vi "NoGV_Omniax_MotorDrive_XYZR_20101203stable2.vi"() -> ()   [LabVIEW 2009]
uses:
  <vilib>/Utility/file.llb/Read From Spreadsheet File (DBL).vi
  <vilib>/Utility/file.llb/Read From Spreadsheet File (string).vi
  <vilib>/Instr/_visa.llb/VISA Configure Serial Port (Instr).vi
  <vilib>/Utility/file.llb/Write To Spreadsheet File (string).vi
  <vilib>/Utility/file.llb/Write To Spreadsheet File (DBL).vi
panel:
  out "Scanning":bool
  out "Laser Shutter":bool
  in  "SHUTTER SYNC":bool
  in  "Laser Shutter":bool
  out "#th loop":dbl
  in  "# of loops":dbl
  in  "LOOP":bool
  out "OP":bool
  out "CL":bool
  out "Valve \nopend/closed":bool
  in  "OK Button":bool
  out "STATUS":string
  in  "Delete Button":bool
  in  "String":string
  in  "Add Button":bool
  in  "Set Button":bool
  in  "Preset positions":i32(ring) items=["ZERO", "Default", "CDOSE", "QMS", "test", "test2", "test3", "yag position", "Sample Long Edge  ", "SPUTTER POS"]
  out "Presets":i32[][](array[numeric])
  out "X MINPOS":i32=-94296
  out "X MAXPOS":i32=-34296
  out "Y MINPOS":i32=-94296
  out "Y MAXPOS":i32=-34296
  out "R MAXPOS":i32=-34296
  out "R MINPOS":i32=-94296
  out "Z MINPOS":i32=-94296
  out "Z MAXPOS":i32=-34296
  in  "HARDSTOP":bool
  in  "GO":bool
  out "XYZR VEL PV Array":i32[](array[numeric])
  out "XYZ in RANGE Array":bool[](array[boolean])
  out "STEP SP Array":i32[](array[numeric])
  out "RUNHOLDArray":i32[](array[numeric])
  out "ZCONSTArray":dbl[](array[numeric])
  out "RCONSTArray":dbl[](array[numeric])
  out "XCONSTArray":dbl[](array[numeric])
  out "YCONSTArray":dbl[](array[numeric])
  out "Error Array":errorcluster[](array[cluster])
  out "COM PORT Array":refnum<visa-resource-name>[](array[refnum])
  out "Z COM PORT":refnum<visa-resource-name>="COM6"
  in  "Tab Control 3":enum32{"Status", "Reset"}(tab)
  out "Y in Range":bool
  out "Y Scan":bool
  out "Y in Motion":bool
  out "Y Backlash corr":bool
  out "X  in Range":bool
  out "X Scan":bool
  out "X  in Motion":bool
  out "X Backlash corr":bool
  out "Z in Range":bool
  out "Z Scan":bool
  out "Z in Motion":bool
  out "Z Backlash corr":bool
  out "R in Range":bool
  out "R Scan":bool
  out "R in Motion":bool
  out "R Backlash corr":bool
  out "X Ready":bool
  out "Y Ready":bool
  out "Z Ready":bool
  out "R Ready":bool
  in  "Reset Y Position mm":dbl
  out "Reset Y Motor Steps":i32
  in  "Reset X Position mm":dbl
  out "Reset X Motor Steps":i32
  in  "Reset Z Position mm":dbl
  out "Reset Z Motor Steps":i32
  in  "Reset R Position deg":dbl
  out "Reset R Motor Steps":i32
  in  "Reset":bool
  in  "Tab Control 2":enum32{"mm", "step"}(tab)
  in  "X Scan Length SP mm":dbl
  in  "X Scan Velocity SP mm/sec":dbl
  in  "Y Scan Length SP mm":dbl
  in  "Y Scan Velocity SP mm/sec":dbl
  in  "Set Scan \nParameters":bool
  in  "Z Scan Length SP mm":dbl
  in  "Z Scan Velocity SP mm/sec":dbl
  in  "R Scan Length SP deg":dbl
  in  "R Scan Velocity SP deg/sec":dbl
  in  "Z as dominating length":bool
  in  "X Scan Velocity SP steps/sec":i32=1 min=1 max=102400 step=1
  in  "X Scan Length SP steps":i32 min=-2304000 max=2304000 step=100
  out "X Scan length MV mm":dbl
  out "X Scan velocity MV mm/sec":dbl format="%#_6f"
  in  "Y Scan Velocity SP steps/sec":i32=1 min=1 max=102400 step=1
  in  "Y Scan Length SP steps":i32 min=-2304000 max=2304000 step=100
  out "Y Scan length MV mm":dbl
  out "Y Scan velocity MV mm/sec":dbl format="%#_6f"
  in  "Z Scan Velocity SP steps/sec":i32=1 min=1 max=204800 step=1
  in  "Z Scan Length SP steps":i32 min=-10240000 max=92160000 step=100
  out "Z Scan length MV mm":dbl
  out "Z Scan velocity MV mm/sec":dbl format="%#_6f"
  in  "R Scan Velocity SP steps/sec":i32=1 min=1 max=102400 step=1
  in  "R Scan Length SP steps":i32 min=-1501867 max=4642133 step=100
  out "R Scan length MV deg":dbl
  out "R Scan velocity MV deg/sec":dbl format="%#_6f"
  out "atan Y/Z":dbl
  in  "Tab Control":enum32{"mm", "step"}(tab)
  in  "X Position SP mm":dbl
  in  "X Velocity SP mm/sec":dbl
  in  "X Move Set":bool
  in  "Y Move Set":bool
  in  "Y Position SP mm":dbl
  in  "Y Velocity SP mm/sec":dbl
  in  "Z Position SP mm":dbl
  in  "Z Velocity SP mm/sec":dbl
  in  "Z Move Set":bool
  in  "R Position SP deg":dbl
  in  "R Velocity SP deg/sec":dbl
  in  "R Move Set":bool
  in  "X Velocity SP step/sec":i32 min=1 max=128000
  out "X Velocity MV mm/sec":dbl
  in  "Y Velocity SP step/sec":i32 min=1 max=128000
  out "Y Velocity MV mm/sec":dbl
  in  "Z Velocity SP step/sec":i32 min=1 max=204800
  out "Z Velocity MV mm/sec":dbl
  in  "R Velocity SP step/sec":i32 min=1 max=20000
  out "R Velocity MVdeg/sec":dbl
  in  "Y Step SP":i32=-20000 min=-2304000 max=2304000 step=500
  out "Y Position MV mm":dbl
  in  "X Step SP":i32=-20000 min=-2304000 max=2304000 step=500
  out "X Position MV mm":dbl
  in  "Z Step SP":i32=-20000 min=0 max=102400000 step=500
  out "Z Position MV mm":dbl
  in  "R Step SP":i32=-20000 min=-6144000 max=0 step=500
  out "R Position MV deg":dbl
  out "X Step PV":i32 max=2000
  out "Y Step PV":i32 max=2000
  out "Z Step PV":i32 max=2000
  out "R Step PV":i32 max=2000
  in  "Clear ZY":bool
  out "ZY Graph":cluster{dbl[], dbl[]}(graph)
  out "ZR Graph":cluster{"Y":dbl[], "Y":dbl[]}[](graph)
  out "XY Graph":cluster{"Y":dbl[], "Y":dbl[]}[](graph)
  out "X Scan Duration":dbl
  out "Y Scan Duration":dbl
  out "Z Scan Duration":dbl
  out "R Scan Duration":dbl
  out "R Backlash steps/sec":i32
  out "R Backlash":i32
  out "R Holding Current %":i32
  out "R Run Current %":i32
  out "R offset deg":dbl
  out "R deg/rev":dbl
  out "R steps/rev":u32
  out "R velocity PV step/sec":i32
  out "R COM PORT":refnum<visa-resource-name>="COM5"
  out "R Position deg PV":dbl=270.5
  out "Z Backlash steps/sec":i32
  out "Z Backlash":i32
  out "Z Holding Current %":i32
  out "Z Run Current %":i32
  out "Z offset mm":dbl
  out "Z mm/rev":dbl
  out "Z steps/rev":u32
  out "Z  velocity PV step/sec":i32
  out "Z Position mm PV":dbl=45.0
  out "X Position mm PV":dbl
  out "X velocity PV step/sec":i32
  in  "Send scan parameter":bool
  out "X Backlash steps/sec":i32
  out "X Backlash":i32
  out "X Holding Current %":i32
  out "X Run Current %":i32
  out "X offset mm":dbl
  out "X mm/rev":dbl
  out "X steps/rev":u32
  out "X COM PORT":refnum<visa-resource-name>="COM5"
  out "Y Backlash steps/sec":i32
  out "Y Backlash":i32
  out "Y Holding Current %":i32
  out "Y Run Current %":i32
  in  "Scan Cancel":bool
  out "Y Position mm PV":dbl
  out "Y offset mm":dbl
  out "Y mm/rev":dbl
  out "Y steps/rev":u32
  out "Y velocity PV step/sec":i32
  in  "Scan Go":bool
  in  "Stop":bool
  out "Y COM PORT":refnum<visa-resource-name>="COM5"
  # "MX"
  # "MY"
  # "MZ"
  # "MR"
  # "Indicators"
  # "L"
  # "M"
  # "B"
  # "S"
  # "R"
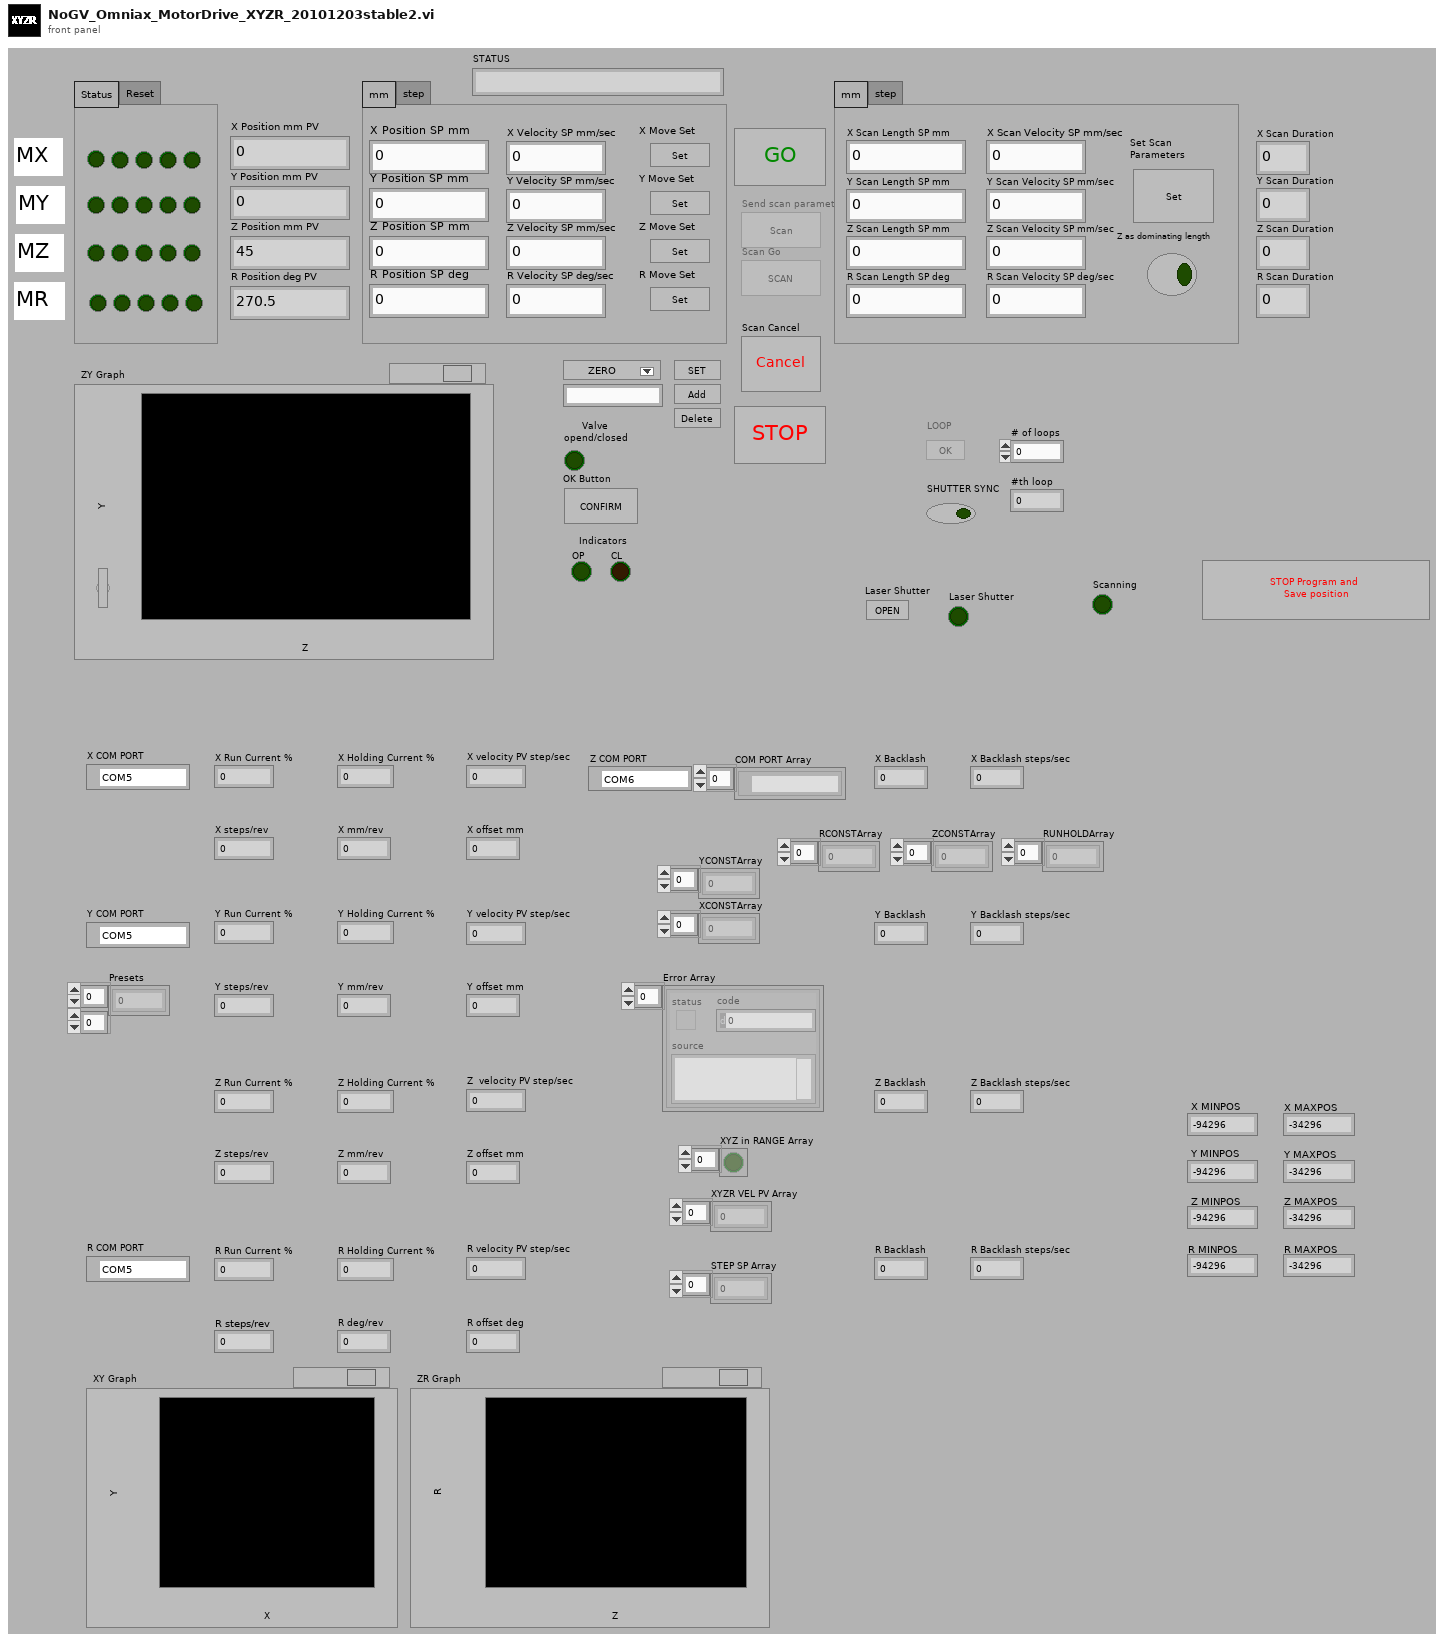
[diagram p1: front panel]
types:
  T1 = cluster{"Error Array OUT[0]":errorcluster, "Error Array OUT[1]":errorcluster, "Error Array OUT[2]":errorcluster, "Error Array OUT[3]":errorcluster, "Error Array OUT[4]":errorcluster, "Error Array OUT[5]":errorcluster, "Error Array OUT[6]":errorcluster, "Error Array OUT[7]":errorcluster, "Error Array OUT[8]":errorcluster}
  T2 = cluster{"COM PORT Array OUT[0]":refnum<visa-resource-name>, "COM PORT Array OUT[1]":refnum<visa-resource-name>, "COM PORT Array OUT[2]":refnum<visa-resource-name>, "COM PORT Array OUT[3]":refnum<visa-resource-name>, "COM PORT Array OUT[4]":refnum<visa-resource-name>, "COM PORT Array OUT[5]":refnum<visa-resource-name>, "COM PORT Array OUT[6]":refnum<visa-resource-name>, "COM PORT Array OUT[7]":refnum<visa-resource-name>, "COM PORT Array OUT[8]":refnum<visa-resource-name>}
  T3 = cluster{"STEP SP Array OUT[0]":i32, "STEP SP Array OUT[1]":i32, "STEP SP Array OUT[2]":i32, "STEP SP Array OUT[3]":i32, "STEP SP Array OUT[4]":i32, "STEP SP Array OUT[5]":i32, "STEP SP Array OUT[6]":i32, "STEP SP Array OUT[7]":i32, "STEP SP Array OUT[8]":i32}
  T4 = cluster{"XYZR MAX MIN POS[0]":i32, "XYZR MAX MIN POS[1]":i32, "XYZR MAX MIN POS[2]":i32, "XYZR MAX MIN POS[3]":i32, "XYZR MAX MIN POS[4]":i32, "XYZR MAX MIN POS[5]":i32, "XYZR MAX MIN POS[6]":i32, "XYZR MAX MIN POS[7]":i32, "XYZR MAX MIN POS[8]":i32}
  T5 = cluster{"XYZ in RANGE Array OUT[0]":bool, "XYZ in RANGE Array OUT[1]":bool, "XYZ in RANGE Array OUT[2]":bool, "XYZ in RANGE Array OUT[3]":bool, "XYZ in RANGE Array OUT[4]":bool, "XYZ in RANGE Array OUT[5]":bool, "XYZ in RANGE Array OUT[6]":bool, "XYZ in RANGE Array OUT[7]":bool, "XYZ in RANGE Array OUT[8]":bool}
  T6 = cluster{"XY Max Min array OUT[0]":dbl, "XY Max Min array OUT[1]":dbl, "XY Max Min array OUT[2]":dbl, "XY Max Min array OUT[3]":dbl, "XY Max Min array OUT[4]":dbl, "XY Max Min array OUT[5]":dbl, "XY Max Min array OUT[6]":dbl, "XY Max Min array OUT[7]":dbl, "XY Max Min array OUT[8]":dbl}
  T7 = cluster{"XYZR VEL PV Array OUT[0]":i32, "XYZR VEL PV Array OUT[1]":i32, "XYZR VEL PV Array OUT[2]":i32, "XYZR VEL PV Array OUT[3]":i32, "XYZR VEL PV Array OUT[4]":i32, "XYZR VEL PV Array OUT[5]":i32, "XYZR VEL PV Array OUT[6]":i32, "XYZR VEL PV Array OUT[7]":i32, "XYZR VEL PV Array OUT[8]":i32}
  T8 = cluster{"[0]":i32, "[1]":i32, "[2]":i32, "[3]":i32, "[4]":i32, "[5]":i32, "[6]":i32, "[7]":i32, "[8]":i32}
  T9 = enum8{"Enabled", "Disabled", "Disabled and Grayed Out"}
  T10 = enum16{"Stop", "Reset", "Run Current", "Holding Current", "Accel Rate", "Decel Rate", "Move to Relative Position", "Move to Absolute Position", "Echo Mode", "Print Parameter", "Send String", "Microstep Resolution", "Set Current Position", "Max Velocity"}
  T11 = cluster{"Presets[0]":i32, "Presets[1]":i32, "Presets[2]":i32, "Presets[3]":i32, "Presets[4]":i32, "Presets[5]":i32, "Presets[6]":i32, "Presets[7]":i32, "Presets[8]":i32}
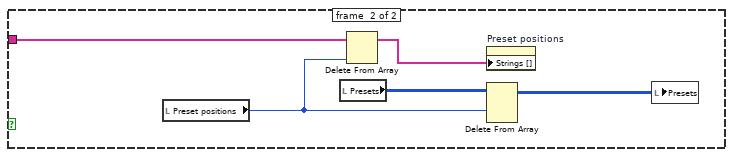
[diagram p4: hidden frame]
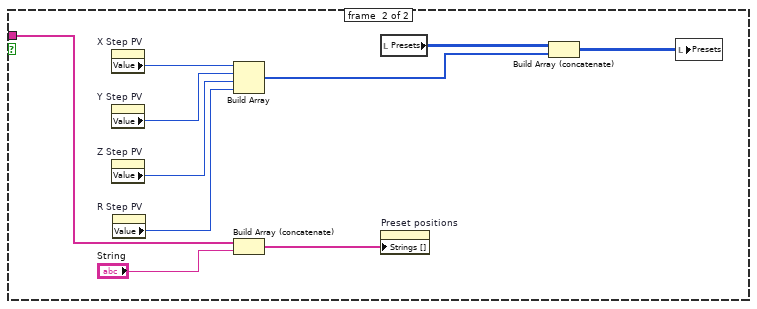
[diagram p5: hidden frame]
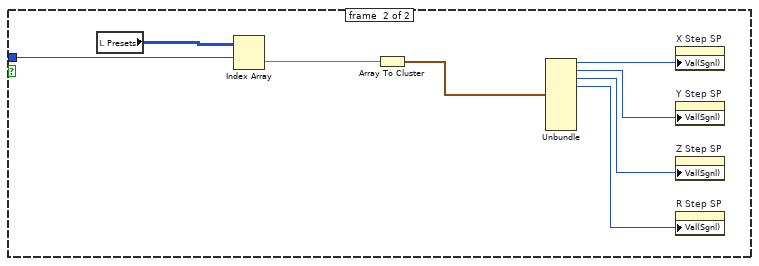
[diagram p6: hidden frame]
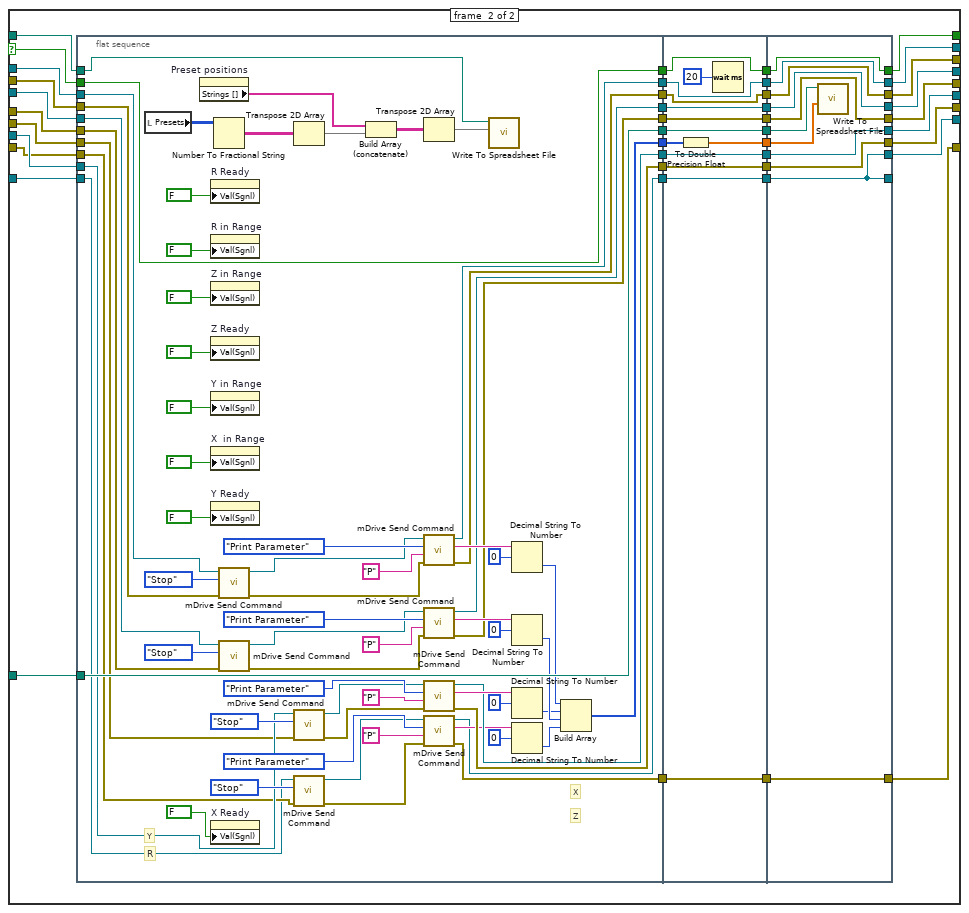
[diagram p7: hidden frame]
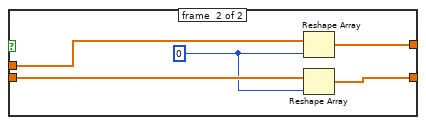
[diagram p8: hidden frame]
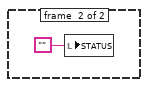
[diagram p10: hidden frame]
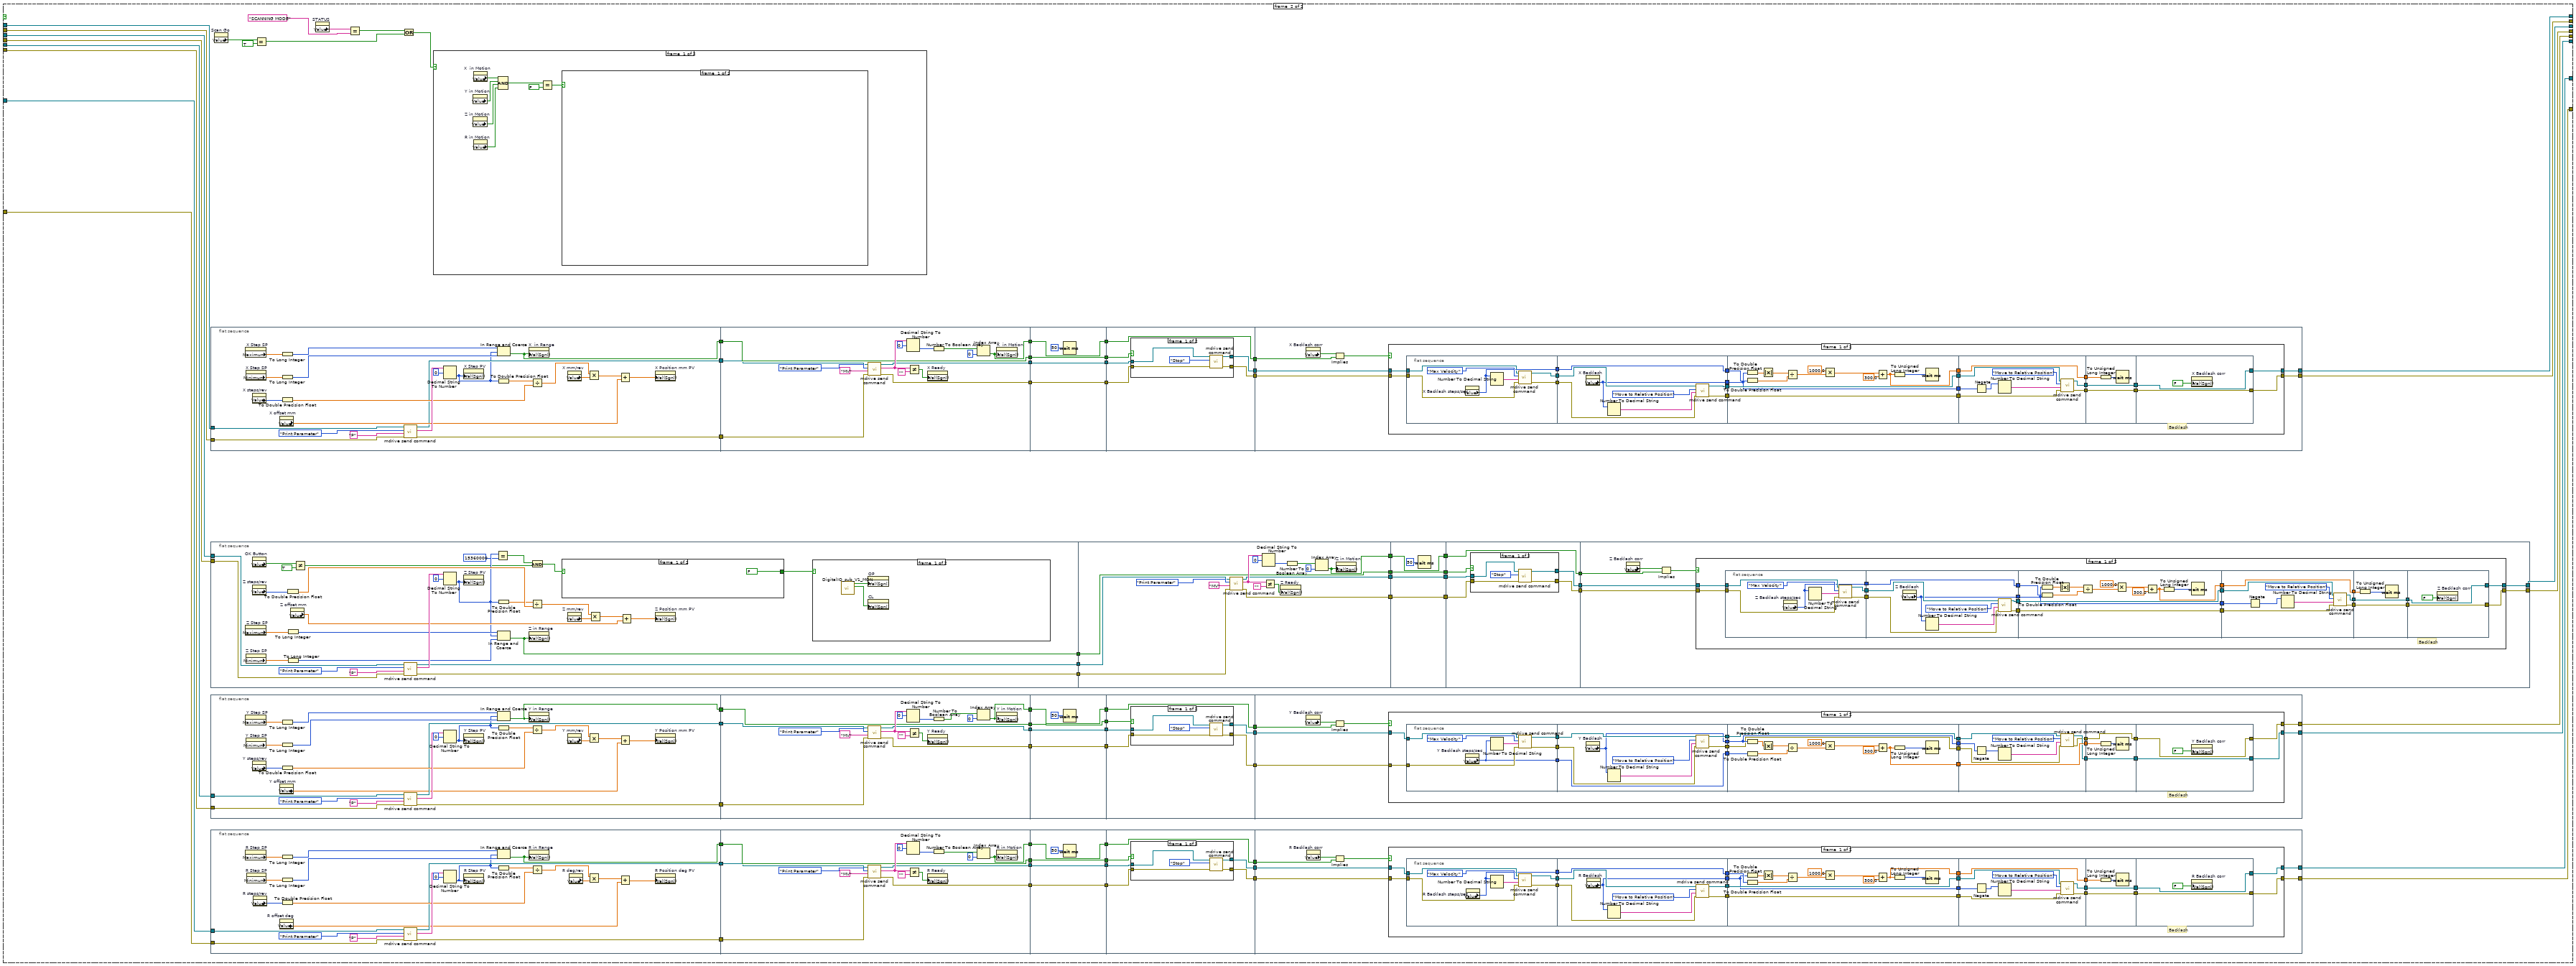
[diagram p11: hidden frame]
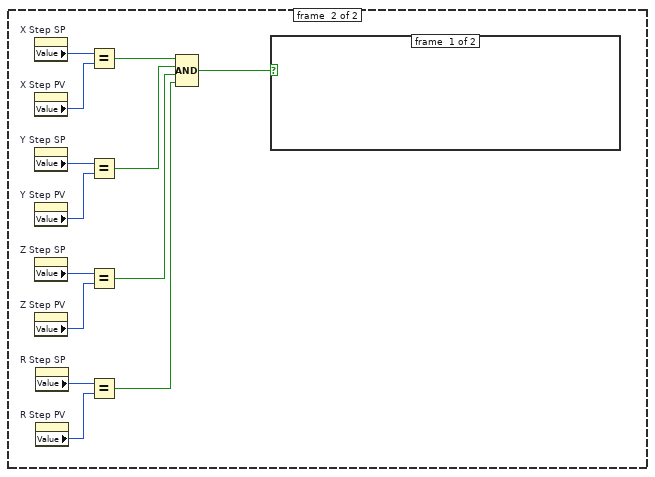
[diagram p12: hidden frame]
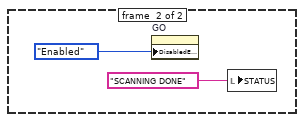
[diagram p13: hidden frame]
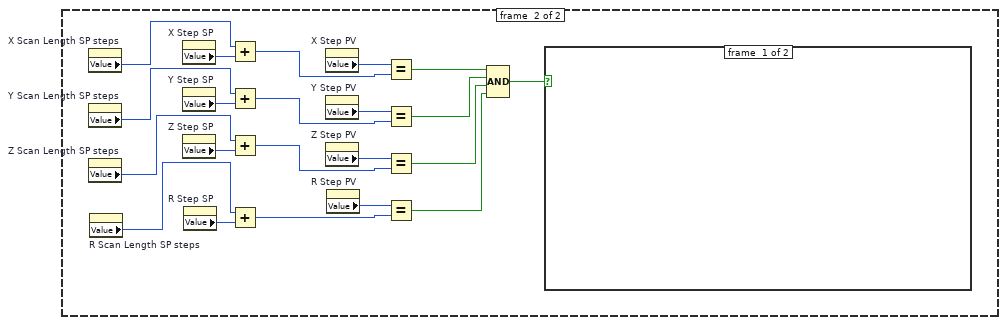
[diagram p14: hidden frame]
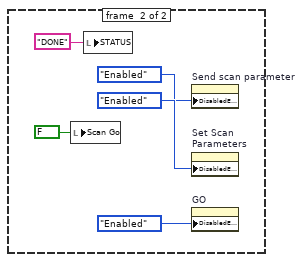
[diagram p15: hidden frame]
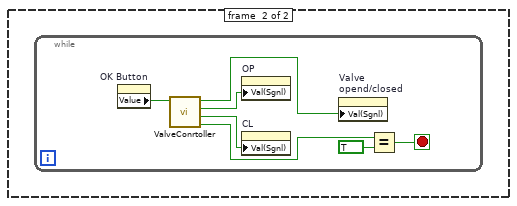
[diagram p20: hidden frame]
diagram:
  (unwired) FALSE ("LOOP MODE")
  n1 = flat-sequence {
    tunnel: [w153] -> w10
    tunnel: [w152] -> w9
    tunnel: [w151] -> w8
    tunnel: [w150] -> w7
    tunnel: [w149] -> w6
    tunnel: [w148] -> w5
    tunnel: [w147] -> w4
    tunnel: [w146] -> w3
    tunnel: [w143] -> w2
    tunnel: [w113] -> w1
    tunnel: [w188] -> w13
    tunnel: [w189] -> w14
    tunnel: [w190] -> w15
    tunnel: [w191] -> w16
    tunnel: [w192] -> w17
    tunnel: [w193] -> w18
    tunnel: [w194] -> w19
    tunnel: [w195] -> w20
    tunnel: [w196] -> w21
    tunnel: [w197] -> w22
    tunnel: w10 -> [w197]
    tunnel: w9 -> [w196]
    tunnel: w8 -> [w195]
    tunnel: w7 -> [w194]
    tunnel: w6 -> [w193]
    tunnel: w5 -> [w192]
    tunnel: w4 -> [w191]
    tunnel: w3 -> [w190]
    tunnel: w2 -> [w189]
    tunnel: w1 -> [w188]
    frame #0 {
      w113 = path "C:/Documents and Settings/b_ogasawara/Desktop/lv1/LV codes/IMS/PRESET.TXT"
      w111 = 0 ("element")
      w143 = path "C:/Documents and Settings/b_ogasawara/Desktop/lv1/LV codes/IMS/POS.TXT"
      w173 = refnum<visa-resource-name> "COM7" ("COM PORT")
      w174 = refnum<visa-resource-name> "COM5" ("COM PORT")
      w175 = refnum<visa-resource-name> "COM6" ("VISA resource name")
      w176 = refnum<visa-resource-name> "COM4" ("COM PORT")
      n2 = property on="Z Step SP" class="DigNum (strict)"() -> ("Maximum"=w68:dbl)  [unwired: 2 in, 2 out]
      n3 = property on="R Step SP" class="DigNum (strict)"() -> ("Maximum"=w66:dbl)  [unwired: 2 in, 2 out]
      n4 = property on="Z Step SP" class="DigNum (strict)"() -> ("Minimum"=w69:dbl)  [unwired: 2 in, 2 out]
      n5 = property on="R Step SP" class="DigNum (strict)"() -> ("Minimum"=w67:dbl)  [unwired: 2 in, 2 out]
      n6 = property on="X steps/rev" class="DigNum (strict)"() -> ("Value"=w84:u32)  [unwired: 2 in, 2 out]
      n7 = property on="Y steps/rev" class="DigNum (strict)"() -> ("Value"=w83:u32)  [unwired: 2 in, 2 out]
      n8 = property on="Z steps/rev" class="DigNum (strict)"() -> ("Value"=w82:u32)  [unwired: 2 in, 2 out]
      n9 = property on="R steps/rev" class="DigNum (strict)"() -> ("Value"=w81:u32)  [unwired: 2 in, 2 out]
      n10 = call "DigitalIO_sub_V1_MON.vi"() -> ("CL"=w70:bool, "OP"=w71:bool)  [unwired: 8 in]
      n11 = local read "RUNHOLDArray"() -> (w163:i32[])
      n12 = local read "STEP SP Array"() -> (w166:i32[])
      n13 = local read "XYZ in RANGE Array"() -> (w165:bool[])
      n14 = local read "XYZR VEL PV Array"() -> (w164:i32[])
      n15 = property on="R offset deg" class="DigNum (strict)"() -> ("Value"=w76:dbl)  [unwired: 2 in, 2 out]
      n16 = property on="X offset mm" class="DigNum (strict)"() -> ("Value"=w73:dbl)  [unwired: 2 in, 2 out]
      n17 = property on="Y offset mm" class="DigNum (strict)"() -> ("Value"=w74:dbl)  [unwired: 2 in, 2 out]
      n18 = property on="Z offset mm" class="DigNum (strict)"() -> ("Value"=w75:dbl)  [unwired: 2 in, 2 out]
      n19 = property on="OP" class="Bool (strict)"("Val(Sgnl)"=w71) -> ()  [unwired: 2 in, 2 out]
      n20 = property on="CL" class="Bool (strict)"("Val(Sgnl)"=w70) -> ()  [unwired: 2 in, 2 out]
      n21 = Build Array(w176, w175, w174, w173) -> (w171:refnum<visa-resource-name>[])
      n22 = Build Array(w68, w69, w66, w67) -> (w65:dbl[])
      n23 = local write "STATUS"("INITIALIZING" ("STATUS")) -> ()
      n24 = for {
        N: 4 -> [_]
        tunnel: w171 -> [w179] mode=indexing
        tunnel: [w178] -> w169 mode=indexing
        tunnel: [w177] -> w170 mode=indexing
        w181 = u16 0 items=["None", "XON/XOFF", "RTS/CTS", "XON/XOFF & RTS/CTS", "DTR/DSR", "XON/XOFF & DTR/DSR"] ("flow control (0:none)")
        w182 = u16 10 items=["1.0"=10, "1.5"=15, "2.0"=20] ("stop bits (10: 1 bit)")
        # "Stop bits"
        n25 = call-poly "VISA Configure Serial Port"("VISA resource name"=w179, "timeout (10sec)"=u32 10000, "baud rate (9600)"=u32 9600, "data bits (8)"=u16 8, "parity (0:none)"=enum16{"None", "Odd", "Even", "Mark", "Space"}."None", "stop bits (10: 1 bit)"=w182, "flow control (0:none)"=w181) -> ("VISA resource name out"=w178:refnum<visa-resource-name>, "error out"=w177:errorcluster)  [unwired: 7 in]
      }
      "COM PORT Array" <- w169
      "Error Array" <- w170
      n26 = call "InitializeMotorsXYZR_V2.vi"("COM PORT Array IN"=w169, "STEP SP Array IN"=w166, "XYZ in RANGE Array IN"=w165, "XYZR VEL PV Array IN"=w164, "RUNHOLDArray IN"=w163, "Error Array IN"=w170, "ZR Max Min array"=w65) -> ("XY Max Min array OUT"=w64:dbl[], "COM PORT Array OUT"=w168:refnum<visa-resource-name>[], "STEP SP Array OUT"=w162:i32[], "XYZ in RANGE Array OUT"=w161:bool[], "XYZR VEL PV Array OUT"=w160:i32[], "XYZR MAX MIN POS"=w145:i32[], "Error Array OUT"=w167:errorcluster[])  [unwired: 6 in]
      n27 = Array To Cluster(array=w167) -> (cluster=w158:T1)
      n28 = Array To Cluster(array=w168) -> (cluster=w159:T2)
      n29 = Array To Cluster(array=w162) -> (cluster=w157:T3)
      n30 = Array To Cluster(array=w145) -> (cluster=w154:T4)
      n31 = Array To Cluster(array=w161) -> (cluster=w156:T5)
      n32 = Array To Cluster(array=w64) -> (cluster=w63:T6)
      n33 = Array To Cluster(array=w160) -> (cluster=w155:T7)
      n34 = Unbundle(w157) -> ("STEP SP Array OUT[0]"=w127:i32, "STEP SP Array OUT[1]"=w128:i32, "STEP SP Array OUT[2]"=w129:i32, "STEP SP Array OUT[3]"=w130:i32)  [unwired: 5 out]
      n35 = Unbundle(w154) -> ("XYZR MAX MIN POS[0]"=w138:i32, "XYZR MAX MIN POS[1]"=w137:i32, "XYZR MAX MIN POS[2]"=w136:i32, "XYZR MAX MIN POS[3]"=w135:i32, "XYZR MAX MIN POS[4]"=w134:i32, "XYZR MAX MIN POS[5]"=w133:i32, "XYZR MAX MIN POS[6]"=w132:i32, "XYZR MAX MIN POS[7]"=w131:i32)  [unwired: 1 out]
      n36 = Unbundle(w156) -> ("XYZ in RANGE Array OUT[0]"=w142:bool, "XYZ in RANGE Array OUT[1]"=w141:bool, "XYZ in RANGE Array OUT[2]"=w140:bool, "XYZ in RANGE Array OUT[3]"=w139:bool)  [unwired: 5 out]
      n37 = Unbundle(w63) -> ("XY Max Min array OUT[0]"=w62:dbl, "XY Max Min array OUT[1]"=w60:dbl, "XY Max Min array OUT[2]"=w59:dbl, "XY Max Min array OUT[3]"=w61:dbl)  [unwired: 5 out]
      n38 = Unbundle(w155) -> ("XYZR VEL PV Array OUT[0]"=w126:i32, "XYZR VEL PV Array OUT[1]"=w125:i32, "XYZR VEL PV Array OUT[2]"=w124:i32, "XYZR VEL PV Array OUT[3]"=w123:i32)  [unwired: 5 out]
      n39 = call-poly <vilib>:"Read From Spreadsheet File.vi"("file path (dialog if empty)"=w113) -> ("all rows"=w118:string[][])  [unwired: 6 in, 4 out]
      n40 = call-poly <vilib>:"Read From Spreadsheet File.vi"("file path (dialog if empty)"=w143) -> ("first row"=w144:dbl[])  [unwired: 6 in, 4 out]
      n41 = To Long Integer(number=w144) -> (32bit integer=w110:i32[])
      n42 = Transpose 2D Array(2D array=w118) -> (transposed array=w117:string[][])
      n43 = property on="X Step SP" class="DigNum (strict)"("Val(Sgnl)"=w127) -> ()  [unwired: 2 in, 2 out]
      n44 = property on="Y Step SP" class="DigNum (strict)"("Val(Sgnl)"=w128) -> ()  [unwired: 2 in, 2 out]
      n45 = property on="Z Step SP" class="DigNum (strict)"("Val(Sgnl)"=w129) -> ()  [unwired: 2 in, 2 out]
      n46 = property on="R Step SP" class="DigNum (strict)"("Val(Sgnl)"=w130) -> ()  [unwired: 2 in, 2 out]
      n47 = property on="X MAXPOS" class="DigNum (strict)"("Val(Sgnl)"=w138) -> ()  [unwired: 2 in, 2 out]
      n48 = property on="X MINPOS" class="DigNum (strict)"("Val(Sgnl)"=w137) -> ()  [unwired: 2 in, 2 out]
      n49 = property on="Y MAXPOS" class="DigNum (strict)"("Val(Sgnl)"=w136) -> ()  [unwired: 2 in, 2 out]
      n50 = property on="Y MINPOS" class="DigNum (strict)"("Val(Sgnl)"=w135) -> ()  [unwired: 2 in, 2 out]
      n51 = property on="Z MAXPOS" class="DigNum (strict)"("Val(Sgnl)"=w134) -> ()  [unwired: 2 in, 2 out]
      n52 = property on="Z MINPOS" class="DigNum (strict)"("Val(Sgnl)"=w133) -> ()  [unwired: 2 in, 2 out]
      n53 = property on="R MAXPOS" class="DigNum (strict)"("Val(Sgnl)"=w132) -> ()  [unwired: 2 in, 2 out]
      n54 = property on="R MINPOS" class="DigNum (strict)"("Val(Sgnl)"=w131) -> ()  [unwired: 2 in, 2 out]
      n55 = property on="X  in Range" class="Bool (strict)"("Val(Sgnl)"=w142) -> ()  [unwired: 2 in, 2 out]
      n56 = property on="Y in Range" class="Bool (strict)"("Val(Sgnl)"=w141) -> ()  [unwired: 2 in, 2 out]
      n57 = property on="Z in Range" class="Bool (strict)"("Val(Sgnl)"=w140) -> ()  [unwired: 2 in, 2 out]
      n58 = property on="R in Range" class="Bool (strict)"("Val(Sgnl)"=w139) -> ()  [unwired: 2 in, 2 out]
      n59 = property on="X velocity PV step/sec" class="DigNum (strict)"("Val(Sgnl)"=w126) -> ()  [unwired: 2 in, 2 out]
      n60 = property on="R velocity PV step/sec" class="DigNum (strict)"("Val(Sgnl)"=w123) -> ()  [unwired: 2 in, 2 out]
      n61 = property on="X Step SP" class="DigNum (strict)"("Maximum"=w62) -> ()  [unwired: 2 in, 2 out]
      n62 = property on="X Step SP" class="DigNum (strict)"("Minimum"=w60) -> ()  [unwired: 2 in, 2 out]
      n63 = property on="Y Step SP" class="DigNum (strict)"("Maximum"=w59) -> ()  [unwired: 2 in, 2 out]
      n64 = property on="Y Step SP" class="DigNum (strict)"("Minimum"=w61) -> ()  [unwired: 2 in, 2 out]
      n65 = property on="Y velocity PV step/sec" class="DigNum (strict)"("Val(Sgnl)"=w125) -> ()  [unwired: 2 in, 2 out]
      n66 = property on="Z  velocity PV step/sec" class="DigNum (strict)"("Val(Sgnl)"=w124) -> ()  [unwired: 2 in, 2 out]
      n67 = Array To Cluster(array=w110) -> (cluster=w109:T8)
      n68 = Delete From Array(array=w117, index (row)=0) -> (deleted portion=w112:string[], array with subset deleted=w115:string[][])  [unwired: 2 in]
      n69 = Transpose 2D Array(2D array=w115) -> (transposed array=w114:string[][])
      n70 = property on="Preset positions" class="Ring (strict)"("Strings []"=w112) -> ()  [unwired: 2 in, 2 out]
      n71 = Unbundle(w109) -> ("[0]"=w85:i32, "[1]"=w86:i32, "[2]"=w87:i32, "[3]"=w88:i32)  [unwired: 5 out]
      n72 = To Double Precision Float(number=w84) -> (double precision float=w105:dbl)
      n73 = To Double Precision Float(number=w85) -> (double precision float=w106:dbl)
      n74 = To Double Precision Float(number=w83) -> (double precision float=w101:dbl)
      n75 = To Double Precision Float(number=w86) -> (double precision float=w102:dbl)
      n76 = To Double Precision Float(number=w87) -> (double precision float=w98:dbl)
      n77 = To Double Precision Float(number=w82) -> (double precision float=w97:dbl)
      n78 = To Double Precision Float(number=w88) -> (double precision float=w94:dbl)
      n79 = To Double Precision Float(number=w81) -> (double precision float=w93:dbl)
      n80 = property on="Reset X Motor Steps" class="DigNum (strict)"("Val(Sgnl)"=w85) -> ()  [unwired: 2 in, 2 out]
      n81 = property on="Reset Y Motor Steps" class="DigNum (strict)"("Val(Sgnl)"=w86) -> ()  [unwired: 2 in, 2 out]
      n82 = property on="Reset Z Motor Steps" class="DigNum (strict)"("Val(Sgnl)"=w87) -> ()  [unwired: 2 in, 2 out]
      n83 = property on="Reset R Motor Steps" class="DigNum (strict)"("Val(Sgnl)"=w88) -> ()  [unwired: 2 in, 2 out]
      n84 = Decimal String To Number(string=w114) -> (number=w116:i32[][])  [unwired: 2 in, 1 out]
      n85 = Divide(x=w106, y=w105) -> (x/y=w108:dbl)
      n86 = Divide(x=w102, y=w101) -> (x/y=w104:dbl)
      n87 = Divide(x=w98, y=w97) -> (x/y=w100:dbl)
      n88 = Divide(x=w94, y=w93) -> (x/y=w96:dbl)
      n89 = Initialize Array(w111, w111, 4 ("dimension size")) -> (w121:i32[][])
      n90 = Build Array (concatenate)(w121, w116) -> (→"Presets":i32[][])
      n91 = property on="X mm/rev" class="DigNum (strict)"() -> ("Value"=w78:dbl)  [unwired: 2 in, 2 out]
      n92 = property on="Y mm/rev" class="DigNum (strict)"() -> ("Value"=w79:dbl)  [unwired: 2 in, 2 out]
      n93 = property on="Z mm/rev" class="DigNum (strict)"() -> ("Value"=w80:dbl)  [unwired: 2 in, 2 out]
      n94 = property on="R deg/rev" class="DigNum (strict)"() -> ("Value"=w77:dbl)  [unwired: 2 in, 2 out]
      n95 = Multiply(x=w108, y=w78) -> (x*y=w107:dbl)
      n96 = Multiply(x=w104, y=w79) -> (x*y=w103:dbl)
      n97 = Multiply(x=w100, y=w80) -> (x*y=w99:dbl)
      n98 = Multiply(x=w96, y=w77) -> (x*y=w95:dbl)
      n99 = Add(x=w107, y=w73) -> (x+y=w89:dbl)
      n100 = Add(x=w103, y=w74) -> (x+y=w90:dbl)
      n101 = Add(x=w99, y=w75) -> (x+y=w91:dbl)
      n102 = Add(x=w95, y=w76) -> (x+y=w92:dbl)
      n103 = property on="X Position mm PV" class="DigNum (strict)"("Val(Sgnl)"=w89) -> ()  [unwired: 2 in, 2 out]
      n104 = property on="X Position SP mm" class="DigNum (strict)"("Val(Sgnl)"=w89) -> ()  [unwired: 2 in, 2 out]
      n105 = property on="Y Position SP mm" class="DigNum (strict)"("Val(Sgnl)"=w90) -> ()  [unwired: 2 in, 2 out]
      n106 = property on="Y Position mm PV" class="DigNum (strict)"("Val(Sgnl)"=w90) -> ()  [unwired: 2 in, 2 out]
      n107 = property on="Z Position SP mm" class="DigNum (strict)"("Val(Sgnl)"=w91) -> ()  [unwired: 2 in, 2 out]
      n108 = property on="Z Position mm PV" class="DigNum (strict)"("Val(Sgnl)"=w91) -> ()  [unwired: 2 in, 2 out]
      n109 = property on="R Position deg PV" class="DigNum (strict)"("Val(Sgnl)"=w92) -> ()  [unwired: 2 in, 2 out]
      n110 = property on="R Position SP deg" class="DigNum (strict)"("Val(Sgnl)"=w92) -> ()  [unwired: 2 in, 2 out]
      n111 = Unbundle(w159) -> ("COM PORT Array OUT[0]"=w153:refnum<visa-resource-name>, "COM PORT Array OUT[1]"=w152:refnum<visa-resource-name>, "COM PORT Array OUT[2]"=w151:refnum<visa-resource-name>, "COM PORT Array OUT[3]"=w150:refnum<visa-resource-name>)  [unwired: 5 out]
      n112 = Unbundle(w158) -> ("Error Array OUT[0]"=w149:errorcluster, "Error Array OUT[1]"=w148:errorcluster, "Error Array OUT[2]"=w147:errorcluster, "Error Array OUT[3]"=w146:errorcluster)  [unwired: 5 out]
      "X COM PORT" <- w176
      "Z COM PORT" <- w175
      "Y COM PORT" <- w174
      "R COM PORT" <- w173
    }
    frame #1 {
      w186 = T9."Disabled and Grayed Out" ("Disabled")
      w187 = T9."Enabled" ("Disabled")
      n113 = property on="LOOP" class="Bool (strict)"("DisabledEnum"=w186) -> ()  [unwired: 2 in, 2 out]
      n114 = property on="GO" class="Bool"("DisabledEnum"=w187) -> ()  [unwired: 2 in, 2 out]
      n115 = property on="Set Scan \nParameters" class="Bool"("DisabledEnum"=w187) -> ()  [unwired: 2 in, 2 out]
      n116 = property on="Send scan parameter" class="Bool"("DisabledEnum"=w186) -> ()  [unwired: 2 in, 2 out]
    }
  }
  n117 = flat-sequence {
    frame #0 {
      n118 = property on="Y Scan" class="Bool (strict)"("Val(Sgnl)"=FALSE ("Value (Signaling)")) -> ()  [unwired: 2 in, 2 out]
      n119 = property on="Z Scan Velocity SP mm/sec" class="DigNum (strict)"("Val(Sgnl)"=0.1 ("Value (Signaling)")) -> ()  [unwired: 2 in, 2 out]
      n120 = property on="Z Scan Velocity SP steps/sec" class="DigNum (strict)"("Minimum"=1.0 ("Data Entry Limits:Maximum")) -> ()  [unwired: 2 in, 2 out]
      n121 = property on="R Scan" class="Bool (strict)"("Val(Sgnl)"=FALSE ("Value (Signaling)")) -> ()  [unwired: 2 in, 2 out]
      n122 = property on="X Scan Velocity SP mm/sec" class="DigNum (strict)"("Val(Sgnl)"=0.1 ("Value (Signaling)")) -> ()  [unwired: 2 in, 2 out]
      n123 = property on="R Velocity SP deg/sec" class="DigNum (strict)"("Val(Sgnl)"=0.1 ("Value (Signaling)")) -> ()  [unwired: 2 in, 2 out]
      n124 = property on="Z Scan Velocity SP steps/sec" class="DigNum (strict)"("Maximum"=204800.0 ("Data Entry Limits:Maximum")) -> ()  [unwired: 2 in, 2 out]
      n125 = property on="X Scan" class="Bool (strict)"("Val(Sgnl)"=FALSE ("Value (Signaling)")) -> ()  [unwired: 2 in, 2 out]
      n126 = property on="Y Scan Velocity SP mm/sec" class="DigNum (strict)"("Val(Sgnl)"=0.1 ("Value (Signaling)")) -> ()  [unwired: 2 in, 2 out]
      n127 = property on="Z Scan" class="Bool (strict)"("Val(Sgnl)"=FALSE ("Value (Signaling)")) -> ()  [unwired: 2 in, 2 out]
      n128 = property on="Scan Go" class="Bool (strict)"("DisabledEnum"=T9."Disabled and Grayed Out" ("Disabled")) -> ()  [unwired: 2 in, 2 out]
    }
  }
  n129 = local read "X  in Range"() -> (w33:bool)
  n130 = flat-sequence {
    tunnel: [w212] -> w45
    frame #0 {
      w210 = 0.2 ("MM/rev")
      w215 = u32 51200 ("step/rev")
      w217 = 128000 ("Value (Signaling)")
      w218 = 1.0 ("Data Entry Limits:Minimum")
      w211 = 0.0 ("offset")
      # "a=1000000"
      n131 = property on="X Velocity SP step/sec" class="DigNum (strict)"("Val(Sgnl)"=w217) -> ()  [unwired: 2 in, 2 out]
      n132 = To Double Precision Float(number=w215) -> (double precision float=w220:dbl)
      n133 = To Double Precision Float(number=w217) -> (double precision float=w209:dbl)
      n134 = Divide(x=w209, y=w220) -> (x/y=w219:dbl)
      n135 = property on="X Velocity SP step/sec" class="DigNum (strict)"("Maximum"=w209) -> ()  [unwired: 2 in, 2 out]
      n136 = Multiply(x=w219, y=w210) -> (x*y=w213:dbl)
      n137 = To Double Precision Float(number=w217) -> (double precision float=w216:dbl)
      n138 = To Double Precision Float(number=w215) -> (double precision float=w214:dbl)
      n139 = property on="X Velocity SP step/sec" class="DigNum (strict)"("Minimum"=w218) -> ()  [unwired: 2 in, 2 out]
      n140 = Build Array(w218, w216, w214, w213, w209, w210, w211) -> (w212:dbl[])
      n141 = property on="X Velocity SP mm/sec" class="DigNum (strict)"("Val(Sgnl)"=w213) -> ()  [unwired: 2 in, 2 out]
      "X offset mm" <- w211
      "X steps/rev" <- w215
      "X mm/rev" <- w210
    }
  }
  n142 = local read "Z  velocity PV step/sec"() -> (w26:i32)
  n143 = flat-sequence {
    tunnel: [w224] -> w46
    frame #0 {
      w222 = 0.2 ("MM/rev")
      w227 = u32 51200 ("step/rev")
      w229 = 128000 ("Value (Signaling)")
      w230 = 1.0 ("Data Entry Limits:Minimum")
      w223 = 0.0 ("offset")
      n144 = property on="Y Velocity SP step/sec" class="DigNum (strict)"("Val(Sgnl)"=w229) -> ()  [unwired: 2 in, 2 out]
      n145 = To Double Precision Float(number=w227) -> (double precision float=w232:dbl)
      n146 = To Double Precision Float(number=w229) -> (double precision float=w221:dbl)
      n147 = Divide(x=w221, y=w232) -> (x/y=w231:dbl)
      n148 = property on="Y Velocity SP step/sec" class="DigNum (strict)"("Maximum"=w221) -> ()  [unwired: 2 in, 2 out]
      n149 = Multiply(x=w231, y=w222) -> (x*y=w225:dbl)
      n150 = To Double Precision Float(number=w229) -> (double precision float=w228:dbl)
      n151 = To Double Precision Float(number=w227) -> (double precision float=w226:dbl)
      n152 = property on="Y Velocity SP step/sec" class="DigNum (strict)"("Minimum"=w230) -> ()  [unwired: 2 in, 2 out]
      n153 = Build Array(w230, w228, w226, w225, w221, w222, w223) -> (w224:dbl[])
      n154 = property on="Y Velocity SP mm/sec" class="DigNum (strict)"("Val(Sgnl)"=w225) -> ()  [unwired: 2 in, 2 out]
      "Y offset mm" <- w223
      "Y steps/rev" <- w227
      "Y mm/rev" <- w222
    }
  }
  n155 = flat-sequence {
    frame #0 {
      n156 = property on="X Backlash corr" class="Bool (strict)"("Val(Sgnl)"=FALSE ("Value (Signaling)")) -> ()  [unwired: 2 in, 2 out]
      n157 = property on="Y Backlash corr" class="Bool (strict)"("Val(Sgnl)"=FALSE ("Value (Signaling)")) -> ()  [unwired: 2 in, 2 out]
      n158 = property on="R Backlash corr" class="Bool (strict)"("Val(Sgnl)"=FALSE ("Value (Signaling)")) -> ()  [unwired: 2 in, 2 out]
      n159 = property on="Z Backlash corr" class="Bool (strict)"("Val(Sgnl)"=FALSE ("Value (Signaling)")) -> ()  [unwired: 2 in, 2 out]
      "Z Backlash steps/sec" <- 25600 ("Z Backlash steps/sec")
      "Z Backlash" <- -12800 ("Z Backlash")
      "X Backlash steps/sec" <- 25600 ("Value (Signaling)")
      "X Backlash" <- 5120 ("Backlash2")
      "Y Backlash" <- -5120 ("Backlash2")
      "Y Backlash steps/sec" <- 25600 ("Value (Signaling)")
      "R Backlash steps/sec" <- 6400 ("R Backlash steps/sec")
      "R Backlash" <- -12800 ("R Backlash")
    }
  }
  n160 = flat-sequence {
    tunnel: [w245] -> w43
    frame #0 {
      w247 = 0.2 ("Z mm/rev")
      w251 = u32 51200 ("step/rev")
      w253 = 204800 ("Value (Signaling)")
      w254 = 1.0 ("Data Entry Limits:Minimum")
      w246 = 0.0 ("Z offset mm")
      n161 = property on="Z Velocity SP step/sec" class="DigNum (strict)"("Val(Sgnl)"=w253) -> ()  [unwired: 2 in, 2 out]
      n162 = To Double Precision Float(number=w251) -> (double precision float=w256:dbl)
      n163 = To Double Precision Float(number=w253) -> (double precision float=w249:dbl)
      n164 = Divide(x=w249, y=w256) -> (x/y=w255:dbl)
      n165 = property on="Z Velocity SP step/sec" class="DigNum (strict)"("Maximum"=w249) -> ()  [unwired: 2 in, 2 out]
      n166 = Multiply(x=w255, y=w247) -> (x*y=w248:dbl)
      n167 = To Double Precision Float(number=w251) -> (double precision float=w250:dbl)
      n168 = To Double Precision Float(number=w253) -> (double precision float=w252:dbl)
      n169 = Build Array(w254, w252, w250, w249, w248, w247, w246) -> (w245:dbl[])
      n170 = property on="Z Velocity SP mm/sec" class="DigNum (strict)"("Val(Sgnl)"=w248) -> ()  [unwired: 2 in, 2 out]
      n171 = property on="Z Velocity SP step/sec" class="DigNum (strict)"("Minimum"=w254) -> ()  [unwired: 2 in, 2 out]
      "Z offset mm" <- w246
      "Z mm/rev" <- w247
      "Z steps/rev" <- w251
    }
  }
  n172 = flat-sequence {
    tunnel: [w257] -> w42
    frame #0 {
      w260 = 20 ("R Holding Current %")
      w259 = 100 ("R Run Current %")
      w262 = 20 ("Holding Current %")
      w261 = 40 ("Run Current %")
      w264 = 20 ("Holding Current %")
      w265 = 40 ("Run Current %")
      w263 = 40 ("Z Run Current %")
      w258 = 20 ("Z Holding Current %")
      n173 = Build Array(w265, w264, w263, w262, w261, w260, w259, w258) -> (w257:i32[])
      "Z Holding Current %" <- w258
      "Z Run Current %" <- w263
      "X Run Current %" <- w265
      "X Holding Current %" <- w264
      "Y Run Current %" <- w261
      "Y Holding Current %" <- w262
      "R Holding Current %" <- w260
      "R Run Current %" <- w259
    }
  }
  n174 = flat-sequence {
    tunnel: [w266] -> w44
    frame #0 {
      w275 = 1.0 ("Data Entry Limits:Minimum")
      w269 = 0.0 ("R offset deg")
      w270 = -3.0 ("R deg/rev")
      w273 = u32 51200 ("step/rev")
      w274 = 20000 ("Value (Signaling)")
      n175 = property on="R Velocity SP step/sec" class="DigNum (strict)"("Val(Sgnl)"=w274) -> ()  [unwired: 2 in, 2 out]
      n176 = To Double Precision Float(number=w273) -> (double precision float=w276:dbl)
      n177 = To Double Precision Float(number=w274) -> (double precision float=w272:dbl)
      n178 = Divide(x=w272, y=w276) -> (x/y=w278:dbl)
      n179 = property on="R Velocity SP step/sec" class="DigNum (strict)"("Maximum"=w272) -> ()  [unwired: 2 in, 2 out]
      n180 = Multiply(x=w278, y=w270) -> (x*y=w277:dbl)
      n181 = To Double Precision Float(number=w273) -> (double precision float=w267:dbl)
      n182 = To Double Precision Float(number=w274) -> (double precision float=w268:dbl)
      n183 = Absolute Value(x=w277) -> (abs(x)=w271:dbl)
      n184 = Build Array(w275, w268, w267, w272, w271, w270, w269) -> (w266:dbl[])
      n185 = property on="R Velocity SP deg/sec" class="DigNum (strict)"("Val(Sgnl)"=w271) -> ()  [unwired: 2 in, 2 out]
      n186 = property on="R Velocity SP step/sec" class="DigNum (strict)"("Minimum"=w275) -> ()  [unwired: 2 in, 2 out]
      "R offset deg" <- w269
      "R deg/rev" <- w270
      "R steps/rev" <- w273
    }
  }
  n187 = local read "Y in Range"() -> (w32:bool)
  n188 = local read "Z in Range"() -> (w31:bool)
  n189 = local read "R in Range"() -> (w30:bool)
  n190 = local read "X velocity PV step/sec"() -> (w29:i32)
  n191 = local read "Y velocity PV step/sec"() -> (w27:i32)
  n192 = local read "R velocity PV step/sec"() -> (w28:i32)
  n193 = property on="Z Step SP" class="DigNum (strict)"("Minimum"=0.0 ("lower limit")) -> ()  [unwired: 2 in, 2 out]
  n194 = property on="R Step SP" class="DigNum (strict)"("Maximum"=0.0 ("Data Entry Limits:Maximum")) -> ()  [unwired: 2 in, 2 out]
  n195 = property on="R Step SP" class="DigNum (strict)"("Minimum"=-6144000.0 ("Data Entry Limits:Minimum")) -> ()  [unwired: 2 in, 2 out]
  n196 = property on="Z Step SP" class="DigNum (strict)"("Maximum"=102400000.0 ("upper limit")) -> ()  [unwired: 2 in, 2 out]
  n197 = Build Array(w33, w32, w31, w30) -> (→"XYZ in RANGE Array":bool[])
  n198 = Build Array("X Step SP", "Y Step SP", "Z Step SP", "R Step SP", "X Velocity SP step/sec", "Y Velocity SP step/sec", "Z Velocity SP step/sec", "R Velocity SP step/sec") -> (→"STEP SP Array":i32[])
  n199 = Build Array(w29, w27, w26, w28) -> (→"XYZR VEL PV Array":i32[])
  n200 = while {
    tunnel: [w306] -> w49
    tunnel: [w309] -> w50
    tunnel: [w312] -> w58
    tunnel: [w305] -> w57
    tunnel: [w311] -> w52
    tunnel: [w310] -> w51
    tunnel: [w308] -> w48
    tunnel: [w307] -> w47
    tunnel: w22 -> [w320]
    tunnel: w21 -> [w318]
    tunnel: w20 -> [w316]
    tunnel: w19 -> [w314]
    tunnel: w18 -> [w319]
    tunnel: w17 -> [w317]
    tunnel: w16 -> [w315]
    tunnel: w15 -> [w313]
    tunnel: w14 -> [w302]
    tunnel: w13 -> [w301]
    shift-right: [w295] -> _
    shift-left: dbl[] [] -> [w293]
    shift-right: [w294] -> _
    shift-left: dbl[] [] -> [w292]
    stop <- w303 stop-if-true
    # "XZYR"
    n201 = property on="Preset positions" class="Ring (strict)"() -> ("Strings []"=w296:string[])  [unwired: 2 in, 2 out]
    n202 = event shown="[0] Timeout" {
      selector: _ -> [_ _ _ _ _ _ _ _ _ _ _ _ _ _ _ _ _]
      dyn-events: _ -> [_ _ _ _ _ _ _ _ _ _ _ _ _ _ _ _ _]
      timeout: 100 -> [_ _ _ _ _ _ _ _ _ _ _ _ _ _ _ _ _]
      tunnel: w320 -> [w524 _ w1393 w1689 _ _ _ _ _ _ _ _ w2219 w2353 w2420 w2650 w2698]
      tunnel: w319 -> [w523 _ w1392 w1710 _ _ _ _ _ _ _ _ w2220 w2351 w2419 w2654 w2694]
      tunnel: w318 -> [w522 _ w1390 w1692 _ _ _ _ _ _ _ _ w2187 w2352 w2418 w2649 w2696]
      tunnel: w317 -> [w521 _ w1391 w1709 _ _ _ _ _ _ _ _ w2188 w2350 w2417 w2653 w2692]
      tunnel: w316 -> [w520 _ w1388 w1695 _ _ _ _ _ _ _ _ w2199 w2349 w2416 w2648 w2690]
      tunnel: w315 -> [w519 _ w1389 w1708 _ _ _ _ _ _ _ _ w2200 w2347 w2415 w2652 w2688]
      tunnel: w314 -> [w518 _ w1386 w1698 _ _ _ _ _ _ _ _ w2175 w2348 w2414 w2647 w2702]
      tunnel: w313 -> [w517 _ w1387 w1707 _ _ _ _ _ _ _ _ w2176 w2346 w2413 w2651 w2700]
      tunnel: [w500 _ _ _ _ _ _ _ _ _ _ _ _ _ _ _ _] -> w295
      tunnel: [w498 _ _ _ _ _ _ _ _ _ _ _ _ _ _ _ _] -> w294
      tunnel: w293 -> [w503 _ _ _ _ _ _ _ _ _ _ _ _ _ _ _ _]
      tunnel: w292 -> [w502 _ _ _ _ _ _ _ _ _ _ _ _ _ _ _ _]
      tunnel: [w496 _ w1371 _ _ _ _ _ _ _ _ _ _ _ _ _ _] -> w286
      tunnel: [w495 _ w1370 _ _ _ _ _ _ _ _ _ _ _ _ _ _] -> w283
      tunnel: [w494 _ w1369 _ _ _ _ _ _ _ _ _ _ _ _ _ _] -> w285
      tunnel: [w493 _ w1368 _ _ _ _ _ _ _ _ _ _ _ _ _ _] -> w284
      tunnel: [w490 _ w1367 _ _ _ _ _ _ _ _ _ _ _ _ _ _] -> w282
      tunnel: [w489 _ w1366 _ _ _ _ _ _ _ _ _ _ _ _ _ _] -> w281
      tunnel: [w492 _ w1365 _ _ _ _ _ _ _ _ _ _ _ _ _ _] -> w279
      tunnel: [_ _ w1364 _ _ _ _ _ _ _ _ _ _ _ _ _ _] -> w280
      tunnel: [w491 _ _ _ _ _ _ _ _ _ _ _ _ _ _ _ _] -> _
      event #0 {
        # "R"
        # "Y"
        # "Z"
        # "X"
        n203 = event-data() -> ()  [unwired: 1 in, 2 out]
        n204 = property on="X Position mm PV" class="DigNum (strict)"() -> ("Value"=w537:dbl)  [unwired: 2 in, 2 out]
        n205 = property on="Z Position mm PV" class="DigNum (strict)"() -> ("Value"=w506:dbl)  [unwired: 2 in, 2 out]
        n206 = property on="Y Position mm PV" class="DigNum (strict)"() -> ("Value"=w505:dbl)  [unwired: 2 in, 2 out]
        n207 = property on="R Position deg PV" class="DigNum (strict)"() -> ("Value"=w538:dbl)  [unwired: 2 in, 2 out]
        n208 = property on="GO" class="Bool"() -> ("DisabledEnum"=w513:T9)  [unwired: 2 in, 2 out]
        n209 = property on="Y Scan Length SP steps" class="DigNum (strict)"() -> ("Value"=w527:i32)  [unwired: 2 in, 2 out]
        n210 = property on="Z Scan Length SP steps" class="DigNum (strict)"() -> ("Value"=w528:i32)  [unwired: 2 in, 2 out]
        n211 = call "Build XY Graph2"("Reset"=TRUE, "Y Input"=w538, "X Input"=w506) -> ("XY Graph"=→"ZR Graph":cluster{"Y":dbl[], "Y":dbl[]}[])  [unwired: 7 in, 1 out]
        n212 = call "Build XY Graph"("Reset"=TRUE, "Y Input"=w505, "X Input"=w537) -> ("XY Graph"=→"XY Graph":cluster{"Y":dbl[], "Y":dbl[]}[])  [unwired: 7 in, 1 out]
        n213 = Build Array (concatenate)(w503, w506) -> (w501:dbl[])
        n214 = Build Array (concatenate)(w502, w505) -> (w499:dbl[])
        n215 = Equal?(x=w513, y=T9."Enabled") -> (x = y?=w511:bool)
        n216 = To Double Precision Float(number=w527) -> (double precision float=w526:dbl)
        n217 = To Double Precision Float(number=w528) -> (double precision float=w525:dbl)
        n218 = Bundle(w501, w499) -> (→"ZY Graph":cluster{dbl[], dbl[]})  [unwired: 1 in]
        n219 = property on="Clear ZY" class="Bool (strict)"() -> ("Value"=w497:bool)  [unwired: 2 in, 2 out]
        n220 = property on="Scan Go" class="Bool (strict)"() -> ("DisabledEnum"=w510:T9)  [unwired: 2 in, 2 out]
        n221 = property on="GO" class="Bool"() -> ("DisabledEnum"=w516:T9)  [unwired: 2 in, 2 out]
        n222 = Divide(x=w526, y=w525) -> (x/y=w529:dbl)
        n223 = Equal?(x=w510, y=T9."Disabled and Grayed Out") -> (x = y?=w507:bool)
        n224 = Equal?(x=w516, y=T9."Disabled and Grayed Out") -> (x = y?=w514:bool)
        n225 = Inverse Tangent(1:w529) -> (0:w530:dbl)
        n226 = case shown="False" w514 {
          tunnel: [w580 w706] -> w496
          tunnel: [w579 w705] -> w495
          tunnel: [w578 w704] -> w494
          tunnel: [w577 w703] -> w493
          tunnel: [w576 w702] -> w490
          tunnel: [w575 w701] -> w489
          tunnel: [w574 w700] -> w492
          tunnel: [w573 w699] -> w491
          tunnel: w524 -> [w566 w698]
          tunnel: w523 -> [w564 w697]
          tunnel: w522 -> [w553 w696]
          tunnel: w521 -> [w552 w695]
          tunnel: w520 -> [w557 w694]
          tunnel: w519 -> [w556 w693]
          tunnel: w518 -> [w562 w692]
          tunnel: w517 -> [w563 w691]
          frame #0 {
            n227 = flat-sequence {
              tunnel: [w621] -> w558
              tunnel: w557 -> [w620]
              tunnel: [w619] -> w559
              tunnel: w556 -> [w618]
              frame #0 {
                n228 = property on="Y Step SP" class="DigNum (strict)"() -> ("Maximum"=w635:dbl)  [unwired: 2 in, 2 out]
                n229 = property on="Y Step SP" class="DigNum (strict)"() -> ("Minimum"=w637:dbl)  [unwired: 2 in, 2 out]
                n230 = property on="Y steps/rev" class="DigNum (strict)"() -> ("Value"=w632:u32)  [unwired: 2 in, 2 out]
                n231 = property on="Y mm/rev" class="DigNum (strict)"() -> ("Value"=w630:dbl)  [unwired: 2 in, 2 out]
                n232 = To Long Integer(number=w635) -> (32bit integer=w634:i32)
                n233 = To Long Integer(number=w637) -> (32bit integer=w636:i32)
                n234 = To Double Precision Float(number=w632) -> (double precision float=w633:dbl)
                n235 = call "mdrive send command.vi"("error in (no error)"=w618, "Extra"="P", "Command"=T10."Print Parameter", "VISA resource name"=w620) -> ("error out"=w619:errorcluster, "read buffer"=w639:string, "VISA resource name out"=w621:refnum<visa-resource-name>)  [unwired: 3 in]
                n236 = Decimal String To Number(string=w639, offset=0) -> (number=w622:i32)  [unwired: 1 in, 1 out]
                n237 = In Range and Coerce(upper limit=w634, x=w622, lower limit=w636) -> (In Range?=w623:bool)  [unwired: 1 out]
                n238 = To Double Precision Float(number=w622) -> (double precision float=w627:dbl)
                n239 = Divide(x=w627, y=w633) -> (x/y=w631:dbl)
                n240 = property on="Y offset mm" class="DigNum (strict)"() -> ("Value"=w628:dbl)  [unwired: 2 in, 2 out]
                n241 = Multiply(x=w631, y=w630) -> (x*y=w629:dbl)
                n242 = Add(x=w629, y=w628) -> (x+y=w626:dbl)
                n243 = property on="Y Position mm PV" class="DigNum (strict)"("Val(Sgnl)"=w626) -> ()  [unwired: 2 in, 2 out]
                n244 = property on="Y in Range" class="Bool (strict)"("Val(Sgnl)"=w623) -> ()  [unwired: 2 in, 2 out]
                n245 = property on="Y Step PV" class="DigNum (strict)"("Val(Sgnl)"=w622) -> ()  [unwired: 2 in, 2 out]
              }
            }
            n246 = flat-sequence {
              tunnel: [w665] -> w551
              tunnel: w566 -> [w664]
              tunnel: [w663] -> w565
              tunnel: w564 -> [w662]
              frame #0 {
                n247 = property on="X Step SP" class="DigNum (strict)"() -> ("Maximum"=w679:dbl)  [unwired: 2 in, 2 out]
                n248 = property on="X Step SP" class="DigNum (strict)"() -> ("Minimum"=w681:dbl)  [unwired: 2 in, 2 out]
                n249 = property on="X steps/rev" class="DigNum (strict)"() -> ("Value"=w676:u32)  [unwired: 2 in, 2 out]
                n250 = To Long Integer(number=w679) -> (32bit integer=w678:i32)
                n251 = To Long Integer(number=w681) -> (32bit integer=w680:i32)
                n252 = To Double Precision Float(number=w676) -> (double precision float=w677:dbl)
                n253 = call "mdrive send command.vi"("error in (no error)"=w662, "Extra"="P", "Command"=T10."Print Parameter", "VISA resource name"=w664) -> ("error out"=w663:errorcluster, "read buffer"=w683:string, "VISA resource name out"=w665:refnum<visa-resource-name>)  [unwired: 3 in]
                n254 = Decimal String To Number(string=w683, offset=0) -> (number=w666:i32)  [unwired: 1 in, 1 out]
                n255 = property on="X Step PV" class="DigNum (strict)"("Val(Sgnl)"=w666) -> ()  [unwired: 2 in, 2 out]
                n256 = In Range and Coerce(upper limit=w678, x=w666, lower limit=w680) -> (In Range?=w667:bool)  [unwired: 1 out]
                n257 = To Double Precision Float(number=w666) -> (double precision float=w671:dbl)
                n258 = Divide(x=w671, y=w677) -> (x/y=w675:dbl)
                n259 = property on="X mm/rev" class="DigNum (strict)"() -> ("Value"=w674:dbl)  [unwired: 2 in, 2 out]
                n260 = property on="X offset mm" class="DigNum (strict)"() -> ("Value"=w672:dbl)  [unwired: 2 in, 2 out]
                n261 = Multiply(x=w675, y=w674) -> (x*y=w673:dbl)
                n262 = Add(x=w673, y=w672) -> (x+y=w670:dbl)
                n263 = property on="X Position mm PV" class="DigNum (strict)"("Val(Sgnl)"=w670) -> ()  [unwired: 2 in, 2 out]
                n264 = property on="X  in Range" class="Bool (strict)"("Val(Sgnl)"=w667) -> ()  [unwired: 2 in, 2 out]
              }
            }
            n265 = flat-sequence {
              tunnel: [w599] -> w555
              tunnel: [w598] -> w554
              tunnel: w553 -> [w597]
              tunnel: w552 -> [w596]
              frame #0 {
                n266 = property on="Z Step SP" class="DigNum (strict)"() -> ("Maximum"=w613:dbl)  [unwired: 2 in, 2 out]
                n267 = property on="Z Step SP" class="DigNum (strict)"() -> ("Minimum"=w615:dbl)  [unwired: 2 in, 2 out]
                n268 = property on="Z steps/rev" class="DigNum (strict)"() -> ("Value"=w610:u32)  [unwired: 2 in, 2 out]
                n269 = To Long Integer(number=w613) -> (32bit integer=w612:i32)
                n270 = To Long Integer(number=w615) -> (32bit integer=w614:i32)
                n271 = To Double Precision Float(number=w610) -> (double precision float=w611:dbl)
                n272 = call "mdrive send command.vi"("error in (no error)"=w596, "Extra"="P", "Command"=T10."Print Parameter", "VISA resource name"=w597) -> ("error out"=w598:errorcluster, "read buffer"=w617:string, "VISA resource name out"=w599:refnum<visa-resource-name>)  [unwired: 3 in]
                n273 = Decimal String To Number(string=w617, offset=0) -> (number=w600:i32)  [unwired: 1 in, 1 out]
                n274 = property on="Z Step PV" class="DigNum (strict)"("Val(Sgnl)"=w600) -> ()  [unwired: 2 in, 2 out]
                n275 = In Range and Coerce(upper limit=w612, x=w600, lower limit=w614) -> (In Range?=w601:bool)  [unwired: 1 out]
                n276 = To Double Precision Float(number=w600) -> (double precision float=w605:dbl)
                n277 = Divide(x=w605, y=w611) -> (x/y=w609:dbl)
                n278 = property on="Z mm/rev" class="DigNum (strict)"() -> ("Value"=w608:dbl)  [unwired: 2 in, 2 out]
                n279 = property on="Z offset mm" class="DigNum (strict)"() -> ("Value"=w606:dbl)  [unwired: 2 in, 2 out]
                n280 = Multiply(x=w609, y=w608) -> (x*y=w607:dbl)
                n281 = Add(x=w607, y=w606) -> (x+y=w604:dbl)
                n282 = property on="Z Position mm PV" class="DigNum (strict)"("Val(Sgnl)"=w604) -> ()  [unwired: 2 in, 2 out]
                n283 = property on="Z in Range" class="Bool (strict)"("Val(Sgnl)"=w601) -> ()  [unwired: 2 in, 2 out]
              }
            }
            n284 = flat-sequence {
              tunnel: [w643] -> w560
              tunnel: w562 -> [w642]
              tunnel: [w641] -> w561
              tunnel: w563 -> [w640]
              frame #0 {
                n285 = property on="R Step SP" class="DigNum (strict)"() -> ("Maximum"=w657:dbl)  [unwired: 2 in, 2 out]
                n286 = property on="R Step SP" class="DigNum (strict)"() -> ("Minimum"=w659:dbl)  [unwired: 2 in, 2 out]
                n287 = property on="R steps/rev" class="DigNum (strict)"() -> ("Value"=w654:u32)  [unwired: 2 in, 2 out]
                n288 = property on="R deg/rev" class="DigNum (strict)"() -> ("Value"=w652:dbl)  [unwired: 2 in, 2 out]
                n289 = To Long Integer(number=w657) -> (32bit integer=w656:i32)
                n290 = To Long Integer(number=w659) -> (32bit integer=w658:i32)
                n291 = To Double Precision Float(number=w654) -> (double precision float=w655:dbl)
                n292 = call "mdrive send command.vi"("error in (no error)"=w640, "Extra"="P", "Command"=T10."Print Parameter", "VISA resource name"=w642) -> ("error out"=w641:errorcluster, "read buffer"=w661:string, "VISA resource name out"=w643:refnum<visa-resource-name>)  [unwired: 3 in]
                n293 = Decimal String To Number(string=w661, offset=0) -> (number=w644:i32)  [unwired: 1 in, 1 out]
                n294 = In Range and Coerce(upper limit=w656, x=w644, lower limit=w658) -> (In Range?=w645:bool)  [unwired: 1 out]
                n295 = To Double Precision Float(number=w644) -> (double precision float=w649:dbl)
                n296 = Divide(x=w649, y=w655) -> (x/y=w653:dbl)
                n297 = property on="R offset deg" class="DigNum (strict)"() -> ("Value"=w650:dbl)  [unwired: 2 in, 2 out]
                n298 = Multiply(x=w653, y=w652) -> (x*y=w651:dbl)
                n299 = Add(x=w651, y=w650) -> (x+y=w648:dbl)
                n300 = property on="R Position deg PV" class="DigNum (strict)"("Val(Sgnl)"=w648) -> ()  [unwired: 2 in, 2 out]
                n301 = property on="R in Range" class="Bool (strict)"("Val(Sgnl)"=w645) -> ()  [unwired: 2 in, 2 out]
                n302 = property on="R Step PV" class="DigNum (strict)"("Val(Sgnl)"=w644) -> ()  [unwired: 2 in, 2 out]
              }
            }
            n303 = call "mdrive send command.vi"("error in (no error)"=w561, "Extra"="MV", "Command"=T10."Print Parameter", "VISA resource name"=w560) -> ("error out"=w573:errorcluster, "read buffer"=w582:string, "VISA resource name out"=w574:refnum<visa-resource-name>)  [unwired: 3 in]
            n304 = call "mdrive send command.vi"("error in (no error)"=w559, "Extra"="MV", "Command"=T10."Print Parameter", "VISA resource name"=w558) -> ("error out"=w575:errorcluster, "read buffer"=w586:string, "VISA resource name out"=w576:refnum<visa-resource-name>)  [unwired: 3 in]
            n305 = Not Equal?(x=w582, y="") -> (x != y?=w569:bool)
            n306 = Not Equal?(x=w586, y="") -> (x != y?=w570:bool)
            n307 = property on="R Ready" class="Bool (strict)"("Val(Sgnl)"=w569) -> ()  [unwired: 2 in, 2 out]
            n308 = property on="Y Ready" class="Bool (strict)"("Val(Sgnl)"=w570) -> ()  [unwired: 2 in, 2 out]
            n309 = call "mdrive send command.vi"("error in (no error)"=w554, "Extra"="MV", "Command"=T10."Print Parameter", "VISA resource name"=w555) -> ("error out"=w577:errorcluster, "read buffer"=w590:string, "VISA resource name out"=w578:refnum<visa-resource-name>)  [unwired: 3 in]
            n310 = Not Equal?(x=w590, y="") -> (x != y?=w571:bool)
            n311 = call "DigitalIO_sub_V1_MON.vi"() -> ("CL"=w567:bool, "OP"=w568:bool)  [unwired: 8 in]
            n312 = property on="Z Ready" class="Bool (strict)"("Val(Sgnl)"=w571) -> ()  [unwired: 2 in, 2 out]
            n313 = property on="OP" class="Bool (strict)"("Val(Sgnl)"=w568) -> ()  [unwired: 2 in, 2 out]
            n314 = property on="CL" class="Bool (strict)"("Val(Sgnl)"=w567) -> ()  [unwired: 2 in, 2 out]
            n315 = call "mdrive send command.vi"("error in (no error)"=w565, "Extra"="MV", "Command"=T10."Print Parameter", "VISA resource name"=w551) -> ("error out"=w579:errorcluster, "read buffer"=w594:string, "VISA resource name out"=w580:refnum<visa-resource-name>)  [unwired: 3 in]
            n316 = Not Equal?(x=w594, y="") -> (x != y?=w572:bool)
            n317 = property on="X Ready" class="Bool (strict)"("Val(Sgnl)"=w572) -> ()  [unwired: 2 in, 2 out]
          }
          frame #1 {
            n318 = flat-sequence {
              tunnel: [w1219] -> w762
              tunnel: [w1218] -> w761
              tunnel: [w1217] -> w760
              tunnel: w698 -> [w1216]
              tunnel: w697 -> [w1215]
              tunnel: [w1241] -> w759
              tunnel: [w1240] -> w758
              tunnel: [w1238] -> w757
              tunnel: [w1239] -> w756
              tunnel: w762 -> [w1238]
              tunnel: w761 -> [w1237]
              tunnel: w760 -> [w1236]
              tunnel: w759 -> [w1255]
              tunnel: [w1255] -> w755
              tunnel: w758 -> [w1254]
              tunnel: [w1254] -> w754
              tunnel: w757 -> [w1253]
              tunnel: [w1253] -> w753
              tunnel: w756 -> [w1252]
              tunnel: [w1252] -> w752
              tunnel: [w1259] -> w751
              tunnel: [w1260] -> w750
              tunnel: [w1256] -> w749
              tunnel: w752 -> [w1256]
              tunnel: w753 -> [w1257]
              tunnel: w754 -> [w1261]
              tunnel: w755 -> [w1258]
              tunnel: w751 -> [w1271]
              tunnel: w750 -> [w1272]
              tunnel: w749 -> [w1274]
              tunnel: [w1270] -> w705
              tunnel: [w1269] -> w706
              frame #0 {
                n319 = property on="X Step SP" class="DigNum (strict)"() -> ("Maximum"=w1231:dbl)  [unwired: 2 in, 2 out]
                n320 = property on="X Step SP" class="DigNum (strict)"() -> ("Minimum"=w1233:dbl)  [unwired: 2 in, 2 out]
                n321 = property on="X steps/rev" class="DigNum (strict)"() -> ("Value"=w1228:u32)  [unwired: 2 in, 2 out]
                n322 = property on="X offset mm" class="DigNum (strict)"() -> ("Value"=w1224:dbl)  [unwired: 2 in, 2 out]
                n323 = To Long Integer(number=w1231) -> (32bit integer=w1230:i32)
                n324 = To Long Integer(number=w1233) -> (32bit integer=w1232:i32)
                n325 = To Double Precision Float(number=w1228) -> (double precision float=w1229:dbl)
                n326 = call "mdrive send command.vi"("error in (no error)"=w1215, "Extra"="P", "Command"=T10."Print Parameter", "VISA resource name"=w1216) -> ("error out"=w1217:errorcluster, "read buffer"=w1235:string, "VISA resource name out"=w1218:refnum<visa-resource-name>)  [unwired: 3 in]
                n327 = Decimal String To Number(string=w1235, offset=0) -> (number=w1214:i32)  [unwired: 1 in, 1 out]
                n328 = property on="X Step PV" class="DigNum (strict)"("Val(Sgnl)"=w1214) -> ()  [unwired: 2 in, 2 out]
                n329 = In Range and Coerce(upper limit=w1230, x=w1214, lower limit=w1232) -> (In Range?=w1219:bool)  [unwired: 1 out]
                n330 = To Double Precision Float(number=w1214) -> (double precision float=w1223:dbl)
                n331 = property on="X  in Range" class="Bool (strict)"("Val(Sgnl)"=w1219) -> ()  [unwired: 2 in, 2 out]
                n332 = Divide(x=w1223, y=w1229) -> (x/y=w1227:dbl)
                n333 = property on="X mm/rev" class="DigNum (strict)"() -> ("Value"=w1226:dbl)  [unwired: 2 in, 2 out]
                n334 = Multiply(x=w1227, y=w1226) -> (x*y=w1225:dbl)
                n335 = Add(x=w1225, y=w1224) -> (x+y=w1222:dbl)
                n336 = property on="X Position mm PV" class="DigNum (strict)"("Val(Sgnl)"=w1222) -> ()  [unwired: 2 in, 2 out]
              }
              frame #1 {
                n337 = call "mdrive send command.vi"("error in (no error)"=w1236, "Extra"="MV", "Command"=T10."Print Parameter", "VISA resource name"=w1237) -> ("error out"=w1240:errorcluster, "read buffer"=w1244:string, "VISA resource name out"=w1241:refnum<visa-resource-name>)  [unwired: 3 in]
                n338 = Decimal String To Number(string=w1244, offset=0 ("offset (0)")) -> (number=w1247:i32)  [unwired: 1 in, 1 out]
                n339 = Not Equal?(x=w1244, y="") -> (x != y?=w1242:bool)
                n340 = property on="X Ready" class="Bool (strict)"("Val(Sgnl)"=w1242) -> ()  [unwired: 2 in, 2 out]
                n341 = Number To Boolean Array(number=w1247) -> (Boolean array=w1246:bool[])
                n342 = Index Array(array=w1246, index=0) -> (element=w1239:bool)
                n343 = property on="X  in Motion" class="Bool (strict)"("Val(Sgnl)"=w1239) -> ()  [unwired: 2 in, 2 out]
              }
              frame #2 {
                n344 = Wait (ms)(milliseconds to wait=u32 50) -> ()  [unwired: 1 out]
              }
              frame #3 {
                n345 = case shown="True" w1257 {
                  tunnel: w1258 -> [w1264 w1268]
                  tunnel: [w1265 w1268] -> w1259
                  tunnel: [w1266 w1267] -> w1260
                  tunnel: w1261 -> [w1263 w1267]
                  frame #0 {
                    n346 = call "mdrive send command.vi"("error in (no error)"=w1263, "Command"=T10."Stop", "VISA resource name"=w1264) -> ("error out"=w1266:errorcluster, "VISA resource name out"=w1265:refnum<visa-resource-name>)  [unwired: 4 in, 1 out]
                  }
                  frame #1 {
                  }
                }
              }
              frame #4 {
                n347 = property on="X Backlash corr" class="Bool (strict)"() -> ("Value"=w1275:bool)  [unwired: 2 in, 2 out]
                n348 = Implies(1:w1274, 2:w1275) -> (0:w1273:bool)
                n349 = case shown="False" w1273 {
                  tunnel: w1272 -> [w1283 w1340]
                  tunnel: w1271 -> [w1282 w1341]
                  tunnel: [w1277 w1340] -> w1270
                  tunnel: [w1281 w1341] -> w1269
                  frame #0 {
                    # "Backlash"
                    n350 = flat-sequence {
                      tunnel: [w1298] -> w1295
                      tunnel: [w1300] -> w1294
                      tunnel: [w1299] -> w1293
                      tunnel: w1283 -> [w1297]
                      tunnel: w1282 -> [w1296]
                      tunnel: w1295 -> [w1308]
                      tunnel: [w1308] -> w1292
                      tunnel: w1294 -> [w1307]
                      tunnel: w1293 -> [w1306]
                      tunnel: [w1305] -> w1291
                      tunnel: [w1304] -> w1290
                      tunnel: [w1303] -> w1280
                      tunnel: w1292 -> [w1322]
                      tunnel: w1291 -> [w1313]
                      tunnel: w1290 -> [w1321]
                      tunnel: [w1313] -> w1289
                      tunnel: [w1321] -> w1288
                      tunnel: [w1312] -> w1285
                      tunnel: [w1320] -> w1284
                      tunnel: w1280 -> [w1320]
                      tunnel: w1289 -> [w1325]
                      tunnel: w1288 -> [w1326]
                      tunnel: [w1324] -> w1287
                      tunnel: [w1332] -> w1286
                      tunnel: w1285 -> [w1332]
                      tunnel: w1284 -> [w1328]
                      tunnel: [w1327] -> w1278
                      tunnel: w1287 -> [w1335]
                      tunnel: w1286 -> [w1334]
                      tunnel: [w1336] -> w1279
                      tunnel: w1278 -> [w1336]
                      tunnel: [w1335] -> w1276
                      tunnel: [w1339] -> w1281
                      tunnel: w1279 -> [w1339]
                      tunnel: [w1337] -> w1277
                      tunnel: w1276 -> [w1337]
                      frame #0 {
                        n351 = property on="X Backlash steps/sec" class="DigNum (strict)"() -> ("Value"=w1298:i32)  [unwired: 2 in, 2 out]
                        n352 = Number To Decimal String(number=w1298) -> (decimal integer string=w1301:string)  [unwired: 1 in]
                        n353 = call "mdrive send command.vi"("error in (no error)"=w1297, "Extra"=w1301, "Command"=T10."Max Velocity", "VISA resource name"=w1296) -> ("error out"=w1299:errorcluster, "VISA resource name out"=w1300:refnum<visa-resource-name>)  [unwired: 3 in, 1 out]
                      }
                      frame #1 {
                        n354 = property on="X Backlash" class="DigNum (strict)"() -> ("Value"=w1303:i32)  [unwired: 2 in, 2 out]
                        n355 = Number To Decimal String(number=w1303) -> (decimal integer string=w1309:string)  [unwired: 1 in]
                        n356 = call "mdrive send command.vi"("error in (no error)"=w1306, "Extra"=w1309, "Command"=T10."Move to Relative Position", "VISA resource name"=w1307) -> ("error out"=w1305:errorcluster, "VISA resource name out"=w1304:refnum<visa-resource-name>)  [unwired: 3 in, 1 out]
                      }
                      frame #2 {
                        n357 = To Double Precision Float(number=w1320) -> (double precision float=w1318:dbl)
                        n358 = To Double Precision Float(number=w1322) -> (double precision float=w1323:dbl)
                        n359 = Absolute Value(x=w1318) -> (abs(x)=w1319:dbl)
                        n360 = Divide(x=w1319, y=w1323) -> (x/y=w1316:dbl)
                        n361 = Multiply(x=1000.0, y=w1316) -> (x*y=w1314:dbl)
                        n362 = Add(x=w1314, y=300.0) -> (x+y=w1312:dbl)
                        n363 = To Unsigned Long Integer(number=w1312) -> (unsigned 32bit integer=w1311:u32)
                        n364 = Wait (ms)(milliseconds to wait=w1311) -> ()  [unwired: 1 out]
                      }
                      frame #3 {
                        n365 = Negate(x=w1328) -> (-x=w1329:i32)
                        n366 = Number To Decimal String(number=w1329) -> (decimal integer string=w1330:string)  [unwired: 1 in]
                        n367 = call "mdrive send command.vi"("error in (no error)"=w1325, "Extra"=w1330, "Command"=T10."Move to Relative Position", "VISA resource name"=w1326) -> ("error out"=w1324:errorcluster, "VISA resource name out"=w1327:refnum<visa-resource-name>)  [unwired: 3 in, 1 out]
                      }
                      frame #4 {
                        n368 = To Unsigned Long Integer(number=w1334) -> (unsigned 32bit integer=w1333:u32)
                        n369 = Wait (ms)(milliseconds to wait=w1333) -> ()  [unwired: 1 out]
                      }
                      frame #5 {
                        n370 = property on="X Backlash corr" class="Bool (strict)"("Val(Sgnl)"=FALSE ("Value (Signaling)")) -> ()  [unwired: 2 in, 2 out]
                      }
                    }
                  }
                  frame #1 {
                  }
                }
              }
            }
            n371 = flat-sequence {
              tunnel: [w1085] -> w748
              tunnel: [w1076] -> w747
              tunnel: [w1075] -> w746
              tunnel: w696 -> [w1079]
              tunnel: w695 -> [w1078]
              tunnel: [w1117] -> w745
              tunnel: [w1116] -> w744
              tunnel: [w1115] -> w743
              tunnel: [w1108] -> w742
              tunnel: w748 -> [w1115]
              tunnel: w747 -> [w1114]
              tunnel: w746 -> [w1113]
              tunnel: w745 -> [w1127]
              tunnel: [w1127] -> w741
              tunnel: w744 -> [w1126]
              tunnel: [w1126] -> w740
              tunnel: w743 -> [w1125]
              tunnel: [w1125] -> w739
              tunnel: w742 -> [w1124]
              tunnel: [w1124] -> w738
              tunnel: [w1131] -> w737
              tunnel: [w1132] -> w736
              tunnel: [w1128] -> w735
              tunnel: w738 -> [w1128]
              tunnel: w739 -> [w1129]
              tunnel: w740 -> [w1133]
              tunnel: w741 -> [w1130]
              tunnel: w737 -> [w1144]
              tunnel: w736 -> [w1145]
              tunnel: w735 -> [w1147]
              tunnel: [w1143] -> w703
              tunnel: [w1142] -> w704
              frame #0 {
                n372 = property on="Z Step SP" class="DigNum (strict)"() -> ("Maximum"=w1086:dbl)  [unwired: 2 in, 2 out]
                n373 = property on="Z Step SP" class="DigNum (strict)"() -> ("Minimum"=w1080:dbl)  [unwired: 2 in, 2 out]
                n374 = property on="OK Button" class="Bool (strict)"() -> ("Value"=w1071:bool)  [unwired: 2 in, 2 out]
                n375 = property on="Z steps/rev" class="DigNum (strict)"() -> ("Value"=w1084:u32)  [unwired: 2 in, 2 out]
                n376 = To Double Precision Float(number=w1084) -> (double precision float=w1091:dbl)
                n377 = To Long Integer(number=w1086) -> (32bit integer=w1092:i32)
                n378 = To Long Integer(number=w1080) -> (32bit integer=w1093:i32)
                n379 = property on="Z offset mm" class="DigNum (strict)"() -> ("Value"=w1082:dbl)  [unwired: 2 in, 2 out]
                n380 = Not Equal?(x=w1071, y=TRUE) -> (x != y?=w1069:bool)
                n381 = call "mdrive send command.vi"("error in (no error)"=w1078, "Extra"="P", "Command"=T10."Print Parameter", "VISA resource name"=w1079) -> ("error out"=w1075:errorcluster, "read buffer"=w1095:string, "VISA resource name out"=w1076:refnum<visa-resource-name>)  [unwired: 3 in]
                n382 = Decimal String To Number(string=w1095, offset=0) -> (number=w1074:i32)  [unwired: 1 in, 1 out]
                n383 = property on="Z Step PV" class="DigNum (strict)"("Val(Sgnl)"=w1074) -> ()  [unwired: 2 in, 2 out]
                n384 = Equal?(x=w1074, y=15360000) -> (x = y?=w1068:bool)
                n385 = To Double Precision Float(number=w1074) -> (double precision float=w1089:dbl)
                n386 = In Range and Coerce(upper limit=w1092, x=w1074, lower limit=w1093) -> (In Range?=w1085:bool)  [unwired: 1 out]
                n387 = property on="Z in Range" class="Bool (strict)"("Val(Sgnl)"=w1085) -> ()  [unwired: 2 in, 2 out]
                n388 = Divide(x=w1089, y=w1091) -> (x/y=w1090:dbl)
                n389 = And(x=w1068, y=w1069) -> (x .and. y?=w1067:bool)
                n390 = case shown="True" w1067 {
                  tunnel: [FALSE ("true") w1106] -> w1072
                  frame #0 {
                  }
                  frame #1 {
                    n391 = One Button Dialog(message="HAVE YOU OPEND THE VALVE???\nTHEN REWRITE YOUR POSITION\n AND PRESS GO!") -> (true=w1106:bool)  [unwired: 1 in]
                  }
                }
                n392 = property on="Z mm/rev" class="DigNum (strict)"() -> ("Value"=w1083:dbl)  [unwired: 2 in, 2 out]
                n393 = Multiply(x=w1090, y=w1083) -> (x*y=w1077:dbl)
                n394 = Add(x=w1077, y=w1082) -> (x+y=w1081:dbl)
                n395 = property on="Z Position mm PV" class="DigNum (strict)"("Val(Sgnl)"=w1081) -> ()  [unwired: 2 in, 2 out]
                n396 = case shown="True" w1072 {
                  frame #0 {
                    n397 = call "DigitalIO_sub_V1_MON.vi"() -> ("CL"=w1096:bool, "OP"=w1097:bool)  [unwired: 8 in]
                    n398 = property on="OP" class="Bool (strict)"("Val(Sgnl)"=w1097) -> ()  [unwired: 2 in, 2 out]
                    n399 = property on="CL" class="Bool (strict)"("Val(Sgnl)"=w1096) -> ()  [unwired: 2 in, 2 out]
                  }
                  frame #1 {
                    n400 = while {
                      stop <- w1104 stop-if-true
                      n401 = property on="OK Button" class="Bool (strict)"() -> ("Value"=w1098:bool)  [unwired: 2 in, 2 out]
                      n402 = call "ValveConrtoller.vi"("OK Button"=w1098) -> ("OUTGOING SIGNAL"=w1099:bool, "CL"=w1100:bool, "OP"=w1101:bool, "VALVE\nopend/closed"=w1102:bool)  [unwired: 3 in]
                      n403 = property on="OP" class="Bool (strict)"("Val(Sgnl)"=w1101) -> ()  [unwired: 2 in, 2 out]
                      n404 = property on="CL" class="Bool (strict)"("Val(Sgnl)"=w1100) -> ()  [unwired: 2 in, 2 out]
                      n405 = property on="Valve \nopend/closed" class="Bool (strict)"("Val(Sgnl)"=w1102) -> ()  [unwired: 2 in, 2 out]
                      n406 = Equal?(x=w1099, y=TRUE) -> (x = y?=w1104:bool)
                    }
                  }
                }
              }
              frame #1 {
                n407 = call "mdrive send command.vi"("error in (no error)"=w1113, "Extra"="MV", "Command"=T10."Print Parameter", "VISA resource name"=w1114) -> ("error out"=w1116:errorcluster, "read buffer"=w1119:string, "VISA resource name out"=w1117:refnum<visa-resource-name>)  [unwired: 3 in]
                n408 = Decimal String To Number(string=w1119, offset=0 ("offset (0)")) -> (number=w1109:i32)  [unwired: 1 in, 1 out]
                n409 = Not Equal?(x=w1119, y="") -> (x != y?=w1112:bool)
                n410 = property on="Z Ready" class="Bool (strict)"("Val(Sgnl)"=w1112) -> ()  [unwired: 2 in, 2 out]
                n411 = Number To Boolean Array(number=w1109) -> (Boolean array=w1111:bool[])
                n412 = Index Array(array=w1111, index=0) -> (element=w1108:bool)
                n413 = property on="Z in Motion" class="Bool (strict)"("Val(Sgnl)"=w1108) -> ()  [unwired: 2 in, 2 out]
              }
              frame #2 {
                n414 = Wait (ms)(milliseconds to wait=u32 50) -> ()  [unwired: 1 out]
              }
              frame #3 {
                n415 = case shown="False" w1129 {
                  tunnel: w1130 -> [w1136 w1140]
                  tunnel: [w1137 w1140] -> w1131
                  tunnel: [w1138 w1139] -> w1132
                  tunnel: w1133 -> [w1135 w1139]
                  frame #0 {
                    n416 = call "mdrive send command.vi"("error in (no error)"=w1135, "Command"=T10."Stop", "VISA resource name"=w1136) -> ("error out"=w1138:errorcluster, "VISA resource name out"=w1137:refnum<visa-resource-name>)  [unwired: 4 in, 1 out]
                  }
                  frame #1 {
                  }
                }
              }
              frame #4 {
                n417 = property on="Z Backlash corr" class="Bool (strict)"() -> ("Value"=w1141:bool)  [unwired: 2 in, 2 out]
                n418 = Implies(1:w1147, 2:w1141) -> (0:w1146:bool)
                n419 = case shown="False" w1146 {
                  tunnel: w1145 -> [w1155 w1212]
                  tunnel: w1144 -> [w1154 w1213]
                  tunnel: [w1149 w1212] -> w1143
                  tunnel: [w1153 w1213] -> w1142
                  frame #0 {
                    # "Backlash"
                    n420 = flat-sequence {
                      tunnel: [w1168] -> w1167
                      tunnel: [w1172] -> w1166
                      tunnel: [w1171] -> w1165
                      tunnel: w1155 -> [w1170]
                      tunnel: w1154 -> [w1169]
                      tunnel: w1167 -> [w1180]
                      tunnel: [w1180] -> w1164
                      tunnel: w1166 -> [w1179]
                      tunnel: w1165 -> [w1178]
                      tunnel: [w1177] -> w1163
                      tunnel: [w1176] -> w1162
                      tunnel: [w1175] -> w1152
                      tunnel: w1164 -> [w1194]
                      tunnel: w1163 -> [w1185]
                      tunnel: w1162 -> [w1193]
                      tunnel: [w1185] -> w1161
                      tunnel: [w1193] -> w1160
                      tunnel: [w1184] -> w1157
                      tunnel: [w1192] -> w1156
                      tunnel: w1152 -> [w1192]
                      tunnel: w1161 -> [w1197]
                      tunnel: w1160 -> [w1198]
                      tunnel: [w1196] -> w1159
                      tunnel: [w1204] -> w1158
                      tunnel: w1157 -> [w1204]
                      tunnel: w1156 -> [w1200]
                      tunnel: [w1199] -> w1150
                      tunnel: w1159 -> [w1207]
                      tunnel: w1158 -> [w1206]
                      tunnel: [w1208] -> w1151
                      tunnel: w1150 -> [w1208]
                      tunnel: [w1207] -> w1148
                      tunnel: [w1211] -> w1153
                      tunnel: w1151 -> [w1211]
                      tunnel: [w1210] -> w1149
                      tunnel: w1148 -> [w1210]
                      frame #0 {
                        n421 = property on="Z Backlash steps/sec" class="DigNum (strict)"() -> ("Value"=w1168:i32)  [unwired: 2 in, 2 out]
                        n422 = Number To Decimal String(number=w1168) -> (decimal integer string=w1173:string)  [unwired: 1 in]
                        n423 = call "mdrive send command.vi"("error in (no error)"=w1170, "Extra"=w1173, "Command"=T10."Max Velocity", "VISA resource name"=w1169) -> ("error out"=w1171:errorcluster, "VISA resource name out"=w1172:refnum<visa-resource-name>)  [unwired: 3 in, 1 out]
                      }
                      frame #1 {
                        n424 = property on="Z Backlash" class="DigNum (strict)"() -> ("Value"=w1175:i32)  [unwired: 2 in, 2 out]
                        n425 = Number To Decimal String(number=w1175) -> (decimal integer string=w1181:string)  [unwired: 1 in]
                        n426 = call "mdrive send command.vi"("error in (no error)"=w1178, "Extra"=w1181, "Command"=T10."Move to Relative Position", "VISA resource name"=w1179) -> ("error out"=w1177:errorcluster, "VISA resource name out"=w1176:refnum<visa-resource-name>)  [unwired: 3 in, 1 out]
                      }
                      frame #2 {
                        n427 = To Double Precision Float(number=w1192) -> (double precision float=w1190:dbl)
                        n428 = To Double Precision Float(number=w1194) -> (double precision float=w1195:dbl)
                        n429 = Absolute Value(x=w1190) -> (abs(x)=w1191:dbl)
                        n430 = Divide(x=w1191, y=w1195) -> (x/y=w1188:dbl)
                        n431 = Multiply(x=1000.0, y=w1188) -> (x*y=w1186:dbl)
                        n432 = Add(x=w1186, y=300.0) -> (x+y=w1184:dbl)
                        n433 = To Unsigned Long Integer(number=w1184) -> (unsigned 32bit integer=w1183:u32)
                        n434 = Wait (ms)(milliseconds to wait=w1183) -> ()  [unwired: 1 out]
                      }
                      frame #3 {
                        n435 = Negate(x=w1200) -> (-x=w1201:i32)
                        n436 = Number To Decimal String(number=w1201) -> (decimal integer string=w1202:string)  [unwired: 1 in]
                        n437 = call "mdrive send command.vi"("error in (no error)"=w1197, "Extra"=w1202, "Command"=T10."Move to Relative Position", "VISA resource name"=w1198) -> ("error out"=w1196:errorcluster, "VISA resource name out"=w1199:refnum<visa-resource-name>)  [unwired: 3 in, 1 out]
                      }
                      frame #4 {
                        n438 = To Unsigned Long Integer(number=w1206) -> (unsigned 32bit integer=w1205:u32)
                        n439 = Wait (ms)(milliseconds to wait=w1205) -> ()  [unwired: 1 out]
                      }
                      frame #5 {
                        n440 = property on="Z Backlash corr" class="Bool (strict)"("Val(Sgnl)"=FALSE ("Value (Signaling)")) -> ()  [unwired: 2 in, 2 out]
                      }
                    }
                  }
                  frame #1 {
                  }
                }
              }
            }
            n441 = flat-sequence {
              tunnel: [w948] -> w734
              tunnel: [w950] -> w733
              tunnel: [w949] -> w732
              tunnel: w694 -> [w941]
              tunnel: w693 -> [w940]
              tunnel: [w970] -> w731
              tunnel: [w969] -> w730
              tunnel: [w968] -> w729
              tunnel: [w961] -> w728
              tunnel: w734 -> [w968]
              tunnel: w733 -> [w967]
              tunnel: w732 -> [w966]
              tunnel: w731 -> [w980]
              tunnel: [w980] -> w727
              tunnel: w730 -> [w979]
              tunnel: [w979] -> w726
              tunnel: w729 -> [w978]
              tunnel: [w978] -> w725
              tunnel: w728 -> [w977]
              tunnel: [w977] -> w724
              tunnel: [w984] -> w723
              tunnel: [w985] -> w722
              tunnel: [w981] -> w721
              tunnel: w724 -> [w981]
              tunnel: w725 -> [w982]
              tunnel: w726 -> [w986]
              tunnel: w727 -> [w983]
              tunnel: w723 -> [w997]
              tunnel: w722 -> [w998]
              tunnel: w721 -> [w1000]
              tunnel: [w996] -> w701
              tunnel: [w995] -> w702
              frame #0 {
                n442 = property on="Y Step SP" class="DigNum (strict)"() -> ("Maximum"=w943:dbl)  [unwired: 2 in, 2 out]
                n443 = property on="Y Step SP" class="DigNum (strict)"() -> ("Minimum"=w942:dbl)  [unwired: 2 in, 2 out]
                n444 = property on="Y steps/rev" class="DigNum (strict)"() -> ("Value"=w944:u32)  [unwired: 2 in, 2 out]
                n445 = property on="Y offset mm" class="DigNum (strict)"() -> ("Value"=w946:dbl)  [unwired: 2 in, 2 out]
                n446 = To Long Integer(number=w943) -> (32bit integer=w957:i32)
                n447 = To Long Integer(number=w942) -> (32bit integer=w958:i32)
                n448 = To Double Precision Float(number=w944) -> (double precision float=w956:dbl)
                n449 = call "mdrive send command.vi"("error in (no error)"=w940, "Extra"="P", "Command"=T10."Print Parameter", "VISA resource name"=w941) -> ("error out"=w949:errorcluster, "read buffer"=w960:string, "VISA resource name out"=w950:refnum<visa-resource-name>)  [unwired: 3 in]
                n450 = Decimal String To Number(string=w960, offset=0) -> (number=w939:i32)  [unwired: 1 in, 1 out]
                n451 = property on="Y Step PV" class="DigNum (strict)"("Val(Sgnl)"=w939) -> ()  [unwired: 2 in, 2 out]
                n452 = In Range and Coerce(upper limit=w957, x=w939, lower limit=w958) -> (In Range?=w948:bool)  [unwired: 1 out]
                n453 = To Double Precision Float(number=w939) -> (double precision float=w953:dbl)
                n454 = property on="Y in Range" class="Bool (strict)"("Val(Sgnl)"=w948) -> ()  [unwired: 2 in, 2 out]
                n455 = Divide(x=w953, y=w956) -> (x/y=w955:dbl)
                n456 = property on="Y mm/rev" class="DigNum (strict)"() -> ("Value"=w945:dbl)  [unwired: 2 in, 2 out]
                n457 = Multiply(x=w955, y=w945) -> (x*y=w954:dbl)
                n458 = Add(x=w954, y=w946) -> (x+y=w947:dbl)
                n459 = property on="Y Position mm PV" class="DigNum (strict)"("Val(Sgnl)"=w947) -> ()  [unwired: 2 in, 2 out]
              }
              frame #1 {
                n460 = call "mdrive send command.vi"("error in (no error)"=w966, "Extra"="MV", "Command"=T10."Print Parameter", "VISA resource name"=w967) -> ("error out"=w969:errorcluster, "read buffer"=w972:string, "VISA resource name out"=w970:refnum<visa-resource-name>)  [unwired: 3 in]
                n461 = Decimal String To Number(string=w972, offset=0 ("offset (0)")) -> (number=w962:i32)  [unwired: 1 in, 1 out]
                n462 = Not Equal?(x=w972, y="") -> (x != y?=w965:bool)
                n463 = property on="Y Ready" class="Bool (strict)"("Val(Sgnl)"=w965) -> ()  [unwired: 2 in, 2 out]
                n464 = Number To Boolean Array(number=w962) -> (Boolean array=w964:bool[])
                n465 = Index Array(array=w964, index=0) -> (element=w961:bool)
                n466 = property on="Y in Motion" class="Bool (strict)"("Val(Sgnl)"=w961) -> ()  [unwired: 2 in, 2 out]
              }
              frame #2 {
                n467 = Wait (ms)(milliseconds to wait=u32 50) -> ()  [unwired: 1 out]
              }
              frame #3 {
                n468 = case shown="True" w982 {
                  tunnel: w983 -> [w989 w992]
                  tunnel: [w990 w992] -> w984
                  tunnel: [w991 w993] -> w985
                  tunnel: w986 -> [w988 w993]
                  frame #0 {
                    n469 = call "mdrive send command.vi"("error in (no error)"=w988, "Command"=T10."Stop", "VISA resource name"=w989) -> ("error out"=w991:errorcluster, "VISA resource name out"=w990:refnum<visa-resource-name>)  [unwired: 4 in, 1 out]
                  }
                  frame #1 {
                  }
                }
              }
              frame #4 {
                n470 = property on="Y Backlash corr" class="Bool (strict)"() -> ("Value"=w994:bool)  [unwired: 2 in, 2 out]
                n471 = Implies(1:w1000, 2:w994) -> (0:w999:bool)
                n472 = case shown="False" w999 {
                  tunnel: w998 -> [w1008 w1065]
                  tunnel: w997 -> [w1007 w1066]
                  tunnel: [w1002 w1065] -> w996
                  tunnel: [w1006 w1066] -> w995
                  frame #0 {
                    # "Backlash"
                    n473 = flat-sequence {
                      tunnel: [w1021] -> w1020
                      tunnel: [w1025] -> w1019
                      tunnel: [w1024] -> w1018
                      tunnel: w1008 -> [w1023]
                      tunnel: w1007 -> [w1022]
                      tunnel: w1020 -> [w1033]
                      tunnel: [w1033] -> w1017
                      tunnel: w1019 -> [w1032]
                      tunnel: w1018 -> [w1031]
                      tunnel: [w1030] -> w1016
                      tunnel: [w1029] -> w1015
                      tunnel: [w1028] -> w1005
                      tunnel: w1017 -> [w1047]
                      tunnel: w1016 -> [w1038]
                      tunnel: w1015 -> [w1046]
                      tunnel: [w1038] -> w1014
                      tunnel: [w1046] -> w1013
                      tunnel: [w1037] -> w1010
                      tunnel: [w1045] -> w1009
                      tunnel: w1005 -> [w1045]
                      tunnel: w1014 -> [w1050]
                      tunnel: w1013 -> [w1051]
                      tunnel: [w1049] -> w1012
                      tunnel: [w1057] -> w1011
                      tunnel: w1010 -> [w1057]
                      tunnel: w1009 -> [w1053]
                      tunnel: [w1052] -> w1003
                      tunnel: w1012 -> [w1060]
                      tunnel: w1011 -> [w1059]
                      tunnel: [w1061] -> w1004
                      tunnel: w1003 -> [w1061]
                      tunnel: [w1060] -> w1001
                      tunnel: [w1064] -> w1006
                      tunnel: w1004 -> [w1064]
                      tunnel: [w1063] -> w1002
                      tunnel: w1001 -> [w1063]
                      frame #0 {
                        n474 = property on="Y Backlash steps/sec" class="DigNum (strict)"() -> ("Value"=w1021:i32)  [unwired: 2 in, 2 out]
                        n475 = Number To Decimal String(number=w1021) -> (decimal integer string=w1026:string)  [unwired: 1 in]
                        n476 = call "mdrive send command.vi"("error in (no error)"=w1023, "Extra"=w1026, "Command"=T10."Max Velocity", "VISA resource name"=w1022) -> ("error out"=w1024:errorcluster, "VISA resource name out"=w1025:refnum<visa-resource-name>)  [unwired: 3 in, 1 out]
                      }
                      frame #1 {
                        n477 = property on="Y Backlash" class="DigNum (strict)"() -> ("Value"=w1028:i32)  [unwired: 2 in, 2 out]
                        n478 = Number To Decimal String(number=w1028) -> (decimal integer string=w1034:string)  [unwired: 1 in]
                        n479 = call "mdrive send command.vi"("error in (no error)"=w1031, "Extra"=w1034, "Command"=T10."Move to Relative Position", "VISA resource name"=w1032) -> ("error out"=w1030:errorcluster, "VISA resource name out"=w1029:refnum<visa-resource-name>)  [unwired: 3 in, 1 out]
                      }
                      frame #2 {
                        n480 = To Double Precision Float(number=w1045) -> (double precision float=w1043:dbl)
                        n481 = To Double Precision Float(number=w1047) -> (double precision float=w1048:dbl)
                        n482 = Absolute Value(x=w1043) -> (abs(x)=w1044:dbl)
                        n483 = Divide(x=w1044, y=w1048) -> (x/y=w1041:dbl)
                        n484 = Multiply(x=1000.0, y=w1041) -> (x*y=w1039:dbl)
                        n485 = Add(x=w1039, y=300.0) -> (x+y=w1037:dbl)
                        n486 = To Unsigned Long Integer(number=w1037) -> (unsigned 32bit integer=w1036:u32)
                        n487 = Wait (ms)(milliseconds to wait=w1036) -> ()  [unwired: 1 out]
                      }
                      frame #3 {
                        n488 = Negate(x=w1053) -> (-x=w1054:i32)
                        n489 = Number To Decimal String(number=w1054) -> (decimal integer string=w1055:string)  [unwired: 1 in]
                        n490 = call "mdrive send command.vi"("error in (no error)"=w1050, "Extra"=w1055, "Command"=T10."Move to Relative Position", "VISA resource name"=w1051) -> ("error out"=w1049:errorcluster, "VISA resource name out"=w1052:refnum<visa-resource-name>)  [unwired: 3 in, 1 out]
                      }
                      frame #4 {
                        n491 = To Unsigned Long Integer(number=w1059) -> (unsigned 32bit integer=w1058:u32)
                        n492 = Wait (ms)(milliseconds to wait=w1058) -> ()  [unwired: 1 out]
                      }
                      frame #5 {
                        n493 = property on="Y Backlash corr" class="Bool (strict)"("Val(Sgnl)"=FALSE ("Value (Signaling)")) -> ()  [unwired: 2 in, 2 out]
                      }
                    }
                  }
                  frame #1 {
                  }
                }
              }
            }
            n494 = flat-sequence {
              tunnel: [w820] -> w720
              tunnel: [w822] -> w719
              tunnel: [w821] -> w718
              tunnel: w692 -> [w813]
              tunnel: w691 -> [w812]
              tunnel: [w842] -> w717
              tunnel: [w841] -> w716
              tunnel: [w840] -> w715
              tunnel: [w833] -> w714
              tunnel: w720 -> [w840]
              tunnel: w719 -> [w839]
              tunnel: w718 -> [w838]
              tunnel: w717 -> [w852]
              tunnel: [w852] -> w713
              tunnel: w716 -> [w851]
              tunnel: [w851] -> w712
              tunnel: w715 -> [w850]
              tunnel: [w850] -> w711
              tunnel: w714 -> [w849]
              tunnel: [w849] -> w710
              tunnel: [w856] -> w709
              tunnel: [w857] -> w708
              tunnel: [w853] -> w707
              tunnel: w710 -> [w853]
              tunnel: w711 -> [w854]
              tunnel: w712 -> [w858]
              tunnel: w713 -> [w855]
              tunnel: w709 -> [w869]
              tunnel: w708 -> [w870]
              tunnel: w707 -> [w872]
              tunnel: [w868] -> w699
              tunnel: [w867] -> w700
              frame #0 {
                n495 = property on="R Step SP" class="DigNum (strict)"() -> ("Maximum"=w815:dbl)  [unwired: 2 in, 2 out]
                n496 = property on="R Step SP" class="DigNum (strict)"() -> ("Minimum"=w816:dbl)  [unwired: 2 in, 2 out]
                n497 = property on="R steps/rev" class="DigNum (strict)"() -> ("Value"=w814:u32)  [unwired: 2 in, 2 out]
                n498 = property on="R offset deg" class="DigNum (strict)"() -> ("Value"=w818:dbl)  [unwired: 2 in, 2 out]
                n499 = To Long Integer(number=w815) -> (32bit integer=w829:i32)
                n500 = To Long Integer(number=w816) -> (32bit integer=w830:i32)
                n501 = To Double Precision Float(number=w814) -> (double precision float=w828:dbl)
                n502 = call "mdrive send command.vi"("error in (no error)"=w812, "Extra"="P", "Command"=T10."Print Parameter", "VISA resource name"=w813) -> ("error out"=w821:errorcluster, "read buffer"=w832:string, "VISA resource name out"=w822:refnum<visa-resource-name>)  [unwired: 3 in]
                n503 = Decimal String To Number(string=w832, offset=0) -> (number=w811:i32)  [unwired: 1 in, 1 out]
                n504 = property on="R Step PV" class="DigNum (strict)"("Val(Sgnl)"=w811) -> ()  [unwired: 2 in, 2 out]
                n505 = In Range and Coerce(upper limit=w829, x=w811, lower limit=w830) -> (In Range?=w820:bool)  [unwired: 1 out]
                n506 = To Double Precision Float(number=w811) -> (double precision float=w825:dbl)
                n507 = property on="R in Range" class="Bool (strict)"("Val(Sgnl)"=w820) -> ()  [unwired: 2 in, 2 out]
                n508 = Divide(x=w825, y=w828) -> (x/y=w827:dbl)
                n509 = property on="R deg/rev" class="DigNum (strict)"() -> ("Value"=w817:dbl)  [unwired: 2 in, 2 out]
                n510 = Multiply(x=w827, y=w817) -> (x*y=w826:dbl)
                n511 = Add(x=w826, y=w818) -> (x+y=w819:dbl)
                n512 = property on="R Position deg PV" class="DigNum (strict)"("Val(Sgnl)"=w819) -> ()  [unwired: 2 in, 2 out]
              }
              frame #1 {
                n513 = call "mdrive send command.vi"("error in (no error)"=w838, "Extra"="MV", "Command"=T10."Print Parameter", "VISA resource name"=w839) -> ("error out"=w841:errorcluster, "read buffer"=w844:string, "VISA resource name out"=w842:refnum<visa-resource-name>)  [unwired: 3 in]
                n514 = Decimal String To Number(string=w844, offset=0 ("offset (0)")) -> (number=w834:i32)  [unwired: 1 in, 1 out]
                n515 = Not Equal?(x=w844, y="") -> (x != y?=w837:bool)
                n516 = property on="R Ready" class="Bool (strict)"("Val(Sgnl)"=w837) -> ()  [unwired: 2 in, 2 out]
                n517 = Number To Boolean Array(number=w834) -> (Boolean array=w836:bool[])
                n518 = Index Array(array=w836, index=0) -> (element=w833:bool)
                n519 = property on="R in Motion" class="Bool (strict)"("Val(Sgnl)"=w833) -> ()  [unwired: 2 in, 2 out]
              }
              frame #2 {
                n520 = Wait (ms)(milliseconds to wait=u32 50) -> ()  [unwired: 1 out]
              }
              frame #3 {
                n521 = case shown="True" w854 {
                  tunnel: w855 -> [w861 w865]
                  tunnel: [w862 w865] -> w856
                  tunnel: [w863 w864] -> w857
                  tunnel: w858 -> [w860 w864]
                  frame #0 {
                    n522 = call "mdrive send command.vi"("error in (no error)"=w860, "Command"=T10."Stop", "VISA resource name"=w861) -> ("error out"=w863:errorcluster, "VISA resource name out"=w862:refnum<visa-resource-name>)  [unwired: 4 in, 1 out]
                  }
                  frame #1 {
                  }
                }
              }
              frame #4 {
                n523 = property on="R Backlash corr" class="Bool (strict)"() -> ("Value"=w866:bool)  [unwired: 2 in, 2 out]
                n524 = Implies(1:w872, 2:w866) -> (0:w871:bool)
                n525 = case shown="False" w871 {
                  tunnel: w870 -> [w880 w937]
                  tunnel: w869 -> [w879 w938]
                  tunnel: [w874 w937] -> w868
                  tunnel: [w878 w938] -> w867
                  frame #0 {
                    # "Backlash"
                    n526 = flat-sequence {
                      tunnel: [w893] -> w892
                      tunnel: [w897] -> w891
                      tunnel: [w896] -> w890
                      tunnel: w880 -> [w895]
                      tunnel: w879 -> [w894]
                      tunnel: w892 -> [w905]
                      tunnel: [w905] -> w889
                      tunnel: w891 -> [w904]
                      tunnel: w890 -> [w903]
                      tunnel: [w902] -> w888
                      tunnel: [w901] -> w887
                      tunnel: [w900] -> w877
                      tunnel: w889 -> [w919]
                      tunnel: w888 -> [w910]
                      tunnel: w887 -> [w918]
                      tunnel: [w910] -> w886
                      tunnel: [w918] -> w885
                      tunnel: [w909] -> w882
                      tunnel: [w917] -> w881
                      tunnel: w877 -> [w917]
                      tunnel: w886 -> [w922]
                      tunnel: w885 -> [w923]
                      tunnel: [w921] -> w884
                      tunnel: [w929] -> w883
                      tunnel: w882 -> [w929]
                      tunnel: w881 -> [w925]
                      tunnel: [w924] -> w875
                      tunnel: w884 -> [w932]
                      tunnel: w883 -> [w931]
                      tunnel: [w933] -> w876
                      tunnel: w875 -> [w933]
                      tunnel: [w932] -> w873
                      tunnel: [w936] -> w878
                      tunnel: w876 -> [w936]
                      tunnel: [w935] -> w874
                      tunnel: w873 -> [w935]
                      frame #0 {
                        n527 = property on="R Backlash steps/sec" class="DigNum (strict)"() -> ("Value"=w893:i32)  [unwired: 2 in, 2 out]
                        n528 = Number To Decimal String(number=w893) -> (decimal integer string=w898:string)  [unwired: 1 in]
                        n529 = call "mdrive send command.vi"("error in (no error)"=w895, "Extra"=w898, "Command"=T10."Max Velocity", "VISA resource name"=w894) -> ("error out"=w896:errorcluster, "VISA resource name out"=w897:refnum<visa-resource-name>)  [unwired: 3 in, 1 out]
                      }
                      frame #1 {
                        n530 = property on="R Backlash" class="DigNum (strict)"() -> ("Value"=w900:i32)  [unwired: 2 in, 2 out]
                        n531 = Number To Decimal String(number=w900) -> (decimal integer string=w906:string)  [unwired: 1 in]
                        n532 = call "mdrive send command.vi"("error in (no error)"=w903, "Extra"=w906, "Command"=T10."Move to Relative Position", "VISA resource name"=w904) -> ("error out"=w902:errorcluster, "VISA resource name out"=w901:refnum<visa-resource-name>)  [unwired: 3 in, 1 out]
                      }
                      frame #2 {
                        n533 = To Double Precision Float(number=w917) -> (double precision float=w915:dbl)
                        n534 = To Double Precision Float(number=w919) -> (double precision float=w920:dbl)
                        n535 = Absolute Value(x=w915) -> (abs(x)=w916:dbl)
                        n536 = Divide(x=w916, y=w920) -> (x/y=w913:dbl)
                        n537 = Multiply(x=1000.0, y=w913) -> (x*y=w911:dbl)
                        n538 = Add(x=w911, y=300.0) -> (x+y=w909:dbl)
                        n539 = To Unsigned Long Integer(number=w909) -> (unsigned 32bit integer=w908:u32)
                        n540 = Wait (ms)(milliseconds to wait=w908) -> ()  [unwired: 1 out]
                      }
                      frame #3 {
                        n541 = Negate(x=w925) -> (-x=w926:i32)
                        n542 = Number To Decimal String(number=w926) -> (decimal integer string=w927:string)  [unwired: 1 in]
                        n543 = call "mdrive send command.vi"("error in (no error)"=w922, "Extra"=w927, "Command"=T10."Move to Relative Position", "VISA resource name"=w923) -> ("error out"=w921:errorcluster, "VISA resource name out"=w924:refnum<visa-resource-name>)  [unwired: 3 in, 1 out]
                      }
                      frame #4 {
                        n544 = To Unsigned Long Integer(number=w931) -> (unsigned 32bit integer=w930:u32)
                        n545 = Wait (ms)(milliseconds to wait=w930) -> ()  [unwired: 1 out]
                      }
                      frame #5 {
                        n546 = property on="R Backlash corr" class="Bool (strict)"("Val(Sgnl)"=FALSE ("Value (Signaling)")) -> ()  [unwired: 2 in, 2 out]
                      }
                    }
                  }
                  frame #1 {
                  }
                }
              }
            }
            n547 = property on="Scan Go" class="Bool (strict)"() -> ("Value"=w690:bool)  [unwired: 2 in, 2 out]
            n548 = Equal?(x=w690, y=TRUE) -> (x = y?=w685:bool)
            n549 = property on="STATUS" class="Str"() -> ("Value"=w688:string)  [unwired: 2 in, 2 out]
            n550 = Equal?(x=w688, y="SCANNING MODE" ("STATUS")) -> (x = y?=w686:bool)
            n551 = Or(x=w686, y=w685) -> (x .or. y?=w684:bool)
            n552 = case shown="False" w684 {
              frame #0 {
                n553 = property on="Y in Motion" class="Bool (strict)"() -> ("Value"=w766:bool)  [unwired: 2 in, 2 out]
                n554 = property on="Z in Motion" class="Bool (strict)"() -> ("Value"=w769:bool)  [unwired: 2 in, 2 out]
                n555 = property on="X  in Motion" class="Bool (strict)"() -> ("Value"=w767:bool)  [unwired: 2 in, 2 out]
                n556 = property on="R in Motion" class="Bool (strict)"() -> ("Value"=w768:bool)  [unwired: 2 in, 2 out]
                n557 = Compound Arithmetic op=AND(w767, w766, w769, w768) -> (w764:bool)
                n558 = Equal?(x=w764, y=FALSE) -> (x = y?=w765:bool)
                n559 = case shown="True" w765 {
                  frame #0 {
                  }
                  frame #1 {
                    n560 = property on="X Step SP" class="DigNum (strict)"() -> ("Value"=w777:i32)  [unwired: 2 in, 2 out]
                    n561 = property on="X Step PV" class="DigNum (strict)"() -> ("Value"=w776:i32)  [unwired: 2 in, 2 out]
                    n562 = property on="Y Step SP" class="DigNum (strict)"() -> ("Value"=w775:i32)  [unwired: 2 in, 2 out]
                    n563 = property on="Y Step PV" class="DigNum (strict)"() -> ("Value"=w774:i32)  [unwired: 2 in, 2 out]
                    n564 = property on="Z Step SP" class="DigNum (strict)"() -> ("Value"=w773:i32)  [unwired: 2 in, 2 out]
                    n565 = property on="Z Step PV" class="DigNum (strict)"() -> ("Value"=w772:i32)  [unwired: 2 in, 2 out]
                    n566 = property on="R Step SP" class="DigNum (strict)"() -> ("Value"=w770:i32)  [unwired: 2 in, 2 out]
                    n567 = property on="R Step PV" class="DigNum (strict)"() -> ("Value"=w771:i32)  [unwired: 2 in, 2 out]
                    n568 = Equal?(x=w777, y=w776) -> (x = y?=w782:bool)
                    n569 = Equal?(x=w775, y=w774) -> (x = y?=w781:bool)
                    n570 = Equal?(x=w773, y=w772) -> (x = y?=w779:bool)
                    n571 = Equal?(x=w770, y=w771) -> (x = y?=w780:bool)
                    n572 = Compound Arithmetic op=AND(w782, w781, w779, w780) -> (w778:bool)
                    n573 = case shown="True" w778 {
                      frame #0 {
                      }
                      frame #1 {
                        n574 = property on="GO" class="Bool"("DisabledEnum"=T9."Enabled" ("Disabled")) -> ()  [unwired: 2 in, 2 out]
                        n575 = local write "STATUS"("SCANNING DONE" ("STATUS")) -> ()
                      }
                    }
                  }
                }
              }
              frame #1 {
                n576 = property on="X Scan Length SP steps" class="DigNum (strict)"() -> ("Value"=w796:i32)  [unwired: 2 in, 2 out]
                n577 = property on="Y Scan Length SP steps" class="DigNum (strict)"() -> ("Value"=w795:i32)  [unwired: 2 in, 2 out]
                n578 = property on="Z Scan Length SP steps" class="DigNum (strict)"() -> ("Value"=w794:i32)  [unwired: 2 in, 2 out]
                n579 = property on="R Scan Length SP steps" class="DigNum (strict)"() -> ("Value"=w793:i32)  [unwired: 2 in, 2 out]
                n580 = property on="X Step SP" class="DigNum (strict)"() -> ("Value"=w792:i32)  [unwired: 2 in, 2 out]
                n581 = property on="Y Step SP" class="DigNum (strict)"() -> ("Value"=w791:i32)  [unwired: 2 in, 2 out]
                n582 = property on="Z Step SP" class="DigNum (strict)"() -> ("Value"=w790:i32)  [unwired: 2 in, 2 out]
                n583 = property on="R Step SP" class="DigNum (strict)"() -> ("Value"=w789:i32)  [unwired: 2 in, 2 out]
                n584 = Add(x=w796, y=w792) -> (x+y=w805:i32)
                n585 = Add(x=w795, y=w791) -> (x+y=w804:i32)
                n586 = Add(x=w794, y=w790) -> (x+y=w803:i32)
                n587 = Add(x=w793, y=w789) -> (x+y=w802:i32)
                n588 = property on="X Step PV" class="DigNum (strict)"() -> ("Value"=w788:i32)  [unwired: 2 in, 2 out]
                n589 = property on="Y Step PV" class="DigNum (strict)"() -> ("Value"=w787:i32)  [unwired: 2 in, 2 out]
                n590 = property on="Z Step PV" class="DigNum (strict)"() -> ("Value"=w786:i32)  [unwired: 2 in, 2 out]
                n591 = property on="R Step PV" class="DigNum (strict)"() -> ("Value"=w785:i32)  [unwired: 2 in, 2 out]
                n592 = Equal?(x=w788, y=w805) -> (x = y?=w801:bool)
                n593 = Equal?(x=w787, y=w804) -> (x = y?=w800:bool)
                n594 = Equal?(x=w786, y=w803) -> (x = y?=w798:bool)
                n595 = Equal?(x=w785, y=w802) -> (x = y?=w799:bool)
                n596 = Compound Arithmetic op=AND(w801, w800, w798, w799) -> (w797:bool)
                n597 = case shown="True" w797 {
                  frame #0 {
                  }
                  frame #1 {
                    n598 = local write "Scan Go"(FALSE ("Scan Go")) -> ()
                    n599 = local write "STATUS"("DONE" ("STATUS")) -> ()
                    n600 = property on="Send scan parameter" class="Bool"("DisabledEnum"=T9."Enabled" ("Disabled")) -> ()  [unwired: 2 in, 2 out]
                    n601 = property on="Set Scan \nParameters" class="Bool"("DisabledEnum"=T9."Enabled" ("Disabled")) -> ()  [unwired: 2 in, 2 out]
                    n602 = property on="GO" class="Bool"("DisabledEnum"=T9."Enabled" ("Disabled")) -> ()  [unwired: 2 in, 2 out]
                  }
                }
              }
            }
          }
        }
        n603 = case shown="False" w497 {
          tunnel: w501 -> [w542 w547]
          tunnel: [w542 w546] -> w500
          tunnel: w499 -> [w541 w545]
          tunnel: [w541 w544] -> w498
          frame #0 {
          }
          frame #1 {
            w543 = 0 ("dimension size")
            n604 = Reshape Array(w547, w543) -> (w546:dbl[])
            n605 = Reshape Array(w545, w543) -> (w544:dbl[])
          }
        }
        n606 = And(x=w511, y=w507) -> (x .and. y?=w508:bool)
        n607 = case shown="False" w507 {
          frame #0 {
            n608 = local write "STATUS"("SCANNING MODE" ("STATUS")) -> ()
          }
          frame #1 {
          }
        }
        n609 = Divide(x=w530, y=6.283185307179586) -> (x/y=w531:dbl)
        n610 = case shown="False" w508 {
          frame #0 {
          }
          frame #1 {
            n611 = local write "STATUS"("") -> ()
          }
        }
        n612 = Multiply(x=360.0, y=w531) -> (x*y=w534:dbl)
        n613 = property on="atan Y/Z" class="DigNum (strict)"("Val(Sgnl)"=w534) -> ()  [unwired: 2 in, 2 out]
      }
      event #1 {
        n614 = event-data() -> ()  [unwired: 1 in, 5 out]
        n615 = property on="OK Button" class="Bool (strict)"() -> ("Value"=w1342:bool)  [unwired: 2 in, 2 out]
        n616 = property on="Z Step PV" class="DigNum (strict)"() -> ("Value"=w1347:i32)  [unwired: 2 in, 2 out]
        n617 = Greater?(x=w1347, y=15360000) -> (0:w1344:bool)
        n618 = Equal?(x=w1342, y=TRUE) -> (x = y?=w1345:bool)
        n619 = local write "STATUS"("VALVE CHANGED" ("STATUS")) -> ()
        n620 = And(x=w1345, y=w1344) -> (x .and. y?=w1343:bool)
        n621 = case shown="False" w1343 {
          frame #0 {
            n622 = property on="OK Button" class="Bool (strict)"() -> ("Value"=w1350:bool)  [unwired: 2 in, 2 out]
            n623 = property on="Z Step PV" class="DigNum (strict)"() -> ("Value"=w1355:i32)  [unwired: 2 in, 2 out]
            n624 = Greater?(x=w1355, y=15360000) -> (0:w1353:bool)
            n625 = Equal?(x=w1350, y=FALSE) -> (x = y?=w1352:bool)
            n626 = And(x=w1352, y=w1353) -> (x .and. y?=w1351:bool)
            n627 = case shown="True" w1351 {
              frame #0 {
              }
              frame #1 {
                n628 = One Button Dialog(message="YOU CAN'T CLOSE THE VALVE\nWHEN YOU ARE IN THE THIS\nPOSITION!!") -> (true=w1357:bool)  [unwired: 1 in]
                n629 = property on="OK Button" class="Bool (strict)"("Val(Sgnl)"=w1357) -> ()  [unwired: 2 in, 2 out]
              }
            }
          }
          frame #1 {
            n630 = flat-sequence {
              frame #0 {
                n631 = local read "OK Button"() -> (w1360:bool)
                n632 = call "DigitalIO_sub_V1_CNTL.vi"("OK Button"=w1360) -> ("Boolean"=w1359:bool)  [unwired: 2 in]
                n633 = property on="Valve \nopend/closed" class="Bool (strict)"("Val(Sgnl)"=w1359) -> ()  [unwired: 2 in, 2 out]
              }
              frame #1 {
                n634 = call "DigitalIO_sub_V1_MON.vi"() -> ("CL"=w1362:bool, "OP"=w1361:bool)  [unwired: 8 in]
                n635 = property on="OP" class="Bool (strict)"("Val(Sgnl)"=w1361) -> ()  [unwired: 2 in, 2 out]
                n636 = property on="CL" class="Bool (strict)"("Val(Sgnl)"=w1362) -> ()  [unwired: 2 in, 2 out]
              }
              frame #2 {
                n637 = Wait (ms)(milliseconds to wait=u32 100) -> ()  [unwired: 1 out]
              }
            }
          }
        }
      }
      event #2 {
        n638 = event-data() -> ()  [unwired: 1 in, 7 out]
        n639 = local write "STATUS"("MOVING" ("STATUS")) -> ()
        n640 = property on="X Position mm PV" class="DigNum (strict)"() -> ("Value"=w1384:dbl)  [unwired: 2 in, 2 out]
        n641 = property on="X Position SP mm" class="DigNum (strict)"() -> ("Value"=w1383:dbl)  [unwired: 2 in, 2 out]
        n642 = property on="Z Position mm PV" class="DigNum (strict)"() -> ("Value"=w1380:dbl)  [unwired: 2 in, 2 out]
        n643 = property on="Z Position SP mm" class="DigNum (strict)"() -> ("Value"=w1372:dbl)  [unwired: 2 in, 2 out]
        n644 = property on="Y Position mm PV" class="DigNum (strict)"() -> ("Value"=w1378:dbl)  [unwired: 2 in, 2 out]
        n645 = property on="Y Position SP mm" class="DigNum (strict)"() -> ("Value"=w1377:dbl)  [unwired: 2 in, 2 out]
        n646 = property on="R Position SP deg" class="DigNum (strict)"() -> ("Value"=w1375:dbl)  [unwired: 2 in, 2 out]
        n647 = property on="R Position deg PV" class="DigNum (strict)"() -> ("Value"=w1374:dbl)  [unwired: 2 in, 2 out]
        n648 = Not Equal?(x=w1384, y=w1383) -> (x != y?=w1382:bool)
        n649 = Not Equal?(x=w1380, y=w1372) -> (x != y?=w1381:bool)
        n650 = Not Equal?(x=w1378, y=w1377) -> (x != y?=w1379:bool)
        n651 = Not Equal?(x=w1375, y=w1374) -> (x != y?=w1376:bool)
        n652 = case shown="True" w1381 {
          tunnel: w1391 -> [w1534 w1541]
          tunnel: w1390 -> [w1535 w1540]
          tunnel: [w1535 w1539] -> w1369
          tunnel: [w1534 w1538] -> w1368
          frame #0 {
          }
          frame #1 {
            n653 = flat-sequence {
              tunnel: w1540 -> [w1563]
              tunnel: w1541 -> [w1564]
              tunnel: [w1564] -> w1537
              tunnel: [w1563] -> w1536
              tunnel: [w1579] -> w1555
              tunnel: [w1578] -> w1554
              tunnel: [w1566] -> w1553
              tunnel: w1537 -> [w1579]
              tunnel: w1536 -> [w1578]
              tunnel: [w1582] -> w1552
              tunnel: [w1581] -> w1551
              tunnel: [w1580] -> w1550
              tunnel: w1553 -> [w1580]
              tunnel: w1554 -> [w1581]
              tunnel: w1555 -> [w1582]
              tunnel: [w1598] -> w1549
              tunnel: [w1597] -> w1548
              tunnel: w1552 -> [w1596]
              tunnel: w1551 -> [w1595]
              tunnel: [w1594] -> w1547
              tunnel: w1550 -> [w1594]
              tunnel: w1549 -> [w1605]
              tunnel: [w1605] -> w1546
              tunnel: w1548 -> [w1604]
              tunnel: [w1604] -> w1545
              tunnel: w1547 -> [w1603]
              tunnel: [w1603] -> w1544
              tunnel: [w1610] -> w1543
              tunnel: [w1609] -> w1542
              tunnel: w1546 -> [w1608]
              tunnel: w1545 -> [w1607]
              tunnel: w1544 -> [w1606]
              tunnel: [w1614] -> w1538
              tunnel: [w1615] -> w1539
              tunnel: w1543 -> [w1615]
              tunnel: w1542 -> [w1614]
              frame #0 {
                n654 = property on="Z Position mm PV" class="DigNum (strict)"() -> ("Value"=w1556:dbl)  [unwired: 2 in, 2 out]
                n655 = property on="Z Position SP mm" class="DigNum (strict)"() -> ("Value"=w1558:dbl)  [unwired: 2 in, 2 out]
                n656 = Less?(x=w1556, y=60.0) -> (x < y?=w1560:bool)
                n657 = Greater?(x=w1558, y=60.0) -> (0:w1561:bool)
                n658 = And(x=w1560, y=w1561) -> (x .and. y?=w1562:bool)
                n659 = case shown="True" w1562 {
                  frame #0 {
                  }
                  frame #1 {
                    n660 = property on="Z Position SP mm" class="DigNum (strict)"("Val(Sgnl)"=60.0 ("Value (Signaling)")) -> ()  [unwired: 2 in, 2 out]
                  }
                }
              }
              frame #1 {
                n661 = property on="Z steps/rev" class="DigNum (strict)"() -> ("Value"=w1575:u32)  [unwired: 2 in, 2 out]
                n662 = To Double Precision Float(number=w1575) -> (double precision float=w1571:dbl)
                n663 = property on="Z offset mm" class="DigNum (strict)"() -> ("Value"=w1573:dbl)  [unwired: 2 in, 2 out]
                n664 = property on="Z Position SP mm" class="DigNum (strict)"() -> ("Value"=w1572:dbl)  [unwired: 2 in, 2 out]
                n665 = Subtract(x=w1572, y=w1573) -> (x-y=w1568:dbl)
                n666 = property on="Z mm/rev" class="DigNum (strict)"() -> ("Value"=w1574:dbl)  [unwired: 2 in, 2 out]
                n667 = Divide(x=w1568, y=w1574) -> (x/y=w1567:dbl)
                n668 = property on="Z Step SP" class="DigNum (strict)"() -> ("Maximum"=w1577:dbl)  [unwired: 2 in, 2 out]
                n669 = property on="Z Step SP" class="DigNum (strict)"() -> ("Minimum"=w1576:dbl)  [unwired: 2 in, 2 out]
                n670 = Multiply(x=w1567, y=w1571) -> (x*y=w1569:dbl)
                n671 = In Range and Coerce(upper limit=w1577, x=w1569, lower limit=w1576) -> (coerced(x)=w1570:dbl)  [unwired: 1 out]
                n672 = To Long Integer(number=w1570) -> (32bit integer=w1566:i32)
                n673 = property on="Z Step SP" class="DigNum (strict)"("Val(Sgnl)"=w1566) -> ()  [unwired: 2 in, 2 out]
              }
              frame #2 {
                n674 = property on="Z Step SP" class="DigNum (strict)"() -> ("Value"=w1591:i32)  [unwired: 2 in, 2 out]
                n675 = property on="Z Step PV" class="DigNum (strict)"() -> ("Value"=w1590:i32)  [unwired: 2 in, 2 out]
                n676 = property on="Z Backlash" class="DigNum (strict)"() -> ("Value"=w1583:i32)  [unwired: 2 in, 2 out]
                n677 = Subtract(x=w1591, y=w1590) -> (x-y=w1589:i32)
                n678 = Sign(1:w1583) -> (0:w1587:i32)
                n679 = Sign(1:w1589) -> (0:w1588:i32)
                n680 = Multiply(x=w1588, y=w1587) -> (x*y=w1586:i32)
                n681 = Equal?(x=w1586, y=1) -> (x = y?=w1584:bool)
                n682 = case shown="False" w1584 {
                  frame #0 {
                    n683 = property on="Z Backlash corr" class="Bool (strict)"("Val(Sgnl)"=FALSE ("Value (Signaling)")) -> ()  [unwired: 2 in, 2 out]
                  }
                  frame #1 {
                    n684 = property on="Z Backlash corr" class="Bool (strict)"("Val(Sgnl)"=TRUE ("Value (Signaling)")) -> ()  [unwired: 2 in, 2 out]
                  }
                }
              }
              frame #3 {
                # "Velocity Setting"
                n685 = property on="Z Velocity SP step/sec" class="DigNum (strict)"() -> ("Value"=w1599:i32)  [unwired: 2 in, 2 out]
                n686 = Number To Decimal String(number=w1599) -> (decimal integer string=w1600:string)  [unwired: 1 in]
                n687 = call "mdrive send command.vi"("error in (no error)"=w1596, "Extra"=w1600, "Command"=T10."Max Velocity", "VISA resource name"=w1595) -> ("error out"=w1597:errorcluster, "VISA resource name out"=w1598:refnum<visa-resource-name>)  [unwired: 3 in, 1 out]
              }
              frame #4 {
                n688 = Wait (ms)(milliseconds to wait=u32 50) -> ()  [unwired: 1 out]
              }
              frame #5 {
                # "Move to Abs Position"
                n689 = Number To Decimal String(number=w1606) -> (decimal integer string=w1612:string)  [unwired: 1 in]
                n690 = call "mdrive send command.vi"("error in (no error)"=w1607, "Extra"=w1612, "Command"=T10."Move to Absolute Position", "VISA resource name"=w1608) -> ("error out"=w1609:errorcluster, "VISA resource name out"=w1610:refnum<visa-resource-name>)  [unwired: 3 in, 1 out]
              }
              frame #6 {
                n691 = Wait (ms)(milliseconds to wait=u32 50) -> ()  [unwired: 1 out]
              }
            }
          }
        }
        n692 = property on="GO" class="Bool"("DisabledEnum"=T9."Disabled and Grayed Out" ("Disabled")) -> ()  [unwired: 2 in, 2 out]
        n693 = case shown="True" w1382 {
          tunnel: w1393 -> [w1617 w1621]
          tunnel: w1392 -> [w1616 w1620]
          tunnel: [w1617 w1619] -> w1371
          tunnel: [w1616 w1618] -> w1370
          frame #0 {
          }
          frame #1 {
            n694 = flat-sequence {
              tunnel: w1620 -> [w1648]
              tunnel: w1621 -> [w1649]
              tunnel: [w1649] -> w1635
              tunnel: [w1648] -> w1634
              tunnel: [w1637] -> w1633
              tunnel: [w1652] -> w1632
              tunnel: [w1651] -> w1631
              tunnel: [w1650] -> w1630
              tunnel: w1633 -> [w1650]
              tunnel: w1634 -> [w1651]
              tunnel: w1635 -> [w1652]
              tunnel: [w1668] -> w1629
              tunnel: [w1667] -> w1628
              tunnel: w1632 -> [w1666]
              tunnel: w1631 -> [w1665]
              tunnel: w1630 -> [w1664]
              tunnel: [w1664] -> w1627
              tunnel: w1629 -> [w1675]
              tunnel: [w1675] -> w1626
              tunnel: w1628 -> [w1674]
              tunnel: [w1674] -> w1625
              tunnel: [w1672] -> w1624
              tunnel: w1627 -> [w1672]
              tunnel: [w1680] -> w1623
              tunnel: [w1679] -> w1622
              tunnel: w1626 -> [w1678]
              tunnel: w1625 -> [w1677]
              tunnel: w1624 -> [w1676]
              tunnel: [w1684] -> w1618
              tunnel: [w1685] -> w1619
              tunnel: w1623 -> [w1685]
              tunnel: w1622 -> [w1684]
              frame #0 {
                n695 = property on="X steps/rev" class="DigNum (strict)"() -> ("Value"=w1647:u32)  [unwired: 2 in, 2 out]
                n696 = To Double Precision Float(number=w1647) -> (double precision float=w1642:dbl)
                n697 = property on="X offset mm" class="DigNum (strict)"() -> ("Value"=w1646:dbl)  [unwired: 2 in, 2 out]
                n698 = property on="X Position SP mm" class="DigNum (strict)"() -> ("Value"=w1645:dbl)  [unwired: 2 in, 2 out]
                n699 = Subtract(x=w1645, y=w1646) -> (x-y=w1639:dbl)
                n700 = property on="X mm/rev" class="DigNum (strict)"() -> ("Value"=w1636:dbl)  [unwired: 2 in, 2 out]
                n701 = Divide(x=w1639, y=w1636) -> (x/y=w1638:dbl)
                n702 = property on="X Step SP" class="DigNum (strict)"() -> ("Maximum"=w1644:dbl)  [unwired: 2 in, 2 out]
                n703 = property on="X Step SP" class="DigNum (strict)"() -> ("Minimum"=w1643:dbl)  [unwired: 2 in, 2 out]
                n704 = Multiply(x=w1638, y=w1642) -> (x*y=w1640:dbl)
                n705 = In Range and Coerce(upper limit=w1644, x=w1640, lower limit=w1643) -> (coerced(x)=w1641:dbl)  [unwired: 1 out]
                n706 = To Long Integer(number=w1641) -> (32bit integer=w1637:i32)
                n707 = property on="X Step SP" class="DigNum (strict)"("Val(Sgnl)"=w1637) -> ()  [unwired: 2 in, 2 out]
              }
              frame #1 {
                n708 = property on="X Step SP" class="DigNum (strict)"() -> ("Value"=w1661:i32)  [unwired: 2 in, 2 out]
                n709 = property on="X Step PV" class="DigNum (strict)"() -> ("Value"=w1660:i32)  [unwired: 2 in, 2 out]
                n710 = property on="X Backlash" class="DigNum (strict)"() -> ("Value"=w1653:i32)  [unwired: 2 in, 2 out]
                n711 = Subtract(x=w1661, y=w1660) -> (x-y=w1659:i32)
                n712 = Sign(1:w1653) -> (0:w1657:i32)
                n713 = Sign(1:w1659) -> (0:w1658:i32)
                n714 = Multiply(x=w1658, y=w1657) -> (x*y=w1656:i32)
                n715 = Equal?(x=w1656, y=1) -> (x = y?=w1654:bool)
                n716 = case shown="False" w1654 {
                  frame #0 {
                    n717 = property on="X Backlash corr" class="Bool (strict)"("Val(Sgnl)"=FALSE ("Value (Signaling)")) -> ()  [unwired: 2 in, 2 out]
                  }
                  frame #1 {
                    n718 = property on="X Backlash corr" class="Bool (strict)"("Val(Sgnl)"=TRUE ("Value (Signaling)")) -> ()  [unwired: 2 in, 2 out]
                  }
                }
              }
              frame #2 {
                # "Velocity Setting"
                n719 = property on="X Velocity SP step/sec" class="DigNum (strict)"() -> ("Value"=w1669:i32)  [unwired: 2 in, 2 out]
                n720 = Number To Decimal String(number=w1669) -> (decimal integer string=w1670:string)  [unwired: 1 in]
                n721 = call "mDrive Send Command.vi"("error in (no error)"=w1665, "Extra"=w1670, "Command"=T10."Max Velocity", "VISA resource name"=w1666) -> ("error out"=w1667:errorcluster, "VISA resource name out"=w1668:refnum<visa-resource-name>)  [unwired: 3 in, 1 out]
              }
              frame #3 {
                n722 = Wait (ms)(milliseconds to wait=u32 50) -> ()  [unwired: 1 out]
              }
              frame #4 {
                # "Move to Abs Position"
                n723 = Number To Decimal String(number=w1676) -> (decimal integer string=w1682:string)  [unwired: 1 in]
                n724 = call "mDrive Send Command.vi"("error in (no error)"=w1677, "Extra"=w1682, "Command"=T10."Move to Absolute Position", "VISA resource name"=w1678) -> ("error out"=w1679:errorcluster, "VISA resource name out"=w1680:refnum<visa-resource-name>)  [unwired: 3 in, 1 out]
              }
              frame #5 {
                n725 = Wait (ms)(milliseconds to wait=u32 50) -> ()  [unwired: 1 out]
              }
            }
          }
        }
        n726 = case shown="True" w1379 {
          tunnel: w1389 -> [w1464 w1469]
          tunnel: w1388 -> [w1465 w1468]
          tunnel: [w1465 w1467] -> w1367
          tunnel: [w1464 w1466] -> w1366
          frame #0 {
          }
          frame #1 {
            n727 = flat-sequence {
              tunnel: [w1497] -> w1483
              tunnel: [w1496] -> w1482
              tunnel: [w1484] -> w1481
              tunnel: w1468 -> [w1496]
              tunnel: w1469 -> [w1497]
              tunnel: [w1500] -> w1480
              tunnel: [w1499] -> w1479
              tunnel: [w1498] -> w1478
              tunnel: w1481 -> [w1498]
              tunnel: w1482 -> [w1499]
              tunnel: w1483 -> [w1500]
              tunnel: [w1516] -> w1477
              tunnel: [w1515] -> w1476
              tunnel: w1480 -> [w1514]
              tunnel: w1479 -> [w1513]
              tunnel: [w1512] -> w1475
              tunnel: w1478 -> [w1512]
              tunnel: w1477 -> [w1523]
              tunnel: [w1523] -> w1474
              tunnel: w1476 -> [w1522]
              tunnel: [w1522] -> w1473
              tunnel: [w1520] -> w1472
              tunnel: w1475 -> [w1520]
              tunnel: [w1528] -> w1471
              tunnel: [w1527] -> w1470
              tunnel: w1474 -> [w1526]
              tunnel: w1473 -> [w1525]
              tunnel: w1472 -> [w1524]
              tunnel: [w1531] -> w1466
              tunnel: [w1533] -> w1467
              tunnel: w1471 -> [w1533]
              tunnel: w1470 -> [w1531]
              frame #0 {
                n728 = property on="Y steps/rev" class="DigNum (strict)"() -> ("Value"=w1493:u32)  [unwired: 2 in, 2 out]
                n729 = To Double Precision Float(number=w1493) -> (double precision float=w1489:dbl)
                n730 = property on="Y offset mm" class="DigNum (strict)"() -> ("Value"=w1491:dbl)  [unwired: 2 in, 2 out]
                n731 = property on="Y Position SP mm" class="DigNum (strict)"() -> ("Value"=w1490:dbl)  [unwired: 2 in, 2 out]
                n732 = Subtract(x=w1490, y=w1491) -> (x-y=w1486:dbl)
                n733 = property on="Y mm/rev" class="DigNum (strict)"() -> ("Value"=w1492:dbl)  [unwired: 2 in, 2 out]
                n734 = Divide(x=w1486, y=w1492) -> (x/y=w1485:dbl)
                n735 = property on="Y Step SP" class="DigNum (strict)"() -> ("Maximum"=w1494:dbl)  [unwired: 2 in, 2 out]
                n736 = property on="Y Step SP" class="DigNum (strict)"() -> ("Minimum"=w1495:dbl)  [unwired: 2 in, 2 out]
                n737 = Multiply(x=w1485, y=w1489) -> (x*y=w1487:dbl)
                n738 = In Range and Coerce(upper limit=w1494, x=w1487, lower limit=w1495) -> (coerced(x)=w1488:dbl)  [unwired: 1 out]
                n739 = To Long Integer(number=w1488) -> (32bit integer=w1484:i32)
                n740 = property on="Y Step SP" class="DigNum (strict)"("Val(Sgnl)"=w1484) -> ()  [unwired: 2 in, 2 out]
              }
              frame #1 {
                n741 = property on="Y Step SP" class="DigNum (strict)"() -> ("Value"=w1509:i32)  [unwired: 2 in, 2 out]
                n742 = property on="Y Step PV" class="DigNum (strict)"() -> ("Value"=w1508:i32)  [unwired: 2 in, 2 out]
                n743 = property on="Y Backlash" class="DigNum (strict)"() -> ("Value"=w1501:i32)  [unwired: 2 in, 2 out]
                n744 = Subtract(x=w1509, y=w1508) -> (x-y=w1507:i32)
                n745 = Sign(1:w1501) -> (0:w1505:i32)
                n746 = Sign(1:w1507) -> (0:w1506:i32)
                n747 = Multiply(x=w1506, y=w1505) -> (x*y=w1504:i32)
                n748 = Equal?(x=w1504, y=1) -> (x = y?=w1502:bool)
                n749 = case shown="False" w1502 {
                  frame #0 {
                    n750 = property on="Y Backlash corr" class="Bool (strict)"("Val(Sgnl)"=FALSE ("Value (Signaling)")) -> ()  [unwired: 2 in, 2 out]
                  }
                  frame #1 {
                    n751 = property on="Y Backlash corr" class="Bool (strict)"("Val(Sgnl)"=TRUE ("Value (Signaling)")) -> ()  [unwired: 2 in, 2 out]
                  }
                }
              }
              frame #2 {
                # "Velocity Setting"
                n752 = property on="Y Velocity SP step/sec" class="DigNum (strict)"() -> ("Value"=w1517:i32)  [unwired: 2 in, 2 out]
                n753 = Number To Decimal String(number=w1517) -> (decimal integer string=w1518:string)  [unwired: 1 in]
                n754 = call "mdrive send command.vi"("error in (no error)"=w1514, "Extra"=w1518, "Command"=T10."Max Velocity", "VISA resource name"=w1513) -> ("error out"=w1515:errorcluster, "VISA resource name out"=w1516:refnum<visa-resource-name>)  [unwired: 3 in, 1 out]
              }
              frame #3 {
                n755 = Wait (ms)(milliseconds to wait=u32 50) -> ()  [unwired: 1 out]
              }
              frame #4 {
                # "Move to Abs Position"
                n756 = Number To Decimal String(number=w1524) -> (decimal integer string=w1530:string)  [unwired: 1 in]
                n757 = call "mdrive send command.vi"("error in (no error)"=w1525, "Extra"=w1530, "Command"=T10."Move to Absolute Position", "VISA resource name"=w1526) -> ("error out"=w1527:errorcluster, "VISA resource name out"=w1528:refnum<visa-resource-name>)  [unwired: 3 in, 1 out]
              }
              frame #5 {
                n758 = Wait (ms)(milliseconds to wait=u32 25) -> ()  [unwired: 1 out]
              }
            }
          }
        }
        n759 = case shown="True" w1376 {
          tunnel: w1387 -> [w1394 w1399]
          tunnel: w1386 -> [w1395 w1398]
          tunnel: [w1395 w1397] -> w1365
          tunnel: [w1394 w1396] -> w1364
          frame #0 {
          }
          frame #1 {
            n760 = flat-sequence {
              tunnel: w1398 -> [w1426]
              tunnel: w1399 -> [w1427]
              tunnel: [w1427] -> w1413
              tunnel: [w1426] -> w1412
              tunnel: [w1414] -> w1411
              tunnel: [w1430] -> w1410
              tunnel: [w1429] -> w1409
              tunnel: [w1428] -> w1408
              tunnel: w1411 -> [w1428]
              tunnel: w1412 -> [w1429]
              tunnel: w1413 -> [w1430]
              tunnel: [w1446] -> w1407
              tunnel: [w1445] -> w1406
              tunnel: w1410 -> [w1444]
              tunnel: w1409 -> [w1443]
              tunnel: [w1442] -> w1405
              tunnel: w1408 -> [w1442]
              tunnel: w1407 -> [w1453]
              tunnel: [w1453] -> w1404
              tunnel: w1406 -> [w1452]
              tunnel: [w1452] -> w1403
              tunnel: w1405 -> [w1451]
              tunnel: [w1451] -> w1402
              tunnel: [w1458] -> w1401
              tunnel: [w1457] -> w1400
              tunnel: w1404 -> [w1456]
              tunnel: w1403 -> [w1455]
              tunnel: w1402 -> [w1454]
              tunnel: [w1463] -> w1397
              tunnel: w1401 -> [w1463]
              tunnel: w1400 -> [w1462]
              tunnel: [w1462] -> w1396
              frame #0 {
                n761 = property on="R steps/rev" class="DigNum (strict)"() -> ("Value"=w1422:u32)  [unwired: 2 in, 2 out]
                n762 = To Double Precision Float(number=w1422) -> (double precision float=w1419:dbl)
                n763 = property on="R offset deg" class="DigNum (strict)"() -> ("Value"=w1423:dbl)  [unwired: 2 in, 2 out]
                n764 = property on="R Position SP deg" class="DigNum (strict)"() -> ("Value"=w1424:dbl)  [unwired: 2 in, 2 out]
                n765 = Subtract(x=w1424, y=w1423) -> (x-y=w1416:dbl)
                n766 = property on="R deg/rev" class="DigNum (strict)"() -> ("Value"=w1425:dbl)  [unwired: 2 in, 2 out]
                n767 = Divide(x=w1416, y=w1425) -> (x/y=w1415:dbl)
                n768 = property on="R Step SP" class="DigNum (strict)"() -> ("Maximum"=w1420:dbl)  [unwired: 2 in, 2 out]
                n769 = Multiply(x=w1415, y=w1419) -> (x*y=w1417:dbl)
                n770 = property on="R Step SP" class="DigNum (strict)"() -> ("Minimum"=w1421:dbl)  [unwired: 2 in, 2 out]
                n771 = In Range and Coerce(upper limit=w1420, x=w1417, lower limit=w1421) -> (coerced(x)=w1418:dbl)  [unwired: 1 out]
                n772 = To Long Integer(number=w1418) -> (32bit integer=w1414:i32)
                n773 = property on="R Step SP" class="DigNum (strict)"("Val(Sgnl)"=w1414) -> ()  [unwired: 2 in, 2 out]
              }
              frame #1 {
                n774 = property on="R Step SP" class="DigNum (strict)"() -> ("Value"=w1439:i32)  [unwired: 2 in, 2 out]
                n775 = property on="R Step PV" class="DigNum (strict)"() -> ("Value"=w1438:i32)  [unwired: 2 in, 2 out]
                n776 = property on="R Backlash" class="DigNum (strict)"() -> ("Value"=w1431:i32)  [unwired: 2 in, 2 out]
                n777 = Subtract(x=w1439, y=w1438) -> (x-y=w1437:i32)
                n778 = Sign(1:w1431) -> (0:w1435:i32)
                n779 = Sign(1:w1437) -> (0:w1436:i32)
                n780 = Multiply(x=w1436, y=w1435) -> (x*y=w1434:i32)
                n781 = Equal?(x=w1434, y=1) -> (x = y?=w1432:bool)
                n782 = case shown="False" w1432 {
                  frame #0 {
                    n783 = property on="R Backlash corr" class="Bool (strict)"("Val(Sgnl)"=FALSE ("Value (Signaling)")) -> ()  [unwired: 2 in, 2 out]
                  }
                  frame #1 {
                    n784 = property on="R Backlash corr" class="Bool (strict)"("Val(Sgnl)"=TRUE ("Value (Signaling)")) -> ()  [unwired: 2 in, 2 out]
                  }
                }
              }
              frame #2 {
                # "Velocity Setting"
                n785 = property on="R Velocity SP step/sec" class="DigNum (strict)"() -> ("Value"=w1447:i32)  [unwired: 2 in, 2 out]
                n786 = Number To Decimal String(number=w1447) -> (decimal integer string=w1448:string)  [unwired: 1 in]
                n787 = call "mdrive send command.vi"("error in (no error)"=w1444, "Extra"=w1448, "Command"=T10."Max Velocity", "VISA resource name"=w1443) -> ("error out"=w1445:errorcluster, "VISA resource name out"=w1446:refnum<visa-resource-name>)  [unwired: 3 in, 1 out]
              }
              frame #3 {
                n788 = Wait (ms)(milliseconds to wait=u32 50) -> ()  [unwired: 1 out]
              }
              frame #4 {
                # "Move to Abs Position"
                n789 = Number To Decimal String(number=w1454) -> (decimal integer string=w1460:string)  [unwired: 1 in]
                n790 = call "mdrive send command.vi"("error in (no error)"=w1455, "Extra"=w1460, "Command"=T10."Move to Absolute Position", "VISA resource name"=w1456) -> ("error out"=w1457:errorcluster, "VISA resource name out"=w1458:refnum<visa-resource-name>)  [unwired: 3 in, 1 out]
              }
              frame #5 {
                n791 = Wait (ms)(milliseconds to wait=u32 25) -> ()  [unwired: 1 out]
              }
            }
          }
        }
      }
      event #3 {
        n792 = event-data() -> ()  [unwired: 1 in, 7 out]
        n793 = flat-sequence {
          tunnel: w1710 -> [w1739]
          tunnel: [w1738] -> w1705
          tunnel: w1689 -> [w1737]
          tunnel: [w1736] -> w1687
          tunnel: [w1743] -> w1706
          tunnel: w1705 -> [w1743]
          tunnel: [w1742] -> w1688
          tunnel: w1687 -> [w1742]
          tunnel: w1706 -> [w1760]
          tunnel: w1688 -> [w1757]
          tunnel: [w1756] -> _
          tunnel: [w1755] -> _
          frame #0 {
            n794 = call "mDrive Send Command.vi"("error in (no error)"=w1739, "Command"=T10."Stop", "VISA resource name"=w1737) -> ("error out"=w1738:errorcluster, "VISA resource name out"=w1736:refnum<visa-resource-name>)  [unwired: 4 in, 1 out]
          }
          frame #1 {
            n795 = Wait (ms)(milliseconds to wait=u32 50) -> ()  [unwired: 1 out]
          }
          frame #2 {
            n796 = property on="X steps/rev" class="DigNum (strict)"() -> ("Value"=w1746:u32)  [unwired: 2 in, 2 out]
            n797 = property on="X offset mm" class="DigNum (strict)"() -> ("Value"=w1744:dbl)  [unwired: 2 in, 2 out]
            n798 = To Double Precision Float(number=w1746) -> (double precision float=w1751:dbl)
            n799 = call "mDrive Send Command.vi"("error in (no error)"=w1760, "Extra"="P", "Command"=T10."Print Parameter", "VISA resource name"=w1757) -> ("error out"=w1755:errorcluster, "read buffer"=w1750:string, "VISA resource name out"=w1756:refnum<visa-resource-name>)  [unwired: 3 in]
            n800 = Decimal String To Number(string=w1750, offset=0) -> (number=w1748:i32)  [unwired: 1 in, 1 out]
            n801 = property on="X Step PV" class="DigNum (strict)"("Val(Sgnl)"=w1748) -> ()  [unwired: 2 in, 2 out]
            n802 = To Double Precision Float(number=w1748) -> (double precision float=w1752:dbl)
            n803 = Divide(x=w1752, y=w1751) -> (x/y=w1754:dbl)
            n804 = property on="X mm/rev" class="DigNum (strict)"() -> ("Value"=w1745:dbl)  [unwired: 2 in, 2 out]
            n805 = Multiply(x=w1754, y=w1745) -> (x*y=w1753:dbl)
            n806 = Add(x=w1753, y=w1744) -> (x+y=w1747:dbl)
            n807 = property on="X Position mm PV" class="DigNum (strict)"("Val(Sgnl)"=w1747) -> ()  [unwired: 2 in, 2 out]
          }
        }
        n808 = property on="GO" class="Bool"("DisabledEnum"=T9."Enabled" ("Disabled")) -> ()  [unwired: 2 in, 2 out]
        n809 = flat-sequence {
          tunnel: w1707 -> [w1714]
          tunnel: [w1713] -> w1699
          tunnel: w1698 -> [w1712]
          tunnel: [w1711] -> w1696
          tunnel: [w1718] -> w1700
          tunnel: w1699 -> [w1718]
          tunnel: [w1717] -> w1697
          tunnel: w1696 -> [w1717]
          tunnel: w1700 -> [w1735]
          tunnel: w1697 -> [w1732]
          tunnel: [w1731] -> _
          tunnel: [w1730] -> _
          frame #0 {
            n810 = call "mDrive Send Command.vi"("error in (no error)"=w1714, "Command"=T10."Stop", "VISA resource name"=w1712) -> ("error out"=w1713:errorcluster, "VISA resource name out"=w1711:refnum<visa-resource-name>)  [unwired: 4 in, 1 out]
          }
          frame #1 {
            n811 = Wait (ms)(milliseconds to wait=u32 50) -> ()  [unwired: 1 out]
          }
          frame #2 {
            n812 = property on="R steps/rev" class="DigNum (strict)"() -> ("Value"=w1723:u32)  [unwired: 2 in, 2 out]
            n813 = property on="R offset deg" class="DigNum (strict)"() -> ("Value"=w1720:dbl)  [unwired: 2 in, 2 out]
            n814 = To Double Precision Float(number=w1723) -> (double precision float=w1726:dbl)
            n815 = call "mDrive Send Command.vi"("error in (no error)"=w1735, "Extra"="P", "Command"=T10."Print Parameter", "VISA resource name"=w1732) -> ("error out"=w1730:errorcluster, "read buffer"=w1725:string, "VISA resource name out"=w1731:refnum<visa-resource-name>)  [unwired: 3 in]
            n816 = Decimal String To Number(string=w1725, offset=0) -> (number=w1722:i32)  [unwired: 1 in, 1 out]
            n817 = property on="R Step PV" class="DigNum (strict)"("Val(Sgnl)"=w1722) -> ()  [unwired: 2 in, 2 out]
            n818 = To Double Precision Float(number=w1722) -> (double precision float=w1727:dbl)
            n819 = Divide(x=w1727, y=w1726) -> (x/y=w1729:dbl)
            n820 = property on="R deg/rev" class="DigNum (strict)"() -> ("Value"=w1721:dbl)  [unwired: 2 in, 2 out]
            n821 = Multiply(x=w1729, y=w1721) -> (x*y=w1728:dbl)
            n822 = Add(x=w1728, y=w1720) -> (x+y=w1719:dbl)
            n823 = property on="R Position deg PV" class="DigNum (strict)"("Val(Sgnl)"=w1719) -> ()  [unwired: 2 in, 2 out]
          }
        }
        n824 = flat-sequence {
          tunnel: w1709 -> [w1764]
          tunnel: [w1763] -> w1703
          tunnel: w1692 -> [w1762]
          tunnel: [w1761] -> w1690
          tunnel: [w1768] -> w1704
          tunnel: w1703 -> [w1768]
          tunnel: [w1767] -> w1691
          tunnel: w1690 -> [w1767]
          tunnel: w1704 -> [w1785]
          tunnel: w1691 -> [w1782]
          tunnel: [w1781] -> _
          tunnel: [w1780] -> _
          frame #0 {
            n825 = call "mDrive Send Command.vi"("error in (no error)"=w1764, "Command"=T10."Stop", "VISA resource name"=w1762) -> ("error out"=w1763:errorcluster, "VISA resource name out"=w1761:refnum<visa-resource-name>)  [unwired: 4 in, 1 out]
          }
          frame #1 {
            n826 = Wait (ms)(milliseconds to wait=u32 50) -> ()  [unwired: 1 out]
          }
          frame #2 {
            n827 = property on="Z steps/rev" class="DigNum (strict)"() -> ("Value"=w1771:u32)  [unwired: 2 in, 2 out]
            n828 = property on="Z offset mm" class="DigNum (strict)"() -> ("Value"=w1769:dbl)  [unwired: 2 in, 2 out]
            n829 = To Double Precision Float(number=w1771) -> (double precision float=w1776:dbl)
            n830 = call "mDrive Send Command.vi"("error in (no error)"=w1785, "Extra"="P", "Command"=T10."Print Parameter", "VISA resource name"=w1782) -> ("error out"=w1780:errorcluster, "read buffer"=w1775:string, "VISA resource name out"=w1781:refnum<visa-resource-name>)  [unwired: 3 in]
            n831 = Decimal String To Number(string=w1775, offset=0) -> (number=w1773:i32)  [unwired: 1 in, 1 out]
            n832 = property on="Z Step PV" class="DigNum (strict)"("Val(Sgnl)"=w1773) -> ()  [unwired: 2 in, 2 out]
            n833 = To Double Precision Float(number=w1773) -> (double precision float=w1777:dbl)
            n834 = Divide(x=w1777, y=w1776) -> (x/y=w1779:dbl)
            n835 = property on="Z mm/rev" class="DigNum (strict)"() -> ("Value"=w1770:dbl)  [unwired: 2 in, 2 out]
            n836 = Multiply(x=w1779, y=w1770) -> (x*y=w1778:dbl)
            n837 = Add(x=w1778, y=w1769) -> (x+y=w1772:dbl)
            n838 = property on="Z Position mm PV" class="DigNum (strict)"("Val(Sgnl)"=w1772) -> ()  [unwired: 2 in, 2 out]
          }
        }
        n839 = flat-sequence {
          tunnel: w1708 -> [w1789]
          tunnel: [w1788] -> w1701
          tunnel: w1695 -> [w1787]
          tunnel: [w1786] -> w1693
          tunnel: [w1793] -> w1702
          tunnel: w1701 -> [w1793]
          tunnel: [w1792] -> w1694
          tunnel: w1693 -> [w1792]
          tunnel: w1702 -> [w1810]
          tunnel: w1694 -> [w1807]
          tunnel: [w1806] -> _
          tunnel: [w1805] -> _
          frame #0 {
            n840 = call "mDrive Send Command.vi"("error in (no error)"=w1789, "Command"=T10."Stop", "VISA resource name"=w1787) -> ("error out"=w1788:errorcluster, "VISA resource name out"=w1786:refnum<visa-resource-name>)  [unwired: 4 in, 1 out]
          }
          frame #1 {
            n841 = Wait (ms)(milliseconds to wait=u32 50) -> ()  [unwired: 1 out]
          }
          frame #2 {
            n842 = property on="Y steps/rev" class="DigNum (strict)"() -> ("Value"=w1796:u32)  [unwired: 2 in, 2 out]
            n843 = property on="Y offset mm" class="DigNum (strict)"() -> ("Value"=w1794:dbl)  [unwired: 2 in, 2 out]
            n844 = To Double Precision Float(number=w1796) -> (double precision float=w1801:dbl)
            n845 = call "mDrive Send Command.vi"("error in (no error)"=w1810, "Extra"="P", "Command"=T10."Print Parameter", "VISA resource name"=w1807) -> ("error out"=w1805:errorcluster, "read buffer"=w1800:string, "VISA resource name out"=w1806:refnum<visa-resource-name>)  [unwired: 3 in]
            n846 = Decimal String To Number(string=w1800, offset=0) -> (number=w1797:i32)  [unwired: 1 in, 1 out]
            n847 = property on="Y Step PV" class="DigNum (strict)"("Val(Sgnl)"=w1797) -> ()  [unwired: 2 in, 2 out]
            n848 = To Double Precision Float(number=w1797) -> (double precision float=w1802:dbl)
            n849 = Divide(x=w1802, y=w1801) -> (x/y=w1804:dbl)
            n850 = property on="Y mm/rev" class="DigNum (strict)"() -> ("Value"=w1795:dbl)  [unwired: 2 in, 2 out]
            n851 = Multiply(x=w1804, y=w1795) -> (x*y=w1803:dbl)
            n852 = Add(x=w1803, y=w1794) -> (x+y=w1798:dbl)
            n853 = property on="Y Position mm PV" class="DigNum (strict)"("Val(Sgnl)"=w1798) -> ()  [unwired: 2 in, 2 out]
          }
        }
      }
      event #4 {
        n854 = event-data() -> ()  [unwired: 1 in, 5 out]
        n855 = property on="Y steps/rev" class="DigNum (strict)"() -> ("Value"=w1841:u32)  [unwired: 2 in, 2 out]
        n856 = property on="X steps/rev" class="DigNum (strict)"() -> ("Value"=w1832:u32)  [unwired: 2 in, 2 out]
        n857 = property on="Z steps/rev" class="DigNum (strict)"() -> ("Value"=w1823:u32)  [unwired: 2 in, 2 out]
        n858 = property on="R steps/rev" class="DigNum (strict)"() -> ("Value"=w1814:u32)  [unwired: 2 in, 2 out]
        n859 = property on="R offset deg" class="DigNum (strict)"() -> ("Value"=w1812:dbl)  [unwired: 2 in, 2 out]
        n860 = property on="Y offset mm" class="DigNum (strict)"() -> ("Value"=w1839:dbl)  [unwired: 2 in, 2 out]
        n861 = property on="X offset mm" class="DigNum (strict)"() -> ("Value"=w1830:dbl)  [unwired: 2 in, 2 out]
        n862 = property on="Z offset mm" class="DigNum (strict)"() -> ("Value"=w1821:dbl)  [unwired: 2 in, 2 out]
        n863 = To Double Precision Float(number=w1814) -> (double precision float=w1817:dbl)
        n864 = To Double Precision Float(number=w1832) -> (double precision float=w1835:dbl)
        n865 = To Double Precision Float(number=w1823) -> (double precision float=w1826:dbl)
        n866 = property on="Reset Y Position mm" class="DigNum (strict)"() -> ("Value"=w1847:dbl)  [unwired: 2 in, 2 out]
        n867 = property on="Reset X Position mm" class="DigNum (strict)"() -> ("Value"=w1838:dbl)  [unwired: 2 in, 2 out]
        n868 = property on="Reset Z Position mm" class="DigNum (strict)"() -> ("Value"=w1829:dbl)  [unwired: 2 in, 2 out]
        n869 = property on="Reset R Position deg" class="DigNum (strict)"() -> ("Value"=w1820:dbl)  [unwired: 2 in, 2 out]
        n870 = local write "STATUS"("RESSETTING" ("STATUS")) -> ()
        n871 = Subtract(x=w1847, y=w1839) -> (x-y=w1846:dbl)
        n872 = Subtract(x=w1820, y=w1812) -> (x-y=w1819:dbl)
        n873 = Subtract(x=w1838, y=w1830) -> (x-y=w1837:dbl)
        n874 = Subtract(x=w1829, y=w1821) -> (x-y=w1828:dbl)
        n875 = property on="Y mm/rev" class="DigNum (strict)"() -> ("Value"=w1840:dbl)  [unwired: 2 in, 2 out]
        n876 = property on="X mm/rev" class="DigNum (strict)"() -> ("Value"=w1831:dbl)  [unwired: 2 in, 2 out]
        n877 = property on="Z mm/rev" class="DigNum (strict)"() -> ("Value"=w1822:dbl)  [unwired: 2 in, 2 out]
        n878 = property on="R deg/rev" class="DigNum (strict)"() -> ("Value"=w1813:dbl)  [unwired: 2 in, 2 out]
        n879 = Divide(x=w1819, y=w1813) -> (x/y=w1818:dbl)
        n880 = Divide(x=w1837, y=w1831) -> (x/y=w1836:dbl)
        n881 = Divide(x=w1828, y=w1822) -> (x/y=w1827:dbl)
        n882 = Divide(x=w1846, y=w1840) -> (x/y=w1845:dbl)
        n883 = To Double Precision Float(number=w1841) -> (double precision float=w1844:dbl)
        n884 = Multiply(x=w1845, y=w1844) -> (x*y=w1843:dbl)
        n885 = Multiply(x=w1818, y=w1817) -> (x*y=w1816:dbl)
        n886 = Multiply(x=w1836, y=w1835) -> (x*y=w1834:dbl)
        n887 = Multiply(x=w1827, y=w1826) -> (x*y=w1825:dbl)
        n888 = To Long Integer(number=w1843) -> (32bit integer=w1842:i32)
        n889 = To Long Integer(number=w1816) -> (32bit integer=w1815:i32)
        n890 = To Long Integer(number=w1834) -> (32bit integer=w1833:i32)
        n891 = To Long Integer(number=w1825) -> (32bit integer=w1824:i32)
        n892 = property on="Reset Y Motor Steps" class="DigNum (strict)"("Val(Sgnl)"=w1842) -> ()  [unwired: 2 in, 2 out]
        n893 = property on="Reset R Motor Steps" class="DigNum (strict)"("Val(Sgnl)"=w1815) -> ()  [unwired: 2 in, 2 out]
        n894 = property on="Reset X Motor Steps" class="DigNum (strict)"("Val(Sgnl)"=w1833) -> ()  [unwired: 2 in, 2 out]
        n895 = property on="Reset Z Motor Steps" class="DigNum (strict)"("Val(Sgnl)"=w1824) -> ()  [unwired: 2 in, 2 out]
      }
      event #5 {
        n896 = event-data() -> ()  [unwired: 1 in, 5 out]
        n897 = property on="X Step SP" class="DigNum (strict)"() -> ("Value"=w1872:i32)  [unwired: 2 in, 2 out]
        n898 = property on="Z Step SP" class="DigNum (strict)"() -> ("Value"=w1864:i32)  [unwired: 2 in, 2 out]
        n899 = property on="Y Step SP" class="DigNum (strict)"() -> ("Value"=w1880:i32)  [unwired: 2 in, 2 out]
        n900 = property on="X steps/rev" class="DigNum (strict)"() -> ("Value"=w1897:u32)  [unwired: 2 in, 2 out]
        n901 = property on="X steps/rev" class="DigNum (strict)"() -> ("Value"=w1870:u32)  [unwired: 2 in, 2 out]
        n902 = property on="R Step SP" class="DigNum (strict)"() -> ("Value"=w1856:i32)  [unwired: 2 in, 2 out]
        n903 = property on="Z steps/rev" class="DigNum (strict)"() -> ("Value"=w1891:u32)  [unwired: 2 in, 2 out]
        n904 = property on="Z steps/rev" class="DigNum (strict)"() -> ("Value"=w1862:u32)  [unwired: 2 in, 2 out]
        n905 = property on="Y steps/rev" class="DigNum (strict)"() -> ("Value"=w1903:u32)  [unwired: 2 in, 2 out]
        n906 = property on="Y steps/rev" class="DigNum (strict)"() -> ("Value"=w1878:u32)  [unwired: 2 in, 2 out]
        n907 = property on="R steps/rev" class="DigNum (strict)"() -> ("Value"=w1885:u32)  [unwired: 2 in, 2 out]
        n908 = property on="R steps/rev" class="DigNum (strict)"() -> ("Value"=w1854:u32)  [unwired: 2 in, 2 out]
        n909 = property on="R offset deg" class="DigNum (strict)"() -> ("Value"=w1853:dbl)  [unwired: 2 in, 2 out]
        n910 = property on="X offset mm" class="DigNum (strict)"() -> ("Value"=w1869:dbl)  [unwired: 2 in, 2 out]
        n911 = property on="Z offset mm" class="DigNum (strict)"() -> ("Value"=w1861:dbl)  [unwired: 2 in, 2 out]
        n912 = property on="Y offset mm" class="DigNum (strict)"() -> ("Value"=w1877:dbl)  [unwired: 2 in, 2 out]
        n913 = To Double Precision Float(number=w1897) -> (double precision float=w1902:dbl)
        n914 = To Double Precision Float(number=w1872) -> (double precision float=w1873:dbl)
        n915 = To Double Precision Float(number=w1870) -> (double precision float=w1876:dbl)
        n916 = To Double Precision Float(number=w1885) -> (double precision float=w1890:dbl)
        n917 = To Double Precision Float(number=w1856) -> (double precision float=w1857:dbl)
        n918 = To Double Precision Float(number=w1854) -> (double precision float=w1860:dbl)
        n919 = To Double Precision Float(number=w1891) -> (double precision float=w1896:dbl)
        n920 = To Double Precision Float(number=w1864) -> (double precision float=w1865:dbl)
        n921 = To Double Precision Float(number=w1862) -> (double precision float=w1868:dbl)
        n922 = To Double Precision Float(number=w1903) -> (double precision float=w1908:dbl)
        n923 = To Double Precision Float(number=w1880) -> (double precision float=w1881:dbl)
        n924 = To Double Precision Float(number=w1878) -> (double precision float=w1884:dbl)
        n925 = Divide(x=w1873, y=w1876) -> (x/y=w1875:dbl)
        n926 = Divide(x=w1865, y=w1868) -> (x/y=w1867:dbl)
        n927 = Divide(x=w1881, y=w1884) -> (x/y=w1883:dbl)
        n928 = Divide(x=w1857, y=w1860) -> (x/y=w1859:dbl)
        n929 = property on="X Velocity SP step/sec" class="DigNum (strict)"() -> ("Value"=w1899:i32)  [unwired: 2 in, 2 out]
        n930 = property on="X mm/rev" class="DigNum (strict)"() -> ("Value"=w1850:dbl)  [unwired: 2 in, 2 out]
        n931 = property on="Z Velocity SP step/sec" class="DigNum (strict)"() -> ("Value"=w1893:i32)  [unwired: 2 in, 2 out]
        n932 = property on="Z mm/rev" class="DigNum (strict)"() -> ("Value"=w1851:dbl)  [unwired: 2 in, 2 out]
        n933 = property on="Y Velocity SP step/sec" class="DigNum (strict)"() -> ("Value"=w1905:i32)  [unwired: 2 in, 2 out]
        n934 = property on="Y mm/rev" class="DigNum (strict)"() -> ("Value"=w1849:dbl)  [unwired: 2 in, 2 out]
        n935 = property on="R Velocity SP step/sec" class="DigNum (strict)"() -> ("Value"=w1887:i32)  [unwired: 2 in, 2 out]
        n936 = property on="R deg/rev" class="DigNum (strict)"() -> ("Value"=w1852:dbl)  [unwired: 2 in, 2 out]
        n937 = Multiply(x=w1875, y=w1850) -> (x*y=w1874:dbl)
        n938 = Multiply(x=w1859, y=w1852) -> (x*y=w1858:dbl)
        n939 = Multiply(x=w1867, y=w1851) -> (x*y=w1866:dbl)
        n940 = Multiply(x=w1883, y=w1849) -> (x*y=w1882:dbl)
        n941 = To Double Precision Float(number=w1899) -> (double precision float=w1900:dbl)
        n942 = To Double Precision Float(number=w1887) -> (double precision float=w1888:dbl)
        n943 = To Double Precision Float(number=w1893) -> (double precision float=w1894:dbl)
        n944 = To Double Precision Float(number=w1905) -> (double precision float=w1906:dbl)
        n945 = Divide(x=w1900, y=w1902) -> (x/y=w1901:dbl)
        n946 = Add(x=w1874, y=w1869) -> (x+y=w1871:dbl)
        n947 = Divide(x=w1888, y=w1890) -> (x/y=w1889:dbl)
        n948 = Add(x=w1858, y=w1853) -> (x+y=w1855:dbl)
        n949 = Divide(x=w1894, y=w1896) -> (x/y=w1895:dbl)
        n950 = Add(x=w1866, y=w1861) -> (x+y=w1863:dbl)
        n951 = Divide(x=w1906, y=w1908) -> (x/y=w1907:dbl)
        n952 = Add(x=w1882, y=w1877) -> (x+y=w1879:dbl)
        n953 = Multiply(x=w1901, y=w1850) -> (x*y=w1898:dbl)
        n954 = Multiply(x=w1889, y=w1852) -> (x*y=w1886:dbl)
        n955 = Multiply(x=w1895, y=w1851) -> (x*y=w1892:dbl)
        n956 = Multiply(x=w1907, y=w1849) -> (x*y=w1904:dbl)
        n957 = property on="X Position MV mm" class="DigNum (strict)"("Val(Sgnl)"=w1871) -> ()  [unwired: 2 in, 2 out]
        n958 = property on="R Position MV deg" class="DigNum (strict)"("Val(Sgnl)"=w1855) -> ()  [unwired: 2 in, 2 out]
        n959 = property on="Z Position MV mm" class="DigNum (strict)"("Val(Sgnl)"=w1863) -> ()  [unwired: 2 in, 2 out]
        n960 = property on="Y Position MV mm" class="DigNum (strict)"("Val(Sgnl)"=w1879) -> ()  [unwired: 2 in, 2 out]
        n961 = property on="X Velocity MV mm/sec" class="DigNum (strict)"("Val(Sgnl)"=w1898) -> ()  [unwired: 2 in, 2 out]
        n962 = property on="Z Velocity MV mm/sec" class="DigNum (strict)"("Val(Sgnl)"=w1892) -> ()  [unwired: 2 in, 2 out]
        n963 = property on="Y Velocity MV mm/sec" class="DigNum (strict)"("Val(Sgnl)"=w1904) -> ()  [unwired: 2 in, 2 out]
        n964 = Absolute Value(x=w1886) -> (abs(x)=w1848:dbl)
        n965 = property on="R Velocity MVdeg/sec" class="DigNum (strict)"("Val(Sgnl)"=w1848) -> ()  [unwired: 2 in, 2 out]
      }
      event #6 {
        n966 = event-data() -> ()  [unwired: 1 in, 5 out]
        n967 = property on="R Step PV" class="DigNum (strict)"() -> ("Value"=w1941:i32)  [unwired: 2 in, 2 out]
        n968 = property on="X steps/rev" class="DigNum (strict)"() -> ("Value"=w1982:u32)  [unwired: 2 in, 2 out]
        n969 = property on="Y steps/rev" class="DigNum (strict)"() -> ("Value"=w1970:u32)  [unwired: 2 in, 2 out]
        n970 = property on="Z steps/rev" class="DigNum (strict)"() -> ("Value"=w1957:u32)  [unwired: 2 in, 2 out]
        n971 = property on="X Step PV" class="DigNum (strict)"() -> ("Value"=w1981:i32)  [unwired: 2 in, 2 out]
        n972 = property on="Y Step PV" class="DigNum (strict)"() -> ("Value"=w1968:i32)  [unwired: 2 in, 2 out]
        n973 = property on="Z Step PV" class="DigNum (strict)"() -> ("Value"=w1955:i32)  [unwired: 2 in, 2 out]
        n974 = property on="R steps/rev" class="DigNum (strict)"() -> ("Value"=w1943:u32)  [unwired: 2 in, 2 out]
        n975 = To Double Precision Float(number=w1981) -> (double precision float=w1935:dbl)
        n976 = To Double Precision Float(number=w1968) -> (double precision float=w1934:dbl)
        n977 = To Double Precision Float(number=w1955) -> (double precision float=w1933:dbl)
        n978 = To Double Precision Float(number=w1941) -> (double precision float=w1932:dbl)
        n979 = To Double Precision Float(number=w1982) -> (double precision float=w1980:dbl)
        n980 = To Double Precision Float(number=w1970) -> (double precision float=w1925:dbl)
        n981 = To Double Precision Float(number=w1943) -> (double precision float=w1940:dbl)
        n982 = To Double Precision Float(number=w1957) -> (double precision float=w1954:dbl)
        n983 = property on="X Step SP" class="DigNum (strict)"() -> ("Maximum"=w1985:dbl)  [unwired: 2 in, 2 out]
        n984 = property on="Y Step SP" class="DigNum (strict)"() -> ("Maximum"=w1974:dbl)  [unwired: 2 in, 2 out]
        n985 = property on="Z Step SP" class="DigNum (strict)"() -> ("Maximum"=w1961:dbl)  [unwired: 2 in, 2 out]
        n986 = property on="R Step SP" class="DigNum (strict)"() -> ("Maximum"=w1949:dbl)  [unwired: 2 in, 2 out]
        n987 = property on="X Scan Length SP steps" class="DigNum (strict)"() -> ("Value"=w1979:i32)  [unwired: 2 in, 2 out]
        n988 = property on="X Scan Length SP mm" class="DigNum (strict)"() -> ("Value"=w1911:dbl)  [unwired: 2 in, 2 out]
        n989 = property on="Y Scan Length SP mm" class="DigNum (strict)"() -> ("Value"=w1912:dbl)  [unwired: 2 in, 2 out]
        n990 = property on="Y Scan Length SP steps" class="DigNum (strict)"() -> ("Value"=w1971:i32)  [unwired: 2 in, 2 out]
        n991 = property on="Z Scan Length SP steps" class="DigNum (strict)"() -> ("Value"=w1958:i32)  [unwired: 2 in, 2 out]
        n992 = property on="R Scan Length SP steps" class="DigNum (strict)"() -> ("Value"=w1944:i32)  [unwired: 2 in, 2 out]
        n993 = property on="X Step SP" class="DigNum (strict)"() -> ("Minimum"=w1986:dbl)  [unwired: 2 in, 2 out]
        n994 = property on="Y Step SP" class="DigNum (strict)"() -> ("Minimum"=w1975:dbl)  [unwired: 2 in, 2 out]
        n995 = property on="Z Step SP" class="DigNum (strict)"() -> ("Minimum"=w1962:dbl)  [unwired: 2 in, 2 out]
        n996 = property on="R Step SP" class="DigNum (strict)"() -> ("Minimum"=w1946:dbl)  [unwired: 2 in, 2 out]
        n997 = property on="Z Scan Velocity SP steps/sec" class="DigNum (strict)"() -> ("Value"=w1953:i32)  [unwired: 2 in, 2 out]
        n998 = property on="R Scan Velocity SP steps/sec" class="DigNum (strict)"() -> ("Value"=w1939:i32)  [unwired: 2 in, 2 out]
        n999 = Subtract(x=w1985, y=w1935) -> (x-y=w1984:dbl)
        n1000 = Subtract(x=w1986, y=w1935) -> (x-y=w1987:dbl)
        n1001 = Subtract(x=w1975, y=w1934) -> (x-y=w1976:dbl)
        n1002 = Subtract(x=w1974, y=w1934) -> (x-y=w1973:dbl)
        n1003 = Subtract(x=w1962, y=w1933) -> (x-y=w1963:dbl)
        n1004 = Subtract(x=w1961, y=w1933) -> (x-y=w1960:dbl)
        n1005 = Subtract(x=w1946, y=w1932) -> (x-y=w1947:dbl)
        n1006 = Subtract(x=w1949, y=w1932) -> (x-y=w1948:dbl)
        n1007 = To Double Precision Float(number=w1944) -> (double precision float=w1929:dbl)
        n1008 = To Double Precision Float(number=w1958) -> (double precision float=w1931:dbl)
        n1009 = To Double Precision Float(number=w1979) -> (double precision float=w1922:dbl)
        n1010 = To Double Precision Float(number=w1971) -> (double precision float=w1924:dbl)
        n1011 = property on="X Scan Velocity SP steps/sec" class="DigNum (strict)"() -> ("Value"=w1983:i32)  [unwired: 2 in, 2 out]
        n1012 = property on="Y Scan Velocity SP steps/sec" class="DigNum (strict)"() -> ("Value"=w1967:i32)  [unwired: 2 in, 2 out]
        n1013 = Equal?(x=w1911, y=0.0) -> (x = y?=w1909:bool)
        n1014 = Equal?(x=w1912, y=0.0) -> (x = y?=w1910:bool)
        n1015 = property on="X Scan Length SP steps" class="DigNum (strict)"("Maximum"=w1984) -> ()  [unwired: 2 in, 2 out]
        n1016 = property on="X Scan Length SP steps" class="DigNum (strict)"("Minimum"=w1987) -> ()  [unwired: 2 in, 2 out]
        n1017 = property on="Y Scan Length SP steps" class="DigNum (strict)"("Minimum"=w1976) -> ()  [unwired: 2 in, 2 out]
        n1018 = property on="Y Scan Length SP steps" class="DigNum (strict)"("Maximum"=w1973) -> ()  [unwired: 2 in, 2 out]
        n1019 = property on="Z Scan Length SP steps" class="DigNum (strict)"("Minimum"=w1963) -> ()  [unwired: 2 in, 2 out]
        n1020 = property on="Z Scan Length SP steps" class="DigNum (strict)"("Maximum"=w1960) -> ()  [unwired: 2 in, 2 out]
        n1021 = property on="R Scan Length SP steps" class="DigNum (strict)"("Minimum"=w1947) -> ()  [unwired: 2 in, 2 out]
        n1022 = property on="R Scan Length SP steps" class="DigNum (strict)"("Maximum"=w1948) -> ()  [unwired: 2 in, 2 out]
        n1023 = Divide(x=w1922, y=w1980) -> (x/y=w1917:dbl)
        n1024 = Divide(x=w1924, y=w1925) -> (x/y=w1972:dbl)
        n1025 = Divide(x=w1931, y=w1954) -> (x/y=w1959:dbl)
        n1026 = Divide(x=w1929, y=w1940) -> (x/y=w1945:dbl)
        n1027 = To Double Precision Float(number=w1983) -> (double precision float=w1921:dbl)
        n1028 = To Double Precision Float(number=w1967) -> (double precision float=w1923:dbl)
        n1029 = To Double Precision Float(number=w1953) -> (double precision float=w1930:dbl)
        n1030 = To Double Precision Float(number=w1939) -> (double precision float=w1928:dbl)
        n1031 = property on="X mm/rev" class="DigNum (strict)"() -> ("Value"=w1916:dbl)  [unwired: 2 in, 2 out]
        n1032 = property on="Y mm/rev" class="DigNum (strict)"() -> ("Value"=w1969:dbl)  [unwired: 2 in, 2 out]
        n1033 = property on="Z mm/rev" class="DigNum (strict)"() -> ("Value"=w1956:dbl)  [unwired: 2 in, 2 out]
        n1034 = property on="R deg/rev" class="DigNum (strict)"() -> ("Value"=w1942:dbl)  [unwired: 2 in, 2 out]
        n1035 = Multiply(x=w1917, y=w1916) -> (x*y=w1977:dbl)
        n1036 = Divide(x=w1921, y=w1980) -> (x/y=w1915:dbl)
        n1037 = Multiply(x=w1972, y=w1969) -> (x*y=w1965:dbl)
        n1038 = Divide(x=w1923, y=w1925) -> (x/y=w1966:dbl)
        n1039 = Divide(x=w1929, y=w1928) -> (x/y=w1927:dbl)
        n1040 = Multiply(x=w1945, y=w1942) -> (x*y=w1937:dbl)
        n1041 = Divide(x=w1928, y=w1940) -> (x/y=w1938:dbl)
        n1042 = Multiply(x=w1959, y=w1956) -> (x*y=w1951:dbl)
        n1043 = Divide(x=w1931, y=w1930) -> (x/y=w1926:dbl)
        n1044 = Divide(x=w1930, y=w1954) -> (x/y=w1952:dbl)
        n1045 = case shown="True" w1909 {
          tunnel: w1922 -> [w1990 _]
          tunnel: w1921 -> [w1989 _]
          frame #0 {
            n1046 = Divide(x=w1990, y=w1989) -> (x/y=w1991:dbl)
            n1047 = Absolute Value(x=w1991) -> (abs(x)=→"X Scan Duration":dbl)
          }
          frame #1 {
            n1048 = local write "X Scan Duration"(0.0 ("X Scan Duration")) -> ()
          }
        }
        n1049 = case shown="True" w1910 {
          tunnel: w1924 -> [w1996 _]
          tunnel: w1923 -> [w1995 _]
          frame #0 {
            n1050 = Divide(x=w1996, y=w1995) -> (x/y=w1994:dbl)
            n1051 = Absolute Value(x=w1994) -> (abs(x)=→"Y Scan Duration":dbl)
          }
          frame #1 {
            n1052 = local write "Y Scan Duration"(0.0 ("Y Scan Duration")) -> ()
          }
        }
        n1053 = Multiply(x=w1916, y=w1915) -> (x*y=w1978:dbl)
        n1054 = Multiply(x=w1969, y=w1966) -> (x*y=w1964:dbl)
        n1055 = Multiply(x=w1942, y=w1938) -> (x*y=w1936:dbl)
        n1056 = Multiply(x=w1956, y=w1952) -> (x*y=w1950:dbl)
        n1057 = Absolute Value(x=w1927) -> (abs(x)=→"R Scan Duration":dbl)
        n1058 = Absolute Value(x=w1926) -> (abs(x)=→"Z Scan Duration":dbl)
        n1059 = property on="X Scan length MV mm" class="DigNum (strict)"("Val(Sgnl)"=w1977) -> ()  [unwired: 2 in, 2 out]
        n1060 = property on="Y Scan length MV mm" class="DigNum (strict)"("Value"=w1965) -> ()  [unwired: 2 in, 2 out]
        n1061 = property on="R Scan length MV deg" class="DigNum (strict)"("Value"=w1937) -> ()  [unwired: 2 in, 2 out]
        n1062 = property on="Z Scan length MV mm" class="DigNum (strict)"("Value"=w1951) -> ()  [unwired: 2 in, 2 out]
        n1063 = Absolute Value(x=w1936) -> (abs(x)=w1920:dbl)
        n1064 = property on="X Scan velocity MV mm/sec" class="DigNum (strict)"("Value"=w1978) -> ()  [unwired: 2 in, 2 out]
        n1065 = property on="Y Scan velocity MV mm/sec" class="DigNum (strict)"("Val(Sgnl)"=w1964) -> ()  [unwired: 2 in, 2 out]
        n1066 = property on="Z Scan velocity MV mm/sec" class="DigNum (strict)"("Val(Sgnl)"=w1950) -> ()  [unwired: 2 in, 2 out]
        n1067 = property on="R Scan Velocity SP deg/sec" class="DigNum (strict)"("Val(Sgnl)"=w1920) -> ()  [unwired: 2 in, 2 out]
      }
      event #7 {
        n1068 = event-data() -> ()  [unwired: 1 in, 7 out]
        n1069 = property on="Y steps/rev" class="DigNum (strict)"() -> ("Value"=w2016:u32)  [unwired: 2 in, 2 out]
        n1070 = Wait (ms)(milliseconds to wait=u32 100) -> ()  [unwired: 1 out]
        n1071 = To Double Precision Float(number=w2016) -> (double precision float=w2001:dbl)
        n1072 = property on="Y offset mm" class="DigNum (strict)"() -> ("Value"=w2014:dbl)  [unwired: 2 in, 2 out]
        n1073 = property on="Y Position SP mm" class="DigNum (strict)"() -> ("Value"=w2013:dbl)  [unwired: 2 in, 2 out]
        n1074 = property on="Y Velocity SP step/sec" class="DigNum (strict)"() -> ("Maximum"=w2003:dbl)  [unwired: 2 in, 2 out]
        n1075 = local write "STATUS"("SETTING Y" ("STATUS")) -> ()
        n1076 = property on="Y Velocity SP step/sec" class="DigNum (strict)"() -> ("Minimum"=w2002:dbl)  [unwired: 2 in, 2 out]
        n1077 = Subtract(x=w2013, y=w2014) -> (x-y=w2017:dbl)
        n1078 = property on="Y Velocity SP mm/sec" class="DigNum (strict)"() -> ("Value"=w2007:dbl)  [unwired: 2 in, 2 out]
        n1079 = property on="Y mm/rev" class="DigNum (strict)"() -> ("Value"=w2000:dbl)  [unwired: 2 in, 2 out]
        n1080 = Divide(x=w2017, y=w2000) -> (x/y=w2018:dbl)
        n1081 = Divide(x=w2007, y=w2000) -> (x/y=w2008:dbl)
        n1082 = Multiply(x=w2018, y=w2001) -> (x*y=w2012:dbl)
        n1083 = Multiply(x=w2008, y=w2001) -> (x*y=w2005:dbl)
        n1084 = In Range and Coerce(upper limit=w2003, x=w2005, lower limit=w2002) -> (coerced(x)=w2004:dbl)  [unwired: 1 out]
        n1085 = property on="Y Step SP" class="DigNum (strict)"() -> ("Maximum"=w2010:dbl)  [unwired: 2 in, 2 out]
        n1086 = property on="Y Step SP" class="DigNum (strict)"() -> ("Minimum"=w2009:dbl)  [unwired: 2 in, 2 out]
        n1087 = To Long Integer(number=w2004) -> (32bit integer=w2006:i32)
        n1088 = In Range and Coerce(upper limit=w2010, x=w2012, lower limit=w2009) -> (coerced(x)=w2011:dbl)  [unwired: 1 out]
        n1089 = To Long Integer(number=w2011) -> (32bit integer=w2015:i32)
        n1090 = property on="Y Velocity SP step/sec" class="DigNum (strict)"("Val(Sgnl)"=w2006) -> ()  [unwired: 2 in, 2 out]
        n1091 = property on="Y Step SP" class="DigNum (strict)"("Val(Sgnl)"=w2015) -> ()  [unwired: 2 in, 2 out]
      }
      event #8 {
        n1092 = event-data() -> ()  [unwired: 1 in, 7 out]
        n1093 = property on="X steps/rev" class="DigNum (strict)"() -> ("Value"=w2037:u32)  [unwired: 2 in, 2 out]
        n1094 = Wait (ms)(milliseconds to wait=u32 100) -> ()  [unwired: 1 out]
        n1095 = property on="X offset mm" class="DigNum (strict)"() -> ("Value"=w2035:dbl)  [unwired: 2 in, 2 out]
        n1096 = property on="X Position SP mm" class="DigNum (strict)"() -> ("Value"=w2034:dbl)  [unwired: 2 in, 2 out]
        n1097 = property on="X Velocity SP step/sec" class="DigNum (strict)"() -> ("Maximum"=w2024:dbl)  [unwired: 2 in, 2 out]
        n1098 = local write "STATUS"("SETTING X" ("STATUS")) -> ()
        n1099 = property on="X Velocity SP step/sec" class="DigNum (strict)"() -> ("Minimum"=w2023:dbl)  [unwired: 2 in, 2 out]
        n1100 = Subtract(x=w2034, y=w2035) -> (x-y=w2038:dbl)
        n1101 = property on="X Velocity SP mm/sec" class="DigNum (strict)"() -> ("Value"=w2028:dbl)  [unwired: 2 in, 2 out]
        n1102 = property on="X mm/rev" class="DigNum (strict)"() -> ("Value"=w2021:dbl)  [unwired: 2 in, 2 out]
        n1103 = Divide(x=w2038, y=w2021) -> (x/y=w2039:dbl)
        n1104 = Divide(x=w2028, y=w2021) -> (x/y=w2029:dbl)
        n1105 = To Double Precision Float(number=w2037) -> (double precision float=w2022:dbl)
        n1106 = Multiply(x=w2039, y=w2022) -> (x*y=w2033:dbl)
        n1107 = Multiply(x=w2029, y=w2022) -> (x*y=w2026:dbl)
        n1108 = In Range and Coerce(upper limit=w2024, x=w2026, lower limit=w2023) -> (coerced(x)=w2025:dbl)  [unwired: 1 out]
        n1109 = property on="X Step SP" class="DigNum (strict)"() -> ("Maximum"=w2031:dbl)  [unwired: 2 in, 2 out]
        n1110 = property on="X Step SP" class="DigNum (strict)"() -> ("Minimum"=w2030:dbl)  [unwired: 2 in, 2 out]
        n1111 = To Long Integer(number=w2025) -> (32bit integer=w2027:i32)
        n1112 = In Range and Coerce(upper limit=w2031, x=w2033, lower limit=w2030) -> (coerced(x)=w2032:dbl)  [unwired: 1 out]
        n1113 = To Long Integer(number=w2032) -> (32bit integer=w2036:i32)
        n1114 = property on="X Velocity SP step/sec" class="DigNum (strict)"("Val(Sgnl)"=w2027) -> ()  [unwired: 2 in, 2 out]
        n1115 = property on="X Step SP" class="DigNum (strict)"("Val(Sgnl)"=w2036) -> ()  [unwired: 2 in, 2 out]
      }
      event #9 {
        n1116 = event-data() -> ()  [unwired: 1 in, 7 out]
        n1117 = property on="Z steps/rev" class="DigNum (strict)"() -> ("Value"=w2056:u32)  [unwired: 2 in, 2 out]
        n1118 = Wait (ms)(milliseconds to wait=u32 100) -> ()  [unwired: 1 out]
        n1119 = property on="Z offset mm" class="DigNum (strict)"() -> ("Value"=w2054:dbl)  [unwired: 2 in, 2 out]
        n1120 = property on="Z Position SP mm" class="DigNum (strict)"() -> ("Value"=w2053:dbl)  [unwired: 2 in, 2 out]
        n1121 = property on="Z Velocity SP step/sec" class="DigNum (strict)"() -> ("Maximum"=w2043:dbl)  [unwired: 2 in, 2 out]
        n1122 = local write "STATUS"("SETTING Z" ("STATUS")) -> ()
        n1123 = property on="Z Velocity SP step/sec" class="DigNum (strict)"() -> ("Minimum"=w2042:dbl)  [unwired: 2 in, 2 out]
        n1124 = Subtract(x=w2053, y=w2054) -> (x-y=w2057:dbl)
        n1125 = property on="Z Velocity SP mm/sec" class="DigNum (strict)"() -> ("Value"=w2047:dbl)  [unwired: 2 in, 2 out]
        n1126 = property on="Z mm/rev" class="DigNum (strict)"() -> ("Value"=w2059:dbl)  [unwired: 2 in, 2 out]
        n1127 = Divide(x=w2057, y=w2059) -> (x/y=w2058:dbl)
        n1128 = Divide(x=w2047, y=w2059) -> (x/y=w2048:dbl)
        n1129 = To Double Precision Float(number=w2056) -> (double precision float=w2060:dbl)
        n1130 = Multiply(x=w2058, y=w2060) -> (x*y=w2052:dbl)
        n1131 = Multiply(x=w2048, y=w2060) -> (x*y=w2045:dbl)
        n1132 = In Range and Coerce(upper limit=w2043, x=w2045, lower limit=w2042) -> (coerced(x)=w2044:dbl)  [unwired: 1 out]
        n1133 = property on="Z Step SP" class="DigNum (strict)"() -> ("Maximum"=w2050:dbl)  [unwired: 2 in, 2 out]
        n1134 = property on="Z Step SP" class="DigNum (strict)"() -> ("Minimum"=w2049:dbl)  [unwired: 2 in, 2 out]
        n1135 = To Long Integer(number=w2044) -> (32bit integer=w2046:i32)
        n1136 = In Range and Coerce(upper limit=w2050, x=w2052, lower limit=w2049) -> (coerced(x)=w2051:dbl)  [unwired: 1 out]
        n1137 = To Long Integer(number=w2051) -> (32bit integer=w2055:i32)
        n1138 = property on="Z Velocity SP step/sec" class="DigNum (strict)"("Val(Sgnl)"=w2046) -> ()  [unwired: 2 in, 2 out]
        n1139 = property on="Z Step SP" class="DigNum (strict)"("Val(Sgnl)"=w2055) -> ()  [unwired: 2 in, 2 out]
      }
      event #10 {
        n1140 = event-data() -> ()  [unwired: 1 in, 7 out]
        n1141 = property on="R steps/rev" class="DigNum (strict)"() -> ("Value"=w2080:u32)  [unwired: 2 in, 2 out]
        n1142 = Wait (ms)(milliseconds to wait=u32 100) -> ()  [unwired: 1 out]
        n1143 = property on="R offset deg" class="DigNum (strict)"() -> ("Value"=w2078:dbl)  [unwired: 2 in, 2 out]
        n1144 = property on="R Position SP deg" class="DigNum (strict)"() -> ("Value"=w2077:dbl)  [unwired: 2 in, 2 out]
        n1145 = property on="R Velocity SP step/sec" class="DigNum (strict)"() -> ("Maximum"=w2067:dbl)  [unwired: 2 in, 2 out]
        n1146 = local write "STATUS"("SETTING R" ("STATUS")) -> ()
        n1147 = property on="R Velocity SP step/sec" class="DigNum (strict)"() -> ("Minimum"=w2066:dbl)  [unwired: 2 in, 2 out]
        n1148 = Subtract(x=w2077, y=w2078) -> (x-y=w2081:dbl)
        n1149 = property on="R Velocity SP deg/sec" class="DigNum (strict)"() -> ("Value"=w2071:dbl)  [unwired: 2 in, 2 out]
        n1150 = property on="R deg/rev" class="DigNum (strict)"() -> ("Value"=w2064:dbl)  [unwired: 2 in, 2 out]
        n1151 = Divide(x=w2081, y=w2064) -> (x/y=w2082:dbl)
        n1152 = Divide(x=w2071, y=w2064) -> (x/y=w2072:dbl)
        n1153 = To Double Precision Float(number=w2080) -> (double precision float=w2065:dbl)
        n1154 = Multiply(x=w2082, y=w2065) -> (x*y=w2076:dbl)
        n1155 = Multiply(x=w2072, y=w2065) -> (x*y=w2069:dbl)
        n1156 = property on="R Step SP" class="DigNum (strict)"() -> ("Maximum"=w2074:dbl)  [unwired: 2 in, 2 out]
        n1157 = property on="R Step SP" class="DigNum (strict)"() -> ("Minimum"=w2073:dbl)  [unwired: 2 in, 2 out]
        n1158 = Absolute Value(x=w2069) -> (abs(x)=w2063:dbl)
        n1159 = In Range and Coerce(upper limit=w2074, x=w2076, lower limit=w2073) -> (coerced(x)=w2075:dbl)  [unwired: 1 out]
        n1160 = In Range and Coerce(upper limit=w2067, x=w2063, lower limit=w2066) -> (coerced(x)=w2068:dbl)  [unwired: 1 out]
        n1161 = To Long Integer(number=w2075) -> (32bit integer=w2079:i32)
        n1162 = To Long Integer(number=w2068) -> (32bit integer=w2070:i32)
        n1163 = property on="R Step SP" class="DigNum (strict)"("Val(Sgnl)"=w2079) -> ()  [unwired: 2 in, 2 out]
        n1164 = property on="R Velocity SP step/sec" class="DigNum (strict)"("Val(Sgnl)"=w2070) -> ()  [unwired: 2 in, 2 out]
      }
      event #11 {
        n1165 = event-data() -> ()  [unwired: 1 in, 7 out]
        n1166 = flat-sequence {
          frame #0 {
            n1167 = property on="Z steps/rev" class="DigNum (strict)"() -> ("Value"=w2151:u32)  [unwired: 2 in, 2 out]
            n1168 = property on="X steps/rev" class="DigNum (strict)"() -> ("Value"=w2134:u32)  [unwired: 2 in, 2 out]
            n1169 = property on="Y steps/rev" class="DigNum (strict)"() -> ("Value"=w2099:u32)  [unwired: 2 in, 2 out]
            n1170 = property on="R steps/rev" class="DigNum (strict)"() -> ("Value"=w2117:u32)  [unwired: 2 in, 2 out]
            n1171 = To Double Precision Float(number=w2151) -> (double precision float=w2137:dbl)
            n1172 = To Double Precision Float(number=w2134) -> (double precision float=w2120:dbl)
            n1173 = To Double Precision Float(number=w2099) -> (double precision float=w2085:dbl)
            n1174 = To Double Precision Float(number=w2117) -> (double precision float=w2103:dbl)
            n1175 = property on="R Velocity SP step/sec" class="DigNum (strict)"() -> ("Maximum"=w2105:dbl)  [unwired: 2 in, 2 out]
            n1176 = property on="Z mm/rev" class="DigNum (strict)"() -> ("Value"=w2136:dbl)  [unwired: 2 in, 2 out]
            n1177 = property on="X mm/rev" class="DigNum (strict)"() -> ("Value"=w2119:dbl)  [unwired: 2 in, 2 out]
            n1178 = property on="Y mm/rev" class="DigNum (strict)"() -> ("Value"=w2084:dbl)  [unwired: 2 in, 2 out]
            n1179 = property on="Z Scan Length SP mm" class="DigNum (strict)"() -> ("Value"=w2149:dbl)  [unwired: 2 in, 2 out]
            n1180 = property on="Z Scan Velocity SP mm/sec" class="DigNum (strict)"() -> ("Value"=w2143:dbl)  [unwired: 2 in, 2 out]
            n1181 = property on="X Scan Length SP mm" class="DigNum (strict)"() -> ("Value"=w2132:dbl)  [unwired: 2 in, 2 out]
            n1182 = property on="X Scan Velocity SP mm/sec" class="DigNum (strict)"() -> ("Value"=w2126:dbl)  [unwired: 2 in, 2 out]
            n1183 = property on="Y Scan Length SP mm" class="DigNum (strict)"() -> ("Value"=w2097:dbl)  [unwired: 2 in, 2 out]
            n1184 = property on="Y Scan Velocity SP mm/sec" class="DigNum (strict)"() -> ("Value"=w2091:dbl)  [unwired: 2 in, 2 out]
            n1185 = property on="R Scan Length SP deg" class="DigNum (strict)"() -> ("Value"=w2115:dbl)  [unwired: 2 in, 2 out]
            n1186 = property on="R deg/rev" class="DigNum (strict)"() -> ("Value"=w2102:dbl)  [unwired: 2 in, 2 out]
            n1187 = property on="Z Scan Velocity SP steps/sec" class="DigNum (strict)"() -> ("Maximum"=w2139:dbl)  [unwired: 2 in, 2 out]
            n1188 = property on="X Scan Velocity SP steps/sec" class="DigNum (strict)"() -> ("Maximum"=w2122:dbl)  [unwired: 2 in, 2 out]
            n1189 = property on="Y Scan Velocity SP steps/sec" class="DigNum (strict)"() -> ("Maximum"=w2087:dbl)  [unwired: 2 in, 2 out]
            n1190 = property on="R Scan Velocity SP steps/sec" class="DigNum (strict)"() -> ("Minimum"=w2104:dbl)  [unwired: 2 in, 2 out]
            n1191 = property on="Z Scan Velocity SP steps/sec" class="DigNum (strict)"() -> ("Minimum"=w2138:dbl)  [unwired: 2 in, 2 out]
            n1192 = property on="X Scan Velocity SP steps/sec" class="DigNum (strict)"() -> ("Minimum"=w2121:dbl)  [unwired: 2 in, 2 out]
            n1193 = property on="Y Scan Velocity SP steps/sec" class="DigNum (strict)"() -> ("Minimum"=w2086:dbl)  [unwired: 2 in, 2 out]
            n1194 = property on="R Scan Velocity SP deg/sec" class="DigNum (strict)"() -> ("Value"=w2109:dbl)  [unwired: 2 in, 2 out]
            n1195 = Divide(x=w2149, y=w2136) -> (x/y=w2152:dbl)
            n1196 = Divide(x=w2143, y=w2136) -> (x/y=w2144:dbl)
            n1197 = Divide(x=w2132, y=w2119) -> (x/y=w2135:dbl)
            n1198 = Divide(x=w2126, y=w2119) -> (x/y=w2127:dbl)
            n1199 = Divide(x=w2097, y=w2084) -> (x/y=w2100:dbl)
            n1200 = Divide(x=w2091, y=w2084) -> (x/y=w2092:dbl)
            n1201 = Divide(x=w2115, y=w2102) -> (x/y=w2118:dbl)
            n1202 = Multiply(x=w2152, y=w2137) -> (x*y=w2148:dbl)
            n1203 = Multiply(x=w2144, y=w2137) -> (x*y=w2141:dbl)
            n1204 = Multiply(x=w2135, y=w2120) -> (x*y=w2131:dbl)
            n1205 = Multiply(x=w2127, y=w2120) -> (x*y=w2124:dbl)
            n1206 = Multiply(x=w2100, y=w2085) -> (x*y=w2096:dbl)
            n1207 = Multiply(x=w2092, y=w2085) -> (x*y=w2089:dbl)
            n1208 = Multiply(x=w2118, y=w2103) -> (x*y=w2114:dbl)
            n1209 = Divide(x=w2109, y=w2102) -> (x/y=w2110:dbl)
            n1210 = property on="Z Step SP" class="DigNum (strict)"() -> ("Maximum"=w2145:dbl)  [unwired: 2 in, 2 out]
            n1211 = property on="X Step SP" class="DigNum (strict)"() -> ("Maximum"=w2128:dbl)  [unwired: 2 in, 2 out]
            n1212 = property on="Y Step SP" class="DigNum (strict)"() -> ("Maximum"=w2093:dbl)  [unwired: 2 in, 2 out]
            n1213 = property on="R Step SP" class="DigNum (strict)"() -> ("Maximum"=w2111:dbl)  [unwired: 2 in, 2 out]
            n1214 = property on="Z Step SP" class="DigNum (strict)"() -> ("Minimum"=w2146:dbl)  [unwired: 2 in, 2 out]
            n1215 = property on="X Step SP" class="DigNum (strict)"() -> ("Minimum"=w2129:dbl)  [unwired: 2 in, 2 out]
            n1216 = property on="Y Step SP" class="DigNum (strict)"() -> ("Minimum"=w2094:dbl)  [unwired: 2 in, 2 out]
            n1217 = property on="R Step SP" class="DigNum (strict)"() -> ("Minimum"=w2112:dbl)  [unwired: 2 in, 2 out]
            n1218 = Multiply(x=w2110, y=w2103) -> (x*y=w2107:dbl)
            n1219 = In Range and Coerce(upper limit=w2139, x=w2141, lower limit=w2138) -> (coerced(x)=w2140:dbl)  [unwired: 1 out]
            n1220 = In Range and Coerce(upper limit=w2122, x=w2124, lower limit=w2121) -> (coerced(x)=w2123:dbl)  [unwired: 1 out]
            n1221 = In Range and Coerce(upper limit=w2087, x=w2089, lower limit=w2086) -> (coerced(x)=w2088:dbl)  [unwired: 1 out]
            n1222 = To Long Integer(number=w2140) -> (32bit integer=w2142:i32)
            n1223 = To Long Integer(number=w2123) -> (32bit integer=w2125:i32)
            n1224 = To Long Integer(number=w2088) -> (32bit integer=w2090:i32)
            n1225 = Absolute Value(x=w2107) -> (abs(x)=w2101:dbl)
            n1226 = In Range and Coerce(upper limit=w2145, x=w2148, lower limit=w2146) -> (coerced(x)=w2147:dbl)  [unwired: 1 out]
            n1227 = In Range and Coerce(upper limit=w2128, x=w2131, lower limit=w2129) -> (coerced(x)=w2130:dbl)  [unwired: 1 out]
            n1228 = In Range and Coerce(upper limit=w2093, x=w2096, lower limit=w2094) -> (coerced(x)=w2095:dbl)  [unwired: 1 out]
            n1229 = In Range and Coerce(upper limit=w2111, x=w2114, lower limit=w2112) -> (coerced(x)=w2113:dbl)  [unwired: 1 out]
            n1230 = To Long Integer(number=w2147) -> (32bit integer=w2150:i32)
            n1231 = To Long Integer(number=w2130) -> (32bit integer=w2133:i32)
            n1232 = To Long Integer(number=w2095) -> (32bit integer=w2098:i32)
            n1233 = To Long Integer(number=w2113) -> (32bit integer=w2116:i32)
            n1234 = property on="Z Scan Velocity SP steps/sec" class="DigNum (strict)"("Val(Sgnl)"=w2142) -> ()  [unwired: 2 in, 2 out]
            n1235 = property on="X Scan Velocity SP steps/sec" class="DigNum (strict)"("Val(Sgnl)"=w2125) -> ()  [unwired: 2 in, 2 out]
            n1236 = property on="Y Scan Velocity SP steps/sec" class="DigNum (strict)"("Val(Sgnl)"=w2090) -> ()  [unwired: 2 in, 2 out]
            n1237 = In Range and Coerce(upper limit=w2105, x=w2101, lower limit=w2104) -> (coerced(x)=w2106:dbl)  [unwired: 1 out]
            n1238 = To Long Integer(number=w2106) -> (32bit integer=w2108:i32)
            n1239 = property on="Z Scan Length SP steps" class="DigNum (strict)"("Val(Sgnl)"=w2150) -> ()  [unwired: 2 in, 2 out]
            n1240 = property on="X Scan Length SP steps" class="DigNum (strict)"("Val(Sgnl)"=w2133) -> ()  [unwired: 2 in, 2 out]
            n1241 = property on="Y Scan Length SP steps" class="DigNum (strict)"("Val(Sgnl)"=w2098) -> ()  [unwired: 2 in, 2 out]
            n1242 = property on="R Scan Length SP steps" class="DigNum (strict)"("Val(Sgnl)"=w2116) -> ()  [unwired: 2 in, 2 out]
            n1243 = property on="R Scan Velocity SP steps/sec" class="DigNum (strict)"("Val(Sgnl)"=w2108) -> ()  [unwired: 2 in, 2 out]
          }
          frame #1 {
            n1244 = case shown="True" "Z as dominating length" {
              frame #0 {
              }
              frame #1 {
                n1245 = property on="Y Scan Length SP steps" class="DigNum (strict)"() -> ("Value"=w2162:i32)  [unwired: 2 in, 2 out]
                n1246 = property on="Z Scan Length SP steps" class="DigNum (strict)"() -> ("Value"=w2161:i32)  [unwired: 2 in, 2 out]
                n1247 = property on="X Scan Length SP steps" class="DigNum (strict)"() -> ("Value"=w2170:i32)  [unwired: 2 in, 2 out]
                n1248 = property on="Z Scan Length SP steps" class="DigNum (strict)"() -> ("Value"=w2169:i32)  [unwired: 2 in, 2 out]
                n1249 = property on="Y Scan Velocity SP steps/sec" class="DigNum (strict)"() -> ("Value"=w2158:i32)  [unwired: 2 in, 2 out]
                n1250 = property on="X Scan Velocity SP steps/sec" class="DigNum (strict)"() -> ("Value"=w2168:i32)  [unwired: 2 in, 2 out]
                n1251 = To Double Precision Float(number=w2162) -> (double precision float=w2160:dbl)
                n1252 = To Double Precision Float(number=w2161) -> (double precision float=w2159:dbl)
                n1253 = To Double Precision Float(number=w2170) -> (double precision float=w2164:dbl)
                n1254 = To Double Precision Float(number=w2169) -> (double precision float=w2165:dbl)
                n1255 = Divide(x=w2160, y=w2159) -> (x/y=w2154:dbl)
                n1256 = Divide(x=w2164, y=w2165) -> (x/y=w2171:dbl)
                n1257 = To Double Precision Float(number=w2158) -> (double precision float=w2157:dbl)
                n1258 = To Double Precision Float(number=w2168) -> (double precision float=w2166:dbl)
                n1259 = Multiply(x=w2154, y=w2157) -> (x*y=w2156:dbl)
                n1260 = Multiply(x=w2171, y=w2166) -> (x*y=w2167:dbl)
                n1261 = To Long Integer(number=w2156) -> (32bit integer=w2155:i32)
                n1262 = To Long Integer(number=w2167) -> (32bit integer=w2163:i32)
                n1263 = property on="Y Scan Velocity SP steps/sec" class="DigNum (strict)"("Val(Sgnl)"=w2155) -> ()  [unwired: 2 in, 2 out]
                n1264 = property on="X Scan Velocity SP steps/sec" class="DigNum (strict)"("Val(Sgnl)"=w2163) -> ()  [unwired: 2 in, 2 out]
              }
            }
          }
          frame #2 {
            w2172 = T9."Enabled" ("Disabled")
            n1265 = property on="Send scan parameter" class="Bool"("DisabledEnum"=w2172) -> ()  [unwired: 2 in, 2 out]
            n1266 = property on="LOOP" class="Bool (strict)"("DisabledEnum"=w2172) -> ()  [unwired: 2 in, 2 out]
          }
        }
        n1267 = local write "STATUS"("SCANNING PARAMETERS SET" ("STATUS")) -> ()
      }
      event #12 {
        n1268 = event-data() -> ()  [unwired: 1 in, 7 out]
        n1269 = local write "STATUS"("READY TO SCAN" ("STATUS")) -> ()
        n1270 = flat-sequence {
          tunnel: [w2226] -> w2186
          tunnel: [w2225] -> w2185
          tunnel: w2176 -> [w2224]
          tunnel: w2175 -> [w2223]
          tunnel: w2186 -> [w2232]
          tunnel: [w2232] -> w2184
          tunnel: w2185 -> [w2231]
          tunnel: [w2231] -> w2183
          tunnel: w2184 -> [w2238]
          tunnel: [w2237] -> w2182
          tunnel: w2183 -> [w2236]
          tunnel: [w2235] -> w2181
          tunnel: w2182 -> [w2244]
          tunnel: w2181 -> [w2243]
          tunnel: [w2244] -> w2180
          tunnel: [w2243] -> w2179
          tunnel: w2180 -> [w2249]
          tunnel: w2179 -> [w2248]
          tunnel: [w2249] -> w2178
          tunnel: [w2248] -> w2177
          tunnel: [w2251] -> _
          tunnel: [w2252] -> _
          tunnel: w2178 -> [w2252]
          tunnel: w2177 -> [w2251]
          frame #0 {
            n1271 = property on="R Scan Velocity SP steps/sec" class="DigNum (strict)"() -> ("Value"=w2228:i32)  [unwired: 2 in, 2 out]
            n1272 = Number To Decimal String(number=w2228) -> (decimal integer string=w2229:string)  [unwired: 1 in]
            n1273 = call "mDrive Send Command.vi"("error in (no error)"=w2224, "Extra"=w2229, "Command"=T10."Max Velocity", "VISA resource name"=w2223) -> ("error out"=w2225:errorcluster, "VISA resource name out"=w2226:refnum<visa-resource-name>)  [unwired: 3 in, 1 out]
          }
          frame #1 {
            n1274 = Wait (ms)(milliseconds to wait=u32 100) -> ()  [unwired: 1 out]
          }
          frame #2 {
            # "VELOCITY"
            n1275 = call "mdrive send command.vi"("error in (no error)"=w2236, "Extra"="VM", "Command"=T10."Print Parameter", "VISA resource name"=w2238) -> ("error out"=w2235:errorcluster, "read buffer"=w2240:string, "VISA resource name out"=w2237:refnum<visa-resource-name>)  [unwired: 3 in]
            n1276 = Decimal String To Number(string=w2240, offset=0) -> (number=w2239:i32)  [unwired: 1 in, 1 out]
            n1277 = property on="R velocity PV step/sec" class="DigNum (strict)"("Val(Sgnl)"=w2239) -> ()  [unwired: 2 in, 2 out]
          }
          frame #3 {
            n1278 = Wait (ms)(milliseconds to wait=u32 100) -> ()  [unwired: 1 out]
          }
          frame #4 {
            n1279 = property on="Scan Go" class="Bool (strict)"("DisabledEnum"=T9."Enabled" ("Disabled")) -> ()  [unwired: 2 in, 2 out]
            n1280 = property on="R Scan Velocity SP steps/sec" class="DigNum (strict)"("DisabledEnum"=T9."Disabled and Grayed Out" ("Disabled")) -> ()  [unwired: 2 in, 2 out]
            n1281 = property on="R Scan Length SP steps" class="DigNum (strict)"("DisabledEnum"=T9."Disabled and Grayed Out" ("Disabled")) -> ()  [unwired: 2 in, 2 out]
          }
          frame #5 {
            n1282 = property on="R Scan" class="Bool (strict)"("Val(Sgnl)"=TRUE ("Slew Ready 2")) -> ()  [unwired: 2 in, 2 out]
          }
        }
        n1283 = flat-sequence {
          tunnel: [w2286] -> w2210
          tunnel: [w2285] -> w2209
          tunnel: w2200 -> [w2284]
          tunnel: w2199 -> [w2283]
          tunnel: w2210 -> [w2292]
          tunnel: [w2292] -> w2208
          tunnel: w2209 -> [w2291]
          tunnel: [w2291] -> w2207
          tunnel: w2208 -> [w2296]
          tunnel: [w2295] -> w2206
          tunnel: w2207 -> [w2294]
          tunnel: [w2293] -> w2205
          tunnel: w2206 -> [w2304]
          tunnel: [w2304] -> w2204
          tunnel: w2205 -> [w2303]
          tunnel: [w2303] -> w2203
          tunnel: w2204 -> [w2309]
          tunnel: w2203 -> [w2308]
          tunnel: [w2309] -> w2202
          tunnel: [w2308] -> w2201
          tunnel: [w2311] -> _
          tunnel: [w2312] -> _
          tunnel: w2202 -> [w2312]
          tunnel: w2201 -> [w2311]
          frame #0 {
            n1284 = property on="Y Scan Velocity SP steps/sec" class="DigNum (strict)"() -> ("Value"=w2288:i32)  [unwired: 2 in, 2 out]
            n1285 = Number To Decimal String(number=w2288) -> (decimal integer string=w2289:string)  [unwired: 1 in]
            n1286 = call "mdrive send command.vi"("error in (no error)"=w2284, "Extra"=w2289, "Command"=T10."Max Velocity", "VISA resource name"=w2283) -> ("error out"=w2285:errorcluster, "VISA resource name out"=w2286:refnum<visa-resource-name>)  [unwired: 3 in, 1 out]
          }
          frame #1 {
            n1287 = Wait (ms)(milliseconds to wait=u32 100) -> ()  [unwired: 1 out]
          }
          frame #2 {
            # "VELOCITY"
            n1288 = call "mdrive send command.vi"("error in (no error)"=w2294, "Extra"="VM", "Command"=T10."Print Parameter", "VISA resource name"=w2296) -> ("error out"=w2293:errorcluster, "read buffer"=w2300:string, "VISA resource name out"=w2295:refnum<visa-resource-name>)  [unwired: 3 in]
            n1289 = Decimal String To Number(string=w2300, offset=0) -> (number=w2298:i32)  [unwired: 1 in, 1 out]
            n1290 = property on="Y velocity PV step/sec" class="DigNum (strict)"("Val(Sgnl)"=w2298) -> ()  [unwired: 2 in, 2 out]
          }
          frame #3 {
            n1291 = Wait (ms)(milliseconds to wait=u32 100) -> ()  [unwired: 1 out]
          }
          frame #4 {
            n1292 = property on="Scan Go" class="Bool (strict)"("DisabledEnum"=T9."Enabled" ("Disabled")) -> ()  [unwired: 2 in, 2 out]
            n1293 = property on="Y Scan Velocity SP steps/sec" class="DigNum (strict)"("DisabledEnum"=T9."Disabled and Grayed Out" ("Disabled")) -> ()  [unwired: 2 in, 2 out]
            n1294 = property on="Y Scan Length SP steps" class="DigNum (strict)"("DisabledEnum"=T9."Disabled and Grayed Out" ("Disabled")) -> ()  [unwired: 2 in, 2 out]
          }
          frame #5 {
            n1295 = property on="Y Scan" class="Bool (strict)"("Val(Sgnl)"=TRUE ("Slew Ready 2")) -> ()  [unwired: 2 in, 2 out]
          }
        }
        n1296 = flat-sequence {
          tunnel: [w2314] -> w2214
          tunnel: [w2313] -> w2212
          tunnel: w2220 -> [w2316]
          tunnel: w2219 -> [w2315]
          tunnel: w2214 -> [w2322]
          tunnel: [w2322] -> w2213
          tunnel: w2212 -> [w2321]
          tunnel: [w2321] -> w2211
          tunnel: w2213 -> [w2326]
          tunnel: [w2325] -> w2216
          tunnel: w2211 -> [w2324]
          tunnel: [w2323] -> w2215
          tunnel: w2216 -> [w2334]
          tunnel: [w2334] -> w2218
          tunnel: w2215 -> [w2333]
          tunnel: [w2333] -> w2217
          tunnel: w2218 -> [w2339]
          tunnel: w2217 -> [w2338]
          tunnel: [w2339] -> w2222
          tunnel: [w2338] -> w2221
          tunnel: [w2341] -> _
          tunnel: [w2342] -> _
          tunnel: w2222 -> [w2342]
          tunnel: w2221 -> [w2341]
          frame #0 {
            n1297 = property on="X Scan Velocity SP steps/sec" class="DigNum (strict)"() -> ("Value"=w2318:i32)  [unwired: 2 in, 2 out]
            n1298 = Number To Decimal String(number=w2318) -> (decimal integer string=w2319:string)  [unwired: 1 in]
            n1299 = call "mdrive send command.vi"("error in (no error)"=w2316, "Extra"=w2319, "Command"=T10."Max Velocity", "VISA resource name"=w2315) -> ("error out"=w2313:errorcluster, "VISA resource name out"=w2314:refnum<visa-resource-name>)  [unwired: 3 in, 1 out]
          }
          frame #1 {
            n1300 = Wait (ms)(milliseconds to wait=u32 100) -> ()  [unwired: 1 out]
          }
          frame #2 {
            # "VELOCITY"
            n1301 = call "mdrive send command.vi"("error in (no error)"=w2324, "Extra"="VM", "Command"=T10."Print Parameter", "VISA resource name"=w2326) -> ("error out"=w2323:errorcluster, "read buffer"=w2329:string, "VISA resource name out"=w2325:refnum<visa-resource-name>)  [unwired: 3 in]
            n1302 = Decimal String To Number(string=w2329, offset=0) -> (number=w2327:i32)  [unwired: 1 in, 1 out]
            n1303 = property on="X velocity PV step/sec" class="DigNum (strict)"("Val(Sgnl)"=w2327) -> ()  [unwired: 2 in, 2 out]
          }
          frame #3 {
            n1304 = Wait (ms)(milliseconds to wait=u32 100) -> ()  [unwired: 1 out]
          }
          frame #4 {
            n1305 = property on="Scan Go" class="Bool (strict)"("DisabledEnum"=T9."Enabled" ("Disabled")) -> ()  [unwired: 2 in, 2 out]
            n1306 = property on="X Scan Velocity SP steps/sec" class="DigNum (strict)"("DisabledEnum"=T9."Disabled and Grayed Out" ("Disabled")) -> ()  [unwired: 2 in, 2 out]
            n1307 = property on="X Scan Length SP steps" class="DigNum (strict)"("DisabledEnum"=T9."Disabled and Grayed Out" ("Disabled")) -> ()  [unwired: 2 in, 2 out]
          }
          frame #5 {
            n1308 = property on="X Scan" class="Bool (strict)"("Val(Sgnl)"=TRUE ("Slew Ready 2")) -> ()  [unwired: 2 in, 2 out]
          }
        }
        n1309 = flat-sequence {
          tunnel: [w2256] -> w2198
          tunnel: [w2255] -> w2197
          tunnel: w2188 -> [w2254]
          tunnel: w2187 -> [w2253]
          tunnel: w2198 -> [w2262]
          tunnel: [w2262] -> w2196
          tunnel: w2197 -> [w2261]
          tunnel: [w2261] -> w2195
          tunnel: w2196 -> [w2268]
          tunnel: [w2267] -> w2194
          tunnel: w2195 -> [w2266]
          tunnel: [w2265] -> w2193
          tunnel: w2194 -> [w2274]
          tunnel: [w2274] -> w2192
          tunnel: w2193 -> [w2273]
          tunnel: [w2273] -> w2191
          tunnel: w2192 -> [w2279]
          tunnel: w2191 -> [w2278]
          tunnel: [w2279] -> w2190
          tunnel: [w2278] -> w2189
          tunnel: [w2281] -> _
          tunnel: [w2282] -> _
          tunnel: w2190 -> [w2282]
          tunnel: w2189 -> [w2281]
          frame #0 {
            n1310 = property on="Z Scan Velocity SP steps/sec" class="DigNum (strict)"() -> ("Value"=w2258:i32)  [unwired: 2 in, 2 out]
            n1311 = Number To Decimal String(number=w2258) -> (decimal integer string=w2259:string)  [unwired: 1 in]
            n1312 = call "mdrive send command.vi"("error in (no error)"=w2254, "Extra"=w2259, "Command"=T10."Max Velocity", "VISA resource name"=w2253) -> ("error out"=w2255:errorcluster, "VISA resource name out"=w2256:refnum<visa-resource-name>)  [unwired: 3 in, 1 out]
          }
          frame #1 {
            n1313 = Wait (ms)(milliseconds to wait=u32 100) -> ()  [unwired: 1 out]
          }
          frame #2 {
            # "VELOCITY"
            n1314 = call "mdrive send command.vi"("error in (no error)"=w2266, "Extra"="VM", "Command"=T10."Print Parameter", "VISA resource name"=w2268) -> ("error out"=w2265:errorcluster, "read buffer"=w2269:string, "VISA resource name out"=w2267:refnum<visa-resource-name>)  [unwired: 3 in]
            n1315 = Decimal String To Number(string=w2269, offset=0) -> (number=w2270:i32)  [unwired: 1 in, 1 out]
            n1316 = property on="Z  velocity PV step/sec" class="DigNum (strict)"("Val(Sgnl)"=w2270) -> ()  [unwired: 2 in, 2 out]
          }
          frame #3 {
            n1317 = Wait (ms)(milliseconds to wait=u32 100) -> ()  [unwired: 1 out]
          }
          frame #4 {
            n1318 = property on="Scan Go" class="Bool (strict)"("DisabledEnum"=T9."Enabled" ("Disabled")) -> ()  [unwired: 2 in, 2 out]
            n1319 = property on="Z Scan Velocity SP steps/sec" class="DigNum (strict)"("DisabledEnum"=T9."Disabled and Grayed Out" ("Disabled")) -> ()  [unwired: 2 in, 2 out]
            n1320 = property on="Z Scan Length SP steps" class="DigNum (strict)"("DisabledEnum"=T9."Disabled and Grayed Out" ("Disabled")) -> ()  [unwired: 2 in, 2 out]
          }
          frame #5 {
            n1321 = property on="Z Scan" class="Bool (strict)"("Val(Sgnl)"=TRUE ("Slew Ready 2")) -> ()  [unwired: 2 in, 2 out]
          }
        }
        n1322 = property on="GO" class="Bool"("DisabledEnum"=T9."Disabled and Grayed Out" ("Disabled")) -> ()  [unwired: 2 in, 2 out]
      }
      event #13 {
        n1323 = event-data() -> ()  [unwired: 1 in, 7 out]
        n1324 = flat-sequence {
          tunnel: [w2367] -> w2355
          tunnel: [w2366] -> w2354
          tunnel: w2348 -> [w2364]
          tunnel: w2346 -> [w2363]
          tunnel: [w2371] -> _
          tunnel: [w2372] -> _
          tunnel: w2355 -> [w2372]
          tunnel: w2354 -> [w2371]
          frame #0 {
            n1325 = call "mDrive Send Command.vi"("error in (no error)"=w2363, "Command"=T10."Stop", "VISA resource name"=w2364) -> ("error out"=w2366:errorcluster, "VISA resource name out"=w2367:refnum<visa-resource-name>)  [unwired: 4 in, 1 out]
          }
          frame #1 {
            n1326 = property on="R Scan" class="Bool (strict)"("Value"=FALSE ("Slew Ready")) -> ()  [unwired: 2 in, 2 out]
            n1327 = property on="R Scan Length SP steps" class="DigNum (strict)"("DisabledEnum"=T9."Enabled" ("Disabled")) -> ()  [unwired: 2 in, 2 out]
            n1328 = property on="R Scan Velocity SP steps/sec" class="DigNum (strict)"("DisabledEnum"=T9."Enabled" ("Disabled")) -> ()  [unwired: 2 in, 2 out]
          }
        }
        n1329 = flat-sequence {
          tunnel: [w2387] -> w2359
          tunnel: [w2386] -> w2358
          tunnel: w2353 -> [w2384]
          tunnel: w2351 -> [w2383]
          tunnel: [w2391] -> _
          tunnel: [w2392] -> _
          tunnel: w2359 -> [w2392]
          tunnel: w2358 -> [w2391]
          frame #0 {
            n1330 = call "mDrive Send Command.vi"("error in (no error)"=w2383, "Command"=T10."Stop", "VISA resource name"=w2384) -> ("error out"=w2386:errorcluster, "VISA resource name out"=w2387:refnum<visa-resource-name>)  [unwired: 4 in, 1 out]
          }
          frame #1 {
            n1331 = property on="X Scan" class="Bool (strict)"("Value"=FALSE ("Slew Ready")) -> ()  [unwired: 2 in, 2 out]
            n1332 = property on="X Scan Velocity SP steps/sec" class="DigNum (strict)"("DisabledEnum"=T9."Enabled" ("Disabled")) -> ()  [unwired: 2 in, 2 out]
            n1333 = property on="X Scan Length SP steps" class="DigNum (strict)"("DisabledEnum"=T9."Enabled" ("Disabled")) -> ()  [unwired: 2 in, 2 out]
          }
        }
        n1334 = flat-sequence {
          tunnel: [w2377] -> w2357
          tunnel: [w2376] -> w2356
          tunnel: w2352 -> [w2374]
          tunnel: w2350 -> [w2373]
          tunnel: [w2381] -> _
          tunnel: [w2382] -> _
          tunnel: w2357 -> [w2382]
          tunnel: w2356 -> [w2381]
          frame #0 {
            n1335 = call "mDrive Send Command.vi"("error in (no error)"=w2373, "Command"=T10."Stop", "VISA resource name"=w2374) -> ("error out"=w2376:errorcluster, "VISA resource name out"=w2377:refnum<visa-resource-name>)  [unwired: 4 in, 1 out]
          }
          frame #1 {
            n1336 = property on="Z Scan" class="Bool (strict)"("Value"=FALSE ("Slew Ready")) -> ()  [unwired: 2 in, 2 out]
            n1337 = property on="Z Scan Velocity SP steps/sec" class="DigNum (strict)"("DisabledEnum"=T9."Enabled" ("Disabled")) -> ()  [unwired: 2 in, 2 out]
            n1338 = property on="Z Scan Length SP steps" class="DigNum (strict)"("DisabledEnum"=T9."Enabled" ("Disabled")) -> ()  [unwired: 2 in, 2 out]
          }
        }
        n1339 = flat-sequence {
          tunnel: [w2397] -> w2361
          tunnel: [w2396] -> w2360
          tunnel: w2349 -> [w2394]
          tunnel: w2347 -> [w2393]
          tunnel: [w2401] -> _
          tunnel: [w2402] -> _
          tunnel: w2361 -> [w2402]
          tunnel: w2360 -> [w2401]
          frame #0 {
            n1340 = call "mDrive Send Command.vi"("error in (no error)"=w2393, "Command"=T10."Stop", "VISA resource name"=w2394) -> ("error out"=w2396:errorcluster, "VISA resource name out"=w2397:refnum<visa-resource-name>)  [unwired: 4 in, 1 out]
          }
          frame #1 {
            n1341 = property on="Y Scan" class="Bool (strict)"("Value"=FALSE ("Slew Ready")) -> ()  [unwired: 2 in, 2 out]
            n1342 = property on="Y Scan Velocity SP steps/sec" class="DigNum (strict)"("DisabledEnum"=T9."Enabled" ("Disabled")) -> ()  [unwired: 2 in, 2 out]
            n1343 = property on="Y Scan Length SP steps" class="DigNum (strict)"("DisabledEnum"=T9."Enabled" ("Disabled")) -> ()  [unwired: 2 in, 2 out]
          }
        }
        n1344 = property on="GO" class="Bool"("DisabledEnum"=T9."Enabled" ("Disabled")) -> ()  [unwired: 2 in, 2 out]
        n1345 = property on="Set Scan \nParameters" class="Bool"("DisabledEnum"=T9."Enabled" ("Disabled")) -> ()  [unwired: 2 in, 2 out]
        n1346 = property on="Send scan parameter" class="Bool"("DisabledEnum"=T9."Enabled" ("Disabled")) -> ()  [unwired: 2 in, 2 out]
        n1347 = property on="Scan Go" class="Bool (strict)"("DisabledEnum"=T9."Disabled and Grayed Out" ("Disabled")) -> ()  [unwired: 2 in, 2 out]
      }
      event #14 {
        w2403 = T9."Disabled and Grayed Out" ("Disabled")
        n1348 = event-data() -> ()  [unwired: 1 in, 7 out]
        n1349 = flat-sequence {
          tunnel: [w2476] -> w2460
          tunnel: [w2474] -> w2453
          tunnel: [w2475] -> w2450
          tunnel: [w2469] -> w2449
          tunnel: [w2473] -> w2448
          tunnel: [w2472] -> w2447
          tunnel: [w2471] -> w2446
          tunnel: [w2470] -> w2445
          tunnel: w2420 -> [w2468]
          tunnel: w2419 -> [w2467]
          tunnel: w2418 -> [w2466]
          tunnel: w2417 -> [w2465]
          tunnel: w2416 -> [w2464]
          tunnel: w2415 -> [w2463]
          tunnel: w2414 -> [w2462]
          tunnel: w2413 -> [w2461]
          tunnel: [w2468] -> w2412
          tunnel: [w2467] -> w2411
          tunnel: [w2466] -> w2410
          tunnel: [w2465] -> w2409
          tunnel: [w2464] -> w2408
          tunnel: [w2463] -> w2407
          tunnel: [w2462] -> w2406
          tunnel: [w2461] -> w2405
          tunnel: [w2528] -> w2457
          tunnel: [w2527] -> w2455
          tunnel: w2460 -> [w2526]
          tunnel: w2453 -> [w2525]
          tunnel: [w2525] -> w2451
          tunnel: w2450 -> [w2524]
          tunnel: w2449 -> [w2513]
          tunnel: w2448 -> [w2523]
          tunnel: w2447 -> [w2519]
          tunnel: w2446 -> [w2516]
          tunnel: w2445 -> [w2522]
          tunnel: [w2521] -> w2443
          tunnel: [w2520] -> w2441
          tunnel: [w2519] -> w2438
          tunnel: [w2518] -> w2436
          tunnel: [w2517] -> w2434
          tunnel: [w2516] -> w2432
          tunnel: [w2515] -> w2430
          tunnel: [w2514] -> w2428
          tunnel: [w2513] -> w2427
          tunnel: w2412 -> [w2512]
          tunnel: w2411 -> [w2511]
          tunnel: w2410 -> [w2510]
          tunnel: w2409 -> [w2509]
          tunnel: w2408 -> [w2508]
          tunnel: w2407 -> [w2507]
          tunnel: w2406 -> [w2506]
          tunnel: w2405 -> [w2505]
          tunnel: w2457 -> [w2569]
          tunnel: [w2569] -> w2456
          tunnel: w2455 -> [w2568]
          tunnel: [w2568] -> w2454
          tunnel: [w2567] -> w2452
          tunnel: w2451 -> [w2567]
          tunnel: [w2566] -> w2444
          tunnel: w2443 -> [w2566]
          tunnel: [w2565] -> w2442
          tunnel: w2441 -> [w2565]
          tunnel: [w2564] -> w2440
          tunnel: [w2563] -> w2439
          tunnel: w2438 -> [w2563]
          tunnel: [w2562] -> w2437
          tunnel: w2436 -> [w2562]
          tunnel: [w2561] -> w2435
          tunnel: w2434 -> [w2561]
          tunnel: [w2560] -> w2433
          tunnel: w2432 -> [w2560]
          tunnel: [w2559] -> w2431
          tunnel: w2430 -> [w2559]
          tunnel: [w2558] -> w2429
          tunnel: w2428 -> [w2558]
          tunnel: w2427 -> [w2564]
          tunnel: w2456 -> [w2589]
          tunnel: [w2587] -> w2459
          tunnel: w2454 -> [w2588]
          tunnel: [w2586] -> w2458
          tunnel: w2452 -> [w2585]
          tunnel: w2444 -> [w2584]
          tunnel: w2442 -> [w2583]
          tunnel: w2440 -> [w2582]
          tunnel: w2439 -> [w2581]
          tunnel: w2437 -> [w2580]
          tunnel: w2435 -> [w2579]
          tunnel: w2433 -> [w2578]
          tunnel: w2431 -> [w2577]
          tunnel: w2429 -> [w2576]
          tunnel: [w2575] -> w2426
          tunnel: [w2574] -> w2425
          tunnel: [w2573] -> w2424
          tunnel: [w2572] -> w2423
          tunnel: [w2571] -> w2422
          tunnel: [w2570] -> w2421
          tunnel: w2459 -> [w2646]
          tunnel: w2458 -> [w2645]
          tunnel: [w2646] -> _
          tunnel: [w2645] -> _
          tunnel: [w2640] -> _
          tunnel: w2426 -> [w2640]
          tunnel: [w2639] -> _
          tunnel: w2425 -> [w2639]
          tunnel: w2424 -> [w2629]
          tunnel: [w2629] -> _
          tunnel: [w2628] -> _
          tunnel: w2423 -> [w2628]
          tunnel: [w2627] -> _
          tunnel: w2422 -> [w2627]
          tunnel: [w2626] -> _
          tunnel: w2421 -> [w2626]
          frame #0 {
            n1350 = property on="X Scan" class="Bool (strict)"() -> ("Value"=w2469:bool)  [unwired: 2 in, 2 out]
            n1351 = property on="Z Scan" class="Bool (strict)"() -> ("Value"=w2471:bool)  [unwired: 2 in, 2 out]
            n1352 = property on="Y Scan" class="Bool (strict)"() -> ("Value"=w2474:bool)  [unwired: 2 in, 2 out]
            n1353 = property on="R Scan" class="Bool (strict)"() -> ("Value"=w2472:bool)  [unwired: 2 in, 2 out]
            n1354 = case shown="False" w2469 {
              tunnel: ["" w2492] -> w2475
              frame #0 {
              }
              frame #1 {
                n1355 = property on="X Scan Length SP steps" class="DigNum (strict)"() -> ("Value"=w2497:i32)  [unwired: 2 in, 2 out]
                n1356 = Number To Decimal String(number=w2497) -> (decimal integer string=w2494:string)  [unwired: 1 in]
                n1357 = call <vilib>:"Space Constant.vi"() -> ("String"=w2495:string)
                n1358 = Concatenate Strings("MR", w2495, w2494, "\r") -> (w2492:string)
              }
            }
            n1359 = case shown="False" w2471 {
              tunnel: ["" w2485] -> w2473
              frame #0 {
              }
              frame #1 {
                n1360 = property on="Z Scan Length SP steps" class="DigNum (strict)"() -> ("Value"=w2490:i32)  [unwired: 2 in, 2 out]
                n1361 = Number To Decimal String(number=w2490) -> (decimal integer string=w2487:string)  [unwired: 1 in]
                n1362 = call <vilib>:"Space Constant.vi"() -> ("String"=w2488:string)
                n1363 = Concatenate Strings("MR", w2488, w2487, "\r") -> (w2485:string)
              }
            }
            n1364 = case shown="False" w2474 {
              tunnel: ["" w2499] -> w2476
              frame #0 {
              }
              frame #1 {
                n1365 = property on="Y Scan Length SP steps" class="DigNum (strict)"() -> ("Value"=w2504:i32)  [unwired: 2 in, 2 out]
                n1366 = Number To Decimal String(number=w2504) -> (decimal integer string=w2501:string)  [unwired: 1 in]
                n1367 = call <vilib>:"Space Constant.vi"() -> ("String"=w2502:string)
                n1368 = Concatenate Strings("MR", w2502, w2501, "\r") -> (w2499:string)
              }
            }
            n1369 = case shown="False" w2472 {
              tunnel: ["" w2478] -> w2470
              frame #0 {
              }
              frame #1 {
                n1370 = property on="R Scan Length SP steps" class="DigNum (strict)"() -> ("Value"=w2483:i32)  [unwired: 2 in, 2 out]
                n1371 = Number To Decimal String(number=w2483) -> (decimal integer string=w2480:string)  [unwired: 1 in]
                n1372 = call <vilib>:"Space Constant.vi"() -> ("String"=w2481:string)
                n1373 = Concatenate Strings("MR", w2481, w2480, "\r") -> (w2478:string)
              }
            }
          }
          frame #1 {
            n1374 = case shown="False" w2513 {
              tunnel: [w2544 w2549] -> w2521
              tunnel: [w2543 w2548] -> w2520
              tunnel: w2524 -> [_ w2547]
              tunnel: w2512 -> [w2544 w2546]
              tunnel: w2511 -> [w2543 w2545]
              frame #0 {
              }
              frame #1 {
                n1375 = VISA Write(VISA resource name=w2546, write buffer=w2547, error in (no error)=w2545) -> (VISA resource name out=w2549:refnum<visa-resource-name>, error out=w2548:errorcluster)  [unwired: 1 out]
              }
            }
            n1376 = case shown="True" w2516 {
              tunnel: [w2537 w2542] -> w2515
              tunnel: [w2536 w2541] -> w2514
              tunnel: w2523 -> [_ w2540]
              tunnel: w2510 -> [w2537 w2539]
              tunnel: w2509 -> [w2536 w2538]
              frame #0 {
              }
              frame #1 {
                n1377 = VISA Write(VISA resource name=w2539, write buffer=w2540, error in (no error)=w2538) -> (VISA resource name out=w2542:refnum<visa-resource-name>, error out=w2541:errorcluster)  [unwired: 1 out]
              }
            }
            n1378 = case shown="True" w2525 {
              tunnel: [w2551 w2556] -> w2528
              tunnel: [w2550 w2555] -> w2527
              tunnel: w2526 -> [_ w2554]
              tunnel: w2508 -> [w2551 w2553]
              tunnel: w2507 -> [w2550 w2552]
              frame #0 {
              }
              frame #1 {
                n1379 = VISA Write(VISA resource name=w2553, write buffer=w2554, error in (no error)=w2552) -> (VISA resource name out=w2556:refnum<visa-resource-name>, error out=w2555:errorcluster)  [unwired: 1 out]
              }
            }
            n1380 = case shown="True" w2519 {
              tunnel: [w2530 w2535] -> w2518
              tunnel: [w2529 w2534] -> w2517
              tunnel: w2522 -> [_ w2533]
              tunnel: w2506 -> [w2530 w2532]
              tunnel: w2505 -> [w2529 w2531]
              frame #0 {
              }
              frame #1 {
                n1381 = VISA Write(VISA resource name=w2532, write buffer=w2533, error in (no error)=w2531) -> (VISA resource name out=w2535:refnum<visa-resource-name>, error out=w2534:errorcluster)  [unwired: 1 out]
              }
            }
          }
          frame #2 {
            n1382 = Wait (ms)(milliseconds to wait=u32 100) -> ()  [unwired: 1 out]
          }
          frame #3 {
            n1383 = case shown="True" w2582 {
              tunnel: w2584 -> [w2609 w2613]
              tunnel: w2583 -> [w2608 w2612]
              tunnel: [w2609 w2611] -> w2571
              tunnel: [w2608 w2610] -> w2570
              frame #0 {
              }
              frame #1 {
                n1384 = property class="Instr"(reference=w2613, error in=w2612) -> (reference out=w2615:refnum<visa-resource-name>, error out=w2614:errorcluster, "Serial Settings:Number of Bytes at Serial Port"=w2616:u32)
                n1385 = VISA Read(VISA resource name=w2615, byte count=w2616, error in (no error)=w2614) -> (VISA resource name out=w2611:refnum<visa-resource-name>, error out=w2610:errorcluster)  [unwired: 2 out]
              }
            }
            n1386 = case shown="True" w2578 {
              tunnel: w2577 -> [w2591 w2595]
              tunnel: w2576 -> [w2590 w2594]
              tunnel: [w2591 w2593] -> w2575
              tunnel: [w2590 w2592] -> w2574
              frame #0 {
              }
              frame #1 {
                n1387 = property class="Instr"(reference=w2595, error in=w2594) -> (reference out=w2597:refnum<visa-resource-name>, error out=w2596:errorcluster, "Serial Settings:Number of Bytes at Serial Port"=w2598:u32)
                n1388 = VISA Read(VISA resource name=w2597, byte count=w2598, error in (no error)=w2596) -> (VISA resource name out=w2593:refnum<visa-resource-name>, error out=w2592:errorcluster)  [unwired: 2 out]
              }
            }
            n1389 = case shown="True" w2585 {
              tunnel: w2589 -> [w2618 w2622]
              tunnel: w2588 -> [w2617 w2621]
              tunnel: [w2618 w2620] -> w2587
              tunnel: [w2617 w2619] -> w2586
              frame #0 {
              }
              frame #1 {
                n1390 = property class="Instr"(reference=w2622, error in=w2621) -> (reference out=w2624:refnum<visa-resource-name>, error out=w2623:errorcluster, "Serial Settings:Number of Bytes at Serial Port"=w2625:u32)
                n1391 = VISA Read(VISA resource name=w2624, byte count=w2625, error in (no error)=w2623) -> (VISA resource name out=w2620:refnum<visa-resource-name>, error out=w2619:errorcluster)  [unwired: 2 out]
              }
            }
            n1392 = case shown="True" w2581 {
              tunnel: w2580 -> [w2600 w2604]
              tunnel: w2579 -> [w2599 w2603]
              tunnel: [w2600 w2602] -> w2573
              tunnel: [w2599 w2601] -> w2572
              frame #0 {
              }
              frame #1 {
                n1393 = property class="Instr"(reference=w2604, error in=w2603) -> (reference out=w2606:refnum<visa-resource-name>, error out=w2605:errorcluster, "Serial Settings:Number of Bytes at Serial Port"=w2607:u32)
                n1394 = VISA Read(VISA resource name=w2606, byte count=w2607, error in (no error)=w2605) -> (VISA resource name out=w2602:refnum<visa-resource-name>, error out=w2601:errorcluster)  [unwired: 2 out]
              }
            }
          }
          frame #4 {
            n1395 = property on="R Scan" class="Bool (strict)"("Val(Sgnl)"=FALSE ("Slew Ready 2")) -> ()  [unwired: 2 in, 2 out]
            n1396 = property on="Z Scan" class="Bool (strict)"("Val(Sgnl)"=FALSE ("Slew Ready 2")) -> ()  [unwired: 2 in, 2 out]
            n1397 = property on="Y Scan" class="Bool (strict)"("Val(Sgnl)"=FALSE ("Slew Ready 2")) -> ()  [unwired: 2 in, 2 out]
            n1398 = property on="X Scan" class="Bool (strict)"("Val(Sgnl)"=FALSE ("Slew Ready 2")) -> ()  [unwired: 2 in, 2 out]
            n1399 = property on="R Scan Length SP steps" class="DigNum (strict)"("DisabledEnum"=T9."Enabled" ("Disabled")) -> ()  [unwired: 2 in, 2 out]
            n1400 = property on="Z Scan Velocity SP steps/sec" class="DigNum (strict)"("DisabledEnum"=T9."Enabled" ("Disabled")) -> ()  [unwired: 2 in, 2 out]
            n1401 = property on="X Scan Length SP steps" class="DigNum (strict)"("DisabledEnum"=T9."Enabled" ("Disabled")) -> ()  [unwired: 2 in, 2 out]
            n1402 = property on="Y Scan Selocity SP steps/sec" class="DigNum (strict)"("DisabledEnum"=T9."Enabled" ("Disabled")) -> ()  [unwired: 2 in, 2 out]
            n1403 = property on="Z Scan Length SP steps" class="DigNum (strict)"("DisabledEnum"=T9."Enabled" ("Disabled")) -> ()  [unwired: 2 in, 2 out]
            n1404 = property on="X Scan Velocity SP steps/sec" class="DigNum (strict)"("DisabledEnum"=T9."Enabled" ("Disabled")) -> ()  [unwired: 2 in, 2 out]
            n1405 = property on="Y Scan Length SP steps" class="DigNum (strict)"("DisabledEnum"=T9."Enabled" ("Disabled")) -> ()  [unwired: 2 in, 2 out]
            n1406 = property on="R Scan Velocity SP steps/sec" class="DigNum (strict)"("DisabledEnum"=T9."Enabled" ("Disabled")) -> ()  [unwired: 2 in, 2 out]
            n1407 = property on="Scan Go" class="Bool (strict)"("DisabledEnum"=T9."Disabled and Grayed Out" ("Disabled")) -> ()  [unwired: 2 in, 2 out]
          }
        }
        n1408 = local write "STATUS"("SCANNING" ("STATUS")) -> ()
        n1409 = property on="GO" class="Bool"("DisabledEnum"=w2403) -> ()  [unwired: 2 in, 2 out]
        n1410 = property on="Set Scan \nParameters" class="Bool"("DisabledEnum"=w2403) -> ()  [unwired: 2 in, 2 out]
        n1411 = property on="Send scan parameter" class="Bool"("DisabledEnum"=w2403) -> ()  [unwired: 2 in, 2 out]
      }
      event #15 {
        n1412 = event-data() -> ()  [unwired: 1 in, 7 out]
        n1413 = flat-sequence {
          tunnel: [w2658] -> _
          tunnel: [w2659] -> _
          tunnel: w2651 -> [w2656]
          tunnel: w2647 -> [w2655]
          frame #0 {
            n1414 = property on="Reset R Motor Steps" class="DigNum (strict)"() -> ("Value"=w2657:i32)  [unwired: 2 in, 2 out]
            n1415 = Number To Decimal String(number=w2657) -> (decimal integer string=w2660:string)  [unwired: 1 in]
            n1416 = call "mDrive Send Command.vi"("error in (no error)"=w2656, "Extra"=w2660, "Command"=T10."Set Current Position", "VISA resource name"=w2655) -> ("error out"=w2659:errorcluster, "VISA resource name out"=w2658:refnum<visa-resource-name>)  [unwired: 3 in, 1 out]
          }
        }
        n1417 = flat-sequence {
          tunnel: [w2678] -> _
          tunnel: [w2679] -> _
          tunnel: w2654 -> [w2677]
          tunnel: w2650 -> [w2676]
          frame #0 {
            n1418 = property on="Reset X Motor Steps" class="DigNum (strict)"() -> ("Value"=w2680:i32)  [unwired: 2 in, 2 out]
            n1419 = Number To Decimal String(number=w2680) -> (decimal integer string=w2681:string)  [unwired: 1 in]
            n1420 = call "mDrive Send Command.vi"("error in (no error)"=w2677, "Extra"=w2681, "Command"=T10."Set Current Position", "VISA resource name"=w2676) -> ("error out"=w2679:errorcluster, "VISA resource name out"=w2678:refnum<visa-resource-name>)  [unwired: 3 in, 1 out]
          }
        }
        n1421 = flat-sequence {
          tunnel: [w2672] -> _
          tunnel: [w2673] -> _
          tunnel: w2653 -> [w2670]
          tunnel: w2649 -> [w2669]
          frame #0 {
            n1422 = property on="Reset Z Motor Steps" class="DigNum (strict)"() -> ("Value"=w2671:i32)  [unwired: 2 in, 2 out]
            n1423 = Number To Decimal String(number=w2671) -> (decimal integer string=w2674:string)  [unwired: 1 in]
            n1424 = call "mDrive Send Command.vi"("error in (no error)"=w2670, "Extra"=w2674, "Command"=T10."Set Current Position", "VISA resource name"=w2669) -> ("error out"=w2673:errorcluster, "VISA resource name out"=w2672:refnum<visa-resource-name>)  [unwired: 3 in, 1 out]
          }
        }
        n1425 = flat-sequence {
          tunnel: [w2665] -> _
          tunnel: [w2666] -> _
          tunnel: w2652 -> [w2663]
          tunnel: w2648 -> [w2662]
          frame #0 {
            n1426 = property on="Reset Y Motor Steps" class="DigNum (strict)"() -> ("Value"=w2664:i32)  [unwired: 2 in, 2 out]
            n1427 = Number To Decimal String(number=w2664) -> (decimal integer string=w2667:string)  [unwired: 1 in]
            n1428 = call "mDrive Send Command.vi"("error in (no error)"=w2663, "Extra"=w2667, "Command"=T10."Set Current Position", "VISA resource name"=w2662) -> ("error out"=w2666:errorcluster, "VISA resource name out"=w2665:refnum<visa-resource-name>)  [unwired: 3 in, 1 out]
          }
        }
      }
      event #16 {
        n1429 = event-data() -> ()  [unwired: 1 in, 7 out]
        n1430 = flat-sequence {
          tunnel: w2702 -> [w4288]
          tunnel: [w4288] -> w2701
          tunnel: w2700 -> [w4287]
          tunnel: [w4287] -> w2699
          tunnel: w2698 -> [w4286]
          tunnel: [w4286] -> w2697
          tunnel: w2696 -> [w4285]
          tunnel: [w4285] -> w2695
          tunnel: w2694 -> [w4284]
          tunnel: [w4284] -> w2693
          tunnel: w2692 -> [w4283]
          tunnel: [w4283] -> w2691
          tunnel: w2690 -> [w4282]
          tunnel: [w4282] -> w2689
          tunnel: w2688 -> [w4281]
          tunnel: [w4281] -> w2687
          frame #0 {
            w4289 = T9."Disabled and Grayed Out" ("Disabled")
            n1431 = local write "STATUS"("ENTERING LOOP" ("STATUS")) -> ()
            n1432 = property on="Z Scan Length SP steps" class="DigNum (strict)"("DisabledEnum"=T9."Disabled and Grayed Out" ("Disabled")) -> ()  [unwired: 2 in, 2 out]
            n1433 = property on="Z Scan Velocity SP steps/sec" class="DigNum (strict)"("DisabledEnum"=T9."Disabled and Grayed Out" ("Disabled")) -> ()  [unwired: 2 in, 2 out]
            n1434 = property on="GO" class="Bool"("DisabledEnum"=w4289) -> ()  [unwired: 2 in, 2 out]
            n1435 = property on="Set Scan \nParameters" class="Bool"("DisabledEnum"=w4289) -> ()  [unwired: 2 in, 2 out]
            n1436 = property on="Scan Go" class="Bool (strict)"("DisabledEnum"=w4289) -> ()  [unwired: 2 in, 2 out]
            n1437 = property on="Send scan parameter" class="Bool"("DisabledEnum"=w4289) -> ()  [unwired: 2 in, 2 out]
            n1438 = property on="R Scan Length SP steps" class="DigNum (strict)"("DisabledEnum"=T9."Disabled and Grayed Out" ("Disabled")) -> ()  [unwired: 2 in, 2 out]
            n1439 = property on="R Scan Velocity SP steps/sec" class="DigNum (strict)"("DisabledEnum"=T9."Disabled and Grayed Out" ("Disabled")) -> ()  [unwired: 2 in, 2 out]
            n1440 = property on="Y Scan Length SP steps" class="DigNum (strict)"("DisabledEnum"=T9."Disabled and Grayed Out" ("Disabled")) -> ()  [unwired: 2 in, 2 out]
            n1441 = property on="Y Scan Velocity SP steps/sec" class="DigNum (strict)"("DisabledEnum"=T9."Disabled and Grayed Out" ("Disabled")) -> ()  [unwired: 2 in, 2 out]
            n1442 = property on="X Scan Length SP steps" class="DigNum (strict)"("DisabledEnum"=T9."Disabled and Grayed Out" ("Disabled")) -> ()  [unwired: 2 in, 2 out]
            n1443 = property on="X Scan Velocity SP steps/sec" class="DigNum (strict)"("DisabledEnum"=T9."Disabled and Grayed Out" ("Disabled")) -> ()  [unwired: 2 in, 2 out]
          }
        }
        n1444 = while {
          tunnel: w2697 -> [w2759]
          tunnel: w2693 -> [w2758]
          tunnel: w2695 -> [w2757]
          tunnel: w2691 -> [w2756]
          tunnel: w2689 -> [w2755]
          tunnel: w2687 -> [w2754]
          tunnel: w2699 -> [w2753]
          tunnel: w2701 -> [w2752]
          tunnel: [w2751] -> w2686 mode=indexing
          tunnel: [w2750] -> w2685 mode=indexing
          tunnel: [w2749] -> w2684 mode=indexing
          tunnel: [w2748] -> w2683 mode=indexing
          i -> [w2714]
          stop <- w2703 stop-if-true
          # "XZYR"
          n1445 = flat-sequence {
            tunnel: w2758 -> [w2787]
            tunnel: w2759 -> [w2788]
            tunnel: [w2784] -> w2775
            tunnel: [w2777] -> w2774
            tunnel: [w2783] -> w2773
            tunnel: [w2782] -> w2772
            tunnel: [w2781] -> w2771
            tunnel: [w2780] -> w2770
            tunnel: [w2776] -> w2769
            tunnel: [w2779] -> w2768
            tunnel: w2757 -> [w2792]
            tunnel: w2756 -> [w2791]
            tunnel: w2755 -> [w2790]
            tunnel: w2754 -> [w2789]
            tunnel: w2753 -> [w2786]
            tunnel: w2752 -> [w2785]
            tunnel: [w2922] -> w2731
            tunnel: [w2921] -> w2729
            tunnel: [w2920] -> w2727
            tunnel: [w2919] -> w2725
            tunnel: [w2917] -> w2723
            tunnel: [w2916] -> w2721
            tunnel: [w2918] -> w2719
            tunnel: w2775 -> [w2915]
            tunnel: w2774 -> [w2914]
            tunnel: w2773 -> [w2913]
            tunnel: w2772 -> [w2912]
            tunnel: w2771 -> [w2911]
            tunnel: w2770 -> [w2910]
            tunnel: w2769 -> [w2909]
            tunnel: w2768 -> [w2908]
            tunnel: [w2907] -> w2717
            tunnel: w2731 -> [w3047]
            tunnel: [w3047] -> w2730
            tunnel: w2729 -> [w3046]
            tunnel: [w3046] -> w2728
            tunnel: w2727 -> [w3045]
            tunnel: [w3045] -> w2726
            tunnel: w2725 -> [w3044]
            tunnel: [w3044] -> w2724
            tunnel: w2723 -> [w3043]
            tunnel: [w3043] -> w2722
            tunnel: w2721 -> [w3042]
            tunnel: [w3042] -> w2720
            tunnel: w2719 -> [w3041]
            tunnel: [w3041] -> w2718
            tunnel: w2717 -> [w3040]
            tunnel: [w3040] -> w2716
            tunnel: [w3062] -> w2747
            tunnel: [w3060] -> w2745
            tunnel: [w3053] -> w2743
            tunnel: [w3052] -> w2741
            tunnel: [w3051] -> w2739
            tunnel: [w3050] -> w2737
            tunnel: [w3049] -> w2735
            tunnel: [w3048] -> w2733
            tunnel: w2730 -> [w3063]
            tunnel: w2728 -> [w3061]
            tunnel: w2726 -> [w3058]
            tunnel: w2724 -> [w3057]
            tunnel: w2722 -> [w3055]
            tunnel: w2720 -> [w3054]
            tunnel: w2718 -> [w3056]
            tunnel: w2716 -> [w3059]
            tunnel: w2747 -> [w3342]
            tunnel: [w3342] -> w2746
            tunnel: w2745 -> [w3341]
            tunnel: [w3341] -> w2744
            tunnel: w2743 -> [w3340]
            tunnel: [w3340] -> w2742
            tunnel: w2741 -> [w3339]
            tunnel: [w3339] -> w2740
            tunnel: w2739 -> [w3338]
            tunnel: [w3338] -> w2738
            tunnel: w2737 -> [w3337]
            tunnel: [w3337] -> w2736
            tunnel: w2735 -> [w3336]
            tunnel: [w3336] -> w2734
            tunnel: w2733 -> [w3335]
            tunnel: [w3335] -> w2732
            tunnel: w2746 -> [w3360]
            tunnel: w2744 -> [w3358]
            tunnel: w2742 -> [w3359]
            tunnel: w2740 -> [w3357]
            tunnel: w2738 -> [w3356]
            tunnel: w2736 -> [w3355]
            tunnel: w2734 -> [w3354]
            tunnel: w2732 -> [w3353]
            tunnel: [w3352] -> w2767
            tunnel: [w3351] -> w2766
            tunnel: [w3350] -> w2765
            tunnel: [w3349] -> w2764
            tunnel: [w3348] -> w2763
            tunnel: [w3347] -> w2762
            tunnel: [w3346] -> w2761
            tunnel: [w3345] -> w2760
            tunnel: w2767 -> [w3653]
            tunnel: w2766 -> [w3654]
            tunnel: w2765 -> [w3656]
            tunnel: w2764 -> [w3655]
            tunnel: w2763 -> [w3659]
            tunnel: w2762 -> [w3660]
            tunnel: w2761 -> [w3657]
            tunnel: w2760 -> [w3658]
            tunnel: [w3662] -> w2713
            tunnel: [w3661] -> w2712
            tunnel: [w3663] -> w2711
            tunnel: [w3664] -> w2710
            tunnel: [w3667] -> w2709
            tunnel: [w3668] -> w2708
            tunnel: [w3665] -> w2707
            tunnel: [w3666] -> w2706
            tunnel: [w4260] -> _
            tunnel: [w4261] -> w2751
            tunnel: [w4262] -> _
            tunnel: [w4263] -> w2750
            tunnel: [w4264] -> _
            tunnel: [w4265] -> w2748
            tunnel: [w4266] -> w2749
            tunnel: [w4267] -> _
            tunnel: w2713 -> [w4267]
            tunnel: w2712 -> [w4266]
            tunnel: w2711 -> [w4265]
            tunnel: w2710 -> [w4264]
            tunnel: w2709 -> [w4263]
            tunnel: w2708 -> [w4262]
            tunnel: w2707 -> [w4261]
            tunnel: w2706 -> [w4260]
            frame #0 {
              n1446 = flat-sequence {
                tunnel: [w2884] -> w2816
                tunnel: [w2883] -> w2815
                tunnel: w2787 -> [w2886]
                tunnel: w2788 -> [w2885]
                tunnel: w2816 -> [w2892]
                tunnel: [w2892] -> w2814
                tunnel: w2815 -> [w2891]
                tunnel: [w2891] -> w2813
                tunnel: w2814 -> [w2896]
                tunnel: [w2895] -> w2812
                tunnel: w2813 -> [w2894]
                tunnel: [w2893] -> w2811
                tunnel: w2812 -> [w2904]
                tunnel: w2811 -> [w2902]
                tunnel: [w2904] -> w2784
                tunnel: [w2902] -> w2777
                frame #0 {
                  n1447 = property on="X Scan Velocity SP steps/sec" class="DigNum (strict)"() -> ("Value"=w2888:i32)  [unwired: 2 in, 2 out]
                  n1448 = Number To Decimal String(number=w2888) -> (decimal integer string=w2889:string)  [unwired: 1 in]
                  n1449 = call "mDrive Send Command.vi"("error in (no error)"=w2886, "Extra"=w2889, "Command"=T10."Max Velocity", "VISA resource name"=w2885) -> ("error out"=w2883:errorcluster, "VISA resource name out"=w2884:refnum<visa-resource-name>)  [unwired: 3 in, 1 out]
                }
                frame #1 {
                  n1450 = Wait (ms)(milliseconds to wait=u32 100) -> ()  [unwired: 1 out]
                }
                frame #2 {
                  # "VELOCITY"
                  n1451 = call "mDrive Send Command.vi"("error in (no error)"=w2894, "Extra"="VM", "Command"=T10."Print Parameter", "VISA resource name"=w2896) -> ("error out"=w2893:errorcluster, "read buffer"=w2899:string, "VISA resource name out"=w2895:refnum<visa-resource-name>)  [unwired: 3 in]
                  n1452 = Decimal String To Number(string=w2899, offset=0) -> (number=w2897:i32)  [unwired: 1 in, 1 out]
                  n1453 = property on="X velocity PV step/sec" class="DigNum (strict)"("Val(Sgnl)"=w2897) -> ()  [unwired: 2 in, 2 out]
                }
                frame #3 {
                  n1454 = Wait (ms)(milliseconds to wait=u32 100) -> ()  [unwired: 1 out]
                }
              }
              n1455 = flat-sequence {
                tunnel: [w2842] -> w2804
                tunnel: [w2841] -> w2803
                tunnel: w2791 -> [w2840]
                tunnel: w2792 -> [w2839]
                tunnel: w2804 -> [w2848]
                tunnel: [w2848] -> w2802
                tunnel: w2803 -> [w2847]
                tunnel: [w2847] -> w2801
                tunnel: w2802 -> [w2854]
                tunnel: [w2853] -> w2800
                tunnel: w2801 -> [w2852]
                tunnel: [w2851] -> w2799
                tunnel: w2800 -> [w2860]
                tunnel: w2799 -> [w2859]
                tunnel: [w2860] -> w2783
                tunnel: [w2859] -> w2782
                frame #0 {
                  n1456 = property on="Z Scan Velocity SP steps/sec" class="DigNum (strict)"() -> ("Value"=w2844:i32)  [unwired: 2 in, 2 out]
                  n1457 = Number To Decimal String(number=w2844) -> (decimal integer string=w2845:string)  [unwired: 1 in]
                  n1458 = call "mDrive Send Command.vi"("error in (no error)"=w2840, "Extra"=w2845, "Command"=T10."Max Velocity", "VISA resource name"=w2839) -> ("error out"=w2841:errorcluster, "VISA resource name out"=w2842:refnum<visa-resource-name>)  [unwired: 3 in, 1 out]
                }
                frame #1 {
                  n1459 = Wait (ms)(milliseconds to wait=u32 100) -> ()  [unwired: 1 out]
                }
                frame #2 {
                  # "VELOCITY"
                  n1460 = call "mDrive Send Command.vi"("error in (no error)"=w2852, "Extra"="VM", "Command"=T10."Print Parameter", "VISA resource name"=w2854) -> ("error out"=w2851:errorcluster, "read buffer"=w2855:string, "VISA resource name out"=w2853:refnum<visa-resource-name>)  [unwired: 3 in]
                  n1461 = Decimal String To Number(string=w2855, offset=0) -> (number=w2856:i32)  [unwired: 1 in, 1 out]
                  n1462 = property on="Z  velocity PV step/sec" class="DigNum (strict)"("Val(Sgnl)"=w2856) -> ()  [unwired: 2 in, 2 out]
                }
                frame #3 {
                  n1463 = Wait (ms)(milliseconds to wait=u32 100) -> ()  [unwired: 1 out]
                }
              }
              n1464 = flat-sequence {
                tunnel: [w2864] -> w2810
                tunnel: [w2863] -> w2809
                tunnel: w2789 -> [w2862]
                tunnel: w2790 -> [w2861]
                tunnel: w2810 -> [w2870]
                tunnel: [w2870] -> w2808
                tunnel: w2809 -> [w2869]
                tunnel: [w2869] -> w2807
                tunnel: w2808 -> [w2874]
                tunnel: [w2873] -> w2806
                tunnel: w2807 -> [w2872]
                tunnel: [w2871] -> w2805
                tunnel: w2806 -> [w2882]
                tunnel: w2805 -> [w2881]
                tunnel: [w2882] -> w2781
                tunnel: [w2881] -> w2780
                frame #0 {
                  n1465 = property on="Y Scan Velocity SP steps/sec" class="DigNum (strict)"() -> ("Value"=w2866:i32)  [unwired: 2 in, 2 out]
                  n1466 = Number To Decimal String(number=w2866) -> (decimal integer string=w2867:string)  [unwired: 1 in]
                  n1467 = call "mDrive Send Command.vi"("error in (no error)"=w2862, "Extra"=w2867, "Command"=T10."Max Velocity", "VISA resource name"=w2861) -> ("error out"=w2863:errorcluster, "VISA resource name out"=w2864:refnum<visa-resource-name>)  [unwired: 3 in, 1 out]
                }
                frame #1 {
                  n1468 = Wait (ms)(milliseconds to wait=u32 100) -> ()  [unwired: 1 out]
                }
                frame #2 {
                  # "VELOCITY"
                  n1469 = call "mDrive Send Command.vi"("error in (no error)"=w2872, "Extra"="VM", "Command"=T10."Print Parameter", "VISA resource name"=w2874) -> ("error out"=w2871:errorcluster, "read buffer"=w2878:string, "VISA resource name out"=w2873:refnum<visa-resource-name>)  [unwired: 3 in]
                  n1470 = Decimal String To Number(string=w2878, offset=0) -> (number=w2876:i32)  [unwired: 1 in, 1 out]
                  n1471 = property on="Y velocity PV step/sec" class="DigNum (strict)"("Val(Sgnl)"=w2876) -> ()  [unwired: 2 in, 2 out]
                }
                frame #3 {
                  n1472 = Wait (ms)(milliseconds to wait=u32 100) -> ()  [unwired: 1 out]
                }
              }
              n1473 = flat-sequence {
                tunnel: [w2820] -> w2798
                tunnel: [w2819] -> w2797
                tunnel: w2786 -> [w2818]
                tunnel: w2785 -> [w2817]
                tunnel: w2798 -> [w2826]
                tunnel: [w2826] -> w2796
                tunnel: w2797 -> [w2825]
                tunnel: [w2825] -> w2795
                tunnel: w2796 -> [w2832]
                tunnel: [w2831] -> w2794
                tunnel: w2795 -> [w2830]
                tunnel: [w2829] -> w2793
                tunnel: w2794 -> [w2836]
                tunnel: w2793 -> [w2838]
                tunnel: [w2838] -> w2779
                tunnel: [w2836] -> w2776
                frame #0 {
                  n1474 = property on="R Scan Velocity SP steps/sec" class="DigNum (strict)"() -> ("Value"=w2822:i32)  [unwired: 2 in, 2 out]
                  n1475 = Number To Decimal String(number=w2822) -> (decimal integer string=w2823:string)  [unwired: 1 in]
                  n1476 = call "mDrive Send Command.vi"("error in (no error)"=w2818, "Extra"=w2823, "Command"=T10."Max Velocity", "VISA resource name"=w2817) -> ("error out"=w2819:errorcluster, "VISA resource name out"=w2820:refnum<visa-resource-name>)  [unwired: 3 in, 1 out]
                }
                frame #1 {
                  n1477 = Wait (ms)(milliseconds to wait=u32 100) -> ()  [unwired: 1 out]
                }
                frame #2 {
                  # "VELOCITY"
                  n1478 = call "mDrive Send Command.vi"("error in (no error)"=w2830, "Extra"="VM", "Command"=T10."Print Parameter", "VISA resource name"=w2832) -> ("error out"=w2829:errorcluster, "read buffer"=w2834:string, "VISA resource name out"=w2831:refnum<visa-resource-name>)  [unwired: 3 in]
                  n1479 = Decimal String To Number(string=w2834, offset=0) -> (number=w2833:i32)  [unwired: 1 in, 1 out]
                  n1480 = property on="R velocity PV step/sec" class="DigNum (strict)"("Val(Sgnl)"=w2833) -> ()  [unwired: 2 in, 2 out]
                }
                frame #3 {
                  n1481 = Wait (ms)(milliseconds to wait=u32 100) -> ()  [unwired: 1 out]
                }
              }
              n1482 = local write "STATUS"("LOOP INITIALIZING" ("STATUS")) -> ()
            }
            frame #1 {
              w2905 = TRUE ("R in Motion")
              n1483 = flat-sequence {
                tunnel: [w2982] -> w2950
                tunnel: [w2981] -> w2949
                tunnel: [w2980] -> w2948
                tunnel: [w2979] -> w2947
                tunnel: w2915 -> [w2978]
                tunnel: w2914 -> [w2977]
                tunnel: w2913 -> [w2976]
                tunnel: w2912 -> [w2975]
                tunnel: w2911 -> [w2974]
                tunnel: w2910 -> [w2973]
                tunnel: w2909 -> [w2972]
                tunnel: w2908 -> [w2971]
                tunnel: [w2978] -> w2946
                tunnel: [w2977] -> w2945
                tunnel: [w2976] -> w2944
                tunnel: [w2975] -> w2943
                tunnel: [w2974] -> w2942
                tunnel: [w2973] -> w2941
                tunnel: [w2972] -> w2940
                tunnel: [w2971] -> w2939
                tunnel: [w3002] -> w2938
                tunnel: [w3001] -> w2937
                tunnel: w2950 -> [w3000]
                tunnel: w2949 -> [w2999]
                tunnel: w2948 -> [w2998]
                tunnel: w2947 -> [w2997]
                tunnel: [w2996] -> w2936
                tunnel: [w2995] -> w2935
                tunnel: [w2994] -> w2934
                tunnel: [w2993] -> w2933
                tunnel: [w2992] -> w2932
                tunnel: [w2991] -> w2931
                tunnel: w2946 -> [w2990]
                tunnel: w2945 -> [w2989]
                tunnel: w2944 -> [w2988]
                tunnel: w2943 -> [w2987]
                tunnel: w2942 -> [w2986]
                tunnel: w2941 -> [w2985]
                tunnel: w2940 -> [w2984]
                tunnel: w2939 -> [w2983]
                tunnel: w2938 -> [w3011]
                tunnel: [w3011] -> w2930
                tunnel: w2937 -> [w3010]
                tunnel: [w3010] -> w2929
                tunnel: [w3009] -> w2928
                tunnel: w2936 -> [w3009]
                tunnel: [w3008] -> w2927
                tunnel: w2935 -> [w3008]
                tunnel: [w3007] -> w2926
                tunnel: w2934 -> [w3007]
                tunnel: [w3006] -> w2925
                tunnel: w2933 -> [w3006]
                tunnel: [w3005] -> w2924
                tunnel: w2932 -> [w3005]
                tunnel: [w3004] -> w2923
                tunnel: w2931 -> [w3004]
                tunnel: w2930 -> [w3039]
                tunnel: w2929 -> [w3038]
                tunnel: w2928 -> [w3035]
                tunnel: w2927 -> [w3034]
                tunnel: w2926 -> [w3033]
                tunnel: w2925 -> [w3032]
                tunnel: w2924 -> [w3031]
                tunnel: w2923 -> [w3030]
                tunnel: [w3037] -> w2919
                tunnel: [w3036] -> w2918
                tunnel: [w3029] -> w2920
                tunnel: [w3028] -> w2917
                tunnel: [w3027] -> w2916
                tunnel: [w3026] -> w2922
                tunnel: [w3025] -> w2921
                tunnel: [w3012] -> w2907
                frame #0 {
                  n1484 = property on="X Scan Length SP steps" class="DigNum (strict)"() -> ("Value"=w2965:i32)  [unwired: 2 in, 2 out]
                  n1485 = property on="Z Scan Length SP steps" class="DigNum (strict)"() -> ("Value"=w2970:i32)  [unwired: 2 in, 2 out]
                  n1486 = property on="Y Scan Length SP steps" class="DigNum (strict)"() -> ("Value"=w2960:i32)  [unwired: 2 in, 2 out]
                  n1487 = property on="R Scan Length SP steps" class="DigNum (strict)"() -> ("Value"=w2955:i32)  [unwired: 2 in, 2 out]
                  n1488 = Number To Decimal String(number=w2965) -> (decimal integer string=w2962:string)  [unwired: 1 in]
                  n1489 = Number To Decimal String(number=w2970) -> (decimal integer string=w2967:string)  [unwired: 1 in]
                  n1490 = Number To Decimal String(number=w2960) -> (decimal integer string=w2957:string)  [unwired: 1 in]
                  n1491 = Number To Decimal String(number=w2955) -> (decimal integer string=w2952:string)  [unwired: 1 in]
                  n1492 = call <vilib>:"Space Constant.vi"() -> ("String"=w2963:string)
                  n1493 = call <vilib>:"Space Constant.vi"() -> ("String"=w2968:string)
                  n1494 = call <vilib>:"Space Constant.vi"() -> ("String"=w2958:string)
                  n1495 = call <vilib>:"Space Constant.vi"() -> ("String"=w2953:string)
                  n1496 = Concatenate Strings("MR", w2963, w2962, "\r") -> (w2981:string)
                  n1497 = Concatenate Strings("MR", w2968, w2967, "\r") -> (w2980:string)
                  n1498 = Concatenate Strings("MR", w2958, w2957, "\r") -> (w2982:string)
                  n1499 = Concatenate Strings("MR", w2953, w2952, "\r") -> (w2979:string)
                }
                frame #1 {
                  n1500 = VISA Write(VISA resource name=w2990, write buffer=w2999, error in (no error)=w2989) -> (VISA resource name out=w2996:refnum<visa-resource-name>, error out=w2995:errorcluster)  [unwired: 1 out]
                  n1501 = VISA Write(VISA resource name=w2988, write buffer=w2998, error in (no error)=w2987) -> (VISA resource name out=w2992:refnum<visa-resource-name>, error out=w2991:errorcluster)  [unwired: 1 out]
                  n1502 = VISA Write(VISA resource name=w2986, write buffer=w3000, error in (no error)=w2985) -> (VISA resource name out=w3002:refnum<visa-resource-name>, error out=w3001:errorcluster)  [unwired: 1 out]
                  n1503 = VISA Write(VISA resource name=w2984, write buffer=w2997, error in (no error)=w2983) -> (VISA resource name out=w2994:refnum<visa-resource-name>, error out=w2993:errorcluster)  [unwired: 1 out]
                }
                frame #2 {
                  n1504 = Wait (ms)(milliseconds to wait=u32 100) -> ()  [unwired: 1 out]
                }
                frame #3 {
                  n1505 = property class="Instr"(reference=w3035, error in=w3034) -> (reference out=w3017:refnum<visa-resource-name>, error out=w3016:errorcluster, "Serial Settings:Number of Bytes at Serial Port"=w3018:u32)
                  n1506 = property class="Instr"(reference=w3031, error in=w3030) -> (reference out=w3014:refnum<visa-resource-name>, error out=w3013:errorcluster, "Serial Settings:Number of Bytes at Serial Port"=w3015:u32)
                  n1507 = property class="Instr"(reference=w3039, error in=w3038) -> (reference out=w3020:refnum<visa-resource-name>, error out=w3019:errorcluster, "Serial Settings:Number of Bytes at Serial Port"=w3021:u32)
                  n1508 = property class="Instr"(reference=w3033, error in=w3032) -> (reference out=w3023:refnum<visa-resource-name>, error out=w3022:errorcluster, "Serial Settings:Number of Bytes at Serial Port"=w3024:u32)
                  n1509 = VISA Read(VISA resource name=w3017, byte count=w3018, error in (no error)=w3016) -> (VISA resource name out=w3026:refnum<visa-resource-name>, error out=w3025:errorcluster)  [unwired: 2 out]
                  n1510 = VISA Read(VISA resource name=w3014, byte count=w3015, error in (no error)=w3013) -> (VISA resource name out=w3012:refnum<visa-resource-name>, error out=w3029:errorcluster)  [unwired: 2 out]
                  n1511 = VISA Read(VISA resource name=w3020, byte count=w3021, error in (no error)=w3019) -> (VISA resource name out=w3037:refnum<visa-resource-name>, error out=w3036:errorcluster)  [unwired: 2 out]
                  n1512 = VISA Read(VISA resource name=w3023, byte count=w3024, error in (no error)=w3022) -> (VISA resource name out=w3028:refnum<visa-resource-name>, error out=w3027:errorcluster)  [unwired: 2 out]
                }
              }
              n1513 = local write "STATUS"("LOOP SCANNING" ("STATUS")) -> ()
              n1514 = property on="Y in Motion" class="Bool (strict)"("Value"=w2905) -> ()  [unwired: 2 in, 2 out]
              n1515 = property on="Z in Motion" class="Bool (strict)"("Value"=w2905) -> ()  [unwired: 2 in, 2 out]
              n1516 = property on="X  in Motion" class="Bool (strict)"("Value"=w2905) -> ()  [unwired: 2 in, 2 out]
              n1517 = property on="R in Motion" class="Bool (strict)"("Value"=w2905) -> ()  [unwired: 2 in, 2 out]
            }
            frame #2 {
            }
            frame #3 {
              n1518 = while {
                tunnel: w3063 -> [w3085]
                tunnel: [w3073] -> w3062
                tunnel: w3061 -> [w3084]
                tunnel: [w3072] -> w3060
                tunnel: w3059 -> [w3083]
                tunnel: w3058 -> [w3082]
                tunnel: w3057 -> [w3081]
                tunnel: w3056 -> [w3080]
                tunnel: w3055 -> [w3079]
                tunnel: w3054 -> [w3078]
                tunnel: [w3075] -> w3053
                tunnel: [w3074] -> w3052
                tunnel: [w3071] -> w3051
                tunnel: [w3070] -> w3050
                tunnel: [w3069] -> w3049
                tunnel: [w3068] -> w3048
                stop <- w3064 stop-if-true
                n1519 = flat-sequence {
                  tunnel: [w3286] -> w3121
                  tunnel: [w3285] -> w3120
                  tunnel: [w3284] -> w3119
                  tunnel: w3085 -> [w3283]
                  tunnel: w3084 -> [w3282]
                  tunnel: [w3308] -> w3118
                  tunnel: [w3307] -> w3117
                  tunnel: [w3305] -> w3116
                  tunnel: w3121 -> [w3305]
                  tunnel: w3120 -> [w3304]
                  tunnel: w3119 -> [w3303]
                  tunnel: w3118 -> [w3321]
                  tunnel: [w3321] -> w3113
                  tunnel: w3117 -> [w3320]
                  tunnel: [w3320] -> w3114
                  tunnel: w3116 -> [w3319]
                  tunnel: [w3319] -> w3115
                  tunnel: w3115 -> [w3324]
                  tunnel: w3114 -> [w3326]
                  tunnel: w3113 -> [w3325]
                  tunnel: [w3323] -> w3073
                  tunnel: [w3322] -> w3072
                  frame #0 {
                    n1520 = property on="X Step SP" class="DigNum (strict)"() -> ("Maximum"=w3298:dbl)  [unwired: 2 in, 2 out]
                    n1521 = property on="X Step SP" class="DigNum (strict)"() -> ("Minimum"=w3300:dbl)  [unwired: 2 in, 2 out]
                    n1522 = property on="X steps/rev" class="DigNum (strict)"() -> ("Value"=w3295:u32)  [unwired: 2 in, 2 out]
                    n1523 = property on="X offset mm" class="DigNum (strict)"() -> ("Value"=w3291:dbl)  [unwired: 2 in, 2 out]
                    n1524 = To Long Integer(number=w3298) -> (32bit integer=w3297:i32)
                    n1525 = To Long Integer(number=w3300) -> (32bit integer=w3299:i32)
                    n1526 = To Double Precision Float(number=w3295) -> (double precision float=w3296:dbl)
                    n1527 = call "mDrive Send Command.vi"("error in (no error)"=w3282, "Extra"="P", "Command"=T10."Print Parameter", "VISA resource name"=w3283) -> ("error out"=w3284:errorcluster, "read buffer"=w3302:string, "VISA resource name out"=w3285:refnum<visa-resource-name>)  [unwired: 3 in]
                    n1528 = Decimal String To Number(string=w3302, offset=0) -> (number=w3281:i32)  [unwired: 1 in, 1 out]
                    n1529 = property on="X Step PV" class="DigNum (strict)"("Val(Sgnl)"=w3281) -> ()  [unwired: 2 in, 2 out]
                    n1530 = In Range and Coerce(upper limit=w3297, x=w3281, lower limit=w3299) -> (In Range?=w3286:bool)  [unwired: 1 out]
                    n1531 = To Double Precision Float(number=w3281) -> (double precision float=w3290:dbl)
                    n1532 = property on="X  in Range" class="Bool (strict)"("Val(Sgnl)"=w3286) -> ()  [unwired: 2 in, 2 out]
                    n1533 = Divide(x=w3290, y=w3296) -> (x/y=w3294:dbl)
                    n1534 = property on="X mm/rev" class="DigNum (strict)"() -> ("Value"=w3293:dbl)  [unwired: 2 in, 2 out]
                    n1535 = Multiply(x=w3294, y=w3293) -> (x*y=w3292:dbl)
                    n1536 = Add(x=w3292, y=w3291) -> (x+y=w3289:dbl)
                    n1537 = property on="X Position mm PV" class="DigNum (strict)"("Val(Sgnl)"=w3289) -> ()  [unwired: 2 in, 2 out]
                  }
                  frame #1 {
                    n1538 = call "mDrive Send Command.vi"("error in (no error)"=w3303, "Extra"="MV", "Command"=T10."Print Parameter", "VISA resource name"=w3304) -> ("error out"=w3307:errorcluster, "read buffer"=w3311:string, "VISA resource name out"=w3308:refnum<visa-resource-name>)  [unwired: 3 in]
                    n1539 = Decimal String To Number(string=w3311, offset=0 ("offset (0)")) -> (number=w3314:i32)  [unwired: 1 in, 1 out]
                    n1540 = Not Equal?(x=w3311, y="") -> (x != y?=w3309:bool)
                    n1541 = property on="X Ready" class="Bool (strict)"("Val(Sgnl)"=w3309) -> ()  [unwired: 2 in, 2 out]
                    n1542 = Number To Boolean Array(number=w3314) -> (Boolean array=w3313:bool[])
                    n1543 = Index Array(array=w3313, index=0) -> (element=w3306:bool)
                    n1544 = property on="X  in Motion" class="Bool (strict)"("Val(Sgnl)"=w3306) -> ()  [unwired: 2 in, 2 out]
                  }
                  frame #2 {
                    n1545 = Wait (ms)(milliseconds to wait=u32 10) -> ()  [unwired: 1 out]
                  }
                  frame #3 {
                    n1546 = case shown="False" w3324 {
                      tunnel: w3325 -> [w3329 w3333]
                      tunnel: [w3330 w3333] -> w3323
                      tunnel: [w3331 w3332] -> w3322
                      tunnel: w3326 -> [w3328 w3332]
                      frame #0 {
                        n1547 = call "mDrive Send Command.vi"("error in (no error)"=w3328, "Command"=T10."Stop", "VISA resource name"=w3329) -> ("error out"=w3331:errorcluster, "VISA resource name out"=w3330:refnum<visa-resource-name>)  [unwired: 4 in, 1 out]
                      }
                      frame #1 {
                      }
                    }
                  }
                }
                n1548 = flat-sequence {
                  tunnel: [w3239] -> w3112
                  tunnel: [w3230] -> w3111
                  tunnel: [w3229] -> w3110
                  tunnel: w3083 -> [w3233]
                  tunnel: w3082 -> [w3232]
                  tunnel: [w3259] -> w3109
                  tunnel: [w3258] -> w3108
                  tunnel: [w3257] -> w3107
                  tunnel: w3112 -> [w3257]
                  tunnel: w3111 -> [w3256]
                  tunnel: w3110 -> [w3255]
                  tunnel: w3109 -> [w3268]
                  tunnel: [w3268] -> w3104
                  tunnel: w3108 -> [w3267]
                  tunnel: [w3267] -> w3105
                  tunnel: w3107 -> [w3266]
                  tunnel: [w3266] -> w3106
                  tunnel: w3106 -> [w3271]
                  tunnel: w3105 -> [w3273]
                  tunnel: w3104 -> [w3272]
                  tunnel: [w3270] -> w3075
                  tunnel: [w3269] -> w3074
                  frame #0 {
                    n1549 = property on="Z Step SP" class="DigNum (strict)"() -> ("Maximum"=w3240:dbl)  [unwired: 2 in, 2 out]
                    n1550 = property on="Z Step SP" class="DigNum (strict)"() -> ("Minimum"=w3234:dbl)  [unwired: 2 in, 2 out]
                    n1551 = property on="Z steps/rev" class="DigNum (strict)"() -> ("Value"=w3238:u32)  [unwired: 2 in, 2 out]
                    n1552 = property on="Z offset mm" class="DigNum (strict)"() -> ("Value"=w3236:dbl)  [unwired: 2 in, 2 out]
                    n1553 = To Long Integer(number=w3240) -> (32bit integer=w3246:i32)
                    n1554 = To Long Integer(number=w3234) -> (32bit integer=w3247:i32)
                    n1555 = To Double Precision Float(number=w3238) -> (double precision float=w3245:dbl)
                    n1556 = call "mDrive Send Command.vi"("error in (no error)"=w3232, "Extra"="P", "Command"=T10."Print Parameter", "VISA resource name"=w3233) -> ("error out"=w3229:errorcluster, "read buffer"=w3249:string, "VISA resource name out"=w3230:refnum<visa-resource-name>)  [unwired: 3 in]
                    n1557 = Decimal String To Number(string=w3249, offset=0) -> (number=w3228:i32)  [unwired: 1 in, 1 out]
                    n1558 = property on="Z Step PV" class="DigNum (strict)"("Val(Sgnl)"=w3228) -> ()  [unwired: 2 in, 2 out]
                    n1559 = In Range and Coerce(upper limit=w3246, x=w3228, lower limit=w3247) -> (In Range?=w3239:bool)  [unwired: 1 out]
                    n1560 = To Double Precision Float(number=w3228) -> (double precision float=w3243:dbl)
                    n1561 = property on="Z in Range" class="Bool (strict)"("Val(Sgnl)"=w3239) -> ()  [unwired: 2 in, 2 out]
                    n1562 = Divide(x=w3243, y=w3245) -> (x/y=w3244:dbl)
                    n1563 = property on="Z mm/rev" class="DigNum (strict)"() -> ("Value"=w3237:dbl)  [unwired: 2 in, 2 out]
                    n1564 = Multiply(x=w3244, y=w3237) -> (x*y=w3231:dbl)
                    n1565 = Add(x=w3231, y=w3236) -> (x+y=w3235:dbl)
                    n1566 = property on="Z Position mm PV" class="DigNum (strict)"("Val(Sgnl)"=w3235) -> ()  [unwired: 2 in, 2 out]
                  }
                  frame #1 {
                    n1567 = call "mDrive Send Command.vi"("error in (no error)"=w3255, "Extra"="MV", "Command"=T10."Print Parameter", "VISA resource name"=w3256) -> ("error out"=w3258:errorcluster, "read buffer"=w3261:string, "VISA resource name out"=w3259:refnum<visa-resource-name>)  [unwired: 3 in]
                    n1568 = Decimal String To Number(string=w3261, offset=0 ("offset (0)")) -> (number=w3251:i32)  [unwired: 1 in, 1 out]
                    n1569 = Not Equal?(x=w3261, y="") -> (x != y?=w3254:bool)
                    n1570 = property on="Z Ready" class="Bool (strict)"("Val(Sgnl)"=w3254) -> ()  [unwired: 2 in, 2 out]
                    n1571 = Number To Boolean Array(number=w3251) -> (Boolean array=w3253:bool[])
                    n1572 = Index Array(array=w3253, index=0) -> (element=w3250:bool)
                    n1573 = property on="Z in Motion" class="Bool (strict)"("Val(Sgnl)"=w3250) -> ()  [unwired: 2 in, 2 out]
                  }
                  frame #2 {
                    n1574 = Wait (ms)(milliseconds to wait=u32 10) -> ()  [unwired: 1 out]
                  }
                  frame #3 {
                    n1575 = case shown="False" w3271 {
                      tunnel: w3272 -> [w3276 w3280]
                      tunnel: [w3277 w3280] -> w3270
                      tunnel: [w3278 w3279] -> w3269
                      tunnel: w3273 -> [w3275 w3279]
                      frame #0 {
                        n1576 = call "mDrive Send Command.vi"("error in (no error)"=w3275, "Command"=T10."Stop", "VISA resource name"=w3276) -> ("error out"=w3278:errorcluster, "VISA resource name out"=w3277:refnum<visa-resource-name>)  [unwired: 4 in, 1 out]
                      }
                      frame #1 {
                      }
                    }
                  }
                }
                n1577 = flat-sequence {
                  tunnel: [w3184] -> w3103
                  tunnel: [w3186] -> w3102
                  tunnel: [w3185] -> w3101
                  tunnel: w3081 -> [w3177]
                  tunnel: w3080 -> [w3176]
                  tunnel: [w3206] -> w3100
                  tunnel: [w3205] -> w3099
                  tunnel: [w3204] -> w3098
                  tunnel: w3103 -> [w3204]
                  tunnel: w3102 -> [w3203]
                  tunnel: w3101 -> [w3202]
                  tunnel: w3100 -> [w3215]
                  tunnel: [w3215] -> w3095
                  tunnel: w3099 -> [w3214]
                  tunnel: [w3214] -> w3096
                  tunnel: w3098 -> [w3213]
                  tunnel: [w3213] -> w3097
                  tunnel: w3097 -> [w3218]
                  tunnel: w3096 -> [w3220]
                  tunnel: w3095 -> [w3219]
                  tunnel: [w3216] -> w3071
                  tunnel: [w3217] -> w3070
                  frame #0 {
                    n1578 = property on="Y Step SP" class="DigNum (strict)"() -> ("Maximum"=w3179:dbl)  [unwired: 2 in, 2 out]
                    n1579 = property on="Y Step SP" class="DigNum (strict)"() -> ("Minimum"=w3178:dbl)  [unwired: 2 in, 2 out]
                    n1580 = property on="Y steps/rev" class="DigNum (strict)"() -> ("Value"=w3180:u32)  [unwired: 2 in, 2 out]
                    n1581 = property on="Y offset mm" class="DigNum (strict)"() -> ("Value"=w3182:dbl)  [unwired: 2 in, 2 out]
                    n1582 = To Long Integer(number=w3179) -> (32bit integer=w3193:i32)
                    n1583 = To Long Integer(number=w3178) -> (32bit integer=w3194:i32)
                    n1584 = To Double Precision Float(number=w3180) -> (double precision float=w3192:dbl)
                    n1585 = call "mDrive Send Command.vi"("error in (no error)"=w3176, "Extra"="P", "Command"=T10."Print Parameter", "VISA resource name"=w3177) -> ("error out"=w3185:errorcluster, "read buffer"=w3196:string, "VISA resource name out"=w3186:refnum<visa-resource-name>)  [unwired: 3 in]
                    n1586 = Decimal String To Number(string=w3196, offset=0) -> (number=w3175:i32)  [unwired: 1 in, 1 out]
                    n1587 = property on="Y Step PV" class="DigNum (strict)"("Val(Sgnl)"=w3175) -> ()  [unwired: 2 in, 2 out]
                    n1588 = In Range and Coerce(upper limit=w3193, x=w3175, lower limit=w3194) -> (In Range?=w3184:bool)  [unwired: 1 out]
                    n1589 = To Double Precision Float(number=w3175) -> (double precision float=w3189:dbl)
                    n1590 = property on="Y in Range" class="Bool (strict)"("Val(Sgnl)"=w3184) -> ()  [unwired: 2 in, 2 out]
                    n1591 = Divide(x=w3189, y=w3192) -> (x/y=w3191:dbl)
                    n1592 = property on="Y mm/rev" class="DigNum (strict)"() -> ("Value"=w3181:dbl)  [unwired: 2 in, 2 out]
                    n1593 = Multiply(x=w3191, y=w3181) -> (x*y=w3190:dbl)
                    n1594 = Add(x=w3190, y=w3182) -> (x+y=w3183:dbl)
                    n1595 = property on="Y Position mm PV" class="DigNum (strict)"("Val(Sgnl)"=w3183) -> ()  [unwired: 2 in, 2 out]
                  }
                  frame #1 {
                    n1596 = call "mDrive Send Command.vi"("error in (no error)"=w3202, "Extra"="MV", "Command"=T10."Print Parameter", "VISA resource name"=w3203) -> ("error out"=w3205:errorcluster, "read buffer"=w3208:string, "VISA resource name out"=w3206:refnum<visa-resource-name>)  [unwired: 3 in]
                    n1597 = Decimal String To Number(string=w3208, offset=0 ("offset (0)")) -> (number=w3198:i32)  [unwired: 1 in, 1 out]
                    n1598 = Not Equal?(x=w3208, y="") -> (x != y?=w3201:bool)
                    n1599 = property on="Y Ready" class="Bool (strict)"("Val(Sgnl)"=w3201) -> ()  [unwired: 2 in, 2 out]
                    n1600 = Number To Boolean Array(number=w3198) -> (Boolean array=w3200:bool[])
                    n1601 = Index Array(array=w3200, index=0) -> (element=w3197:bool)
                    n1602 = property on="Y in Motion" class="Bool (strict)"("Val(Sgnl)"=w3197) -> ()  [unwired: 2 in, 2 out]
                  }
                  frame #2 {
                    n1603 = Wait (ms)(milliseconds to wait=u32 10) -> ()  [unwired: 1 out]
                  }
                  frame #3 {
                    n1604 = case shown="False" w3218 {
                      tunnel: w3219 -> [w3223 w3226]
                      tunnel: [w3224 w3226] -> w3216
                      tunnel: [w3225 w3227] -> w3217
                      tunnel: w3220 -> [w3222 w3227]
                      frame #0 {
                        n1605 = call "mDrive Send Command.vi"("error in (no error)"=w3222, "Command"=T10."Stop", "VISA resource name"=w3223) -> ("error out"=w3225:errorcluster, "VISA resource name out"=w3224:refnum<visa-resource-name>)  [unwired: 4 in, 1 out]
                      }
                      frame #1 {
                      }
                    }
                  }
                }
                n1606 = flat-sequence {
                  tunnel: [w3131] -> w3094
                  tunnel: [w3133] -> w3093
                  tunnel: [w3132] -> w3092
                  tunnel: w3079 -> [w3124]
                  tunnel: w3078 -> [w3123]
                  tunnel: [w3153] -> w3091
                  tunnel: [w3152] -> w3090
                  tunnel: [w3151] -> w3089
                  tunnel: w3094 -> [w3151]
                  tunnel: w3093 -> [w3150]
                  tunnel: w3092 -> [w3149]
                  tunnel: w3091 -> [w3162]
                  tunnel: [w3162] -> w3086
                  tunnel: w3090 -> [w3161]
                  tunnel: [w3161] -> w3087
                  tunnel: w3089 -> [w3160]
                  tunnel: [w3160] -> w3088
                  tunnel: w3088 -> [w3165]
                  tunnel: w3087 -> [w3167]
                  tunnel: w3086 -> [w3166]
                  tunnel: [w3164] -> w3069
                  tunnel: [w3163] -> w3068
                  frame #0 {
                    n1607 = property on="R Step SP" class="DigNum (strict)"() -> ("Maximum"=w3126:dbl)  [unwired: 2 in, 2 out]
                    n1608 = property on="R Step SP" class="DigNum (strict)"() -> ("Minimum"=w3127:dbl)  [unwired: 2 in, 2 out]
                    n1609 = property on="R steps/rev" class="DigNum (strict)"() -> ("Value"=w3125:u32)  [unwired: 2 in, 2 out]
                    n1610 = property on="R offset deg" class="DigNum (strict)"() -> ("Value"=w3129:dbl)  [unwired: 2 in, 2 out]
                    n1611 = To Long Integer(number=w3126) -> (32bit integer=w3140:i32)
                    n1612 = To Long Integer(number=w3127) -> (32bit integer=w3141:i32)
                    n1613 = To Double Precision Float(number=w3125) -> (double precision float=w3139:dbl)
                    n1614 = call "mDrive Send Command.vi"("error in (no error)"=w3123, "Extra"="P", "Command"=T10."Print Parameter", "VISA resource name"=w3124) -> ("error out"=w3132:errorcluster, "read buffer"=w3143:string, "VISA resource name out"=w3133:refnum<visa-resource-name>)  [unwired: 3 in]
                    n1615 = Decimal String To Number(string=w3143, offset=0) -> (number=w3122:i32)  [unwired: 1 in, 1 out]
                    n1616 = property on="R Step PV" class="DigNum (strict)"("Val(Sgnl)"=w3122) -> ()  [unwired: 2 in, 2 out]
                    n1617 = In Range and Coerce(upper limit=w3140, x=w3122, lower limit=w3141) -> (In Range?=w3131:bool)  [unwired: 1 out]
                    n1618 = To Double Precision Float(number=w3122) -> (double precision float=w3136:dbl)
                    n1619 = property on="R in Range" class="Bool (strict)"("Val(Sgnl)"=w3131) -> ()  [unwired: 2 in, 2 out]
                    n1620 = Divide(x=w3136, y=w3139) -> (x/y=w3138:dbl)
                    n1621 = property on="R deg/rev" class="DigNum (strict)"() -> ("Value"=w3128:dbl)  [unwired: 2 in, 2 out]
                    n1622 = Multiply(x=w3138, y=w3128) -> (x*y=w3137:dbl)
                    n1623 = Add(x=w3137, y=w3129) -> (x+y=w3130:dbl)
                    n1624 = property on="R Position deg PV" class="DigNum (strict)"("Val(Sgnl)"=w3130) -> ()  [unwired: 2 in, 2 out]
                  }
                  frame #1 {
                    n1625 = call "mDrive Send Command.vi"("error in (no error)"=w3149, "Extra"="MV", "Command"=T10."Print Parameter", "VISA resource name"=w3150) -> ("error out"=w3152:errorcluster, "read buffer"=w3155:string, "VISA resource name out"=w3153:refnum<visa-resource-name>)  [unwired: 3 in]
                    n1626 = Decimal String To Number(string=w3155, offset=0 ("offset (0)")) -> (number=w3145:i32)  [unwired: 1 in, 1 out]
                    n1627 = Not Equal?(x=w3155, y="") -> (x != y?=w3148:bool)
                    n1628 = property on="R Ready" class="Bool (strict)"("Val(Sgnl)"=w3148) -> ()  [unwired: 2 in, 2 out]
                    n1629 = Number To Boolean Array(number=w3145) -> (Boolean array=w3147:bool[])
                    n1630 = Index Array(array=w3147, index=0) -> (element=w3144:bool)
                    n1631 = property on="R in Motion" class="Bool (strict)"("Val(Sgnl)"=w3144) -> ()  [unwired: 2 in, 2 out]
                  }
                  frame #2 {
                    n1632 = Wait (ms)(milliseconds to wait=u32 10) -> ()  [unwired: 1 out]
                  }
                  frame #3 {
                    n1633 = case shown="False" w3165 {
                      tunnel: w3166 -> [w3170 w3174]
                      tunnel: [w3171 w3174] -> w3164
                      tunnel: [w3172 w3173] -> w3163
                      tunnel: w3167 -> [w3169 w3173]
                      frame #0 {
                        n1634 = call "mDrive Send Command.vi"("error in (no error)"=w3169, "Command"=T10."Stop", "VISA resource name"=w3170) -> ("error out"=w3172:errorcluster, "VISA resource name out"=w3171:refnum<visa-resource-name>)  [unwired: 4 in, 1 out]
                      }
                      frame #1 {
                      }
                    }
                  }
                }
                n1635 = property on="Y in Motion" class="Bool (strict)"() -> ("Value"=w3077:bool)  [unwired: 2 in, 2 out]
                n1636 = property on="Z in Motion" class="Bool (strict)"() -> ("Value"=w3067:bool)  [unwired: 2 in, 2 out]
                n1637 = property on="X  in Motion" class="Bool (strict)"() -> ("Value"=w3076:bool)  [unwired: 2 in, 2 out]
                n1638 = property on="R in Motion" class="Bool (strict)"() -> ("Value"=w3066:bool)  [unwired: 2 in, 2 out]
                n1639 = Compound Arithmetic op=OR(w3076, w3077, w3067, w3066) -> (w3065:bool)
                n1640 = Not(x=w3065) -> (.not. x?=w3064:bool)
              }
            }
            frame #4 {
              n1641 = Wait (ms)(milliseconds to wait=u32 300) -> ()  [unwired: 1 out]
            }
            frame #5 {
              w3343 = TRUE ("R in Motion")
              n1642 = property on="X Position mm PV" class="DigNum (strict)"() -> ("Value"=w3372:dbl)  [unwired: 2 in, 2 out]
              n1643 = property on="X Position SP mm" class="DigNum (strict)"() -> ("Value"=w3371:dbl)  [unwired: 2 in, 2 out]
              n1644 = property on="Z Position mm PV" class="DigNum (strict)"() -> ("Value"=w3368:dbl)  [unwired: 2 in, 2 out]
              n1645 = property on="Z Position SP mm" class="DigNum (strict)"() -> ("Value"=w3361:dbl)  [unwired: 2 in, 2 out]
              n1646 = property on="Y Position mm PV" class="DigNum (strict)"() -> ("Value"=w3366:dbl)  [unwired: 2 in, 2 out]
              n1647 = property on="Y Position SP mm" class="DigNum (strict)"() -> ("Value"=w3365:dbl)  [unwired: 2 in, 2 out]
              n1648 = property on="R Position SP deg" class="DigNum (strict)"() -> ("Value"=w3363:dbl)  [unwired: 2 in, 2 out]
              n1649 = property on="R Position deg PV" class="DigNum (strict)"() -> ("Value"=w3362:dbl)  [unwired: 2 in, 2 out]
              n1650 = Not Equal?(x=w3372, y=w3371) -> (x != y?=w3370:bool)
              n1651 = Not Equal?(x=w3368, y=w3361) -> (x != y?=w3369:bool)
              n1652 = Not Equal?(x=w3366, y=w3365) -> (x != y?=w3367:bool)
              n1653 = Not Equal?(x=w3363, y=w3362) -> (x != y?=w3364:bool)
              n1654 = local write "STATUS"("LOOP HOMING" ("STATUS")) -> ()
              n1655 = case shown="True" w3370 {
                tunnel: w3360 -> [w3584 w3588]
                tunnel: w3358 -> [w3583 w3587]
                tunnel: [w3584 w3586] -> w3345
                tunnel: [w3583 w3585] -> w3346
                frame #0 {
                }
                frame #1 {
                  n1656 = flat-sequence {
                    tunnel: w3587 -> [w3603]
                    tunnel: w3588 -> [w3616]
                    tunnel: [w3616] -> w3602
                    tunnel: [w3603] -> w3601
                    tunnel: [w3605] -> w3600
                    tunnel: [w3619] -> w3599
                    tunnel: [w3618] -> w3598
                    tunnel: [w3617] -> w3597
                    tunnel: w3600 -> [w3617]
                    tunnel: w3601 -> [w3618]
                    tunnel: w3602 -> [w3619]
                    tunnel: [w3635] -> w3596
                    tunnel: [w3634] -> w3595
                    tunnel: w3599 -> [w3633]
                    tunnel: w3598 -> [w3632]
                    tunnel: w3597 -> [w3631]
                    tunnel: [w3631] -> w3594
                    tunnel: w3596 -> [w3642]
                    tunnel: [w3642] -> w3593
                    tunnel: w3595 -> [w3641]
                    tunnel: [w3641] -> w3592
                    tunnel: [w3639] -> w3591
                    tunnel: w3594 -> [w3639]
                    tunnel: [w3647] -> w3590
                    tunnel: [w3646] -> w3589
                    tunnel: w3593 -> [w3645]
                    tunnel: w3592 -> [w3644]
                    tunnel: w3591 -> [w3643]
                    tunnel: [w3651] -> w3585
                    tunnel: [w3652] -> w3586
                    tunnel: w3590 -> [w3652]
                    tunnel: w3589 -> [w3651]
                    frame #0 {
                      n1657 = property on="X steps/rev" class="DigNum (strict)"() -> ("Value"=w3615:u32)  [unwired: 2 in, 2 out]
                      n1658 = To Double Precision Float(number=w3615) -> (double precision float=w3610:dbl)
                      n1659 = property on="X offset mm" class="DigNum (strict)"() -> ("Value"=w3614:dbl)  [unwired: 2 in, 2 out]
                      n1660 = property on="X Position SP mm" class="DigNum (strict)"() -> ("Value"=w3613:dbl)  [unwired: 2 in, 2 out]
                      n1661 = Subtract(x=w3613, y=w3614) -> (x-y=w3607:dbl)
                      n1662 = property on="X mm/rev" class="DigNum (strict)"() -> ("Value"=w3604:dbl)  [unwired: 2 in, 2 out]
                      n1663 = Divide(x=w3607, y=w3604) -> (x/y=w3606:dbl)
                      n1664 = property on="X Step SP" class="DigNum (strict)"() -> ("Maximum"=w3612:dbl)  [unwired: 2 in, 2 out]
                      n1665 = property on="X Step SP" class="DigNum (strict)"() -> ("Minimum"=w3611:dbl)  [unwired: 2 in, 2 out]
                      n1666 = Multiply(x=w3606, y=w3610) -> (x*y=w3608:dbl)
                      n1667 = In Range and Coerce(upper limit=w3612, x=w3608, lower limit=w3611) -> (coerced(x)=w3609:dbl)  [unwired: 1 out]
                      n1668 = To Long Integer(number=w3609) -> (32bit integer=w3605:i32)
                      n1669 = property on="X Step SP" class="DigNum (strict)"("Val(Sgnl)"=w3605) -> ()  [unwired: 2 in, 2 out]
                    }
                    frame #1 {
                      n1670 = property on="X Step SP" class="DigNum (strict)"() -> ("Value"=w3628:i32)  [unwired: 2 in, 2 out]
                      n1671 = property on="X Step PV" class="DigNum (strict)"() -> ("Value"=w3627:i32)  [unwired: 2 in, 2 out]
                      n1672 = property on="X Backlash" class="DigNum (strict)"() -> ("Value"=w3620:i32)  [unwired: 2 in, 2 out]
                      n1673 = Subtract(x=w3628, y=w3627) -> (x-y=w3626:i32)
                      n1674 = Sign(1:w3620) -> (0:w3624:i32)
                      n1675 = Sign(1:w3626) -> (0:w3625:i32)
                      n1676 = Multiply(x=w3625, y=w3624) -> (x*y=w3623:i32)
                      n1677 = Equal?(x=w3623, y=1) -> (x = y?=w3621:bool)
                      n1678 = case shown="True" w3621 {
                        frame #0 {
                          n1679 = property on="X Backlash corr" class="Bool (strict)"("Val(Sgnl)"=FALSE ("Value (Signaling)")) -> ()  [unwired: 2 in, 2 out]
                        }
                        frame #1 {
                          n1680 = property on="X Backlash corr" class="Bool (strict)"("Val(Sgnl)"=TRUE ("Value (Signaling)")) -> ()  [unwired: 2 in, 2 out]
                        }
                      }
                    }
                    frame #2 {
                      # "Velocity Setting"
                      n1681 = property on="X Velocity SP step/sec" class="DigNum (strict)"() -> ("Value"=w3636:i32)  [unwired: 2 in, 2 out]
                      n1682 = Number To Decimal String(number=w3636) -> (decimal integer string=w3637:string)  [unwired: 1 in]
                      n1683 = call "mDrive Send Command.vi"("error in (no error)"=w3632, "Extra"=w3637, "Command"=T10."Max Velocity", "VISA resource name"=w3633) -> ("error out"=w3634:errorcluster, "VISA resource name out"=w3635:refnum<visa-resource-name>)  [unwired: 3 in, 1 out]
                    }
                    frame #3 {
                      n1684 = Wait (ms)(milliseconds to wait=u32 50) -> ()  [unwired: 1 out]
                    }
                    frame #4 {
                      # "Move to Abs Position"
                      n1685 = Number To Decimal String(number=w3643) -> (decimal integer string=w3649:string)  [unwired: 1 in]
                      n1686 = call "mDrive Send Command.vi"("error in (no error)"=w3644, "Extra"=w3649, "Command"=T10."Move to Absolute Position", "VISA resource name"=w3645) -> ("error out"=w3646:errorcluster, "VISA resource name out"=w3647:refnum<visa-resource-name>)  [unwired: 3 in, 1 out]
                    }
                    frame #5 {
                      n1687 = Wait (ms)(milliseconds to wait=u32 50) -> ()  [unwired: 1 out]
                    }
                  }
                }
              }
              n1688 = case shown="True" w3369 {
                tunnel: w3357 -> [w3513 w3518]
                tunnel: w3359 -> [w3514 w3517]
                tunnel: [w3514 w3516] -> w3347
                tunnel: [w3513 w3515] -> w3348
                frame #0 {
                }
                frame #1 {
                  n1689 = flat-sequence {
                    tunnel: [w3546] -> w3532
                    tunnel: [w3545] -> w3531
                    tunnel: [w3534] -> w3530
                    tunnel: w3518 -> [w3546]
                    tunnel: w3517 -> [w3545]
                    tunnel: [w3549] -> w3529
                    tunnel: [w3548] -> w3528
                    tunnel: [w3547] -> w3527
                    tunnel: w3530 -> [w3547]
                    tunnel: w3531 -> [w3548]
                    tunnel: w3532 -> [w3549]
                    tunnel: [w3565] -> w3526
                    tunnel: [w3564] -> w3525
                    tunnel: w3529 -> [w3563]
                    tunnel: w3528 -> [w3562]
                    tunnel: [w3561] -> w3524
                    tunnel: w3527 -> [w3561]
                    tunnel: w3526 -> [w3572]
                    tunnel: [w3572] -> w3523
                    tunnel: w3525 -> [w3571]
                    tunnel: [w3571] -> w3522
                    tunnel: w3524 -> [w3570]
                    tunnel: [w3570] -> w3521
                    tunnel: [w3577] -> w3520
                    tunnel: [w3576] -> w3519
                    tunnel: w3523 -> [w3575]
                    tunnel: w3522 -> [w3574]
                    tunnel: w3521 -> [w3573]
                    tunnel: [w3581] -> w3515
                    tunnel: [w3582] -> w3516
                    tunnel: w3520 -> [w3582]
                    tunnel: w3519 -> [w3581]
                    frame #0 {
                      n1690 = property on="Z steps/rev" class="DigNum (strict)"() -> ("Value"=w3533:u32)  [unwired: 2 in, 2 out]
                      n1691 = To Double Precision Float(number=w3533) -> (double precision float=w3539:dbl)
                      n1692 = property on="Z offset mm" class="DigNum (strict)"() -> ("Value"=w3541:dbl)  [unwired: 2 in, 2 out]
                      n1693 = property on="Z Position SP mm" class="DigNum (strict)"() -> ("Value"=w3540:dbl)  [unwired: 2 in, 2 out]
                      n1694 = Subtract(x=w3540, y=w3541) -> (x-y=w3536:dbl)
                      n1695 = property on="Z mm/rev" class="DigNum (strict)"() -> ("Value"=w3542:dbl)  [unwired: 2 in, 2 out]
                      n1696 = Divide(x=w3536, y=w3542) -> (x/y=w3535:dbl)
                      n1697 = property on="Z Step SP" class="DigNum (strict)"() -> ("Maximum"=w3544:dbl)  [unwired: 2 in, 2 out]
                      n1698 = property on="Z Step SP" class="DigNum (strict)"() -> ("Minimum"=w3543:dbl)  [unwired: 2 in, 2 out]
                      n1699 = Multiply(x=w3535, y=w3539) -> (x*y=w3537:dbl)
                      n1700 = In Range and Coerce(upper limit=w3544, x=w3537, lower limit=w3543) -> (coerced(x)=w3538:dbl)  [unwired: 1 out]
                      n1701 = To Long Integer(number=w3538) -> (32bit integer=w3534:i32)
                      n1702 = property on="Z Step SP" class="DigNum (strict)"("Val(Sgnl)"=w3534) -> ()  [unwired: 2 in, 2 out]
                    }
                    frame #1 {
                      n1703 = property on="Z Step SP" class="DigNum (strict)"() -> ("Value"=w3558:i32)  [unwired: 2 in, 2 out]
                      n1704 = property on="Z Backlash" class="DigNum (strict)"() -> ("Value"=w3550:i32)  [unwired: 2 in, 2 out]
                      n1705 = property on="Z Step PV" class="DigNum (strict)"() -> ("Value"=w3557:i32)  [unwired: 2 in, 2 out]
                      n1706 = Subtract(x=w3558, y=w3557) -> (x-y=w3556:i32)
                      n1707 = Sign(1:w3550) -> (0:w3554:i32)
                      n1708 = Sign(1:w3556) -> (0:w3555:i32)
                      n1709 = Multiply(x=w3555, y=w3554) -> (x*y=w3553:i32)
                      n1710 = Equal?(x=w3553, y=1) -> (x = y?=w3551:bool)
                      n1711 = case shown="False" w3551 {
                        frame #0 {
                          n1712 = property on="Z Backlash corr" class="Bool (strict)"("Val(Sgnl)"=FALSE ("Value (Signaling)")) -> ()  [unwired: 2 in, 2 out]
                        }
                        frame #1 {
                          n1713 = property on="Z Backlash corr" class="Bool (strict)"("Val(Sgnl)"=TRUE ("Value (Signaling)")) -> ()  [unwired: 2 in, 2 out]
                        }
                      }
                    }
                    frame #2 {
                      # "Velocity Setting"
                      n1714 = property on="Z Velocity SP step/sec" class="DigNum (strict)"() -> ("Value"=w3566:i32)  [unwired: 2 in, 2 out]
                      n1715 = Number To Decimal String(number=w3566) -> (decimal integer string=w3567:string)  [unwired: 1 in]
                      n1716 = call "mDrive Send Command.vi"("error in (no error)"=w3563, "Extra"=w3567, "Command"=T10."Max Velocity", "VISA resource name"=w3562) -> ("error out"=w3564:errorcluster, "VISA resource name out"=w3565:refnum<visa-resource-name>)  [unwired: 3 in, 1 out]
                    }
                    frame #3 {
                      n1717 = Wait (ms)(milliseconds to wait=u32 50) -> ()  [unwired: 1 out]
                    }
                    frame #4 {
                      # "Move to Abs Position"
                      n1718 = Number To Decimal String(number=w3573) -> (decimal integer string=w3579:string)  [unwired: 1 in]
                      n1719 = call "mDrive Send Command.vi"("error in (no error)"=w3574, "Extra"=w3579, "Command"=T10."Move to Absolute Position", "VISA resource name"=w3575) -> ("error out"=w3576:errorcluster, "VISA resource name out"=w3577:refnum<visa-resource-name>)  [unwired: 3 in, 1 out]
                    }
                    frame #5 {
                      n1720 = Wait (ms)(milliseconds to wait=u32 50) -> ()  [unwired: 1 out]
                    }
                  }
                }
              }
              n1721 = case shown="True" w3367 {
                tunnel: w3355 -> [w3443 w3448]
                tunnel: w3356 -> [w3444 w3447]
                tunnel: [w3444 w3446] -> w3349
                tunnel: [w3443 w3445] -> w3350
                frame #0 {
                }
                frame #1 {
                  n1722 = flat-sequence {
                    tunnel: [w3476] -> w3462
                    tunnel: [w3475] -> w3461
                    tunnel: [w3463] -> w3460
                    tunnel: w3447 -> [w3475]
                    tunnel: w3448 -> [w3476]
                    tunnel: [w3479] -> w3459
                    tunnel: [w3478] -> w3458
                    tunnel: [w3477] -> w3457
                    tunnel: w3460 -> [w3477]
                    tunnel: w3461 -> [w3478]
                    tunnel: w3462 -> [w3479]
                    tunnel: [w3495] -> w3456
                    tunnel: [w3494] -> w3455
                    tunnel: w3459 -> [w3493]
                    tunnel: w3458 -> [w3492]
                    tunnel: [w3491] -> w3454
                    tunnel: w3457 -> [w3491]
                    tunnel: w3456 -> [w3502]
                    tunnel: [w3502] -> w3453
                    tunnel: w3455 -> [w3501]
                    tunnel: [w3501] -> w3452
                    tunnel: [w3499] -> w3451
                    tunnel: w3454 -> [w3499]
                    tunnel: [w3507] -> w3450
                    tunnel: [w3506] -> w3449
                    tunnel: w3453 -> [w3505]
                    tunnel: w3452 -> [w3504]
                    tunnel: w3451 -> [w3503]
                    tunnel: [w3510] -> w3445
                    tunnel: [w3512] -> w3446
                    tunnel: w3450 -> [w3512]
                    tunnel: w3449 -> [w3510]
                    frame #0 {
                      n1723 = property on="Y steps/rev" class="DigNum (strict)"() -> ("Value"=w3472:u32)  [unwired: 2 in, 2 out]
                      n1724 = To Double Precision Float(number=w3472) -> (double precision float=w3468:dbl)
                      n1725 = property on="Y offset mm" class="DigNum (strict)"() -> ("Value"=w3470:dbl)  [unwired: 2 in, 2 out]
                      n1726 = property on="Y Position SP mm" class="DigNum (strict)"() -> ("Value"=w3469:dbl)  [unwired: 2 in, 2 out]
                      n1727 = Subtract(x=w3469, y=w3470) -> (x-y=w3465:dbl)
                      n1728 = property on="Y mm/rev" class="DigNum (strict)"() -> ("Value"=w3471:dbl)  [unwired: 2 in, 2 out]
                      n1729 = Divide(x=w3465, y=w3471) -> (x/y=w3464:dbl)
                      n1730 = property on="Y Step SP" class="DigNum (strict)"() -> ("Maximum"=w3473:dbl)  [unwired: 2 in, 2 out]
                      n1731 = property on="Y Step SP" class="DigNum (strict)"() -> ("Minimum"=w3474:dbl)  [unwired: 2 in, 2 out]
                      n1732 = Multiply(x=w3464, y=w3468) -> (x*y=w3466:dbl)
                      n1733 = In Range and Coerce(upper limit=w3473, x=w3466, lower limit=w3474) -> (coerced(x)=w3467:dbl)  [unwired: 1 out]
                      n1734 = To Long Integer(number=w3467) -> (32bit integer=w3463:i32)
                      n1735 = property on="Y Step SP" class="DigNum (strict)"("Val(Sgnl)"=w3463) -> ()  [unwired: 2 in, 2 out]
                    }
                    frame #1 {
                      n1736 = property on="Y Step SP" class="DigNum (strict)"() -> ("Value"=w3488:i32)  [unwired: 2 in, 2 out]
                      n1737 = property on="Y Backlash" class="DigNum (strict)"() -> ("Value"=w3480:i32)  [unwired: 2 in, 2 out]
                      n1738 = property on="Y Step PV" class="DigNum (strict)"() -> ("Value"=w3487:i32)  [unwired: 2 in, 2 out]
                      n1739 = Subtract(x=w3488, y=w3487) -> (x-y=w3486:i32)
                      n1740 = Sign(1:w3480) -> (0:w3484:i32)
                      n1741 = Sign(1:w3486) -> (0:w3485:i32)
                      n1742 = Multiply(x=w3485, y=w3484) -> (x*y=w3483:i32)
                      n1743 = Equal?(x=w3483, y=1) -> (x = y?=w3481:bool)
                      n1744 = case shown="True" w3481 {
                        frame #0 {
                          n1745 = property on="Y Backlash corr" class="Bool (strict)"("Val(Sgnl)"=FALSE ("Value (Signaling)")) -> ()  [unwired: 2 in, 2 out]
                        }
                        frame #1 {
                          n1746 = property on="Y Backlash corr" class="Bool (strict)"("Val(Sgnl)"=TRUE ("Value (Signaling)")) -> ()  [unwired: 2 in, 2 out]
                        }
                      }
                    }
                    frame #2 {
                      # "Velocity Setting"
                      n1747 = property on="Y Velocity SP step/sec" class="DigNum (strict)"() -> ("Value"=w3496:i32)  [unwired: 2 in, 2 out]
                      n1748 = Number To Decimal String(number=w3496) -> (decimal integer string=w3497:string)  [unwired: 1 in]
                      n1749 = call "mDrive Send Command.vi"("error in (no error)"=w3493, "Extra"=w3497, "Command"=T10."Max Velocity", "VISA resource name"=w3492) -> ("error out"=w3494:errorcluster, "VISA resource name out"=w3495:refnum<visa-resource-name>)  [unwired: 3 in, 1 out]
                    }
                    frame #3 {
                      n1750 = Wait (ms)(milliseconds to wait=u32 50) -> ()  [unwired: 1 out]
                    }
                    frame #4 {
                      # "Move to Abs Position"
                      n1751 = Number To Decimal String(number=w3503) -> (decimal integer string=w3509:string)  [unwired: 1 in]
                      n1752 = call "mDrive Send Command.vi"("error in (no error)"=w3504, "Extra"=w3509, "Command"=T10."Move to Absolute Position", "VISA resource name"=w3505) -> ("error out"=w3506:errorcluster, "VISA resource name out"=w3507:refnum<visa-resource-name>)  [unwired: 3 in, 1 out]
                    }
                    frame #5 {
                      n1753 = Wait (ms)(milliseconds to wait=u32 25) -> ()  [unwired: 1 out]
                    }
                  }
                }
              }
              n1754 = case shown="True" w3364 {
                tunnel: w3353 -> [w3373 w3378]
                tunnel: w3354 -> [w3374 w3377]
                tunnel: [w3374 w3376] -> w3352
                tunnel: [w3373 w3375] -> w3351
                frame #0 {
                }
                frame #1 {
                  n1755 = flat-sequence {
                    tunnel: w3377 -> [w3405]
                    tunnel: w3378 -> [w3406]
                    tunnel: [w3406] -> w3392
                    tunnel: [w3405] -> w3391
                    tunnel: [w3393] -> w3390
                    tunnel: [w3409] -> w3389
                    tunnel: [w3408] -> w3388
                    tunnel: [w3407] -> w3387
                    tunnel: w3390 -> [w3407]
                    tunnel: w3391 -> [w3408]
                    tunnel: w3392 -> [w3409]
                    tunnel: [w3425] -> w3386
                    tunnel: [w3424] -> w3385
                    tunnel: w3389 -> [w3423]
                    tunnel: w3388 -> [w3422]
                    tunnel: [w3421] -> w3384
                    tunnel: w3387 -> [w3421]
                    tunnel: w3386 -> [w3432]
                    tunnel: [w3432] -> w3383
                    tunnel: w3385 -> [w3431]
                    tunnel: [w3431] -> w3382
                    tunnel: w3384 -> [w3430]
                    tunnel: [w3430] -> w3381
                    tunnel: [w3437] -> w3380
                    tunnel: [w3436] -> w3379
                    tunnel: w3383 -> [w3435]
                    tunnel: w3382 -> [w3434]
                    tunnel: w3381 -> [w3433]
                    tunnel: [w3442] -> w3376
                    tunnel: w3380 -> [w3442]
                    tunnel: w3379 -> [w3441]
                    tunnel: [w3441] -> w3375
                    frame #0 {
                      n1756 = property on="R steps/rev" class="DigNum (strict)"() -> ("Value"=w3401:u32)  [unwired: 2 in, 2 out]
                      n1757 = To Double Precision Float(number=w3401) -> (double precision float=w3398:dbl)
                      n1758 = property on="R offset deg" class="DigNum (strict)"() -> ("Value"=w3402:dbl)  [unwired: 2 in, 2 out]
                      n1759 = property on="R Position SP deg" class="DigNum (strict)"() -> ("Value"=w3403:dbl)  [unwired: 2 in, 2 out]
                      n1760 = Subtract(x=w3403, y=w3402) -> (x-y=w3395:dbl)
                      n1761 = property on="R deg/rev" class="DigNum (strict)"() -> ("Value"=w3404:dbl)  [unwired: 2 in, 2 out]
                      n1762 = Divide(x=w3395, y=w3404) -> (x/y=w3394:dbl)
                      n1763 = property on="R Step SP" class="DigNum (strict)"() -> ("Maximum"=w3399:dbl)  [unwired: 2 in, 2 out]
                      n1764 = Multiply(x=w3394, y=w3398) -> (x*y=w3396:dbl)
                      n1765 = property on="R Step SP" class="DigNum (strict)"() -> ("Minimum"=w3400:dbl)  [unwired: 2 in, 2 out]
                      n1766 = In Range and Coerce(upper limit=w3399, x=w3396, lower limit=w3400) -> (coerced(x)=w3397:dbl)  [unwired: 1 out]
                      n1767 = To Long Integer(number=w3397) -> (32bit integer=w3393:i32)
                      n1768 = property on="R Step SP" class="DigNum (strict)"("Val(Sgnl)"=w3393) -> ()  [unwired: 2 in, 2 out]
                    }
                    frame #1 {
                      n1769 = property on="R Step SP" class="DigNum (strict)"() -> ("Value"=w3418:i32)  [unwired: 2 in, 2 out]
                      n1770 = property on="R Step PV" class="DigNum (strict)"() -> ("Value"=w3417:i32)  [unwired: 2 in, 2 out]
                      n1771 = property on="R Backlash" class="DigNum (strict)"() -> ("Value"=w3410:i32)  [unwired: 2 in, 2 out]
                      n1772 = Subtract(x=w3418, y=w3417) -> (x-y=w3416:i32)
                      n1773 = Sign(1:w3410) -> (0:w3414:i32)
                      n1774 = Sign(1:w3416) -> (0:w3415:i32)
                      n1775 = Multiply(x=w3415, y=w3414) -> (x*y=w3413:i32)
                      n1776 = Equal?(x=w3413, y=1) -> (x = y?=w3411:bool)
                      n1777 = case shown="True" w3411 {
                        frame #0 {
                          n1778 = property on="R Backlash corr" class="Bool (strict)"("Val(Sgnl)"=FALSE ("Value (Signaling)")) -> ()  [unwired: 2 in, 2 out]
                        }
                        frame #1 {
                          n1779 = property on="R Backlash corr" class="Bool (strict)"("Val(Sgnl)"=TRUE ("Value (Signaling)")) -> ()  [unwired: 2 in, 2 out]
                        }
                      }
                    }
                    frame #2 {
                      # "Velocity Setting"
                      n1780 = property on="R Velocity SP step/sec" class="DigNum (strict)"() -> ("Value"=w3426:i32)  [unwired: 2 in, 2 out]
                      n1781 = Number To Decimal String(number=w3426) -> (decimal integer string=w3427:string)  [unwired: 1 in]
                      n1782 = call "mDrive Send Command.vi"("error in (no error)"=w3423, "Extra"=w3427, "Command"=T10."Max Velocity", "VISA resource name"=w3422) -> ("error out"=w3424:errorcluster, "VISA resource name out"=w3425:refnum<visa-resource-name>)  [unwired: 3 in, 1 out]
                    }
                    frame #3 {
                      n1783 = Wait (ms)(milliseconds to wait=u32 50) -> ()  [unwired: 1 out]
                    }
                    frame #4 {
                      # "Move to Abs Position"
                      n1784 = Number To Decimal String(number=w3433) -> (decimal integer string=w3439:string)  [unwired: 1 in]
                      n1785 = call "mDrive Send Command.vi"("error in (no error)"=w3434, "Extra"=w3439, "Command"=T10."Move to Absolute Position", "VISA resource name"=w3435) -> ("error out"=w3436:errorcluster, "VISA resource name out"=w3437:refnum<visa-resource-name>)  [unwired: 3 in, 1 out]
                    }
                    frame #5 {
                      n1786 = Wait (ms)(milliseconds to wait=u32 25) -> ()  [unwired: 1 out]
                    }
                  }
                }
              }
              n1787 = property on="Y in Motion" class="Bool (strict)"("Value"=w3343) -> ()  [unwired: 2 in, 2 out]
              n1788 = property on="R in Motion" class="Bool (strict)"("Value"=w3343) -> ()  [unwired: 2 in, 2 out]
              n1789 = property on="X  in Motion" class="Bool (strict)"("Value"=w3343) -> ()  [unwired: 2 in, 2 out]
              n1790 = property on="Z in Motion" class="Bool (strict)"("Value"=w3343) -> ()  [unwired: 2 in, 2 out]
            }
            frame #6 {
              n1791 = while {
                tunnel: [w3690] -> w3666
                tunnel: [w3689] -> w3665
                tunnel: [w3688] -> w3668
                tunnel: [w3687] -> w3667
                tunnel: [w3686] -> w3664
                tunnel: [w3685] -> w3663
                tunnel: [w3684] -> w3662
                tunnel: [w3683] -> w3661
                tunnel: w3660 -> [w3672]
                tunnel: w3659 -> [w3671]
                tunnel: w3658 -> [w3674]
                tunnel: w3657 -> [w3673]
                tunnel: w3656 -> [w3679]
                tunnel: w3655 -> [w3678]
                tunnel: w3654 -> [w3677]
                tunnel: w3653 -> [w3676]
                stop <- w3675 stop-if-true
                n1792 = flat-sequence {
                  tunnel: [w4136] -> w3746
                  tunnel: [w4135] -> w3745
                  tunnel: [w4134] -> w3744
                  tunnel: w3672 -> [w4132]
                  tunnel: w3671 -> [w4131]
                  tunnel: [w4158] -> w3743
                  tunnel: [w4157] -> w3742
                  tunnel: [w4155] -> w3741
                  tunnel: [w4156] -> w3740
                  tunnel: w3746 -> [w4155]
                  tunnel: w3745 -> [w4154]
                  tunnel: w3744 -> [w4153]
                  tunnel: w3743 -> [w4172]
                  tunnel: [w4172] -> w3736
                  tunnel: w3742 -> [w4171]
                  tunnel: [w4171] -> w3737
                  tunnel: w3741 -> [w4170]
                  tunnel: [w4170] -> w3738
                  tunnel: w3740 -> [w4169]
                  tunnel: [w4169] -> w3739
                  tunnel: [w4176] -> w3735
                  tunnel: [w4177] -> w3734
                  tunnel: [w4173] -> w3733
                  tunnel: w3739 -> [w4173]
                  tunnel: w3738 -> [w4174]
                  tunnel: w3737 -> [w4178]
                  tunnel: w3736 -> [w4175]
                  tunnel: w3735 -> [w4188]
                  tunnel: w3734 -> [w4189]
                  tunnel: w3733 -> [w4191]
                  tunnel: [w4187] -> w3689
                  tunnel: [w4186] -> w3690
                  frame #0 {
                    n1793 = property on="Z Step SP" class="DigNum (strict)"() -> ("Maximum"=w4148:dbl)  [unwired: 2 in, 2 out]
                    n1794 = property on="Z Step SP" class="DigNum (strict)"() -> ("Minimum"=w4150:dbl)  [unwired: 2 in, 2 out]
                    n1795 = property on="Z steps/rev" class="DigNum (strict)"() -> ("Value"=w4145:u32)  [unwired: 2 in, 2 out]
                    n1796 = property on="Z offset mm" class="DigNum (strict)"() -> ("Value"=w4141:dbl)  [unwired: 2 in, 2 out]
                    n1797 = To Long Integer(number=w4148) -> (32bit integer=w4147:i32)
                    n1798 = To Long Integer(number=w4150) -> (32bit integer=w4149:i32)
                    n1799 = To Double Precision Float(number=w4145) -> (double precision float=w4146:dbl)
                    n1800 = call "mDrive Send Command.vi"("error in (no error)"=w4131, "Extra"="P", "Command"=T10."Print Parameter", "VISA resource name"=w4132) -> ("error out"=w4134:errorcluster, "read buffer"=w4152:string, "VISA resource name out"=w4135:refnum<visa-resource-name>)  [unwired: 3 in]
                    n1801 = Decimal String To Number(string=w4152, offset=0) -> (number=w4133:i32)  [unwired: 1 in, 1 out]
                    n1802 = property on="Z Step PV" class="DigNum (strict)"("Val(Sgnl)"=w4133) -> ()  [unwired: 2 in, 2 out]
                    n1803 = In Range and Coerce(upper limit=w4147, x=w4133, lower limit=w4149) -> (In Range?=w4136:bool)  [unwired: 1 out]
                    n1804 = To Double Precision Float(number=w4133) -> (double precision float=w4140:dbl)
                    n1805 = property on="Z in Range" class="Bool (strict)"("Val(Sgnl)"=w4136) -> ()  [unwired: 2 in, 2 out]
                    n1806 = Divide(x=w4140, y=w4146) -> (x/y=w4144:dbl)
                    n1807 = property on="Z mm/rev" class="DigNum (strict)"() -> ("Value"=w4143:dbl)  [unwired: 2 in, 2 out]
                    n1808 = Multiply(x=w4144, y=w4143) -> (x*y=w4142:dbl)
                    n1809 = Add(x=w4142, y=w4141) -> (x+y=w4139:dbl)
                    n1810 = property on="Z Position mm PV" class="DigNum (strict)"("Val(Sgnl)"=w4139) -> ()  [unwired: 2 in, 2 out]
                  }
                  frame #1 {
                    n1811 = call "mDrive Send Command.vi"("error in (no error)"=w4153, "Extra"="MV", "Command"=T10."Print Parameter", "VISA resource name"=w4154) -> ("error out"=w4157:errorcluster, "read buffer"=w4161:string, "VISA resource name out"=w4158:refnum<visa-resource-name>)  [unwired: 3 in]
                    n1812 = Decimal String To Number(string=w4161, offset=0 ("offset (0)")) -> (number=w4164:i32)  [unwired: 1 in, 1 out]
                    n1813 = Not Equal?(x=w4161, y="") -> (x != y?=w4159:bool)
                    n1814 = property on="Z Ready" class="Bool (strict)"("Val(Sgnl)"=w4159) -> ()  [unwired: 2 in, 2 out]
                    n1815 = Number To Boolean Array(number=w4164) -> (Boolean array=w4163:bool[])
                    n1816 = Index Array(array=w4163, index=0) -> (element=w4156:bool)
                    n1817 = property on="Z in Motion" class="Bool (strict)"("Val(Sgnl)"=w4156) -> ()  [unwired: 2 in, 2 out]
                  }
                  frame #2 {
                    n1818 = Wait (ms)(milliseconds to wait=u32 50) -> ()  [unwired: 1 out]
                  }
                  frame #3 {
                    n1819 = case shown="True" w4174 {
                      tunnel: w4175 -> [w4181 w4185]
                      tunnel: [w4182 w4185] -> w4176
                      tunnel: [w4183 w4184] -> w4177
                      tunnel: w4178 -> [w4180 w4184]
                      frame #0 {
                        n1820 = call "mDrive Send Command.vi"("error in (no error)"=w4180, "Command"=T10."Stop", "VISA resource name"=w4181) -> ("error out"=w4183:errorcluster, "VISA resource name out"=w4182:refnum<visa-resource-name>)  [unwired: 4 in, 1 out]
                      }
                      frame #1 {
                      }
                    }
                  }
                  frame #4 {
                    n1821 = property on="Z Backlash corr" class="Bool (strict)"() -> ("Value"=w4192:bool)  [unwired: 2 in, 2 out]
                    n1822 = Implies(1:w4191, 2:w4192) -> (0:w4190:bool)
                    n1823 = case shown="False" w4190 {
                      tunnel: w4189 -> [w4200 w4257]
                      tunnel: w4188 -> [w4199 w4258]
                      tunnel: [w4194 w4257] -> w4187
                      tunnel: [w4198 w4258] -> w4186
                      frame #0 {
                        # "Backlash"
                        n1824 = flat-sequence {
                          tunnel: [w4215] -> w4212
                          tunnel: [w4217] -> w4211
                          tunnel: [w4216] -> w4210
                          tunnel: w4200 -> [w4214]
                          tunnel: w4199 -> [w4213]
                          tunnel: w4212 -> [w4225]
                          tunnel: [w4225] -> w4209
                          tunnel: w4211 -> [w4224]
                          tunnel: w4210 -> [w4223]
                          tunnel: [w4222] -> w4208
                          tunnel: [w4221] -> w4207
                          tunnel: [w4220] -> w4197
                          tunnel: w4209 -> [w4239]
                          tunnel: w4208 -> [w4230]
                          tunnel: w4207 -> [w4238]
                          tunnel: [w4230] -> w4206
                          tunnel: [w4238] -> w4205
                          tunnel: [w4229] -> w4202
                          tunnel: [w4237] -> w4201
                          tunnel: w4197 -> [w4237]
                          tunnel: w4206 -> [w4242]
                          tunnel: w4205 -> [w4243]
                          tunnel: [w4241] -> w4204
                          tunnel: [w4249] -> w4203
                          tunnel: w4202 -> [w4249]
                          tunnel: w4201 -> [w4245]
                          tunnel: [w4244] -> w4195
                          tunnel: w4204 -> [w4252]
                          tunnel: w4203 -> [w4251]
                          tunnel: [w4253] -> w4196
                          tunnel: w4195 -> [w4253]
                          tunnel: [w4252] -> w4193
                          tunnel: [w4256] -> w4198
                          tunnel: w4196 -> [w4256]
                          tunnel: [w4254] -> w4194
                          tunnel: w4193 -> [w4254]
                          frame #0 {
                            n1825 = property on="Z Backlash steps/sec" class="DigNum (strict)"() -> ("Value"=w4215:i32)  [unwired: 2 in, 2 out]
                            n1826 = Number To Decimal String(number=w4215) -> (decimal integer string=w4218:string)  [unwired: 1 in]
                            n1827 = call "mDrive Send Command.vi"("error in (no error)"=w4214, "Extra"=w4218, "Command"=T10."Max Velocity", "VISA resource name"=w4213) -> ("error out"=w4216:errorcluster, "VISA resource name out"=w4217:refnum<visa-resource-name>)  [unwired: 3 in, 1 out]
                          }
                          frame #1 {
                            n1828 = property on="Z Backlash" class="DigNum (strict)"() -> ("Value"=w4220:i32)  [unwired: 2 in, 2 out]
                            n1829 = Number To Decimal String(number=w4220) -> (decimal integer string=w4226:string)  [unwired: 1 in]
                            n1830 = call "mDrive Send Command.vi"("error in (no error)"=w4223, "Extra"=w4226, "Command"=T10."Move to Relative Position", "VISA resource name"=w4224) -> ("error out"=w4222:errorcluster, "VISA resource name out"=w4221:refnum<visa-resource-name>)  [unwired: 3 in, 1 out]
                          }
                          frame #2 {
                            n1831 = To Double Precision Float(number=w4237) -> (double precision float=w4235:dbl)
                            n1832 = To Double Precision Float(number=w4239) -> (double precision float=w4240:dbl)
                            n1833 = Absolute Value(x=w4235) -> (abs(x)=w4236:dbl)
                            n1834 = Divide(x=w4236, y=w4240) -> (x/y=w4233:dbl)
                            n1835 = Multiply(x=1000.0, y=w4233) -> (x*y=w4231:dbl)
                            n1836 = Add(x=w4231, y=300.0) -> (x+y=w4229:dbl)
                            n1837 = To Unsigned Long Integer(number=w4229) -> (unsigned 32bit integer=w4228:u32)
                            n1838 = Wait (ms)(milliseconds to wait=w4228) -> ()  [unwired: 1 out]
                          }
                          frame #3 {
                            n1839 = Negate(x=w4245) -> (-x=w4246:i32)
                            n1840 = Number To Decimal String(number=w4246) -> (decimal integer string=w4247:string)  [unwired: 1 in]
                            n1841 = call "mDrive Send Command.vi"("error in (no error)"=w4242, "Extra"=w4247, "Command"=T10."Move to Relative Position", "VISA resource name"=w4243) -> ("error out"=w4241:errorcluster, "VISA resource name out"=w4244:refnum<visa-resource-name>)  [unwired: 3 in, 1 out]
                          }
                          frame #4 {
                            n1842 = To Unsigned Long Integer(number=w4251) -> (unsigned 32bit integer=w4250:u32)
                            n1843 = Wait (ms)(milliseconds to wait=w4250) -> ()  [unwired: 1 out]
                          }
                          frame #5 {
                            n1844 = property on="Z Backlash corr" class="Bool (strict)"("Val(Sgnl)"=FALSE ("Value (Signaling)")) -> ()  [unwired: 2 in, 2 out]
                          }
                        }
                      }
                      frame #1 {
                      }
                    }
                  }
                }
                n1845 = flat-sequence {
                  tunnel: [w4014] -> w3732
                  tunnel: [w4007] -> w3731
                  tunnel: [w4006] -> w3730
                  tunnel: w3674 -> [w4004]
                  tunnel: w3673 -> [w4003]
                  tunnel: [w4034] -> w3729
                  tunnel: [w4033] -> w3728
                  tunnel: [w4032] -> w3727
                  tunnel: [w4025] -> w3726
                  tunnel: w3732 -> [w4032]
                  tunnel: w3731 -> [w4031]
                  tunnel: w3730 -> [w4030]
                  tunnel: w3729 -> [w4044]
                  tunnel: [w4044] -> w3722
                  tunnel: w3728 -> [w4043]
                  tunnel: [w4043] -> w3723
                  tunnel: w3727 -> [w4042]
                  tunnel: [w4042] -> w3724
                  tunnel: w3726 -> [w4041]
                  tunnel: [w4041] -> w3725
                  tunnel: [w4048] -> w3721
                  tunnel: [w4049] -> w3720
                  tunnel: [w4045] -> w3719
                  tunnel: w3725 -> [w4045]
                  tunnel: w3724 -> [w4046]
                  tunnel: w3723 -> [w4050]
                  tunnel: w3722 -> [w4047]
                  tunnel: w3721 -> [w4061]
                  tunnel: w3720 -> [w4062]
                  tunnel: w3719 -> [w4064]
                  tunnel: [w4060] -> w3687
                  tunnel: [w4059] -> w3688
                  frame #0 {
                    n1846 = property on="X Step SP" class="DigNum (strict)"() -> ("Maximum"=w4015:dbl)  [unwired: 2 in, 2 out]
                    n1847 = property on="X Step SP" class="DigNum (strict)"() -> ("Minimum"=w4009:dbl)  [unwired: 2 in, 2 out]
                    n1848 = property on="X steps/rev" class="DigNum (strict)"() -> ("Value"=w4013:u32)  [unwired: 2 in, 2 out]
                    n1849 = property on="X offset mm" class="DigNum (strict)"() -> ("Value"=w4011:dbl)  [unwired: 2 in, 2 out]
                    n1850 = To Long Integer(number=w4015) -> (32bit integer=w4021:i32)
                    n1851 = To Long Integer(number=w4009) -> (32bit integer=w4022:i32)
                    n1852 = To Double Precision Float(number=w4013) -> (double precision float=w4020:dbl)
                    n1853 = call "mDrive Send Command.vi"("error in (no error)"=w4003, "Extra"="P", "Command"=T10."Print Parameter", "VISA resource name"=w4004) -> ("error out"=w4006:errorcluster, "read buffer"=w4024:string, "VISA resource name out"=w4007:refnum<visa-resource-name>)  [unwired: 3 in]
                    n1854 = Decimal String To Number(string=w4024, offset=0) -> (number=w4005:i32)  [unwired: 1 in, 1 out]
                    n1855 = property on="X Step PV" class="DigNum (strict)"("Val(Sgnl)"=w4005) -> ()  [unwired: 2 in, 2 out]
                    n1856 = In Range and Coerce(upper limit=w4021, x=w4005, lower limit=w4022) -> (In Range?=w4014:bool)  [unwired: 1 out]
                    n1857 = To Double Precision Float(number=w4005) -> (double precision float=w4018:dbl)
                    n1858 = property on="X  in Range" class="Bool (strict)"("Val(Sgnl)"=w4014) -> ()  [unwired: 2 in, 2 out]
                    n1859 = Divide(x=w4018, y=w4020) -> (x/y=w4019:dbl)
                    n1860 = property on="X mm/rev" class="DigNum (strict)"() -> ("Value"=w4012:dbl)  [unwired: 2 in, 2 out]
                    n1861 = Multiply(x=w4019, y=w4012) -> (x*y=w4008:dbl)
                    n1862 = Add(x=w4008, y=w4011) -> (x+y=w4010:dbl)
                    n1863 = property on="X Position mm PV" class="DigNum (strict)"("Val(Sgnl)"=w4010) -> ()  [unwired: 2 in, 2 out]
                  }
                  frame #1 {
                    n1864 = call "mDrive Send Command.vi"("error in (no error)"=w4030, "Extra"="MV", "Command"=T10."Print Parameter", "VISA resource name"=w4031) -> ("error out"=w4033:errorcluster, "read buffer"=w4036:string, "VISA resource name out"=w4034:refnum<visa-resource-name>)  [unwired: 3 in]
                    n1865 = Decimal String To Number(string=w4036, offset=0 ("offset (0)")) -> (number=w4026:i32)  [unwired: 1 in, 1 out]
                    n1866 = Not Equal?(x=w4036, y="") -> (x != y?=w4029:bool)
                    n1867 = property on="X Ready" class="Bool (strict)"("Val(Sgnl)"=w4029) -> ()  [unwired: 2 in, 2 out]
                    n1868 = Number To Boolean Array(number=w4026) -> (Boolean array=w4028:bool[])
                    n1869 = Index Array(array=w4028, index=0) -> (element=w4025:bool)
                    n1870 = property on="X  in Motion" class="Bool (strict)"("Val(Sgnl)"=w4025) -> ()  [unwired: 2 in, 2 out]
                  }
                  frame #2 {
                    n1871 = Wait (ms)(milliseconds to wait=u32 50) -> ()  [unwired: 1 out]
                  }
                  frame #3 {
                    n1872 = case shown="False" w4046 {
                      tunnel: w4047 -> [w4053 w4057]
                      tunnel: [w4054 w4057] -> w4048
                      tunnel: [w4055 w4056] -> w4049
                      tunnel: w4050 -> [w4052 w4056]
                      frame #0 {
                        n1873 = call "mDrive Send Command.vi"("error in (no error)"=w4052, "Command"=T10."Stop", "VISA resource name"=w4053) -> ("error out"=w4055:errorcluster, "VISA resource name out"=w4054:refnum<visa-resource-name>)  [unwired: 4 in, 1 out]
                      }
                      frame #1 {
                      }
                    }
                  }
                  frame #4 {
                    n1874 = property on="X Backlash corr" class="Bool (strict)"() -> ("Value"=w4058:bool)  [unwired: 2 in, 2 out]
                    n1875 = Implies(1:w4064, 2:w4058) -> (0:w4063:bool)
                    n1876 = case shown="False" w4063 {
                      tunnel: w4062 -> [w4072 w4129]
                      tunnel: w4061 -> [w4071 w4130]
                      tunnel: [w4066 w4129] -> w4060
                      tunnel: [w4070 w4130] -> w4059
                      frame #0 {
                        # "Backlash"
                        n1877 = flat-sequence {
                          tunnel: [w4085] -> w4084
                          tunnel: [w4089] -> w4083
                          tunnel: [w4088] -> w4082
                          tunnel: w4072 -> [w4087]
                          tunnel: w4071 -> [w4086]
                          tunnel: w4084 -> [w4097]
                          tunnel: [w4097] -> w4081
                          tunnel: w4083 -> [w4096]
                          tunnel: w4082 -> [w4095]
                          tunnel: [w4094] -> w4080
                          tunnel: [w4093] -> w4079
                          tunnel: [w4092] -> w4069
                          tunnel: w4081 -> [w4111]
                          tunnel: w4080 -> [w4102]
                          tunnel: w4079 -> [w4110]
                          tunnel: [w4102] -> w4078
                          tunnel: [w4110] -> w4077
                          tunnel: [w4101] -> w4074
                          tunnel: [w4109] -> w4073
                          tunnel: w4069 -> [w4109]
                          tunnel: w4078 -> [w4114]
                          tunnel: w4077 -> [w4115]
                          tunnel: [w4113] -> w4076
                          tunnel: [w4121] -> w4075
                          tunnel: w4074 -> [w4121]
                          tunnel: w4073 -> [w4117]
                          tunnel: [w4116] -> w4067
                          tunnel: w4076 -> [w4124]
                          tunnel: w4075 -> [w4123]
                          tunnel: [w4125] -> w4068
                          tunnel: w4067 -> [w4125]
                          tunnel: [w4124] -> w4065
                          tunnel: [w4128] -> w4070
                          tunnel: w4068 -> [w4128]
                          tunnel: [w4127] -> w4066
                          tunnel: w4065 -> [w4127]
                          frame #0 {
                            n1878 = property on="X Backlash steps/sec" class="DigNum (strict)"() -> ("Value"=w4085:i32)  [unwired: 2 in, 2 out]
                            n1879 = Number To Decimal String(number=w4085) -> (decimal integer string=w4090:string)  [unwired: 1 in]
                            n1880 = call "mDrive Send Command.vi"("error in (no error)"=w4087, "Extra"=w4090, "Command"=T10."Max Velocity", "VISA resource name"=w4086) -> ("error out"=w4088:errorcluster, "VISA resource name out"=w4089:refnum<visa-resource-name>)  [unwired: 3 in, 1 out]
                          }
                          frame #1 {
                            n1881 = property on="X Backlash" class="DigNum (strict)"() -> ("Value"=w4092:i32)  [unwired: 2 in, 2 out]
                            n1882 = Number To Decimal String(number=w4092) -> (decimal integer string=w4098:string)  [unwired: 1 in]
                            n1883 = call "mDrive Send Command.vi"("error in (no error)"=w4095, "Extra"=w4098, "Command"=T10."Move to Relative Position", "VISA resource name"=w4096) -> ("error out"=w4094:errorcluster, "VISA resource name out"=w4093:refnum<visa-resource-name>)  [unwired: 3 in, 1 out]
                          }
                          frame #2 {
                            n1884 = To Double Precision Float(number=w4109) -> (double precision float=w4107:dbl)
                            n1885 = To Double Precision Float(number=w4111) -> (double precision float=w4112:dbl)
                            n1886 = Absolute Value(x=w4107) -> (abs(x)=w4108:dbl)
                            n1887 = Divide(x=w4108, y=w4112) -> (x/y=w4105:dbl)
                            n1888 = Multiply(x=1000.0, y=w4105) -> (x*y=w4103:dbl)
                            n1889 = Add(x=w4103, y=300.0) -> (x+y=w4101:dbl)
                            n1890 = To Unsigned Long Integer(number=w4101) -> (unsigned 32bit integer=w4100:u32)
                            n1891 = Wait (ms)(milliseconds to wait=w4100) -> ()  [unwired: 1 out]
                          }
                          frame #3 {
                            n1892 = Negate(x=w4117) -> (-x=w4118:i32)
                            n1893 = Number To Decimal String(number=w4118) -> (decimal integer string=w4119:string)  [unwired: 1 in]
                            n1894 = call "mDrive Send Command.vi"("error in (no error)"=w4114, "Extra"=w4119, "Command"=T10."Move to Relative Position", "VISA resource name"=w4115) -> ("error out"=w4113:errorcluster, "VISA resource name out"=w4116:refnum<visa-resource-name>)  [unwired: 3 in, 1 out]
                          }
                          frame #4 {
                            n1895 = To Unsigned Long Integer(number=w4123) -> (unsigned 32bit integer=w4122:u32)
                            n1896 = Wait (ms)(milliseconds to wait=w4122) -> ()  [unwired: 1 out]
                          }
                          frame #5 {
                            n1897 = property on="X Backlash corr" class="Bool (strict)"("Val(Sgnl)"=FALSE ("Value (Signaling)")) -> ()  [unwired: 2 in, 2 out]
                          }
                        }
                      }
                      frame #1 {
                      }
                    }
                  }
                }
                n1898 = flat-sequence {
                  tunnel: [w3884] -> w3718
                  tunnel: [w3886] -> w3717
                  tunnel: [w3885] -> w3716
                  tunnel: w3679 -> [w3876]
                  tunnel: w3678 -> [w3875]
                  tunnel: [w3906] -> w3715
                  tunnel: [w3905] -> w3714
                  tunnel: [w3904] -> w3713
                  tunnel: [w3897] -> w3712
                  tunnel: w3718 -> [w3904]
                  tunnel: w3717 -> [w3903]
                  tunnel: w3716 -> [w3902]
                  tunnel: w3715 -> [w3916]
                  tunnel: [w3916] -> w3708
                  tunnel: w3714 -> [w3915]
                  tunnel: [w3915] -> w3709
                  tunnel: w3713 -> [w3914]
                  tunnel: [w3914] -> w3710
                  tunnel: w3712 -> [w3913]
                  tunnel: [w3913] -> w3711
                  tunnel: [w3920] -> w3707
                  tunnel: [w3921] -> w3706
                  tunnel: [w3917] -> w3705
                  tunnel: w3711 -> [w3917]
                  tunnel: w3710 -> [w3918]
                  tunnel: w3709 -> [w3922]
                  tunnel: w3708 -> [w3919]
                  tunnel: w3707 -> [w3933]
                  tunnel: w3706 -> [w3934]
                  tunnel: w3705 -> [w3936]
                  tunnel: [w3932] -> w3685
                  tunnel: [w3931] -> w3686
                  frame #0 {
                    n1899 = property on="Y Step SP" class="DigNum (strict)"() -> ("Maximum"=w3879:dbl)  [unwired: 2 in, 2 out]
                    n1900 = property on="Y Step SP" class="DigNum (strict)"() -> ("Minimum"=w3878:dbl)  [unwired: 2 in, 2 out]
                    n1901 = property on="Y steps/rev" class="DigNum (strict)"() -> ("Value"=w3880:u32)  [unwired: 2 in, 2 out]
                    n1902 = property on="Y offset mm" class="DigNum (strict)"() -> ("Value"=w3882:dbl)  [unwired: 2 in, 2 out]
                    n1903 = To Long Integer(number=w3879) -> (32bit integer=w3893:i32)
                    n1904 = To Long Integer(number=w3878) -> (32bit integer=w3894:i32)
                    n1905 = To Double Precision Float(number=w3880) -> (double precision float=w3892:dbl)
                    n1906 = call "mDrive Send Command.vi"("error in (no error)"=w3876, "Extra"="P", "Command"=T10."Print Parameter", "VISA resource name"=w3875) -> ("error out"=w3885:errorcluster, "read buffer"=w3896:string, "VISA resource name out"=w3886:refnum<visa-resource-name>)  [unwired: 3 in]
                    n1907 = Decimal String To Number(string=w3896, offset=0) -> (number=w3877:i32)  [unwired: 1 in, 1 out]
                    n1908 = property on="Y Step PV" class="DigNum (strict)"("Val(Sgnl)"=w3877) -> ()  [unwired: 2 in, 2 out]
                    n1909 = In Range and Coerce(upper limit=w3893, x=w3877, lower limit=w3894) -> (In Range?=w3884:bool)  [unwired: 1 out]
                    n1910 = To Double Precision Float(number=w3877) -> (double precision float=w3889:dbl)
                    n1911 = property on="Y in Range" class="Bool (strict)"("Val(Sgnl)"=w3884) -> ()  [unwired: 2 in, 2 out]
                    n1912 = Divide(x=w3889, y=w3892) -> (x/y=w3891:dbl)
                    n1913 = property on="Y mm/rev" class="DigNum (strict)"() -> ("Value"=w3881:dbl)  [unwired: 2 in, 2 out]
                    n1914 = Multiply(x=w3891, y=w3881) -> (x*y=w3890:dbl)
                    n1915 = Add(x=w3890, y=w3882) -> (x+y=w3883:dbl)
                    n1916 = property on="Y Position mm PV" class="DigNum (strict)"("Val(Sgnl)"=w3883) -> ()  [unwired: 2 in, 2 out]
                  }
                  frame #1 {
                    n1917 = call "mDrive Send Command.vi"("error in (no error)"=w3902, "Extra"="MV", "Command"=T10."Print Parameter", "VISA resource name"=w3903) -> ("error out"=w3905:errorcluster, "read buffer"=w3908:string, "VISA resource name out"=w3906:refnum<visa-resource-name>)  [unwired: 3 in]
                    n1918 = Decimal String To Number(string=w3908, offset=0 ("offset (0)")) -> (number=w3898:i32)  [unwired: 1 in, 1 out]
                    n1919 = Not Equal?(x=w3908, y="") -> (x != y?=w3901:bool)
                    n1920 = property on="Y Ready" class="Bool (strict)"("Val(Sgnl)"=w3901) -> ()  [unwired: 2 in, 2 out]
                    n1921 = Number To Boolean Array(number=w3898) -> (Boolean array=w3900:bool[])
                    n1922 = Index Array(array=w3900, index=0) -> (element=w3897:bool)
                    n1923 = property on="Y in Motion" class="Bool (strict)"("Val(Sgnl)"=w3897) -> ()  [unwired: 2 in, 2 out]
                  }
                  frame #2 {
                    n1924 = Wait (ms)(milliseconds to wait=u32 50) -> ()  [unwired: 1 out]
                  }
                  frame #3 {
                    n1925 = case shown="False" w3918 {
                      tunnel: w3919 -> [w3925 w3928]
                      tunnel: [w3926 w3928] -> w3920
                      tunnel: [w3927 w3929] -> w3921
                      tunnel: w3922 -> [w3924 w3929]
                      frame #0 {
                        n1926 = call "mDrive Send Command.vi"("error in (no error)"=w3924, "Command"=T10."Stop", "VISA resource name"=w3925) -> ("error out"=w3927:errorcluster, "VISA resource name out"=w3926:refnum<visa-resource-name>)  [unwired: 4 in, 1 out]
                      }
                      frame #1 {
                      }
                    }
                  }
                  frame #4 {
                    n1927 = property on="Y Backlash corr" class="Bool (strict)"() -> ("Value"=w3930:bool)  [unwired: 2 in, 2 out]
                    n1928 = Implies(1:w3936, 2:w3930) -> (0:w3935:bool)
                    n1929 = case shown="False" w3935 {
                      tunnel: w3934 -> [w3944 w4001]
                      tunnel: w3933 -> [w3943 w4002]
                      tunnel: [w3938 w4001] -> w3932
                      tunnel: [w3942 w4002] -> w3931
                      frame #0 {
                        # "Backlash"
                        n1930 = flat-sequence {
                          tunnel: [w3957] -> w3956
                          tunnel: [w3961] -> w3955
                          tunnel: [w3960] -> w3954
                          tunnel: w3944 -> [w3959]
                          tunnel: w3943 -> [w3958]
                          tunnel: w3956 -> [w3969]
                          tunnel: [w3969] -> w3953
                          tunnel: w3955 -> [w3968]
                          tunnel: w3954 -> [w3967]
                          tunnel: [w3966] -> w3952
                          tunnel: [w3965] -> w3951
                          tunnel: [w3964] -> w3941
                          tunnel: w3953 -> [w3983]
                          tunnel: w3952 -> [w3974]
                          tunnel: w3951 -> [w3982]
                          tunnel: [w3974] -> w3950
                          tunnel: [w3982] -> w3949
                          tunnel: [w3973] -> w3946
                          tunnel: [w3981] -> w3945
                          tunnel: w3941 -> [w3981]
                          tunnel: w3950 -> [w3986]
                          tunnel: w3949 -> [w3987]
                          tunnel: [w3985] -> w3948
                          tunnel: [w3993] -> w3947
                          tunnel: w3946 -> [w3993]
                          tunnel: w3945 -> [w3989]
                          tunnel: [w3988] -> w3939
                          tunnel: w3948 -> [w3996]
                          tunnel: w3947 -> [w3995]
                          tunnel: [w3997] -> w3940
                          tunnel: w3939 -> [w3997]
                          tunnel: [w3996] -> w3937
                          tunnel: [w4000] -> w3942
                          tunnel: w3940 -> [w4000]
                          tunnel: [w3999] -> w3938
                          tunnel: w3937 -> [w3999]
                          frame #0 {
                            n1931 = property on="Y Backlash steps/sec" class="DigNum (strict)"() -> ("Value"=w3957:i32)  [unwired: 2 in, 2 out]
                            n1932 = Number To Decimal String(number=w3957) -> (decimal integer string=w3962:string)  [unwired: 1 in]
                            n1933 = call "mDrive Send Command.vi"("error in (no error)"=w3959, "Extra"=w3962, "Command"=T10."Max Velocity", "VISA resource name"=w3958) -> ("error out"=w3960:errorcluster, "VISA resource name out"=w3961:refnum<visa-resource-name>)  [unwired: 3 in, 1 out]
                          }
                          frame #1 {
                            n1934 = property on="Y Backlash" class="DigNum (strict)"() -> ("Value"=w3964:i32)  [unwired: 2 in, 2 out]
                            n1935 = Number To Decimal String(number=w3964) -> (decimal integer string=w3970:string)  [unwired: 1 in]
                            n1936 = call "mDrive Send Command.vi"("error in (no error)"=w3967, "Extra"=w3970, "Command"=T10."Move to Relative Position", "VISA resource name"=w3968) -> ("error out"=w3966:errorcluster, "VISA resource name out"=w3965:refnum<visa-resource-name>)  [unwired: 3 in, 1 out]
                          }
                          frame #2 {
                            n1937 = To Double Precision Float(number=w3981) -> (double precision float=w3979:dbl)
                            n1938 = To Double Precision Float(number=w3983) -> (double precision float=w3984:dbl)
                            n1939 = Absolute Value(x=w3979) -> (abs(x)=w3980:dbl)
                            n1940 = Divide(x=w3980, y=w3984) -> (x/y=w3977:dbl)
                            n1941 = Multiply(x=1000.0, y=w3977) -> (x*y=w3975:dbl)
                            n1942 = Add(x=w3975, y=300.0) -> (x+y=w3973:dbl)
                            n1943 = To Unsigned Long Integer(number=w3973) -> (unsigned 32bit integer=w3972:u32)
                            n1944 = Wait (ms)(milliseconds to wait=w3972) -> ()  [unwired: 1 out]
                          }
                          frame #3 {
                            n1945 = Negate(x=w3989) -> (-x=w3990:i32)
                            n1946 = Number To Decimal String(number=w3990) -> (decimal integer string=w3991:string)  [unwired: 1 in]
                            n1947 = call "mDrive Send Command.vi"("error in (no error)"=w3986, "Extra"=w3991, "Command"=T10."Move to Relative Position", "VISA resource name"=w3987) -> ("error out"=w3985:errorcluster, "VISA resource name out"=w3988:refnum<visa-resource-name>)  [unwired: 3 in, 1 out]
                          }
                          frame #4 {
                            n1948 = To Unsigned Long Integer(number=w3995) -> (unsigned 32bit integer=w3994:u32)
                            n1949 = Wait (ms)(milliseconds to wait=w3994) -> ()  [unwired: 1 out]
                          }
                          frame #5 {
                            n1950 = property on="Y Backlash corr" class="Bool (strict)"("Val(Sgnl)"=FALSE ("Value (Signaling)")) -> ()  [unwired: 2 in, 2 out]
                          }
                        }
                      }
                      frame #1 {
                      }
                    }
                  }
                }
                n1951 = flat-sequence {
                  tunnel: [w3756] -> w3704
                  tunnel: [w3758] -> w3703
                  tunnel: [w3757] -> w3702
                  tunnel: w3677 -> [w3748]
                  tunnel: w3676 -> [w3747]
                  tunnel: [w3778] -> w3701
                  tunnel: [w3777] -> w3700
                  tunnel: [w3776] -> w3699
                  tunnel: [w3769] -> w3698
                  tunnel: w3704 -> [w3776]
                  tunnel: w3703 -> [w3775]
                  tunnel: w3702 -> [w3774]
                  tunnel: w3701 -> [w3788]
                  tunnel: [w3788] -> w3694
                  tunnel: w3700 -> [w3787]
                  tunnel: [w3787] -> w3695
                  tunnel: w3699 -> [w3786]
                  tunnel: [w3786] -> w3696
                  tunnel: w3698 -> [w3785]
                  tunnel: [w3785] -> w3697
                  tunnel: [w3792] -> w3693
                  tunnel: [w3793] -> w3692
                  tunnel: [w3789] -> w3691
                  tunnel: w3697 -> [w3789]
                  tunnel: w3696 -> [w3790]
                  tunnel: w3695 -> [w3794]
                  tunnel: w3694 -> [w3791]
                  tunnel: w3693 -> [w3805]
                  tunnel: w3692 -> [w3806]
                  tunnel: w3691 -> [w3808]
                  tunnel: [w3804] -> w3683
                  tunnel: [w3803] -> w3684
                  frame #0 {
                    n1952 = property on="R Step SP" class="DigNum (strict)"() -> ("Maximum"=w3751:dbl)  [unwired: 2 in, 2 out]
                    n1953 = property on="R Step SP" class="DigNum (strict)"() -> ("Minimum"=w3752:dbl)  [unwired: 2 in, 2 out]
                    n1954 = property on="R steps/rev" class="DigNum (strict)"() -> ("Value"=w3750:u32)  [unwired: 2 in, 2 out]
                    n1955 = property on="R offset deg" class="DigNum (strict)"() -> ("Value"=w3754:dbl)  [unwired: 2 in, 2 out]
                    n1956 = To Long Integer(number=w3751) -> (32bit integer=w3765:i32)
                    n1957 = To Long Integer(number=w3752) -> (32bit integer=w3766:i32)
                    n1958 = To Double Precision Float(number=w3750) -> (double precision float=w3764:dbl)
                    n1959 = call "mDrive Send Command.vi"("error in (no error)"=w3748, "Extra"="P", "Command"=T10."Print Parameter", "VISA resource name"=w3747) -> ("error out"=w3757:errorcluster, "read buffer"=w3768:string, "VISA resource name out"=w3758:refnum<visa-resource-name>)  [unwired: 3 in]
                    n1960 = Decimal String To Number(string=w3768, offset=0) -> (number=w3749:i32)  [unwired: 1 in, 1 out]
                    n1961 = property on="R Step PV" class="DigNum (strict)"("Val(Sgnl)"=w3749) -> ()  [unwired: 2 in, 2 out]
                    n1962 = In Range and Coerce(upper limit=w3765, x=w3749, lower limit=w3766) -> (In Range?=w3756:bool)  [unwired: 1 out]
                    n1963 = To Double Precision Float(number=w3749) -> (double precision float=w3761:dbl)
                    n1964 = property on="R in Range" class="Bool (strict)"("Val(Sgnl)"=w3756) -> ()  [unwired: 2 in, 2 out]
                    n1965 = Divide(x=w3761, y=w3764) -> (x/y=w3763:dbl)
                    n1966 = property on="R deg/rev" class="DigNum (strict)"() -> ("Value"=w3753:dbl)  [unwired: 2 in, 2 out]
                    n1967 = Multiply(x=w3763, y=w3753) -> (x*y=w3762:dbl)
                    n1968 = Add(x=w3762, y=w3754) -> (x+y=w3755:dbl)
                    n1969 = property on="R Position deg PV" class="DigNum (strict)"("Val(Sgnl)"=w3755) -> ()  [unwired: 2 in, 2 out]
                  }
                  frame #1 {
                    n1970 = call "mDrive Send Command.vi"("error in (no error)"=w3774, "Extra"="MV", "Command"=T10."Print Parameter", "VISA resource name"=w3775) -> ("error out"=w3777:errorcluster, "read buffer"=w3780:string, "VISA resource name out"=w3778:refnum<visa-resource-name>)  [unwired: 3 in]
                    n1971 = Decimal String To Number(string=w3780, offset=0 ("offset (0)")) -> (number=w3770:i32)  [unwired: 1 in, 1 out]
                    n1972 = Not Equal?(x=w3780, y="") -> (x != y?=w3773:bool)
                    n1973 = property on="R Ready" class="Bool (strict)"("Val(Sgnl)"=w3773) -> ()  [unwired: 2 in, 2 out]
                    n1974 = Number To Boolean Array(number=w3770) -> (Boolean array=w3772:bool[])
                    n1975 = Index Array(array=w3772, index=0) -> (element=w3769:bool)
                    n1976 = property on="R in Motion" class="Bool (strict)"("Val(Sgnl)"=w3769) -> ()  [unwired: 2 in, 2 out]
                  }
                  frame #2 {
                    n1977 = Wait (ms)(milliseconds to wait=u32 50) -> ()  [unwired: 1 out]
                  }
                  frame #3 {
                    n1978 = case shown="False" w3790 {
                      tunnel: w3791 -> [w3797 w3801]
                      tunnel: [w3798 w3801] -> w3792
                      tunnel: [w3799 w3800] -> w3793
                      tunnel: w3794 -> [w3796 w3800]
                      frame #0 {
                        n1979 = call "mDrive Send Command.vi"("error in (no error)"=w3796, "Command"=T10."Stop", "VISA resource name"=w3797) -> ("error out"=w3799:errorcluster, "VISA resource name out"=w3798:refnum<visa-resource-name>)  [unwired: 4 in, 1 out]
                      }
                      frame #1 {
                      }
                    }
                  }
                  frame #4 {
                    n1980 = property on="R Backlash corr" class="Bool (strict)"() -> ("Value"=w3802:bool)  [unwired: 2 in, 2 out]
                    n1981 = Implies(1:w3808, 2:w3802) -> (0:w3807:bool)
                    n1982 = case shown="False" w3807 {
                      tunnel: w3806 -> [w3816 w3873]
                      tunnel: w3805 -> [w3815 w3874]
                      tunnel: [w3810 w3873] -> w3804
                      tunnel: [w3814 w3874] -> w3803
                      frame #0 {
                        # "Backlash"
                        n1983 = flat-sequence {
                          tunnel: [w3829] -> w3828
                          tunnel: [w3833] -> w3827
                          tunnel: [w3832] -> w3826
                          tunnel: w3816 -> [w3831]
                          tunnel: w3815 -> [w3830]
                          tunnel: w3828 -> [w3841]
                          tunnel: [w3841] -> w3825
                          tunnel: w3827 -> [w3840]
                          tunnel: w3826 -> [w3839]
                          tunnel: [w3838] -> w3824
                          tunnel: [w3837] -> w3823
                          tunnel: [w3836] -> w3813
                          tunnel: w3825 -> [w3855]
                          tunnel: w3824 -> [w3846]
                          tunnel: w3823 -> [w3854]
                          tunnel: [w3846] -> w3822
                          tunnel: [w3854] -> w3821
                          tunnel: [w3845] -> w3818
                          tunnel: [w3853] -> w3817
                          tunnel: w3813 -> [w3853]
                          tunnel: w3822 -> [w3858]
                          tunnel: w3821 -> [w3859]
                          tunnel: [w3857] -> w3820
                          tunnel: [w3865] -> w3819
                          tunnel: w3818 -> [w3865]
                          tunnel: w3817 -> [w3861]
                          tunnel: [w3860] -> w3811
                          tunnel: w3820 -> [w3868]
                          tunnel: w3819 -> [w3867]
                          tunnel: [w3869] -> w3812
                          tunnel: w3811 -> [w3869]
                          tunnel: [w3868] -> w3809
                          tunnel: [w3872] -> w3814
                          tunnel: w3812 -> [w3872]
                          tunnel: [w3871] -> w3810
                          tunnel: w3809 -> [w3871]
                          frame #0 {
                            n1984 = property on="R Backlash steps/sec" class="DigNum (strict)"() -> ("Value"=w3829:i32)  [unwired: 2 in, 2 out]
                            n1985 = Number To Decimal String(number=w3829) -> (decimal integer string=w3834:string)  [unwired: 1 in]
                            n1986 = call "mDrive Send Command.vi"("error in (no error)"=w3831, "Extra"=w3834, "Command"=T10."Max Velocity", "VISA resource name"=w3830) -> ("error out"=w3832:errorcluster, "VISA resource name out"=w3833:refnum<visa-resource-name>)  [unwired: 3 in, 1 out]
                          }
                          frame #1 {
                            n1987 = property on="R Backlash steps/sec" class="DigNum (strict)"() -> ("Value"=w3836:i32)  [unwired: 2 in, 2 out]
                            n1988 = Number To Decimal String(number=w3836) -> (decimal integer string=w3842:string)  [unwired: 1 in]
                            n1989 = call "mDrive Send Command.vi"("error in (no error)"=w3839, "Extra"=w3842, "Command"=T10."Move to Relative Position", "VISA resource name"=w3840) -> ("error out"=w3838:errorcluster, "VISA resource name out"=w3837:refnum<visa-resource-name>)  [unwired: 3 in, 1 out]
                          }
                          frame #2 {
                            n1990 = To Double Precision Float(number=w3853) -> (double precision float=w3851:dbl)
                            n1991 = To Double Precision Float(number=w3855) -> (double precision float=w3856:dbl)
                            n1992 = Absolute Value(x=w3851) -> (abs(x)=w3852:dbl)
                            n1993 = Divide(x=w3852, y=w3856) -> (x/y=w3849:dbl)
                            n1994 = Multiply(x=1000.0, y=w3849) -> (x*y=w3847:dbl)
                            n1995 = Add(x=w3847, y=300.0) -> (x+y=w3845:dbl)
                            n1996 = To Unsigned Long Integer(number=w3845) -> (unsigned 32bit integer=w3844:u32)
                            n1997 = Wait (ms)(milliseconds to wait=w3844) -> ()  [unwired: 1 out]
                          }
                          frame #3 {
                            n1998 = Negate(x=w3861) -> (-x=w3862:i32)
                            n1999 = Number To Decimal String(number=w3862) -> (decimal integer string=w3863:string)  [unwired: 1 in]
                            n2000 = call "mDrive Send Command.vi"("error in (no error)"=w3858, "Extra"=w3863, "Command"=T10."Move to Relative Position", "VISA resource name"=w3859) -> ("error out"=w3857:errorcluster, "VISA resource name out"=w3860:refnum<visa-resource-name>)  [unwired: 3 in, 1 out]
                          }
                          frame #4 {
                            n2001 = To Unsigned Long Integer(number=w3867) -> (unsigned 32bit integer=w3866:u32)
                            n2002 = Wait (ms)(milliseconds to wait=w3866) -> ()  [unwired: 1 out]
                          }
                          frame #5 {
                            n2003 = property on="R Backlash corr" class="Bool (strict)"("Val(Sgnl)"=FALSE ("Value (Signaling)")) -> ()  [unwired: 2 in, 2 out]
                          }
                        }
                      }
                      frame #1 {
                      }
                    }
                  }
                }
                n2004 = property on="Y in Motion" class="Bool (strict)"() -> ("Value"=w3682:bool)  [unwired: 2 in, 2 out]
                n2005 = property on="Z in Motion" class="Bool (strict)"() -> ("Value"=w3670:bool)  [unwired: 2 in, 2 out]
                n2006 = property on="X  in Motion" class="Bool (strict)"() -> ("Value"=w3681:bool)  [unwired: 2 in, 2 out]
                n2007 = property on="R in Motion" class="Bool (strict)"() -> ("Value"=w3669:bool)  [unwired: 2 in, 2 out]
                n2008 = Compound Arithmetic op=OR(w3681, w3682, w3670, w3669) -> (w3680:bool)
                n2009 = Not(x=w3680) -> (.not. x?=w3675:bool)
              }
            }
            frame #7 {
              n2010 = Wait (ms)(milliseconds to wait=u32 1000) -> ()  [unwired: 1 out]
            }
          }
          n2011 = Increment(x=w2714) -> (x+1=w2715:i32)
          n2012 = property on="#th loop" class="DigNum (strict)"("Val(Sgnl)"=w2715) -> ()  [unwired: 2 in, 2 out]
          n2013 = property on="#th loop" class="DigNum (strict)"() -> ("Value"=w2704:dbl)  [unwired: 2 in, 2 out]
          n2014 = property on="# of loops" class="DigNum (strict)"() -> ("Value"=w2705:dbl)  [unwired: 2 in, 2 out]
          n2015 = Greater Or Equal?(x=w2704, y=w2705) -> (x >= y?=w2703:bool)
        }
        n2016 = flat-sequence {
          tunnel: [w4269] -> _
          tunnel: w2686 -> [w4269]
          tunnel: w2685 -> [_]
          tunnel: [w4268] -> _
          tunnel: w2684 -> [w4268]
          tunnel: w2683 -> [_]
          frame #0 {
            w4272 = T9."Enabled" ("Disabled")
            n2017 = property on="Z Scan Length SP steps" class="DigNum (strict)"("DisabledEnum"=T9."Enabled" ("Disabled")) -> ()  [unwired: 2 in, 2 out]
            n2018 = property on="Z Scan Velocity SP steps/sec" class="DigNum (strict)"("DisabledEnum"=T9."Enabled" ("Disabled")) -> ()  [unwired: 2 in, 2 out]
            n2019 = property on="R Scan Length SP steps" class="DigNum (strict)"("DisabledEnum"=T9."Enabled" ("Disabled")) -> ()  [unwired: 2 in, 2 out]
            n2020 = property on="X Scan Velocity SP steps/sec" class="DigNum (strict)"("DisabledEnum"=T9."Enabled" ("Disabled")) -> ()  [unwired: 2 in, 2 out]
            n2021 = property on="GO" class="Bool"("DisabledEnum"=w4272) -> ()  [unwired: 2 in, 2 out]
            n2022 = property on="Set Scan \nParameters" class="Bool"("DisabledEnum"=w4272) -> ()  [unwired: 2 in, 2 out]
            n2023 = property on="Y Scan Length SP steps" class="DigNum (strict)"("DisabledEnum"=T9."Enabled" ("Disabled")) -> ()  [unwired: 2 in, 2 out]
            n2024 = local write "STATUS"("LEAVING LOOP" ("STATUS")) -> ()
            n2025 = property on="R Scan Velocity SP steps/sec" class="DigNum (strict)"("DisabledEnum"=T9."Enabled" ("Disabled")) -> ()  [unwired: 2 in, 2 out]
            n2026 = property on="X Scan Length SP steps" class="DigNum (strict)"("DisabledEnum"=T9."Enabled" ("Disabled")) -> ()  [unwired: 2 in, 2 out]
            n2027 = property on="Y Scan Selocity SP steps/sec" class="DigNum (strict)"("DisabledEnum"=T9."Enabled" ("Disabled")) -> ()  [unwired: 2 in, 2 out]
            n2028 = property on="Send scan parameter" class="Bool"("DisabledEnum"=w4272) -> ()  [unwired: 2 in, 2 out]
            n2029 = property on="Scan Go" class="Bool (strict)"("DisabledEnum"=T9."Disabled and Grayed Out" ("Disabled")) -> ()  [unwired: 2 in, 2 out]
          }
        }
      }
    }
    n2030 = case shown="False" "Delete Button" {
      tunnel: w296 -> [_ w329]
      frame #0 {
      }
      frame #1 {
        n2031 = local read "Preset positions"() -> (w327:i32)
        n2032 = local read "Presets"() -> (w328:i32[][])
        n2033 = Delete From Array(array=w329, index=w327) -> (array with subset deleted=w325:string[])  [unwired: 1 in, 1 out]
        n2034 = property on="Preset positions" class="Ring (strict)"("Strings []"=w325) -> ()  [unwired: 2 in, 2 out]
        n2035 = Delete From Array(array=w328, index (row)=w327) -> (array with subset deleted=w326:i32[][])  [unwired: 2 in, 1 out]
        n2036 = local write "Presets"(w326) -> ()
      }
    }
    n2037 = case shown="False" "Add Button" {
      tunnel: w296 -> [_ w339]
      frame #0 {
      }
      frame #1 {
        n2038 = property on="X Step PV" class="DigNum (strict)"() -> ("Value"=w333:i32)  [unwired: 2 in, 2 out]
        n2039 = property on="Y Step PV" class="DigNum (strict)"() -> ("Value"=w332:i32)  [unwired: 2 in, 2 out]
        n2040 = property on="Z Step PV" class="DigNum (strict)"() -> ("Value"=w330:i32)  [unwired: 2 in, 2 out]
        n2041 = property on="R Step PV" class="DigNum (strict)"() -> ("Value"=w331:i32)  [unwired: 2 in, 2 out]
        n2042 = Build Array(w333, w332, w330, w331) -> (w336:i32[])
        n2043 = Build Array (concatenate)(w339, "String") -> (w334:string[])
        n2044 = local read "Presets"() -> (w337:i32[][])
        n2045 = property on="Preset positions" class="Ring (strict)"("Strings []"=w334) -> ()  [unwired: 2 in, 2 out]
        n2046 = Build Array (concatenate)(w337, w336) -> (w335:i32[][])
        n2047 = local write "Presets"(w335) -> ()
      }
    }
    n2048 = case shown="False" "Set Button" {
      tunnel: "Preset positions" -> [_ w346]
      frame #0 {
      }
      frame #1 {
        n2049 = local read "Presets"() -> (w347:i32[][])
        n2050 = Index Array(array=w347, index (row)=w346) -> (element=w345:i32[])  [unwired: 1 in]
        n2051 = Array To Cluster(array=w345) -> (cluster=w344:T11)
        n2052 = Unbundle(w344) -> ("Presets[0]"=w343:i32, "Presets[1]"=w342:i32, "Presets[2]"=w341:i32, "Presets[3]"=w340:i32)  [unwired: 5 out]
        n2053 = property on="X Step SP" class="DigNum (strict)"("Val(Sgnl)"=w343) -> ()  [unwired: 2 in, 2 out]
        n2054 = property on="Y Step SP" class="DigNum (strict)"("Val(Sgnl)"=w342) -> ()  [unwired: 2 in, 2 out]
        n2055 = property on="Z Step SP" class="DigNum (strict)"("Val(Sgnl)"=w341) -> ()  [unwired: 2 in, 2 out]
        n2056 = property on="R Step SP" class="DigNum (strict)"("Val(Sgnl)"=w340) -> ()  [unwired: 2 in, 2 out]
      }
    }
    n2057 = property on="STATUS" class="Str"() -> ("Value"=w289:string)  [unwired: 2 in, 2 out]
    n2058 = Equal?(x=w289, y="SCANNING MODE" ("STATUS")) -> (x = y?=w287:bool)
    "Scanning" <- w287
    n2059 = case shown="True" "Laser Shutter" {
      tunnel: "SHUTTER SYNC" -> [w323 _]
      tunnel: w287 -> [w322 _]
      frame #0 {
        # "SHUTTER SLAVE MODE"
        n2060 = And(x=w323, y=w322) -> (x .and. y?=w324:bool)
        n2061 = case shown="False" w324 {
          frame #0 {
            # "CLOE SHUTTER"
          }
          frame #1 {
            # "OPEN SHUTTER"
          }
        }
      }
      frame #1 {
        # "FORCE TO OPEN SHUTTER"
      }
    }
    n2062 = case shown="True" "Stop" {
      selector: "Stop" -> [w356 w398]
      tunnel: [w356 w395] -> w303
      tunnel: w286 -> [w355 w364]
      tunnel: w283 -> [w354 w363]
      tunnel: [w355 w371] -> w312
      tunnel: [w353 w377] -> w311
      tunnel: [w352 w374] -> w310
      tunnel: [w351 w383] -> w309
      tunnel: [w349 w366] -> w308
      tunnel: [w348 w365] -> w307
      tunnel: [w350 w380] -> w306
      tunnel: [w354 w368] -> w305
      tunnel: w302 -> [_ w390]
      tunnel: w301 -> [_ w367]
      tunnel: w285 -> [w353 w362]
      tunnel: w284 -> [w352 w361]
      tunnel: w282 -> [w351 w360]
      tunnel: w281 -> [w350 w359]
      tunnel: w280 -> [w348 w358]
      tunnel: w279 -> [w349 w357]
      frame #0 {
      }
      frame #1 {
        n2063 = flat-sequence {
          tunnel: w398 -> [w464]
          tunnel: [w464] -> w397
          tunnel: [w463] -> w393
          tunnel: [w462] -> w391
          tunnel: w390 -> [w462]
          tunnel: [w417] -> w388
          tunnel: [w416] -> w386
          tunnel: [w426] -> w384
          tunnel: [w425] -> w381
          tunnel: [w436] -> w378
          tunnel: [w434] -> w375
          tunnel: [w445] -> w372
          tunnel: [w443] -> w369
          tunnel: w367 -> [w453]
          tunnel: w364 -> [w406]
          tunnel: w363 -> [w405]
          tunnel: w362 -> [w404]
          tunnel: w361 -> [w403]
          tunnel: w360 -> [w402]
          tunnel: w359 -> [w401]
          tunnel: w358 -> [w400]
          tunnel: w357 -> [w399]
          tunnel: w397 -> [w476]
          tunnel: [w476] -> w396
          tunnel: [w465] -> w394
          tunnel: w393 -> [w475]
          tunnel: [w474] -> w392
          tunnel: w391 -> [w474]
          tunnel: [w473] -> w389
          tunnel: w388 -> [w473]
          tunnel: [w472] -> w387
          tunnel: w386 -> [w472]
          tunnel: [w471] -> w385
          tunnel: w384 -> [w471]
          tunnel: [w470] -> w382
          tunnel: w381 -> [w470]
          tunnel: [w469] -> w379
          tunnel: w378 -> [w469]
          tunnel: [w468] -> w376
          tunnel: w375 -> [w468]
          tunnel: [w467] -> w373
          tunnel: w372 -> [w467]
          tunnel: [w466] -> w370
          tunnel: w369 -> [w466]
          tunnel: w396 -> [w488]
          tunnel: [w488] -> w395
          tunnel: w394 -> [w479]
          tunnel: w392 -> [w487]
          tunnel: w389 -> [w478]
          tunnel: [w478] -> _
          tunnel: w387 -> [w486]
          tunnel: [w486] -> w365
          tunnel: w385 -> [w485]
          tunnel: [w485] -> w383
          tunnel: [w484] -> w380
          tunnel: w382 -> [w484]
          tunnel: [w483] -> w377
          tunnel: w379 -> [w483]
          tunnel: [w482] -> w374
          tunnel: w376 -> [w482]
          tunnel: [w481] -> w371
          tunnel: w373 -> [w481]
          tunnel: [w480] -> w368
          tunnel: w370 -> [w480]
          tunnel: [w478] -> w366
          frame #0 {
            # "R"
            # "Y"
            # "Z"
            # "X"
            n2064 = local read "Presets"() -> (w452:i32[][])
            n2065 = property on="Preset positions" class="Ring (strict)"() -> ("Strings []"=w451:string[])  [unwired: 2 in, 2 out]
            n2066 = property on="R Ready" class="Bool (strict)"("Val(Sgnl)"=FALSE ("Value (Signaling)")) -> ()  [unwired: 2 in, 2 out]
            n2067 = property on="R in Range" class="Bool (strict)"("Val(Sgnl)"=FALSE ("Value (Signaling)")) -> ()  [unwired: 2 in, 2 out]
            n2068 = property on="Z in Range" class="Bool (strict)"("Val(Sgnl)"=FALSE ("Value (Signaling)")) -> ()  [unwired: 2 in, 2 out]
            n2069 = property on="Z Ready" class="Bool (strict)"("Val(Sgnl)"=FALSE ("Value (Signaling)")) -> ()  [unwired: 2 in, 2 out]
            n2070 = property on="Y in Range" class="Bool (strict)"("Val(Sgnl)"=FALSE ("Value (Signaling)")) -> ()  [unwired: 2 in, 2 out]
            n2071 = property on="X  in Range" class="Bool (strict)"("Val(Sgnl)"=FALSE ("Value (Signaling)")) -> ()  [unwired: 2 in, 2 out]
            n2072 = property on="Y Ready" class="Bool (strict)"("Val(Sgnl)"=FALSE ("Value (Signaling)")) -> ()  [unwired: 2 in, 2 out]
            n2073 = property on="X Ready" class="Bool (strict)"("Val(Sgnl)"=FALSE ("Value (Signaling)")) -> ()  [unwired: 2 in, 2 out]
            n2074 = Number To Fractional String(number=w452) -> (F-format string=w454:string[][])  [unwired: 3 in]
            n2075 = call "mDrive Send Command.vi"("error in (no error)"=w405, "Command"=T10."Stop", "VISA resource name"=w406) -> ("error out"=w444:errorcluster, "VISA resource name out"=w446:refnum<visa-resource-name>)  [unwired: 4 in, 1 out]
            n2076 = call "mDrive Send Command.vi"("error in (no error)"=w403, "Command"=T10."Stop", "VISA resource name"=w404) -> ("error out"=w435:errorcluster, "VISA resource name out"=w437:refnum<visa-resource-name>)  [unwired: 4 in, 1 out]
            n2077 = Transpose 2D Array(2D array=w454) -> (transposed array=w455:string[][])
            n2078 = call "mDrive Send Command.vi"("error in (no error)"=w401, "Command"=T10."Stop", "VISA resource name"=w402) -> ("error out"=w427:errorcluster, "VISA resource name out"=w428:refnum<visa-resource-name>)  [unwired: 4 in, 1 out]
            n2079 = call "mDrive Send Command.vi"("error in (no error)"=w400, "Command"=T10."Stop", "VISA resource name"=w399) -> ("error out"=w418:errorcluster, "VISA resource name out"=w419:refnum<visa-resource-name>)  [unwired: 4 in, 1 out]
            n2080 = Build Array (concatenate)(w451, w455) -> (w456:string[][])
            n2081 = Transpose 2D Array(2D array=w456) -> (transposed array=w457:string[][])
            n2082 = call "mDrive Send Command.vi"("error in (no error)"=w444, "Extra"="P", "Command"=T10."Print Parameter", "VISA resource name"=w446) -> ("error out"=w443:errorcluster, "read buffer"=w450:string, "VISA resource name out"=w445:refnum<visa-resource-name>)  [unwired: 3 in]
            n2083 = call "mDrive Send Command.vi"("error in (no error)"=w435, "Extra"="P", "Command"=T10."Print Parameter", "VISA resource name"=w437) -> ("error out"=w434:errorcluster, "read buffer"=w441:string, "VISA resource name out"=w436:refnum<visa-resource-name>)  [unwired: 3 in]
            n2084 = call "mDrive Send Command.vi"("error in (no error)"=w427, "Extra"="P", "Command"=T10."Print Parameter", "VISA resource name"=w428) -> ("error out"=w425:errorcluster, "read buffer"=w432:string, "VISA resource name out"=w426:refnum<visa-resource-name>)  [unwired: 3 in]
            n2085 = call "mDrive Send Command.vi"("error in (no error)"=w418, "Extra"="P", "Command"=T10."Print Parameter", "VISA resource name"=w419) -> ("error out"=w416:errorcluster, "read buffer"=w423:string, "VISA resource name out"=w417:refnum<visa-resource-name>)  [unwired: 3 in]
            n2086 = call-poly <vilib>:"Write To Spreadsheet File.vi"("2D data"=w457, "file path (dialog if empty)"=w453) -> ()  [unwired: 6 in, 1 out]
            n2087 = Decimal String To Number(string=w450, offset=0) -> (number=w442:i32)  [unwired: 1 in, 1 out]
            n2088 = Decimal String To Number(string=w441, offset=0) -> (number=w433:i32)  [unwired: 1 in, 1 out]
            n2089 = Decimal String To Number(string=w432, offset=0) -> (number=w424:i32)  [unwired: 1 in, 1 out]
            n2090 = Decimal String To Number(string=w423, offset=0) -> (number=w415:i32)  [unwired: 1 in, 1 out]
            n2091 = Build Array(w442, w424, w433, w415) -> (w463:i32[])
          }
          frame #1 {
            n2092 = To Double Precision Float(number=w475) -> (double precision float=w465:dbl[])
            n2093 = Wait (ms)(milliseconds to wait=u32 20) -> ()  [unwired: 1 out]
          }
          frame #2 {
            n2094 = call-poly <vilib>:"Write To Spreadsheet File.vi"("1D data"=w479, "file path (dialog if empty)"=w487) -> ()  [unwired: 6 in, 1 out]
          }
        }
      }
    }
  }
  n2095 = flat-sequence {
    tunnel: w58 -> [w4303]
    tunnel: w57 -> [w4300]
    frame #0 {
      n2096 = call "mDrive Send Command.vi"("error in (no error)"=w4300, "Command"=T10."Stop", "VISA resource name"=w4303) -> ("error out"=w4301:errorcluster, "VISA resource name out"=w4302:refnum<visa-resource-name>)  [unwired: 4 in, 1 out]
      n2097 = VISA Close(VISA resource name=w4302, error in (no error)=w4301) -> ()  [unwired: 1 out]
    }
  }
  n2098 = flat-sequence {
    tunnel: w52 -> [w4308]
    tunnel: w51 -> [w4305]
    frame #0 {
      n2099 = call "mDrive Send Command.vi"("error in (no error)"=w4305, "Command"=T10."Stop", "VISA resource name"=w4308) -> ("error out"=w4306:errorcluster, "VISA resource name out"=w4307:refnum<visa-resource-name>)  [unwired: 4 in, 1 out]
      n2100 = VISA Close(VISA resource name=w4307, error in (no error)=w4306) -> ()  [unwired: 1 out]
    }
  }
  n2101 = flat-sequence {
    tunnel: w50 -> [w4313]
    tunnel: w49 -> [w4310]
    frame #0 {
      n2102 = call "mDrive Send Command.vi"("error in (no error)"=w4310, "Command"=T10."Stop", "VISA resource name"=w4313) -> ("error out"=w4311:errorcluster, "VISA resource name out"=w4312:refnum<visa-resource-name>)  [unwired: 4 in, 1 out]
      n2103 = VISA Close(VISA resource name=w4312, error in (no error)=w4311) -> ()  [unwired: 1 out]
    }
  }
  n2104 = flat-sequence {
    tunnel: w48 -> [w4318]
    tunnel: w47 -> [w4315]
    frame #0 {
      n2105 = call "mDrive Send Command.vi"("error in (no error)"=w4315, "Command"=T10."Stop", "VISA resource name"=w4318) -> ("error out"=w4316:errorcluster, "VISA resource name out"=w4317:refnum<visa-resource-name>)  [unwired: 4 in, 1 out]
      n2106 = VISA Close(VISA resource name=w4317, error in (no error)=w4316) -> ()  [unwired: 1 out]
    }
  }
  "YCONSTArray" <- w46
  "XCONSTArray" <- w45
  "RCONSTArray" <- w44
  "ZCONSTArray" <- w43
  "RUNHOLDArray" <- w42
